vi "UHR-Fleezers Control (host) - Mau_06pol.vi"() -> ()   [LabVIEW 2012]
uses:
  <vilib>/Utility/miscctls.llb/LVPoint32TypeDef.ctl
  <vilib>/Utility/miscctls.llb/LVMinMaxIncTypeDef.ctl
  <vilib>/userdefined/High Color/nirio_resource_hc.ctl
  <vilib>/Platform/TimedLoop/XDataNode/timing_clust.ctl
  <vilib>/Platform/TimedLoop/XDataNode/nitl_modes.ctl
  <vilib>/Platform/TimedLoop/XDataNode/wakeup.ctl
  <vilib>/FPGAPlugInAG/PCIe-7852R/niLvFpga_Open_PCIe-7852R.vi
  <vilib>/FPGAPlugInAG/PCIe-7852R/niLvFpga_Reset_PCIe-7852R.vi
  <vilib>/Utility/error.llb/Error Cluster From Error Code.vi
  <vilib>/rvi/errors/niLvFpgaAdjustHostInterfaceError.vi
  <vilib>/FPGAPlugInAG/PCIe-7852R/niLvFpga_Run_PCIe-7852R.vi
  <vilib>/Analysis/baseanly.llb/Mean (DBL).vi
  <vilib>/express/express analysis/Spectral/Block/exnSpectralBlock spectral measurements PSD poly.vi
  <vilib>/express/express analysis/Spectral/Block/exnSpectralBlock spectral measurements PSD WFM.vi
  <vilib>/Waveform/WDTOps.llb/WDT Append Waveforms DBL.vi
  <vilib>/FPGAPlugInAG/PCIe-7852R/niLvFpga_Abort_PCIe-7852R.vi
  <vilib>/FPGAPlugInAG/PCIe-7852R/niLvFpga_Close_PCIe-7852R.vi
  openfpgaref.8.6.ctl
  <vilib>/Platform/TimedLoop/XDataNode/XDataNode.xnode
  <vilib>/rvi/interface/nirviOpenFPGA/nirviOpenFPGA.xnode
  FPGA Bitfiles/UHR-FleezersInst_FPGATarget_UHR-FleezersCont_0F5B06C4.lvbitx
  UHR-Fleezers Control (fpga) - 10.3.vi
  <vilib>/rvi/interface/nirviMethod/nirviMethod.xnode
  <vilib>/rvi/interface/nirviReadWriteControl/nirviReadWriteControl.xnode
  <vilib>/express/express analysis/Spectral/XNode/ExpressSpectralMeasurementsBlockNode.xnode
  <vilib>/rvi/interface/nirviCloseFPGA/nirviCloseFPGA.xnode
  <vilib>/Analysis/NI_AALBase.lvlib
  <vilib>/Platform/TimedLoop/XDataNode/XDNodeRunTimeDep.lvlib
  <vilib>/vision/NI_Vision_Development_Module.lvlib
  NiFpgaLv.dll
  <vilib>/FPGAPlugInAG/PCIe-7852R/niLvFpga_ConfigureFifo_PCIe-7852R.vi
  <vilib>/rvi/errors/niLvFpgaMergeErrorWithErrorCode.vi
  <vilib>/FPGAPlugInAG/PCIe-7852R/niLvFpga_ReadFifo_PCIe-7852R.vi
panel:
  in  "BD 1 Frequency 1 (MHz) 2":dbl=65.0 caption="T1 X (MHz)" min=50.0 max=100.0 step=1.0 format="%#_6p"
  in  "ESP Port 8":refnum<visa-resource-name>="COM22"
  in  "ESP Port 7":refnum<visa-resource-name>="COM22"
  in  "ESP Port 6":refnum<visa-resource-name>="COM22"
  in  "ESP Port 5":refnum<visa-resource-name>="COM22"
  in  "ESP Port 4":refnum<visa-resource-name>="COM22"
  in  "ESP Port 3":refnum<visa-resource-name>="COM22"
  in  "ESP Port 2":refnum<visa-resource-name>="COM22"
  out "Location path":path=path "D:/UnifiedHighRes_VIs/Locations.txt"
  out "Location Matrix":string[][](array[string])=[["N.D.\r\n", "N.D.\r\n", "N.D.\r\n"], ["0.19233\r\n", "0.00156\r\n", "0.20615\r\n"], ["N.D.\r\n", "N.D.\r\n", "N.D.\r\n"], ["N.D.\r\n", "N.D.\r\n", "N.D.\r\n"]]
  in  "radius":i32=10 min=1 max=20
  in  "clear markers":bool
  in  "trap\nmarkers?":bool
  in  "Sample Channel Flow":bool
  in  "Pump 3 contents":string="Bottom: ADig beads" caption="contents"
  in  "Pump 1 contents":string="Top: DNA beads" caption="contents"
  in  "Scripts":T1(tab)
  in  "Take Stepping Data":bool
  in  "Got DNA bead":bool
  in  "Got ADig bead":bool
  in  "Cap 1 Flow ON":bool=TRUE
  in  "Move Cap. 1 (DNA Top)":bool
  in  "Cal/Data Acq. Spot":bool
  in  "Dump Beads":bool
  in  "Cap 1 T ON":bool=TRUE
  in  "Cap 1 Samp Flow ON":bool=TRUE
  in  "Offset 2 Set":dbl=2.0
  in  "Offset 1 Set":dbl=1.0
  in  "Cal @ (MHz)":dbl=20.0
  in  "W/ Offset 1":bool=TRUE
  in  "Offset 1 Start (MHz)":dbl=13.0
  in  "W/ Offset 2":bool
  in  "Offset 2 Start (MHz)":dbl=16.0
  in  "Pause at Closest Delta (s)":dbl
  in  "Move to Delta 2 (MHz)":dbl=41.0
  in  "Attempt Limit":dbl=30.0 caption="Limit"
  out "Attempts":dbl=1.0
  in  "Wait Before Save (s)":u32=1
  in  "Fish for Tether":bool
  in  "Closest Delta (MHz)":dbl=13.0 step=0.25
  in  "Stop F (pN)":dbl=10.0
  in  "Then...":string(combo)="2"
  in  "Move to Delta 1 (MHz)":dbl=15.0
  in  "Tether Alarm?":bool=TRUE
  out "Tether":bool
  in  "TA Cancel Save?":bool=TRUE
  in  "TA Green Off?":bool=TRUE
  in  "Raster Set Upon Tether":u32=1
  in  "Save at end (5, 6)":bool
  in  "N Steps":dbl=20.0
  in  "Step Size (nm)":dbl=0.34
  in  "Save ave factor":dbl=1.0
  in  "Dip Trap Delta 1 (MHz)":dbl=15.0
  in  "Move Trap Before?":bool
  in  "Save Data After?":bool
  in  "Green ON After?":bool
  in  "Dip Trap Delta 2 (MHz)":dbl=15.0
  in  "Move Trap After?":bool
  in  "Duration (s)":dbl=1.0
  in  "Dip for Protein":bool
  in  "APD to Watch":bool
  out "Duration (s)":dbl
  in  "Action":string(combo)="Yank"
  in  "Fl. Triggered...":bool
  in  "Fl. Delta Thresh. (kHz)":dbl=0.6
  out "Waiting":bool
  out "Fl. High":bool
  in  "N pts to average":u16=6
  in  "Yank Delay (s)":dbl=3.5
  in  "Yank to Delta Array (MHz)":dbl[](array[numeric])=[16.3, 15.85, 14.85]
  in  "N Array El":u8=3 min=1 step=1
  in  "Random Choice":bool=TRUE
  in  "Force Yank":bool
  in  "Force Reset":bool
  in  "Y change (mm)":dbl
  in  "Profile":bool
  out "Sigma/Mean 2":dbl=nan caption="Sigma/Mean" format="%#_2g"
  out "Rate sigma (Hz) 2":dbl caption="Sigma (Hz)" format="%0.2f"
  out "APD 2 Rate (Hz)":dbl format="%#_3p"
  out "Primary Video Display":T2(plugin-control)
  out "Waveform Graph":dbl[](graph) caption="APD Line Scan"
  in  "Inject Top":bool caption="Inject Pump 3"
  in  "Inject Bottom":bool caption="Inject Pump 1"
  out "Messages":string="7:59 AM\tUHR-Fleezers ready.\r"
  in  "APD Ave N":dbl=10.0
  out "Int. Time (s)":dbl=3.0
  in  "Stop All":bool=TRUE
  out "Sigma/Mean":dbl=nan format="%#_2g"
  out "Rate sigma (Hz)":dbl caption="Sigma (Hz)" format="%0.2f"
  in  "Tab Control 6":T3(tab)=enum."Imaging"
  in  "APD 2 Offset":dbl
  in  "APD 1 Offset":dbl
  out "RMS (Ang)":dbl=nan format="%_2g"
  in  "Bead Sep. Int. Time (s)":dbl=5.0 caption="Int. Time (s)"
  in  "Below (kHz)":dbl=0.5
  in  "Above (kHz)":dbl=2.0
  in  "Adjust Scale\nto Mean":bool
  in  "Rescale on Mean":bool
  in  "Offset (nm)":dbl
  out "Mean":dbl=nan caption="Mean (V)" format="%#_3g"
  out "Force":waveform(dbl)[](graph)=[{"t0"=timestamp(12.90000000000001 s since 1904-01-01), "dt"=0.15, "Y"=[nan, nan], "attributes"=variant("NI_ChannelName"=variant(string "T1 X"))}, {"t0"=timestamp(12.90000000000001 s since 1904-01-01), "dt"=0.15, "Y"=[nan, nan], "attributes"=variant("NI_ChannelName"=variant(string "T2 X"))}]
  out "APD Chart":waveform(dbl)[](graph)=[{"t0"=timestamp(12.90000000000001 s since 1904-01-01), "dt"=0.02, "Y"=[0.0, 0.0, 0.0, 0.0, 0.0, 0.0, 0.0, 0.0, 0.0, 0.0, 0.0, 0.0, 0.0, 0.0, 0.0], "attributes"=variant("NI_ChannelName"=variant(string "APD 1"))}, {"t0"=timestamp(12.90000000000001 s since 1904-01-01), "dt"=0.02, "Y"=[0.0, 0.0, 0.0, 0.0, 0.0, 0.0, 0.0, 0.0, 0.0, 0.0, 0.0, 0.0, 0.0, 0.0, 0.0], "attributes"=variant("NI_ChannelName"=variant(string "APD 2"))}]
  in  "Calibration":u16(ring) items=["None", "Position", "Force"]
  out "T1 X":dbl=nan caption="T1 X (V)" format="%0.2f"
  out "T2 X":dbl=nan caption="T2 X (V)" format="%0.2f"
  out "Bead Separation":waveform(dbl)(graph)={"t0"=timestamp(12.90000000000001 s since 1904-01-01), "dt"=0.15, "Y"=[nan, nan], "attributes"=variant("NI_ChannelName"=variant(string "T1 X"))}
  in  "Amplitude (nm)":dbl=3.0
  out "Bead Mean (nm)":dbl=nan caption="Mean (nm)" format="%0.2f"
  out "Difference":dbl=nan caption="Difference (V)" format="%.2g"
  in  "Take Detection Laser\nImage":bool
  out "APD 2":T2(plugin-control) caption="APD 2 (Cy5)"
  in  "Flip Green Filter":bool
  in  "Set X Only":bool
  in  "Set Y Only":bool
  out "APD 1":T2(plugin-control) caption="APD 1 (Cy3)"
  out "Detection Laser Y":T2(plugin-control)
  out "Pointer Y (V)":dbl format="%_3g"
  out "Pointer X (V)":dbl format="%_3g"
  in  "Set Confocal Spot (X-Y)":bool
  out "Detection Laser X":T2(plugin-control)
  out "Saved APD":dbl[][](graph) caption="Most Recent Time Trace"
  out "Trap Delta Graph":dbl[](graph) caption="Most Recent Time Trace"
  out "Save APD Deriv":dbl[][](graph) caption="Most Recent Time Trace"
  out "Delta Fl. 1":dbl
  out "Delta Fl. 2":dbl
  out "All Signals":waveform(dbl)[](graph)=[{"t0"=timestamp(12.90000000000001 s since 1904-01-01), "dt"=0.02, "Y"=[0.0, 0.0, 0.0, 0.0, 0.0, 0.0, 0.0, 0.0, 0.0, 0.0, 0.0, 0.0, 0.0, 0.0, 0.0], "attributes"=variant("NI_ChannelName"=variant(string "APD 1"))}, {"t0"=timestamp(12.90000000000001 s since 1904-01-01), "dt"=0.02, "Y"=[0.0, 0.0, 0.0, 0.0, 0.0, 0.0, 0.0, 0.0, 0.0, 0.0, 0.0, 0.0, 0.0, 0.0, 0.0], "attributes"=variant("NI_ChannelName"=variant(string "APD 2"))}, {"t0"=timestamp(12.90000000000001 s since 1904-01-01), "dt"=0.15, "Y"=[nan, nan], "attributes"=variant("NI_ChannelName"=variant(string "T1 Y"))}, {"t0"=timestamp(12.90000000000001 s since 1904-01-01), "dt"=0.15, "Y"=[nan, nan], "attributes"=variant("NI_ChannelName"=variant(string "T1 X"))}, {"t0"=timestamp(12.90000000000001 s since 1904-01-01), "dt"=0.15, "Y"=[-0.0004235663930173644, -0.0004722739341410556], "attributes"=variant("NI_ChannelName"=variant(string "T1 Sum"))}, {"t0"=timestamp(12.90000000000001 s since 1904-01-01), "dt"=0.15, "Y"=[nan, nan], "attributes"=variant("NI_ChannelName"=variant(string "T2 Y"))}, {"t0"=timestamp(12.90000000000001 s since 1904-01-01), "dt"=0.15, "Y"=[nan, nan], "attributes"=variant("NI_ChannelName"=variant(string "T2 X"))}, {"t0"=timestamp(12.90000000000001 s since 1904-01-01), "dt"=0.15, "Y"=[-0.0005883053071687949, -0.0006281319620349712], "attributes"=variant("NI_ChannelName"=variant(string "T2 Sum"))}, {"t0"=timestamp(12.90000000000001 s since 1904-01-01), "dt"=0.15, "Y"=[nan, nan], "attributes"=variant("NI_ChannelName"=variant(string "T1 FB X"))}, {"t0"=timestamp(12.90000000000001 s since 1904-01-01), "dt"=0.15, "Y"=[-0.0004680013428144157, -0.0005167699209570592], "attributes"=variant("NI_ChannelName"=variant(string "T2 FB Sum"))}, {"t0"=timestamp(12.90000000000001 s since 1904-01-01), "dt"=0.15, "Y"=[nan, nan], "attributes"=variant("NI_ChannelName"=variant(string "T2 FB X"))}, {"t0"=timestamp(12.90000000000001 s since 1904-01-01), "dt"=0.15, "Y"=[-0.0006226691488387671, -0.0006504715109714008], "attributes"=variant("NI_ChannelName"=variant(string "T2 FB Sum"))}, {"t0"=timestamp(12.90000000000001 s since 1904-01-01), "dt"=0.15, "Y"=[-0.0007901852473525123, -0.0008601641895809732], "attributes"=variant("NI_ChannelName"=variant(string "PSD Y"))}, {"t0"=timestamp(12.90000000000001 s since 1904-01-01), "dt"=0.15, "Y"=[0.00031556138798181086, 0.0002525101474044007], "attributes"=variant("NI_ChannelName"=variant(string "PSD X"))}, {"t0"=timestamp(12.90000000000001 s since 1904-01-01), "dt"=0.15, "Y"=[-0.00019678334910122974, -0.0002453993346964931], "attributes"=variant("NI_ChannelName"=variant(string "PSD Sum"))}]
  in  "Signals to Plot":i32(listbox)
  out "Trap Disp. Freq. (Hz)":dbl=6.666666666666667 caption="Freq. (Hz)" format="%#_6p"
  out "Display Period (s)":dbl=0.15 caption="Period (s)" format="%#_6p"
  in  "Trap Disp. Downsample":dbl=10000.0 caption="Downsample" max=20000.0
  in  "APD Disp. Scale":dbl=0.1 caption="Scale (Divide,\nfor above plot only)"
  in  "APD Disp. Downsample":dbl=2.0 caption="Integrate" min=1.0 max=30.0 step=1.0
  out "APD Display Freq. (Hz)":dbl=50.0 caption="Freq. (Hz)"
  out "APD Display Period (s)":dbl=0.02 caption="Period (s)"
  out "FFT 1":cluster{"f0":dbl, "df":dbl, "magnitude":dbl[]}[](graph)=[{"f0"=0.0, "df"=16.666666666666668, "magnitude"=[-331.1367572010275, -79.05506245821404, -86.61411242440559, -88.4728176091699, -90.3181253945935, -94.12566333707997, -92.52740723119955, -94.92192587982518, -99.60936585245742, -96.87568627870715, -94.02570383337763, -83.8058550151726, -97.57441397235512, -101.59968530846606, -101.523049255742, -103.35038532190343, -101.58594091014982, -102.96098031851216, -91.39759462745924, -103.75019963279499, -104.45030075054324, -103.04245334279298, -104.0720279134107, -106.06482372394834, -103.69131867828104, -104.40395035115309, -105.96420043276396, -107.6735556337804, -106.673030006608, -107.34889066208132, -108.05626565233933, -106.25659018850432, -105.29934513380842, -105.43096056709592, -108.3728498841465, -106.0555440144992, -105.78001282181421, -107.48741857324953, -108.67624970548897, -105.39976667156175, -105.91413119232612, -109.4222808198164, -107.0898971593174, -107.91164191890915, -108.26032038855709, -107.58332347164534, -108.23559688234297, -108.01271040303237, -107.66511723652701, -106.51901583170391, -109.27249501469946, -108.55647681594805, -107.93499259231463, -107.05068166453935, -109.13641475410455, -109.29679733781423, -108.19360835527803, -109.57747591546632, -109.58364591011674, -110.47061433372711, -109.8144340420426, -108.79067462293897, -107.54887553357234, -107.99559866705923, -108.85023923652685, -109.68733225238618, -108.51101278437793, -108.51620475114115, -108.22212402200637, -104.63726950302143, -110.2989919678048, -107.61796444414897, -108.68882962798736, -104.79193983043893, -103.59504263746938, -93.64633660288543, -101.9191640501395, -105.73717393151816, -108.92572458793902, -107.43962662800902, -107.79595323081325, -107.0923101993207, -108.17603277205289, -107.87074270713183, -109.20899066381877, -108.61832060412445, -109.10072003106593, -105.76480632823524, -108.60877649218978, -109.67541158970121, -110.2286232768028, -109.84952155309578, -109.33772024076384, -109.95251642394683, -110.14777282585466, -109.13825677905699, -110.05989365698167, -109.39359990189426, -110.56255614635295, -109.66477183197163, -108.9397158528824, -110.26529907650465, -109.20049464984628, -108.20183857013548, -109.09752250184418, -108.00440442238454, -108.35465963524055, -111.16774134451799, -110.34812550238405, -108.94506763426756, -108.72845542102493, -109.41512344014713, -112.44661664432377, -110.35437330889101, -111.32939440655925, -109.42989530434981, -110.98084669076195, -111.92160561143541, -108.57755551751093, -111.40042616180912, -110.15284955891853, -112.21455132279115, -111.40787773511747, -108.82949641635288, -110.13442122547907, -111.42229298204664, -112.06314940885191, -110.6015308813694, -109.51144097251623, -111.15989713761475, -110.25535755335385, -109.65868178057926, -110.51649885452997, -109.77194745285269, -108.4234206864394, -109.50892632093968, -109.46471287444389, -107.92241289271415, -109.72283805386196, -108.63426821579918, -110.37316681536255, -111.09713996884652, -110.32903619589223, -105.32012665515045, -107.36858557554393, -108.00382215905725, -110.06430686942338, -108.81666625979916, -110.01277074453823, -110.94194741225512, -109.65934609082873, -107.80979136006962, -112.81333866824724, -111.61474300955487, -109.83998277184975, -109.45953946904639, -109.79640584952526, -108.19172301667324, -109.28894656674316, -107.61471301278785, -108.83814006090513, -109.08866847726084, -108.20250571862371, -107.96222236861584, -107.03811197900873, -108.93533000393974, -107.74482548035408, -110.79811544577694, -111.1387476496877, -107.42970105883512, -109.18442281176472, -108.73546184641192, -108.71800246690864, -108.51945944378063, -108.06825856571285, -107.27210712368412, -108.12304695877637, -107.84933283677306, -109.73682373154998, -109.32284761503395, -109.31328817453769, -106.68762108642842, -109.79203616876461, -109.9020278896408, -110.27080024357275, -108.54152101558762, -111.00464391726017, -112.42244020766577, -110.82707315747889, -111.00344011890857, -109.90461839395674, -109.42877207451863, -109.73549298167016, -111.67494793393293, -108.85799077901427, -108.5348443278263, -109.803781083881, -108.30644755543659, -108.5079527456017, -111.2055351312823, -108.53089994340155, -108.01739789012176, -108.70360662855235, -107.95873456794631, -109.58297170693093, -108.9372401694271, -110.15921663527153, -109.22399119911955, -110.89883651739237, -108.92840112258382, -110.0545300523626, -109.05961065387005, -109.45831398589371, -108.61239387653227, -110.13001256174265, -108.80060224137931, -109.46327400696283, -108.0177965824709, -109.29727944627197, -110.3237255895986, -109.03258262543821, -110.97880178489321, -109.70034895077919, -111.16405638194153, -109.17324451464711, -109.65698250854277, -108.96750235822178, -112.00534231585624, -108.69274607723942, -108.98110446396657, -108.40723795464795, -111.44459094807324, -111.74799245277113, -111.1601960491512, -108.92048232753773, -110.30506377784799, -111.33145973979093, -110.91850998672503, -110.33684985776448, -108.90206518366908, -109.28458878227542, -108.98773986023751, -110.85813863075646, -109.00041591105906, -110.84543686681204, -109.84382395806176, -109.69722434763266, -108.50915601095721, -107.80829925826895, -110.59736107582401, -109.75377770317087, -109.3992084496136, -110.51151565846742, -112.49753959826434, -109.7299632589479, -109.54070743868353, -109.90314341132164, -111.05974202976806, -109.03766862152392, -109.46667095459878, -109.52800799036197, -111.3163121356807, -110.07817134522178, -108.69251657453547, -109.40472158898045, -109.71400709815576, -110.60534468715097, -109.46937396724682, -107.70342491418788, -109.86331122597839, -108.64971387994616, -110.90117371097081, -108.34928840565928, -110.04172889660904, -111.52979926554961, -110.34759300823305, -109.62712781837159, -109.24131154553284, -110.23196152450447, -108.68509612326807, -108.0246905483419, -106.61876139289784, -101.5519630114271, -80.57695480953835, -102.03744443354402, -107.1449217193017, -110.0695213407169, -106.61597783999268, -110.79221011808191, -109.58974545931426, -109.1149802216988, -109.20993813088597, -109.63768480465863, -110.10428394219181, -109.08445084271477, -108.83472375362581, -109.69508502050168, -108.05588796178941, -110.62586360101581, -109.95315261676905, -107.52208264977473, -108.80708007514875, -110.43484881098874, -110.45942171588936, -107.83804717866751, -109.98973910294193, -109.3496496054193, -108.425252911127, -110.94579264380809, -108.54181722177951, -108.67696070083541, -108.4150202151644, -109.24973583101504, -112.0454922608961, -111.29046597340738, -110.75018248960077, -109.38326363603683, -109.2033340336957, -109.45076170874889, -109.52878049853727, -109.32340869724774, -110.98123395128233, -110.75736340635505, -109.7218385823809, -107.97422606064993, -109.77313701758703, -110.95948744392717, -110.08996774172691, -108.51011830110778, -109.78063140243836, -110.65996628628228, -109.83684298615616, -110.33329049188029, -110.13755118968292, -110.3717925645783, -108.55302219178951, -106.86811628734195, -108.6302156589162, -108.75341391045045, -108.32589578384841, -108.70061474734084, -112.30742263527534, -109.16842570592085, -109.29767035534508, -108.87829025017463, -108.2255616391397, -108.4316108616088, -108.82995906929271, -110.40135575415563, -109.51623498946435, -109.79409808792403, -107.03832759632121, -108.36534528684132, -109.72010868372905, -107.90933028179892, -106.95643597294047, -111.29929166165778, -110.23001135794706, -108.98838015381585, -109.79115357104436, -108.18627479511115, -108.14988122174307, -109.12074063466532, -109.41904850488358, -111.40409873721113, -108.83156790193294, -108.77032248953847, -108.88363158686694, -108.47515048290681, -105.94172147874599, -109.38146940214403, -109.21277078848794, -108.11309390545507, -110.70840012427504, -109.5504457849329, -109.52330684534209, -110.06776026911132, -108.21949434182314, -111.21266686269992, -108.78581501170974, -108.43115799297222, -109.63260325780062, -109.84070220619535, -109.72041980780126, -110.29615941882527, -110.60316734262464, -108.79165446414692, -110.95840439895592, -109.64926233107009, -109.16526769544322, -108.65292362430982, -109.56113898129935, -109.85693046339026, -108.92316027325207, -109.79492493553914, -109.38157962945887, -110.24545136266825, -109.30031463492487, -109.0795429936869, -111.4091719525013, -108.63499083917162, -108.43863465339358, -109.23207864880891, -111.21947487191643, -109.24525201480154, -109.56842406077318, -109.46711940800672, -111.91389548262572, -108.15655736690546, -108.71882059966947, -111.26328503478568, -110.95027143873176, -108.4853106242357, -110.36902802777546, -109.9314203579182, -108.77686164101732, -108.71871020068312, -111.04829661168574, -109.95072655339462, -109.88221342875462, -109.53241732756136, -108.2625005404823, -108.00677030040697, -110.19659317581693, -108.93858924796267, -109.46817875483995, -110.78063992017232, -111.11066570318451, -110.78774336696706, -109.19199744617812, -108.54914256407436, -109.28414960420909, -110.64143585101183, -110.5855350821307, -109.47578632252726, -108.89705360836223, -109.89214013612292, -107.93271261027171, -109.32631601340563, -108.60274611341092, -109.40110159872573, -110.889237682208, -110.01391165813328, -109.99747108785071, -108.65542819213674, -110.37211847668736, -110.44656500845738, -110.8128133834973, -108.8909299260433, -110.19551227077532, -111.37647266643523, -110.83802189730321, -109.98519377913681, -110.52378970770522, -108.16970420057817, -110.70974729773344, -110.76836765494402, -110.26884275594577, -109.22041044268806, -109.87809744746195, -107.76823252107832, -109.12119474042969, -110.28066108731146, -108.55000033509207, -110.18152097767907, -110.73030521152278, -111.49470908029893, -110.2320929919509, -110.03370979233021, -109.79181668155233, -108.6673501209991, -109.86695766650877, -107.88926518046961, -110.95525003776572, -109.18130359755742, -110.42618009658618, -107.90341931158893, -111.44736855661769, -110.72634267386593, -109.29945988519303, -107.67889101961411, -108.81148059987765, -109.13375212757057, -109.8122873383549, -109.80176697684155, -109.96342275204768, -109.90406635707086, -108.75674342748256, -110.12362902701081, -109.82151095527837, -108.62543344241836, -110.09171852771195, -110.21434637862887, -109.97254504855631, -109.27043209093468, -111.35149588204125, -110.12399876776051, -111.65983675538546, -109.28788875768564, -110.86554069990251, -111.26990906470603, -108.60956517491746, -111.49613890850938, -111.79685722966795, -109.26269485364045, -110.38555615546439, -109.40641023162068, -110.966136593156, -108.78892524584494, -110.29340727375603, -111.44032043281035, -109.95212021173755, -109.79233511584334, -112.41184021118175, -109.73687851881148, -108.65493879781806, -110.76132988919045, -108.43230346094671, -110.32968175895853, -110.29890782023821, -108.77609076424456, -110.3298662333555, -109.47734504217333, -108.2677295732245, -109.21234363352882, -107.83278941978479, -108.85136784424789, -108.43241251530755, -109.76609391460555, -108.53204373005357, -110.9660641972934, -110.3152512161094, -110.72570499399905, -109.23877906286317, -111.72407743101837, -109.20311421918561, -108.06021800233717, -109.29288625761943, -108.78395253409145, -111.85250172876302, -108.78827588901797, -109.79775055719482, -109.12089297455859, -109.49896359356035, -110.34432647103819, -107.94700097960238, -109.30489238477631, -108.89170290869342, -108.82574563272509, -110.11024077194833, -107.37946433552314, -109.60167933458756, -107.80625057819019, -110.11489057210264, -107.35436859378505, -105.69819484613895, -109.11280625683739, -109.27770293057978, -107.7053735252589, -109.75022444894368, -109.3310543596577, -107.87683693707739, -108.19931495338068, -109.26462246191564, -106.71885779297867, -100.00018022217961, -92.54434511397295, -107.20472143807373, -107.39203415155283, -110.04461177268398, -108.48860496315312, -109.0057168110333, -108.37627790492552, -108.4108380728248, -109.65509454313073, -109.64243000632982, -97.04219069306761, -109.0928856629964, -107.9760697315632, -107.52611064047497, -108.87702814778996, -109.08437599027614, -110.70097118837974, -109.00969860961283, -110.38275386163214, -110.0699155421545, -106.91498895181175, -106.22178738309017, -109.36827866896039, -107.59953130968307, -109.19516217272808, -108.31502495393616, -109.384158926223, -107.11670654202719, -108.09436312738853, -110.14559230873704, -109.84997663447679, -107.83465335309926, -108.60947100624459, -108.9932479423645, -109.17174810371898, -108.79457339828916, -109.40909327982367, -109.6328723628302, -109.51081854476179, -107.63054408568418, -109.63728404010122, -108.51163794839918, -107.55002282725216, -108.97796212764939, -107.24648164623483, -112.21470452291085, -108.74294024554423, -109.62070777514892, -108.05768666239368, -109.8224946685739, -109.34575507446003, -108.53536952609525, -109.60789300457671, -107.56681538208278, -109.22777325016398, -108.79047910308894, -110.10332477250668, -108.00206387955672, -108.45604004720035, -109.00645795765472, -109.81039564269616, -108.92785144634745, -108.3978471520567, -107.94411095685999, -110.53486519304262, -108.8773780319227, -109.03345093296107, -107.30746693745031, -108.54277704832029, -108.77629108166091, -108.91111762599647, -107.74965195880401, -109.97375370738439, -109.76326492689246, -107.91717581777407, -109.0730556927617, -107.66804873204664, -110.40438871064791, -108.05794247751498, -108.80206615156494, -107.51329354700796, -108.83687012994949, -107.57713176895379, -107.94774159581414, -109.41894615439651, -107.10869425078764, -110.51480854078629, -108.92221367099775, -109.91358786461535, -110.1744263092835, -109.30795472883494, -107.91359710691006, -109.77888185049835, -109.52060975706438, -108.66686651982212, -108.71041801553639, -110.13619546359467, -108.87957097273856, -109.72150387215271, -109.00776068810654, -109.70251113927438, -110.75769213896399, -108.53234896741436, -109.69439526582246, -110.15412541604617, -108.25183374628219, -107.97402569656481, -110.34920156998648, -108.45106995186384, -108.82031145748209, -111.38690005057539, -107.01968459818563, -110.3044500039584, -110.8755481852125, -111.08915057663255, -107.94824988655199, -110.21669144934839, -109.90539774633154, -109.58985438756767, -110.12258796623348, -109.41689951612143, -109.31128210476795, -109.00258476567323, -109.11093063041056, -108.83347064311234, -108.32685287566952, -109.44770946560935, -108.40145063144861, -109.68448193892085, -108.76525439243828, -107.62837139034596, -107.39300298848994, -109.36993934990318, -109.2465218489418, -106.66307369796812, -110.15891092764934, -109.57151745419041, -108.92425698310808, -109.8036704717834, -108.79751146756549, -109.25926431818017, -108.46260574057584, -109.1967554647261, -110.63319560262356, -109.02343067385144, -111.22073171487528, -109.4731095097105, -109.69335000085164, -109.48782989577005, -107.95204227683271, -108.19468255763758, -111.36195112053247, -109.55696116543685, -110.3130767640534, -108.9621824253354, -109.99735074896789, -109.20198058456344, -108.12100614259485, -111.27227490807289, -110.09248554008288, -109.14395535060149, -110.80882692379708, -109.22632926901655, -108.64497210802793, -111.00030482190711, -111.1317849358033, -107.43140429257826, -107.9783302193555, -109.2639893652291, -108.97008485446163, -108.66556668859064, -108.12995785876932, -109.73001061107855, -108.09691302413727, -110.68391499215569, -112.78583642012705, -108.7093037763389, -110.67868795924797, -109.0190959349128, -108.36247198231372, -109.82829353258869, -108.24916379311045, -109.84154533905823, -108.55470160833775, -109.75438989348815, -108.82865632118325, -107.63622268162582, -111.00943492886312, -110.81824358463759, -109.46028423652966, -107.52479398900992, -108.99087806823736, -109.94494831750349, -110.26788355564504, -109.8954055022304, -106.9478122391182, -108.91705388158901, -107.76095584490312, -109.28456723055147, -109.7982307261767, -108.98552661346622, -109.98937979783426, -110.57907422426224, -108.68113463944836, -108.06257240208589, -110.0707224529617, -109.19515280354733, -109.35868842818849, -110.37311467065695, -109.0404734478992, -108.16686395270187, -108.61859220485148, -109.19986437876149, -108.19707189725302, -110.06564239663074, -108.87850403465154, -110.63824157544798, -107.36918104067212, -108.7008736325543, -110.9359398265406, -111.08529123080929, -108.44209934821818, -109.79529621208783, -108.38917887958179, -108.169117639508, -109.24332926356216, -110.50584058811704, -109.63592524002665, -109.32261039377495, -109.16720880524552, -109.3084314664462, -109.5812223978583, -107.70213196487856, -108.0557884982431, -110.67058020007828, -111.68459781023608, -109.66270627185824, -110.52536245663693, -109.70208409132103, -108.78645420809342, -109.23122088059863, -109.24601474121832, -111.25604763816514, -109.50225851581177, -107.32434217163818, -109.28548556764925, -107.59972621660836, -110.46928774723048, -109.25950101547609, -110.32016453935465, -107.78482761561703, -107.89462895091089, -107.51366154391481, -108.08036891159172, -109.53371809947035, -101.2452927166745, -109.32763325689056, -107.52166868423687, -109.89648659445174, -109.11350200980485, -109.81336712738089, -110.02799517445062, -108.02767143538516, -107.97850220501483, -109.50772934896838, -109.31069875721964, -108.49991657749598, -105.60880911233095, -109.79128597340213, -106.91084537903113, -107.84880087118997, -109.63628170511824, -109.03203967193224, -110.64186113413658, -110.98027990365594, -112.33841002907062, -111.01793075565425, -108.58025797022215, -110.4259296883756, -110.38643255981424, -108.93051671115133, -110.97544177116494, -108.63883100482677, -108.37581711765226, -108.90240163126536, -107.94688047875466, -109.9482937437732, -110.09097112364414, -110.09805032265376, -111.44307114024532, -109.15483789122554, -110.9713708217832, -107.8548737634672, -111.41418477109195, -109.45699779859628, -97.03595099331734, -109.16746744169623, -109.66209204485918, -112.57048704774604, -109.73989735035725, -108.16252575067017, -110.7546980664636, -108.91536673403449, -109.20509151422344, -111.0260632167785, -109.62924582406518, -110.45466277291722, -110.2973970018937, -109.67550222925419, -108.84481022020094, -107.23686414357573, -111.79004633370906, -109.85453094194085, -109.45617270081004, -110.73920606732504, -108.90879956851099, -109.67774425528265, -109.4745715721361, -110.18080454693559, -109.26079184315502, -109.41692499885505, -109.02240975088358, -107.80833423058168, -109.32657361431549, -107.87138278655101, -110.910364670719, -109.70067156846706, -108.55301754282077, -109.4243252157005, -109.77567725161107, -107.83737232063925, -110.36509412773016, -109.6371048811367, -109.49430894422814, -108.55509251499753, -108.03996302911446, -110.4385715838736, -110.08864436068788, -109.48922484379962, -109.90865554258562, -109.7491963238264, -110.04796094537969, -107.413043439116, -108.54229076126079, -108.2522516728666, -109.75464941327974, -110.26795832300996, -109.28073673851144, -108.62990200974927, -109.89408067552287, -109.09160284731726, -109.90740624925795, -109.92534708896517, -109.79578862362752, -109.97278346890566, -107.80679350393824, -112.81728446281548, -108.09689504419987, -109.89549991422173, -108.43930976031248, -109.95153099843282, -108.18277483720716, -111.89607792605433, -109.52567003805, -109.17125106979698, -109.64300739407085, -108.21045178846524, -109.64036472149706, -109.02324448538845, -109.039163008889, -110.41006510134076, -109.50289952116489, -110.4732620447796, -110.08777181504614, -110.15589511434341, -109.55705089158471, -109.2547682932589, -110.86823885471617, -109.96330502176939, -109.85995369810554, -110.63211290903473, -112.08007783432191, -110.24725218052279, -107.62861148917592, -110.08691795849435, -108.89793794632287, -111.07702220466341, -109.46946126482341, -109.19747345337464, -110.70018609416007, -109.66366205691908, -110.78032312133551, -108.05724200456513, -108.195661625627, -110.90724508408255, -110.08307674771669, -110.76863516643007, -110.46620425061583, -109.16986788877276, -109.61921294239114, -108.51159432329543, -109.96308336765689, -107.38178944242856, -111.95930944846394, -109.3329826827624, -109.59119636368249, -108.83148571828912, -110.46194288788257, -105.87694286145472, -107.985886302892, -109.2975019660806, -111.05138725716857, -109.60005889204612, -110.92871351729086, -110.73480546964537, -108.41587420326718, -109.84275465824477, -108.8249071047676, -107.65358887817105, -108.3254150042995, -111.47362100321767, -112.7287536850025, -108.8217125660507, -109.50232320231771, -110.29587061625348, -109.30644535112089, -107.69178032077258, -110.84522325672016, -109.3735891463141, -109.12506388923123, -109.65582307934665, -111.11427272192576, -112.19827973435466, -109.11306367925813, -108.19203577968261, -107.89831568266465, -108.85805249169313, -109.51100049661844, -111.71546684086955, -109.53880495724334, -107.07739286222231, -110.66836728754211, -111.5415170557177, -110.16051267940297, -110.6107546662698, -111.36389129556191, -107.77888179117923, -110.34160392509817, -109.61287125994414, -110.23791773883013, -111.00669159903549, -110.97165069538953, -109.43965413392434, -110.6813161690388, -110.31441293654314, -111.96129906273796, -108.15998218707462, -110.08095912053633, -109.41084567452768, -109.28774416263552, -110.80159950384204, -110.41956747809755, -108.85005186267244, -107.9069227847757, -108.84249369063123, -109.92569208845894, -109.34109797584448, -109.41334788055491, -108.76462023086997, -108.22069272136177, -107.0786679601274, -108.30206755098202, -108.57613406368954, -110.83330887636482, -111.93966942736989, -109.76373713473264, -108.25782074884941, -108.16490627215555, -109.93351470267982, -110.75525684428368, -108.22814762283093, -109.73442331991602, -107.53145627482685, -108.27195221226805, -110.33032779278457, -109.48951857415828, -108.12599093700939, -107.97627415508097, -108.81426859968796, -111.21764717894752, -109.80856212352333, -110.92658779118501, -109.71551885834796, -110.38682741010847, -108.87671328341361, -109.68368600774755, -108.35359806351899, -111.7519400010676, -109.89407081573103, -108.24301180922755, -110.00646944788126, -108.6685299083706, -107.52856885980722, -111.7622363038509, -111.0025144494897, -108.64719599357296, -110.62968467177518, -108.821509935539, -107.94915453463719, -111.53070432277694, -109.87282048586256, -110.71167589371663, -109.79225006081626, -109.96203471712074, -110.29921092232489, -110.10644439440416, -111.28815007382043, -111.19165661703703, -108.46024117100558, -110.22528296512183, -110.32184972386672, -110.05120383416072, -109.78792549362107, -109.00355659956696, -108.85989369286315, -113.00899556732638, -110.91756826567867, -111.25016866167897, -111.84225040552181, -110.54451635944174, -110.72722829912917, -109.60759702177283, -110.49362602516815, -108.74419542915284, -110.3379671069179, -109.66259088220754, -110.45956400953156, -109.13956157147233, -109.27130155486806, -110.83015602667983, -109.17970724944131, -109.09662765889193, -108.0447366108107, -108.9536269357457, -110.35663108940085, -108.73418835472056, -113.42965806805827, -111.81270536656905, -110.06155590173537, -108.76582224646269, -106.7488061675813, -108.5700320158723, -111.11038264410035, -110.41435767488723, -109.12763443489911, -109.30517580756394, -111.61251165371237, -109.8116632664339, -109.36845864976851, -109.00390009629231, -110.54359197165573, -109.52629258465976, -110.75932197632896, -109.50903215359567, -107.42652056246085, -107.81146496533543, -103.22224383145215, -108.53803076819163, -109.78623360072066, -109.66306634612869, -110.80245829141279, -111.87835085452016, -102.27372781471168, -111.27763038431458, -108.45838423437681, -108.79077917058028, -109.31951755762685, -110.05415097017186, -109.5535934823387, -111.62732254641111, -110.73478247119641, -109.9468722686683, -110.39698367573979, -109.30612942398305, -109.7578384694043, -109.34817295524313, -105.56944757301993, -110.1940418750125, -109.27076023513962, -111.03491935225027, -112.2980497521063, -110.65725497955563, -109.0567530102422, -110.31700596563523, -109.64508026365678, -109.6190471404421, -110.52566833759428, -109.68595899227789, -109.7431160985074, -110.4798230300751, -109.45506977604765, -110.69504157940786, -110.63067849573177, -108.06456949500138, -107.99354148885966, -108.11349194720599, -109.15944121207349, -110.61766925164031, -110.14145801314527, -110.67420842201165, -111.91532881806512, -112.15901550030345, -109.94774413630104, -109.2819568305201, -110.94623189179737, -110.17685430287735, -110.39082916961016, -109.53953238698966, -110.76940623620611, -109.89327922318515, -109.10275695043765, -110.21445972656734, -110.58968777252528, -110.57016757660259, -109.59208496373341, -109.07946946465374, -109.10762003745964, -110.36892993974607, -109.81864495218393, -112.12972189864566, -109.26185849434863, -111.56305819991357, -111.36019621828058, -110.3397604159226, -109.58675612753163, -110.58041217474447, -106.34739062044932, -108.6722699609389, -110.03906060709869, -109.16794717548382, -109.65012481802809, -109.35377624077988, -110.51889143862303, -110.03397458059777, -110.7981307056636, -110.56653507062292, -107.61367005067231, -109.99279736988825, -111.79875182878175, -108.60382315996031, -109.71381533228038, -108.60388131505613, -107.0933685540362, -107.86037690830757, -108.40980028847238, -108.83869602763895, -110.76921375395764, -109.96766364716046, -110.8256171465781, -110.13805084291067, -108.5349140035878, -110.57158437465219, -110.8920694413417, -108.71646695477324, -108.33274238445665, -108.96152108305608, -111.03750932994224, -109.48915027983756, -110.29725207211165, -110.79527247268442, -109.47969936716117, -109.79306701834035, -110.16840035577498, -110.29840230783668, -109.15306387075587, -110.72651274964761, -109.08881658764956, -110.8349724030761, -110.64653625576447, -111.40392562616867, -109.94581588927414, -108.85136340231294, -109.77228546607624, -111.48297395390018, -109.7334001251941, -109.30537415590783, -109.63937411233408, -109.69785848648013, -109.3523781030017, -112.04667421182404, -111.56311816195343, -108.18548447362308, -110.63388993686104, -111.39768634137992, -109.87157345395542, -108.6734208287271, -109.46213300216168, -111.75774769437145, -110.10245994173216, -109.52385139033495, -110.96513097775451, -111.8709319163154, -111.54948269614047, -110.29760900080463, -108.52168175904663, -111.09033925738258, -111.14752744054172, -108.83074523709202, -109.05704141259113, -111.74377805749482, -109.57200906899736, -108.84121318623825, -110.86657990204343, -109.54363603755047, -110.89448416316372, -109.58965570570145, -110.21012263847972, -110.4063470702923, -109.5021950342969, -110.33648801598177, -110.90551031296536, -109.69205870504638, -109.8648503154861, -110.28183391384131, -109.65970942950766, -108.43615680946908, -111.11790511866548, -110.89043476451553, -113.64898442872548, -113.08004494963895, -110.81525412051718, -113.91009875719509, -110.95802128672312, -110.40944585634135, -110.33464695414992, -109.98984645778987, -110.18795067005652, -110.62364351231234, -110.44029833291248, -109.01598585569788, -110.95430216511514, -109.77987141110621, -108.54452361812068, -111.41780266439777, -110.47172771858405, -109.06084635984516, -109.30794593246578, -108.8764083815745, -108.18222749506985, -110.31330487887435, -109.04176821738014, -108.8558386035048, -109.47888284507395, -110.01459604573937, -110.48596659065309, -112.6781342298378, -109.85522803775775, -109.0569534499285, -109.08991286548698, -110.89485727880403, -109.18715778948663, -111.50381433568144, -111.3545424730884, -110.07710926239977, -111.99977850157067, -109.47444853853723, -109.81605328527645, -110.74995213151195, -112.56834665925544, -108.52052472391404, -110.89121213995557, -112.02004142355113, -108.66413739656008, -111.10053848695652, -110.41241079991636, -111.80152991764473, -110.21746151515111, -110.63265128607344, -109.483042128511, -112.78639954059729, -109.47114195846122, -109.23309637902875, -108.97133643967169, -110.08909147812822, -111.01105271457081, -111.18602432128249, -110.04633990216801, -109.53453538673071, -108.81939452082017, -111.13486114285661, -111.65877073200598, -111.63763706753498, -112.14107810664572, -113.6231865196724, -109.31743865878806, -109.18551713085722, -108.74951309653638, -109.28206426212142, -112.36687029711229, -110.10933061193728, -111.29501093502684, -108.19021080564794, -109.34497312126749, -110.37228033937312, -108.63277512903049, -110.61033993911002, -111.2975761598062, -111.49780004751436, -109.91019436685814, -109.32789992989028, -111.4482538110117, -110.1538439123475, -110.66347034043578, -110.05055133068794, -108.53002033538341, -111.7522199783972, -113.49108651193104, -108.03793940563418, -110.07108694011555, -110.83958739865201, -109.62805629409038, -112.69637731014087, -109.57996950503268, -110.104850643722, -108.83376203949506, -108.69400304840181, -110.59434352922563, -110.69121011800921, -110.18694553784364, -111.90598571547098, -110.30230802494223, -109.66810649416752, -112.6017099000434, -111.00296745333219, -110.64462650261785, -111.4775358707403, -111.98753241268494, -112.26574909791167, -112.04796822399412, -110.65853064447325, -109.6623218025264, -109.40559579075378, -110.42174451813142, -109.18991987957241, -111.02050178263048, -112.77950487440032, -110.42443751566815, -111.35440372400903, -108.5263524245987, -105.07498063939795, -107.15444425741984, -110.4508720018025, -110.25163264819463, -111.1383261104107, -109.91171620173931, -110.52200560606038, -110.5299174299573, -109.34628087255733, -110.26101817411786, -109.65071853372183, -109.66953335961068, -110.83590602054682, -110.980546313788, -109.4110066989163, -111.47223607390256, -110.00281523859483, -109.4088722967626, -109.00401922839337, -109.59655302543185, -109.7359970854586, -111.46016206343049, -110.23478747568004, -109.29441275295858, -109.82941912510167, -110.43088525283673, -108.21649744751299, -108.70220592702613, -105.2334473604296, -110.60620657984927, -107.97533820921146, -110.7664079806058, -110.56406610911355, -111.76465470250328, -108.84172809688911, -111.03661078143631, -109.85351980370237, -110.70091167176791, -109.52380717508088, -108.4356492672842, -112.25498760397127, -110.69648730540193, -110.36748838594507, -109.99090797924349, -111.2678642544111, -110.42541694325627, -111.4575545259775, -109.3211175669008, -112.7465573314208, -109.56208667784249, -111.59733497772172, -109.42295730962105, -108.55804089331346, -108.71397903286748, -110.09188290952392, -108.90810063278326, -110.31333217069538, -109.69794714542728, -109.06210020835357, -112.42465112160288, -111.74630553904855, -109.99304310093493, -108.93867687355595, -113.1669287525049, -109.09193568851137, -109.27500368450697, -108.99643325722404, -110.53962759110647, -111.2052088429852, -110.05855563908841, -110.30763723153481, -110.03411001268613, -109.6161415052669, -110.6304714466923, -110.17116005754627, -109.0753171640551, -110.92564270851628, -109.60831770517053, -110.25913363817017, -107.76644895378317, -109.2619309023068, -107.64198246311884, -107.37056168314048, -107.31978563121643, -107.68171928702894, -104.57515288104209, -104.75187637758803, -105.27246893266054, -106.96524396060869, -105.93920355631757, -103.66449995825586, -104.08476660009461, -104.53081578265315, -103.0148493379086, -106.74751670818362, -104.92309629919443, -103.98320340724693, -104.81633219413234, -105.77996356028235, -107.12559309216644, -107.28196039053535, -108.84583578337953, -109.4494696919565, -109.15525441177898, -109.7634811359225, -110.79433338587495, -108.44440079452527, -108.79597700117748, -109.98590735173822, -110.72144284267539, -109.30550753718086, -109.70072152916897, -109.65801130162137, -109.65949265997646, -109.82238573025273, -110.30669821947491, -109.83394128869384, -108.90433312205332, -110.664046708231, -110.39926453734134, -110.37725911098757, -112.12508639032839, -110.26795666332589, -108.98741993218054, -107.76168841100478, -109.82334992872889, -110.83516363498563, -112.60649745671253, -111.1960726449926, -111.03919163866381, -112.05129034965563, -108.83187987662883, -109.57240688505179, -109.32857861150738, -109.54934849013647, -108.29359879300195, -111.5179112931669, -109.52702486426027, -109.95429980789645, -110.7011078611564, -109.43204524997455, -105.56031249677113, -107.70609254346495, -108.78303653454363, -108.11457060956113, -110.44215460317537, -110.78267897406572, -110.33119812901934, -109.34449539666907, -108.82636558484161, -107.1834151347969, -108.83808254322192, -108.2542825327446, -108.80298057862501, -107.59922121598055, -108.9131916496929, -109.51519107961856, -107.7704986323755, -108.79678029009878, -111.13791068210752, -110.402746275919, -111.31702623823912, -108.49812727557243, -110.63723264798182, -109.32890666586829, -110.29721723278237, -111.66560929315017, -111.04227698307153, -111.36927505376269, -112.5203298417673, -109.93967930487354, -110.14533835678606, -110.3868348991775, -110.85413569165249, -108.44519725537315, -107.93391978795047, -109.82778679299085, -109.79311153223738, -109.25261055399044, -111.47738679135526, -111.11775495397512, -108.65898844492045, -110.26505495390529, -111.02017977446526, -110.34817965403467, -107.55161094495372, -110.21667403085983, -112.43970497917284, -110.70535338255132, -110.79438078890512, -109.81809822502822, -108.99167960596515, -106.5556893069368, -97.51736665041192, -105.29926513345109, -108.72453297392224, -108.23203912463346, -109.50324111400698, -110.9939986929772, -108.05367524487318, -108.37339392211176, -109.8553291283933, -110.46179639493138, -112.48795697163695, -111.88145079973545, -110.8678969738583, -110.62677605624849, -111.83824818603244, -109.76798658735359, -109.6654742351465, -112.58543522753767, -110.3406716250781, -109.55013159400883, -108.00481229232405, -109.90793236599207, -111.28597960985334, -110.54144527494444, -110.14704702870655, -111.2652554338908, -110.97520848958668, -108.63647576273343, -110.52472680617548, -113.16137826273847, -109.62457037485827, -109.53869420402964, -110.71399284283449, -108.55435337782664, -108.09492728294455, -112.2373886856363, -110.3693019226993, -111.65116752865308, -111.3223986412311, -109.67734725401074, -111.36420709226297, -109.14293108556625, -110.5982939020188, -110.29596476096043, -112.69847120697035, -108.39052787054206, -109.06205229490357, -110.00045399262885, -110.71775009467346, -110.69530760167493, -112.54144940754935, -109.55755373438097, -107.88943697845929, -109.98578587243783, -110.14202980613851, -110.80051915904802, -109.11327182471621, -109.50637030500913, -109.77023677605327, -109.98552825925917, -110.40235854896, -109.37603004890141, -111.36989177909379, -110.8399811877331, -109.30394670937987, -112.2769814990538, -109.10893172594731, -109.17733972841754, -108.35968166480572, -112.64492569586005, -110.13779257328873, -110.64439690778532, -108.45446935516622, -108.97325006911116, -110.54637968933774, -110.66412364132371, -111.38627695224784, -109.8942998516069, -110.36392017322382, -109.92355133054227, -109.61886697310419, -109.71969465343778, -109.85627196259388, -112.1407808286419, -111.1013489416651, -110.70428953307596, -109.3454280179969, -110.22984684615578, -109.53826801613613, -107.83673208330934, -108.72742563398342, -109.5745872123195, -108.83031823548816, -110.89059911076627, -109.87842545384129, -109.21980161063786, -109.07140273870678, -109.04628915564135, -108.79255665097845, -105.20875397856382, -110.0838008881032, -109.68293832806683, -111.24644641302518, -110.01257579497496, -110.99281477454484, -108.99296184719546, -110.96495665514604, -110.70404386182749, -108.25078498739035, -100.77667501455139, -107.61479263900088, -110.06600976399395, -110.02035637581871, -111.45524052052504, -109.975541184397, -111.07333860975358, -108.4808974233161, -109.59513524582242, -110.74711589861774, -109.50005300854993, -105.23071652566294, -111.81094849223531, -109.0168079712372, -111.89029991620679, -109.90672274216391, -109.30959446424889, -108.23718655264584, -110.10868108588909, -109.21139771899594, -110.33333323577992, -110.25792318324204, -110.67825932924109, -112.33148517950511, -108.9724848367048, -110.78371843797613, -111.40913868573313, -110.2930522718577, -111.9538408094371, -108.63639312641844, -112.4462941079034, -110.40266356498321, -108.66617580940074, -109.44306834729083, -111.08962916641603, -110.52132608161017, -110.53757698855654, -111.5587344449704, -109.77722315102946, -110.40060629757771, -109.45395807961631, -108.77558572395142, -109.0151938598724, -109.80739619986889, -108.9332873172888, -112.49933978358132, -111.28667321897437, -110.40629082858706, -109.9829216820938, -108.85102919990373, -110.84179127037925, -110.27309817549309, -109.88857884367955, -112.24517967927224, -110.23377125710859, -111.26951227953063, -110.09782138347559, -109.77508406986834, -110.55359722398646, -110.09534729906368, -109.96333904888587, -110.29372855476366, -111.36651812163072, -109.97141184588116, -110.16701683369045, -112.8562627359291, -110.66651146857079, -108.78873821095968, -108.59208174618087, -110.31784275318834, -109.43177042415276, -112.80272887161644, -111.79874205007107, -111.08216899537892, -110.73699224045636, -111.04738767291953, -110.43395896705012, -111.62106163510778, -111.32599933330843, -110.29360981749807, -109.66562228449096, -109.21316193790335, -110.06363162177448, -110.54480468587292, -109.31791670875509, -112.65386492377107, -109.91857609999171, -110.57233605624137, -110.7597333064856, -111.49767138733276, -109.36548654843229, -112.34145274183716, -110.52831153822652, -111.55802243871352, -111.81399803046556, -110.17680125962372, -111.23811621944807, -110.48042049674514, -112.43786993562033, -109.56507357271987, -110.67030752598993, -110.86377249100713, -109.06001892813467, -111.37023727930494, -109.52881096984436, -112.95107295160436, -110.49467818026214, -109.29804210589607, -109.89270706931751, -109.46354468058833, -112.10350702955014, -111.06083529077077, -110.49996587015904, -111.1617248913634, -108.84725633199014, -111.42852695852422, -110.01433866707184, -109.11616968390972, -110.76961079765468, -111.80403513904453, -109.84442686379181, -109.65447921666167, -111.3378640555306, -110.8882647652338, -112.58014202075226, -109.67128881545659, -111.73429980763389, -110.82258070774773, -110.71895931098041, -112.5117489008152, -109.16182299471309, -109.71651258790612, -109.7770618808562, -111.94294809571427, -111.1629115541574, -109.57489224865171, -109.8402445779754, -111.17931450307283, -110.09045865447595, -109.23658206733491, -112.54929616847242, -110.5150381158864, -111.32296447909377, -111.64472156295191, -111.65832771066007, -111.03359562742956, -110.85303206770837, -110.80655337650862, -109.3712696310075, -110.57313454785879, -111.18525355670417, -111.67423695430561, -112.00829831274282, -111.08915434609605, -110.3298290221436, -108.68552957386795, -112.11377370993225, -110.80288297661977, -110.33640536217185, -109.5907971201988, -107.9195263775506, -108.50223113159429, -111.91191347156142, -110.29585599512956, -109.50902788911351, -110.76819145749467, -108.86899533416589, -112.09963049260891, -110.13374376572433, -110.15881393584463, -110.87392107947531, -109.18658540731009, -109.72734703956934, -110.18732487568724, -108.76554115185057, -109.94122289815374, -110.39583285609643, -111.09540935727229, -110.6618176357367, -111.6281345666718, -109.69686483639367, -110.31633402076315, -110.61246951748903, -111.73300235294965, -111.34221378834899, -109.46708370903485, -110.70412671997354, -110.7007891485379, -110.31685483435038, -111.03016917417074, -110.94517365625376, -109.46580797053619, -111.20935248224806, -109.20661126636224, -109.50147037097533, -110.14241781654353, -109.8510950344643, -111.3794198224028, -111.28966889207122, -110.43347441663424, -109.86759980279523, -111.92101892013198, -109.31594011390644, -112.92253433794441, -110.74000829597605, -110.3690783911604, -111.9386136764295, -111.04196305034188, -110.41800427558245, -110.94287511448232, -111.66035388807579, -107.53723747644062, -110.68014818358719, -111.86628806511304, -110.12097497430523, -109.69880468221378, -111.4312783987915, -109.18240866486639, -111.45649839248873, -110.1242345454651, -113.75911576151633, -112.71747598882953, -110.9614554157337, -110.92294419716129, -110.87229098694876, -111.09943759113875, -109.48107247947176, -108.62783006742795, -110.8108025857779, -111.63342408317932, -112.0221522906341, -109.96411229549527, -111.29821085030613, -110.04566676239914, -108.41674583097112, -107.50256474992416, -108.68086611003493, -110.3738906060137, -108.86763212826641, -109.81681043446049, -111.04539822346567, -111.73290882980949, -109.75238769150758, -110.55268275367449, -110.48423701377924, -112.1116140908134, -109.53952175199518, -108.538611608547, -111.3788321484912, -110.36378736224961, -110.37712171023523, -109.82150687920334, -109.17046632238393, -105.1169578108227, -110.84067642540583, -112.91626789016587, -111.32030958133453, -108.93375913686056, -112.44450956563915, -111.1596840012794, -110.17380444915341, -109.634859036508, -110.68819277718731, -110.0648098825346, -108.87385575091399, -111.99676414571755, -111.32585405719519, -110.59892045991457, -110.32589048340424, -111.1172696292077, -109.79946399891651, -110.10030723919304, -110.71841081343656, -112.23013150012054, -108.94400401141407, -109.71044551701596, -111.77560214164039, -109.68779520039777, -110.96119601299907, -113.66477058855787, -110.17794649102234, -110.30159876509862, -110.11953836266514]}, ...(2 in all)]
  out "FFT 2":cluster{"f0":dbl, "df":dbl, "magnitude":dbl[]}[](graph)=[{"f0"=0.0, "df"=16.666666666666668, "magnitude"=[-324.19011195451765, -78.1272953812706, -85.85545438627958, -89.30587144190069, -92.90590394398903, -93.63083388385274, -91.8644929119412, -95.26924857401164, -97.0710469181336, -98.01148078956652, -99.33043660296804, -95.58776817681839, -99.9570097527269, -101.45494093095093, -101.51838334751548, -101.00386616525799, -103.01963069818913, -103.20223925731209, -103.53783076500916, -103.48065647812659, -103.97797518531912, -104.58942778240602, -104.46991277190502, -104.59813972158683, -104.56685024229951, -104.69893799348945, -105.05669000016238, -106.17061117835001, -106.43303821862656, -107.39468286383597, -106.2899368267905, -105.7863846168199, -105.17170638885071, -104.53818172761852, -106.70340956723133, -106.55444321137247, -106.67654843051936, -107.79888413750199, -107.86424326005849, -106.09722609215336, -107.71648639013972, -107.79500725395155, -106.17330953637067, -105.43663624517525, -108.04970689199158, -109.92106271611999, -106.2505251183406, -110.60221373795562, -107.11377887451098, -108.4126937286195, -108.37794745021417, -113.22457316369011, -106.38281814065472, -107.55385617652075, -108.93026538982782, -106.19334142366085, -108.90462602264525, -107.63084712174981, -109.12192537022624, -107.90627042480016, -109.44472079190832, -108.91731458372392, -105.74102972706788, -105.74407510394178, -107.5989477192235, -106.2838630137392, -107.46190542725505, -107.38881299750702, -109.08024783239452, -104.97871836903269, -106.65424712290651, -107.04966019632134, -106.16202578092883, -102.98374199247179, -99.1568704142098, -87.07383781389657, -96.41471411313154, -102.65176579899618, -107.65674867775193, -102.85397890306213, -107.58658613411464, -104.79044898833125, -106.65282019869865, -108.65027966345534, -109.46169054950127, -108.69969979291741, -110.4048706652988, -108.81020193837274, -109.42808902484134, -108.85398463561398, -108.3849716744813, -109.1844457168716, -109.32787859535676, -111.01992124870878, -106.64843449415699, -108.9926343573667, -111.59837822080355, -110.57121677672183, -111.17280164669164, -110.68901970586144, -111.69013245592781, -109.90200577018311, -109.3554172126163, -110.7515368822992, -109.2863324212524, -109.66209701262974, -108.50795548698007, -110.58126481096504, -112.36093896766921, -109.78612141282203, -108.85120530917233, -109.91424431080952, -109.84698632196245, -110.93960894966105, -109.77214706089354, -110.30762971422381, -108.77791302937449, -110.79522659679036, -108.47242514643455, -111.20629758187835, -109.05996769621125, -111.13574821570619, -107.79388178889101, -111.5768481279296, -110.52058839597171, -111.58729762739313, -108.99000864386126, -111.6585121505227, -110.50715371958135, -108.87151956974363, -110.30486244367107, -108.32392040018144, -108.1769507919999, -110.43198471512189, -109.81454097966842, -110.26717009815644, -110.82924135076777, -110.34103661156989, -110.0692667126265, -109.34555682020833, -109.1694484721415, -109.9940980324044, -110.81940616215803, -108.21162003366862, -107.97087538330561, -107.55312461506225, -110.60339321606872, -110.09004629292225, -109.05860430198882, -113.1412749514818, -109.81628200948371, -108.62343219429849, -109.48172424209761, -110.85978755785311, -109.47778611557064, -108.81728552967951, -107.47864241666747, -107.61735128422292, -109.62511618983821, -110.32417726356636, -108.24287897478176, -108.60460879530194, -110.2181558494026, -107.95550802888957, -110.80234484950323, -111.09955733353904, -109.43923052503506, -108.98949130235951, -110.05778199870154, -110.36224432927585, -108.13523430027999, -110.681114579241, -110.49106131529867, -108.73493328004297, -110.07663907252234, -109.9968931372618, -112.10715231091008, -108.80994125105168, -111.63774865669372, -111.54355694032755, -111.64024217585788, -109.34986300492378, -108.88053713185408, -111.14370830146245, -111.17327416167232, -110.36311492990576, -109.99414559884396, -112.96912007380595, -111.43191437097785, -111.71327312809349, -108.77202323682606, -110.25970374932486, -112.59574277180732, -109.77247894866957, -110.09219852365874, -111.7197662726775, -109.85454092697009, -110.06789440397942, -110.38055758638309, -111.04251386932805, -111.54279434240568, -109.74385329575985, -110.98924544863415, -111.17898077762852, -110.98364252730245, -110.75024385843372, -109.24766708578407, -109.67753987004863, -110.6537235844391, -111.84436313010086, -109.12654337292446, -109.65519521121124, -111.1845162935778, -110.5009101465602, -110.22980642268818, -110.88540043278346, -110.29249073109453, -108.80459864528464, -107.49372141121728, -108.50353962704821, -110.00730069533373, -112.012876492648, -109.01283702976382, -109.07442203290057, -108.2961442983685, -111.60962842680907, -108.84312815413224, -108.6276642979969, -108.75132871638827, -109.30004903844721, -107.20359872252604, -109.12175943862074, -110.43914247337625, -109.55954680842791, -110.37116786618797, -108.55907813251434, -110.19249995041955, -106.95269845697632, -111.07027929458712, -110.1073996792702, -110.61729280468039, -109.6419175310234, -109.47995019876329, -109.66602827275211, -110.01953864498805, -108.45989120418268, -109.79778555296474, -109.94663827736616, -109.52410616839379, -110.58014441463794, -110.09182359045897, -111.0487262011397, -110.49609187214915, -110.6114701312941, -111.17752423063314, -109.74965389041003, -108.58973724447526, -108.84292130035902, -108.90689510645983, -110.69840140049361, -111.30494362640982, -111.00224390075273, -110.50848328538423, -111.59232911931113, -109.30826761863756, -108.44510893127558, -109.63744704504391, -108.95037574307332, -111.36486409910674, -112.74508631930381, -111.03952454593811, -110.57133212903979, -110.59969855145111, -108.25570461975128, -110.44617635200193, -110.32190307214704, -110.95204704643322, -112.0595421753479, -110.45342552693265, -112.50183987758867, -110.08217804938009, -108.90353583389084, -107.02032313792242, -88.3334978919524, -107.92027625495886, -109.83148570028482, -110.30427997450572, -110.92855407802753, -109.67404674397338, -111.03606345823586, -110.58277018943096, -109.77692362669393, -109.39170901729935, -110.20711662408928, -109.41601946806779, -110.34213214925832, -111.2283900972803, -111.51682597931386, -110.47069117801351, -110.93808974285523, -111.11277478000933, -112.50698886748012, -112.12918507523611, -110.46316790252011, -109.9387334819968, -109.78723249688426, -107.13037722044297, -108.16132376075751, -109.07255491017162, -108.85068428558272, -110.28038153100799, -107.77611023481016, -110.69754506886444, -110.09495581837979, -109.21214884561816, -112.62718526248648, -109.22048725312992, -109.17793923163308, -110.87372121410577, -109.71902632604333, -112.61041177225496, -109.6374750969677, -110.74738952366951, -108.93404661877067, -109.84938675700889, -112.25316361679832, -110.30788094875312, -109.26929069321925, -111.20853536783942, -110.05212566057608, -111.72448131932816, -111.55474439772887, -111.81988954424324, -108.44452452934028, -109.21897824914645, -109.55634869894358, -111.36318572800242, -110.05777399011298, -109.64458567712875, -108.73315084760529, -108.93332091319675, -108.4816455312154, -108.80120578498936, -108.1804470361839, -109.7177707524778, -109.31977709844544, -109.33603116022124, -111.46120546572519, -111.7480378245176, -109.17907150677627, -110.47970652472505, -109.73718750984082, -109.7935026884937, -110.40458408612054, -110.91781389491092, -108.39352075861481, -108.27512197925346, -109.59155075404814, -110.40183121737397, -109.25423373270381, -108.37769008625712, -107.91335995938509, -109.5576520703013, -107.27392145737491, -110.98592762117059, -108.41809950647861, -111.48163889400448, -109.70961684769624, -109.22952568656495, -109.76504719131209, -108.86928627177666, -107.97855299877004, -109.8412204399902, -109.6690048999326, -112.28329030175193, -111.54977099314607, -109.55689540119126, -107.93716711232997, -109.84247640855929, -111.5098351445789, -109.14317615215809, -110.28319116384824, -110.57901069942578, -107.2890252845352, -109.66754569546274, -110.15708115946433, -108.83782190109405, -111.60783857760667, -111.46884385151185, -109.21985333366634, -109.63605494317056, -110.87999187262697, -112.26992029775087, -111.05491095860552, -109.22795442529183, -108.99135781712076, -110.46475190704264, -109.35746113713218, -109.29125989270668, -107.40922407684049, -109.24391685563656, -110.41554602144217, -110.68952735085914, -110.62457364102458, -110.39856310555466, -108.84256124354566, -110.01614601335088, -109.8071306678428, -110.2804500736802, -108.76205061238203, -110.3962440297242, -108.98253716257014, -109.32990745926702, -111.17276766165281, -110.41113652364085, -110.36616199963426, -112.09767002991742, -108.43599666470733, -110.91876588140981, -109.05329272502944, -107.07198690769708, -108.72934463903034, -108.6666471996132, -108.97529973794413, -109.68895260146817, -109.2658844652487, -109.75690097249196, -109.38585024123027, -110.17593039468063, -107.87223111061134, -108.15261097418302, -110.09277437980633, -110.8665497655964, -108.43061614348413, -110.3052458526819, -109.22446919161898, -110.51909692711594, -110.06620699121913, -109.53439413051383, -110.31952463872884, -111.4732125902982, -110.41443606663168, -109.9579358088152, -109.930778061577, -108.5473214465574, -109.34719220288939, -109.16964653934396, -110.04824158176345, -109.42616539603762, -108.3556027482992, -110.62331917617789, -111.3652147859356, -110.12362012120938, -110.13175448595814, -111.20110099151856, -111.50643914621541, -108.11659117128028, -111.06037600347967, -109.03822892917451, -108.25678204604324, -110.82608024151122, -109.15887945314851, -109.88255674562845, -111.18322672526185, -110.95836040044516, -107.91535345885436, -110.66285812468733, -109.61906549925033, -109.58059721670746, -109.65198009505977, -109.65950565672951, -108.95264505276342, -109.23343669003113, -110.74308548011575, -106.39170014998685, -109.61471203101753, -108.24258770956924, -109.84609566640096, -107.83834185503922, -108.93052854090027, -107.55568820082641, -109.758551082242, -110.65892780872205, -111.99907420485852, -110.71043004141137, -110.62257237494617, -109.15610413532767, -106.87403836327807, -108.19175324576331, -110.27819583792918, -110.23918003777561, -108.29703377268754, -110.07182881114713, -109.60256111108491, -111.00394752430006, -110.30750337485472, -108.78309624082331, -109.24103013025798, -108.76979253891403, -109.91618737478264, -108.83915940855513, -110.92536150834754, -109.72250903746432, -108.96533939688658, -111.08949280651164, -109.20335070860871, -109.37826578362439, -109.77953166722301, -110.1867310744785, -110.07114559821346, -110.7003631567182, -107.86455899696074, -108.94113264174617, -109.35999427135138, -109.33627364788704, -108.96588828808375, -109.08716536982254, -108.73575375369026, -109.47770132070654, -109.83726171472907, -110.73516506891792, -110.56827134787686, -107.65667508354096, -109.30200115708924, -109.28406803847896, -110.55374624323233, -111.2017766725333, -108.50851279608973, -109.79494403619485, -109.08320018013063, -110.21850624918747, -108.4652936555984, -108.74837610538873, -108.81326140648238, -108.83830180036702, -108.785270477003, -110.01845876259073, -108.76030368637825, -108.57879884880157, -110.6610608456059, -108.74669367794318, -111.55956030460833, -110.22906685783455, -110.48411613865359, -109.48060880085136, -112.77556331479562, -108.2676071206087, -108.8571136162698, -108.56944905160177, -109.16406757131058, -111.42259299295839, -108.25216316582294, -110.48487127684025, -109.69532331373831, -108.13992755196784, -109.2987762526628, -109.82536192480795, -111.28650061088359, -109.12820736404241, -109.37960655471406, -108.96014976926716, -107.97535047619023, -112.31953123574708, -109.06198330523004, -107.52722515967098, -107.31555373665437, -99.89671790804692, -107.44442600896275, -110.6549218761941, -108.02265794322076, -109.63582761762919, -110.00574746987859, -109.51565124961209, -109.3550083591902, -110.4541529175301, -107.85799722437162, -105.1197113090786, -110.25038075579738, -110.39710812865657, -109.3618876098789, -107.6131301952152, -109.21529527621463, -108.7995754403799, -108.48347353145697, -106.45678488065816, -109.60427918561142, -110.81194387812535, -109.52215044127382, -109.88751598659705, -109.30205143590227, -110.74984456751768, -109.03952092986351, -110.69170786328897, -110.39236248162467, -108.65456161733339, -107.60439764386904, -109.97367926606955, -110.2754359970249, -108.81546418006434, -106.99691398176165, -108.42047325825182, -107.24499915944605, -109.28116135603187, -108.70650358781573, -108.05516916105047, -107.20893100196241, -112.07029265690055, -109.38099990478445, -111.53461820465232, -108.11312509555277, -108.76714028655223, -109.89565008459624, -107.71879172001115, -108.08434857420214, -108.79142773619792, -107.25153085963885, -110.05595039449301, -109.31604222314259, -109.94405791565286, -109.04715370361387, -108.89278831045846, -108.84682466376424, -110.0067927716526, -107.63768959294084, -108.98109382020348, -111.4720219575084, -110.76023788797733, -108.78599647633777, -106.59726674064618, -108.66715709719243, -107.99134359630926, -110.11396713841884, -107.21091759882775, -108.08576824949941, -108.80217666857972, -111.72949572713338, -107.33126296136014, -107.33731660097102, -108.04470462977443, -109.42963925921418, -111.03517778720736, -109.55293581015796, -107.99948151285162, -106.59480934999681, -107.63777243313498, -108.96490626068824, -108.8948210299064, -108.30870516747477, -109.13612869658097, -109.59971429402015, -110.2571461001396, -108.7655464686992, -109.81144209568883, -109.80796806645141, -109.20948481699544, -108.68653880881129, -109.26329796696166, -109.22428132233863, -110.12571678351438, -109.14615461144786, -107.08261621308327, -109.11338327144382, -107.75421565039201, -107.45291780756361, -109.00477000647248, -107.41031480478154, -109.98948062864928, -107.45953654921264, -106.37522884807879, -107.7786128523167, -108.03610987358499, -108.05926797128022, -108.59400205554164, -109.89620453365603, -109.03811240487515, -109.96909236705363, -109.28212981785472, -109.6772152101994, -108.26493868190678, -110.55558039199732, -106.6252818398841, -110.19075011176416, -109.56520012524705, -109.8023423576176, -111.2697570480663, -108.26752571816566, -112.00337375484828, -109.85709226796116, -109.36922081321148, -108.8424844298318, -111.2512302139209, -110.61775974680471, -110.22501328999012, -107.76874906708105, -110.71023653476604, -109.4025656165291, -107.66667684986125, -107.59759854092948, -107.94763263251238, -107.3888591871119, -108.62692803125044, -109.18012867988286, -107.78662871481455, -108.5072814073944, -109.50348958982907, -109.95177634938378, -107.78756251182895, -108.03865042797304, -110.1814993556385, -109.34937567548833, -109.52162025123161, -109.50819015441117, -108.20953105254624, -110.52154040214435, -109.3324404469266, -109.2696617050831, -109.54675609195674, -108.5940367000989, -109.40184828664549, -108.2518305610941, -108.55972691669434, -109.03647225394408, -108.48166656251695, -107.42023429066523, -109.42453054302521, -110.09532345960083, -108.78315822119662, -109.97508586102265, -108.22687406536997, -109.17110028890058, -110.15390449992647, -107.88577458651508, -108.28851074361447, -108.52030295163331, -110.03496861709483, -109.40014319167584, -107.73048113044877, -108.17571683963915, -110.34839852994926, -108.55894048192191, -108.74107339998285, -111.17734138993401, -110.22946440841412, -109.45511941802884, -108.0657300641843, -109.33797363184166, -106.95974095511333, -107.93068343723691, -109.78867669512647, -107.2087297624043, -109.542665021243, -110.05035859052961, -110.30235238883523, -109.20586170783808, -109.2796396673401, -109.14260673746566, -108.22019460542734, -109.99011886871159, -109.89103038547285, -110.36964772493243, -108.62340319923602, -109.06779821699769, -109.21830861066148, -107.7402395759509, -107.7178850938205, -113.45665085929117, -109.24039191621704, -109.30387033426037, -107.61849760982835, -109.41430582703529, -109.11482836392241, -111.89328423764577, -111.84653367963301, -109.00674896486915, -109.84488648739638, -109.41914760797953, -108.53442910169935, -109.66883322968232, -107.68762956301386, -109.82583101109167, -107.83405397804887, -108.78052031141966, -107.37842078941692, -105.40843158543845, -108.81430898189338, -109.57374640194516, -109.41111270322058, -108.82621700188898, -110.2552502368822, -110.23903890097205, -110.52171662278697, -108.21249857906324, -109.97268479379733, -108.20088823960992, -108.85682002802234, -110.11642849164285, -109.94087886999255, -111.63180946270296, -108.20899499456195, -106.73341567332112, -109.90003508676807, -110.14688274481229, -109.62259307329889, -107.57811196819495, -106.88584597822792, -109.16132624528932, -109.78677836397806, -108.59319344451784, -108.55877448618652, -109.46883711353044, -108.47309455543844, -108.09487065732198, -109.82219079158135, -109.63780237877428, -109.28348848877269, -107.62893405379826, -109.46986737961593, -108.03089712610223, -110.3931917410696, -106.06970126043262, -109.41866550703786, -105.31710372440419, -109.20218082282653, -108.28467118008108, -108.80026326744611, -107.40729224715713, -111.07322915141532, -107.1057186510818, -107.98286374205958, -108.51298722989311, -108.69632670891366, -107.96509231988331, -108.15882223414738, -106.85862416470376, -109.70705792539056, -108.64519930633055, -106.78708421443504, -109.43552377900174, -109.4474526498122, -109.10135248755788, -111.43316642580763, -109.33457343739448, -110.23547887071898, -108.95690647379442, -109.21159903769149, -108.12969562680841, -110.82751409340537, -108.55724349027832, -109.8796329603075, -108.50369978374582, -107.43145467247209, -108.60003323209516, -108.77155705999647, -109.33806063660796, -108.37500858898439, -109.65641721611547, -109.81905873737344, -108.03483220769625, -110.48028107566635, -108.60527372219985, -109.28768201151478, -99.8804125587218, -108.8913334544964, -108.23534920737794, -111.07646463287153, -108.59029790589766, -110.3405916586831, -107.66387718565608, -108.73793152614131, -110.61440166477816, -108.76211382544581, -110.23236978486065, -109.10669297094852, -109.15247609779597, -109.00539004923506, -110.14424353412238, -110.55445060661157, -109.48721312920799, -108.17040942305823, -108.77592227268228, -108.77130256578067, -107.82494496098512, -109.57266989523707, -108.75767497229612, -108.13688624150026, -107.8280716764963, -105.676279602552, -107.6370316684844, -109.73508547021689, -109.25365178573009, -108.86767843317584, -109.70969944273735, -108.91917504090888, -109.97734866522867, -112.17308993943783, -110.28356299479682, -110.7927103729386, -110.30837645846702, -107.56364161860179, -109.50188349731121, -109.36065627483853, -109.75389877587511, -109.81713476007774, -108.14524057525358, -109.43832376796216, -110.89342891210596, -108.15657882822792, -106.84106061627887, -107.83091759905821, -108.61794662682962, -109.57142366843581, -109.85402645528154, -110.12877022469837, -109.19414429724044, -110.56168468006764, -108.74720588273881, -107.90448559921305, -108.54421401507743, -105.06700039841249, -109.17937358052484, -108.94317576365822, -107.79410219455083, -109.24955437598658, -108.23334395173994, -108.98759227946937, -107.05986359444529, -107.20956512998849, -109.00295831471958, -109.43119556916457, -108.93348410522628, -108.99932477701081, -106.6448790859128, -109.06877251308666, -107.67053918439544, -109.15052780608639, -110.16878033319385, -106.55101141640301, -108.02811045752685, -111.52173447126572, -110.16854119242062, -110.93164036911654, -111.25979320890855, -108.82629030379024, -108.52004501839738, -107.09697056562636, -108.94233383169858, -107.37962568194772, -109.1239201710643, -108.93949898577122, -110.62573772949195, -110.09592372075662, -107.56136391005947, -110.45600430869621, -108.79481000016084, -109.41462449554598, -109.30248158488335, -108.70735295493108, -109.9174743694956, -109.94232543385962, -110.71725446170196, -110.0346196158573, -110.34814317845934, -110.6651078322521, -107.55409880424479, -108.71734776861287, -109.50902203986271, -110.40207542979611, -108.7847687630861, -111.10599488129682, -109.30824728923263, -108.20134064331717, -110.55959112431609, -107.77099734327174, -110.23862843385446, -108.48520797666865, -108.54205896654946, -107.79288769037599, -109.84022250170581, -108.02758364115576, -109.35132492327935, -108.87009749667932, -109.86905123364855, -109.19826752168308, -106.835240323691, -109.37910022114056, -110.80633973102931, -109.12703823829597, -111.07432699570984, -111.8064506085314, -110.09349947650527, -108.66467295777367, -108.75119108236053, -112.63983351316729, -110.90940743670113, -110.27973159222081, -109.57141664526549, -108.61645363771719, -109.31742355616147, -109.5839599160637, -110.01188998365383, -110.01923429741011, -108.94779759137936, -108.26169431000017, -109.24553201026085, -109.95709526422822, -110.68677343596859, -108.7678734483002, -110.47090469179284, -110.31604700116512, -110.10256600741997, -109.76634647265719, -110.8830805828562, -109.94609564072982, -109.20662382740542, -108.12492970530919, -110.5274435478767, -108.02351960398035, -110.6264936805739, -107.14559226383577, -109.13821777857531, -111.05324489472586, -110.15190797512811, -107.96366234783144, -110.03950681967147, -109.17476300510336, -110.41251816187909, -111.39219865477246, -111.32530426869943, -109.97369363558423, -108.98666403063845, -109.62049358645565, -109.58130494498671, -111.72738873188874, -110.39825891106616, -108.57430325757545, -111.28625510212446, -108.77421250595326, -109.75025415031793, -109.51948456745635, -108.82129398637998, -109.81362137198361, -107.86292494316123, -107.49318292857053, -109.66948564589373, -109.54288390056654, -107.99912445612077, -110.3497559614379, -108.00549349666127, -110.01361420523357, -108.4977916421456, -109.67078387286976, -109.85678367732866, -112.01237658746248, -108.4855625950998, -110.84880875737286, -110.9178674382154, -110.44187536727453, -108.75076921971127, -110.04946286646651, -109.99780941000827, -110.14242932305507, -109.56343773672316, -109.6278993388131, -108.77419573790174, -109.10543670530926, -109.7801848627463, -110.30733124104881, -113.13440550301436, -109.32709134514755, -109.74136656933283, -110.01525283266193, -109.43924662938396, -110.25325289253, -107.75460576671303, -110.60057027395933, -110.71458404922404, -110.15788509050662, -110.69167485018224, -110.96006652476157, -111.01156633983031, -111.6058448010008, -109.51364005052672, -109.76058205940885, -108.43421621088261, -109.47973949170208, -109.25533250208288, -109.47422603921065, -111.36411644613841, -107.27566171102698, -110.45098686173688, -109.93589296291184, -109.03803734663714, -110.53118128434016, -110.2408872254969, -110.0532234862915, -109.94185495614619, -110.2662004220774, -109.51094016962288, -108.5210104215432, -108.13691752270934, -110.18460088390265, -108.32609309150783, -109.89652230508281, -109.80923900768477, -109.01917388968883, -110.01248300968739, -109.43415605440147, -108.09823485138017, -107.40637725320931, -109.40632232658412, -111.97981999127656, -111.16609811629485, -111.64500793960192, -110.99793748693381, -109.55531276386903, -110.2535662621666, -108.17429802469516, -109.09425673355422, -110.23187110421917, -110.55358397926925, -109.93461124753053, -109.55604345832225, -109.44569510408274, -109.72185151080762, -109.52963702944834, -109.2303630328152, -109.74819502244243, -109.3932530349457, -109.17096788339686, -110.46153727064616, -113.1073731246639, -109.43753070459397, -108.13332547768168, -109.42294574929969, -108.45798401969856, -110.29453435046327, -112.66249403705643, -108.78314667434937, -105.9634478773668, -109.14327524669528, -108.50645190860273, -100.81571594994128, -104.4482859840643, -110.68926237051092, -109.12362553230196, -109.45234390564677, -107.91461416156068, -110.67788819353727, -110.05744935668449, -111.78333392154664, -106.83628914455993, -110.11115457346548, -109.13434608275826, -110.80006861194663, -110.35323502651462, -112.29149906501372, -109.01656376530778, -109.30871662948859, -109.79736315392456, -109.17848983603582, -108.09752397056482, -111.6039030763455, -109.27008844877828, -110.84475733314184, -109.72393917557073, -111.31060762894991, -110.78858793807466, -107.12841545099752, -109.54510865218204, -105.2805426080281, -106.28514149354733, -109.50656759582803, -110.14700878401054, -110.49737016725709, -109.19811547071924, -109.92527399676051, -110.7961615015146, -109.7447227818197, -109.49432012009893, -108.714081576733, -110.09766801550917, -109.08448507943001, -110.36154838733857, -109.86328656267403, -109.21144237434696, -112.4145136888034, -108.57567151011159, -109.66748589540896, -109.72985837578446, -109.29989238126763, -109.85868902806475, -111.01778182304162, -111.23625326328558, -110.01270868104203, -109.27067928081415, -109.71171312410247, -109.28697459293629, -110.67868067201007, -110.91353786857455, -111.21479955051575, -109.11315965407708, -109.40418681804496, -107.80511819596003, -107.37201025889816, -111.81969609169838, -109.89875624306032, -110.29328043898657, -109.74853280072202, -111.39527865400605, -109.47746221101964, -111.75141177452517, -109.31325306583483, -109.30117448911659, -109.3997781364162, -109.45356931295724, -109.60585285774386, -111.33951689512735, -107.74187210470228, -109.62706021606415, -108.72139655505221, -109.79552836110567, -110.64354037499807, -110.96138240913136, -110.02215059889615, -110.92978442698893, -110.0620778287114, -110.85019647293322, -111.77397403227091, -109.81257196800128, -109.15643451383403, -110.72777566469594, -108.7463769025616, -109.80959395914073, -111.24500986151126, -110.48863498350322, -110.30863780110901, -109.79331354195703, -110.34087081762074, -109.45183222569266, -109.6440990067103, -111.15034876658994, -112.14912485578341, -111.8886180186196, -110.57054820211916, -111.07556239924551, -110.5872832735073, -110.28912501038172, -108.91501133754849, -111.44575118962761, -109.90799859177967, -109.74421995550023, -108.70941446115883, -110.28822893097275, -109.70039554000401, -110.33701797570251, -110.79445894683306, -109.57694314608153, -108.816904416038, -109.66517126767175, -109.39501469321644, -110.85775022889956, -109.3689402795614, -112.09107318723095, -110.67985626248422, -110.32971146814747, -112.08166943494875, -109.93955548712543, -109.31722953035252, -110.2062913031861, -108.22565380081006, -110.680898028151, -111.95386604441454, -110.83354130587097, -108.5873626748948, -111.97536144124408, -109.23944159551515, -111.57859477689586, -110.80135186615524, -110.4800953731021, -110.14040729648133, -109.25873050390551, -108.87000960474569, -110.97091597211167, -110.15787270199012, -111.62434537618091, -108.5421625277294, -110.42258666403919, -110.96896115868603, -108.98253068925274, -109.54245055160168, -110.28051096122468, -109.48060498658319, -109.77618362117276, -111.64513838754992, -111.13945484239875, -110.18094280356001, -110.43757222770748, -110.81588360154201, -110.11656805555333, -108.47936291282355, -109.16476249859961, -109.3549985917136, -110.77753190334253, -111.46065694661178, -110.40387985996301, -109.95673803226478, -111.58660981285446, -108.59894875229345, -109.37333363882607, -110.26849699991793, -109.30500469266264, -109.23789020998296, -110.82000706486865, -109.25927538839868, -111.03285659417519, -111.08899832832414, -110.69361682858042, -109.45187168573815, -109.9614018482838, -109.70209527974106, -112.11903952100165, -109.59713611623246, -110.70292028698111, -110.12743849746808, -110.63315585514292, -108.60450276298175, -109.32832664986026, -109.99753023477764, -109.46644696130294, -109.1781290160558, -111.58830180575129, -111.67229040267557, -111.3750024136205, -108.33616679452298, -109.99797067800029, -110.50892429124391, -108.66074740829372, -111.17094662568759, -109.87538933985836, -109.152526628291, -110.44623159817101, -110.21603106403009, -110.64376935639365, -109.36897426842583, -108.67303022227141, -109.89327693080823, -111.50442955563923, -111.37532237834381, -109.38132821290205, -109.73509680539144, -110.53918379735906, -111.22869870340647, -109.39977573957616, -110.3674665334106, -110.5366125953241, -109.99025356764304, -109.97300035646616, -109.87631077033762, -109.64608829594286, -113.02486102973394, -108.26250283140733, -109.62234918138763, -111.18766216512655, -110.33666026406992, -110.5808115327039, -108.2971671321189, -110.10964334161903, -110.61254021379767, -109.89852549557533, -110.16562049054073, -109.41433790018287, -111.2453823439446, -110.45554802599901, -113.11454453784393, -110.7333866145056, -110.00858191882439, -108.54745315874294, -110.08430415376903, -111.9006972727596, -110.3031506154679, -110.26331790366497, -109.36797925566673, -109.04860552478912, -111.83514212681175, -111.38960737633833, -109.01429665187288, -110.96404839103826, -108.95488871107163, -109.09652004914592, -111.884304581971, -110.57566691021339, -111.95113404442795, -110.13677174050159, -108.10078686353354, -107.69442565416006, -112.42676605669463, -109.12681161784135, -109.23120766087519, -110.57649395555585, -110.22143082743162, -108.40065951773644, -109.46923168308618, -111.39095086729745, -110.46375658526013, -111.45145283328486, -112.22610823637353, -110.61090190564383, -112.22250292674809, -111.7379343196361, -110.18530386733481, -108.93867365671692, -111.89304844956082, -109.06146134986984, -110.98405731832798, -109.76366821333497, -108.08326795663608, -109.95041147835065, -112.94140614324155, -111.79814935135965, -108.07337559063119, -109.13733403265212, -111.74906646037496, -111.12228668433455, -110.02899450462209, -110.22237716929811, -109.0224776891049, -110.18135850497721, -113.32516073881047, -111.3576490243877, -110.60510094465171, -109.6935518470342, -110.36313473154901, -111.95933240129618, -109.49625308071019, -109.18827910216122, -110.54311407822692, -108.4811035913567, -112.81280225723607, -108.86530665787413, -110.85796435061886, -110.40059714639627, -108.19250716343407, -108.96956521802292, -108.61281798886506, -109.78061525370413, -111.58885511891798, -109.06279169160345, -111.43043988466789, -111.63169336321079, -109.54702536206447, -109.62860636296405, -109.47865811135546, -108.02265793654806, -109.97461304995515, -110.72549884050886, -111.57309413919933, -110.03317891949746, -110.39570411598524, -110.27606115470397, -110.63294457306095, -110.71821689302902, -110.38076268941819, -111.51223508887897, -110.40703572670697, -112.24933273737743, -109.74954300082398, -108.46020292937696, -111.05315219575881, -110.38635148390118, -109.58268303790976, -112.34211536832117, -108.45894118755307, -108.96463982695337, -110.56040438523046, -110.67803313671729, -111.07349872375121, -110.42184162876096, -111.82081126435692, -108.85923651136297, -112.57723799596502, -113.65690874668172, -112.62314325834605, -110.70357529341362, -110.959925221544, -111.26336183001875, -108.1350700630152, -107.94545932312926, -111.17610778209841, -110.20386728310686, -108.55646511121591, -109.8400922569145, -111.73466587035968, -110.47272877573613, -108.33011124048193, -107.93042857580332, -108.60928277989103, -109.25240966798974, -108.96403833602028, -106.94222615757475, -109.37086694261907, -106.72743097285155, -109.03160193412796, -107.3549903889451, -106.8543848510082, -107.83503929060929, -106.30745467433752, -108.36915807168845, -107.13065938379303, -107.84769200880969, -106.08004345082777, -108.15244601930225, -108.37254117816573, -106.57863034819223, -108.1283698227614, -108.19776505569902, -107.58283412238643, -108.17365133196301, -108.6794309781181, -107.91552140588759, -111.60122989270022, -107.04360635941174, -111.55535949001795, -109.39870426166594, -109.55937904851662, -111.81389508925734, -109.88957041098786, -110.84764586896561, -110.59130246272693, -111.15944135223884, -110.19496154041607, -111.51861903129362, -110.74798816525838, -111.37312965175558, -110.10842817220238, -110.73198099204856, -111.36708667993291, -110.30840247819665, -110.11744489669044, -110.55237850846444, -108.2073528237766, -112.70750856801911, -110.99917956040802, -109.84949484779976, -111.3403161887679, -110.08924435263565, -110.17749213365616, -112.10849123224503, -110.94270741299202, -109.29350963424746, -110.33477486966507, -112.19620157705627, -111.45484078395934, -111.86858843505124, -110.22491147345858, -108.96177661263177, -108.67862820579893, -107.55155410582937, -108.27984439169573, -108.72682528077233, -110.64231212183269, -109.32873093119183, -112.98564364754564, -110.78933114228725, -108.50921025910479, -107.91087245586935, -112.57350030929283, -111.75871577457525, -108.42095298945462, -112.31266064114303, -110.1295657579673, -109.67444664474456, -110.33749884929306, -109.16098218724147, -109.63554874360221, -109.15892392675141, -111.90580809179818, -108.81196712336858, -111.42223552606656, -109.90571484965518, -109.99739812086352, -111.64103850263211, -111.31463957090885, -110.61247447444549, -110.20960333715526, -110.1707327818923, -109.70412636554525, -110.97278093107532, -110.24386747740314, -109.81378546061525, -110.83784085086458, -109.77357954318757, -111.22663832948885, -111.14563050139252, -110.87152231402447, -110.34246044319893, -109.97174570657546, -110.23599592972218, -111.08206161770731, -110.0073315341242, -111.11748366902188, -112.04005964728601, -109.81290191679287, -109.68543639040858, -112.01143296194752, -110.13641850530031, -108.19348942447623, -109.7534468948808, -109.36697824644176, -97.56454580435337, -104.97829040517887, -108.1539132982256, -110.048991273122, -107.46172505860011, -110.49269280640675, -109.94209901400029, -109.38576869679022, -111.43699124347364, -110.89973083498887, -111.2994445418276, -109.25144782032437, -113.25676258473536, -110.82078737428088, -109.97779571182073, -113.36294799183014, -111.38584551238931, -112.17267897274873, -108.56430946159155, -112.06841286528645, -110.36822473102735, -109.54758527532016, -110.48190506674653, -110.03535695860182, -109.3951469796576, -112.41910682256774, -111.38124138857238, -109.37850389100952, -111.65544568836181, -111.55876881606889, -109.3029209617236, -109.20030046194076, -108.82610577621037, -110.53329453526098, -109.96090595542142, -109.67834229432077, -110.62303603007352, -109.8388817181171, -109.22430039793213, -108.92749786663613, -110.05794249283548, -109.58534943218437, -110.50493887507297, -109.96373022997366, -111.0645036323456, -111.28501675364454, -109.77386932343008, -108.8952247140968, -110.09242801628717, -112.90943444063141, -110.72299296247249, -109.39094335967056, -110.95165384057718, -109.59809519359453, -110.4978602309597, -109.67109981692639, -111.2489619905986, -110.0937750887109, -109.76771021128954, -108.32976315018955, -111.3058145792439, -111.09464974601362, -110.99797900696136, -109.174315000222, -109.630351559617, -110.26289147175856, -110.22688407202517, -109.96748050100612, -112.13247633583758, -110.59994952890855, -110.93023020153811, -109.22457750926695, -110.26162558926984, -110.09713110375579, -111.73858994918328, -109.78183160058515, -109.7603471824367, -110.96016892586911, -111.23309626937036, -109.83093663960678, -114.05354944347246, -111.58202863059464, -110.42281828744524, -110.9521484732059, -112.5120328206343, -111.614891937737, -109.84428787405484, -111.61119567831453, -110.43095563229411, -111.71833448430398, -110.01132196809407, -109.37558169247951, -109.14091380022785, -110.42663661754088, -110.3598013572826, -109.78207135281417, -109.94058843992468, -109.88210328447205, -108.6217811850147, -107.17834387173707, -110.6447226986756, -111.10704778101115, -111.24396771977769, -110.47849395539598, -110.75150631628034, -109.67662689396347, -109.23145032835053, -108.83780193265358, -109.43468321661163, -102.22521103859944, -106.90009867479111, -108.91580608784525, -109.58671397003187, -110.56692028436989, -108.75103142680105, -111.00795573084157, -110.75039085328763, -109.48222099288613, -111.8621134816908, -110.26507966786443, -108.885924716389, -109.30841399453053, -112.3188631425597, -111.05677697153163, -108.8268571902449, -109.63028152237679, -114.82339015806369, -107.03435216376964, -111.34847692589166, -109.61354114874855, -112.32687758049907, -109.59816404231358, -111.64248480241805, -111.84075757907273, -110.44017657636552, -110.15181635726277, -111.93813663582833, -109.11826378836209, -109.99779889778326, -109.927119030584, -109.4389650887841, -111.52448814187727, -111.38736268499642, -110.51920914917922, -108.64230614681055, -108.90307263595304, -110.57246891832371, -109.65575340646116, -109.80359672370373, -108.83368585528197, -111.09385004343437, -108.83430005497769, -112.37784208819113, -109.50005381621696, -109.67421750136593, -111.39664088797532, -109.70867599669316, -109.52498993629875, -111.12341349673187, -110.0484037026941, -109.55138667646308, -111.06614422098669, -109.4785941493091, -110.25724082617013, -110.93950616855716, -110.53487953881397, -111.45722057988401, -110.32393446412904, -110.34361936710438, -108.6610336097813, -109.53631603696368, -108.06930707969195, -107.68056561368934, -108.73860971027449, -108.87111384617579, -108.40433837098611, -110.55999576884835, -106.83832061167207, -108.28786975902513, -109.18482905697472, -107.81071696594883, -107.91047268802457, -108.79613111673706, -111.05361322310213, -109.97897453479862, -109.12920563729425, -111.20538391490288, -109.26286135293664, -111.31400407177502, -109.92167984752287, -110.70854322826071, -108.59406515713611, -109.69371333227458, -109.36664873267313, -110.35521729513704, -110.40667924006368, -112.0181844636846, -111.01529188207431, -110.59246505728431, -109.95068312717868, -110.75807466894047, -109.58596443762707, -111.12127793384956, -109.59041634463125, -111.56255571372793, -110.43405578864342, -108.39660324329928, -111.1420710307505, -113.64788483868595, -111.67645688353934, -111.36878760365944, -109.68523694561108, -110.11608766310304, -109.25670490330123, -110.73546181099229, -111.77855039399805, -107.9662794718261, -109.67483334602832, -109.891258579519, -110.24757768183042, -109.50202895993814, -110.07763831916637, -109.96891925839451, -110.97268925927641, -109.31698133827767, -112.27933593506792, -110.36206721075725, -109.47379463718867, -110.27836850941338, -110.63738280998388, -111.3611682777485, -110.72689155959884, -111.55480904927032, -111.16689658479412, -110.35555645743601, -111.56609319131051, -110.88279459952174, -114.73607246523177, -109.95813757295693, -107.64639932425493, -111.26486783320321, -112.03946356928121, -111.8915972448334, -110.35245920812773, -110.83155104803564, -110.67437747473863, -110.9959682920065, -110.7815352345103, -111.13722283763049, -112.54797265493127, -110.06894780898469, -111.65186554925783, -111.83545188116254, -110.65894756123697, -108.48458025065264, -112.43760714427981, -114.1368408201927, -110.40065777895025, -110.1066998945526, -108.60654239598591, -110.5716060205154, -110.74257357180736, -111.1136089342442, -111.53539811075092, -113.2559601458872, -109.2003227548348, -110.42285840441025, -111.4086884998834, -111.61503050693868, -110.8194303494779, -108.9701587059964, -112.58521089509063, -110.10873915265242, -112.43440038319561, -110.03468788439882, -111.57896603236308, -110.21939233582523, -109.03614470500777, -110.11738923539659, -109.55359574898291, -110.416473622654, -109.4626868574157, -111.17164025076731, -110.3579689035081, -109.04338716157822, -112.36157114517567, -109.32125615922843, -112.71105693789394, -110.11019129547768, -108.96439402555632, -111.107663418839, -111.48306369859839, -110.9317530461794, -107.98628540532181, -111.1636972328743, -110.47837837583148, -109.04649309175733, -110.27110334963734, -111.35803630614352, -110.77259078859605, -111.46352820533895, -111.16789261049541, -109.2376344776325, -111.6795794983659, -111.74292205167644, -109.40835022991612, -111.02163652600731, -108.79482078001607, -110.6718658416566, -111.08747067599332, -112.15383726791498, -109.47049126158717, -109.061574046483, -111.23993049318979, -111.02521156588335, -109.46012868444186, -110.13918914826291, -112.08180381836377, -110.61929875223015, -111.4424805369965, -111.43420275069585, -109.71347556238717, -110.24726273025648, -109.7860268673935, -109.94126895018422, -111.41948668868926, -108.90555991781676, -110.81242861886172, -109.65007052722677, -112.12672329335953, -110.01123170946096, -111.13980448279096, -113.92013682657084, -108.6000853867411, -110.66793592761913, -110.61237681642844, -110.00839105230496, -109.38083187034974, -109.46119372195675, -110.3708067287448, -108.55518656223285, -113.33935987443276, -111.92184778392033, -111.80820718236087, -107.36852757311246, -109.51077803361602, -110.066791721019, -108.756710558672, -107.91391289865918, -110.72851430959301, -111.39074956442978, -112.928843679455, -109.87348280521556, -112.21371750380071, -110.82495902297394, -109.94006136010094, -110.58757785050143, -110.2790091349881, -111.43884888223081, -108.09540986530712, -109.63783244641691, -110.19577975613292, -110.01690033746098, -112.75938920157155, -109.27158857362184, -111.19519821680541, -110.14381902425255, -110.45955291199236, -111.55660330002316, -110.75604254261134, -111.02122553784838, -111.6490091060193, -110.93362819419399, -110.49033159684308, -110.70789549836027, -110.41991882034145, -110.0264093421208, -109.18432746063652, -110.15292268755287, -112.40733942236504, -111.32869665965416, -110.95418667871114, -111.14291568823575, -111.75555369152653, -112.98146297069803, -109.73870744292117, -111.33806139459435, -110.18838799491355, -112.60408243005732, -110.26112648646833, -110.58257045107274, -109.75155437454112]}, ...(2 in all)]
  in  "FFT 1 Choice 1":u16(ring) items=["T1 Y", "T1 X", "T1 Sum", "T2 Y", "T2 X", "T2 Sum", "T1 FB X", "T1 FB Sum", "T2 FB X", "T2 FB Sum", "PSD Y", "PSD X", "PSD Y Sum", "none"]
  in  "FFT 2 Choice 1":u16(ring)=3 items=["T1 Y", "T1 X", "T1 Sum", "T2 Y", "T2 X", "T2 Sum", "T1 FB X", "T1 FB Sum", "T2 FB X", "T2 FB Sum", "PSD Y", "PSD X", "PSD Y Sum", "none"]
  in  "FFT 1 Choice 2":u16(ring)=1 items=["T1 Y", "T1 X", "T1 Sum", "T2 Y", "T2 X", "T2 Sum", "T1 FB X", "T1 FB Sum", "T2 FB X", "T2 FB Sum", "PSD Y", "PSD X", "PSD Y Sum", "none"]
  in  "FFT 2 Choice 2":u16(ring)=4 items=["T1 Y", "T1 X", "T1 Sum", "T2 Y", "T2 X", "T2 Sum", "T1 FB X", "T1 FB Sum", "T2 FB X", "T2 FB Sum", "PSD Y", "PSD X", "PSD Y Sum", "none"]
  in  "Compute FFT":bool
  in  "Reset FFT":bool
  in  "# Spectra to Ave.":dbl=25.0
  out "Ave. Time (s)":dbl=1.5
  out "1 Channel":waveform(dbl)(graph)={"t0"=timestamp(0 s since 1904-01-01), "dt"=1.4999999999999999e-05, "Y"=array[20000 elements], "attributes"=variant("NI_ChannelName"=variant(string "T1 Y"))}
  out "Slow mean":dbl=nan format="%0.2f"
  in  "Slow mean N ave.":dbl=1.0 min=1.0 step=1.0
  out "Mean Intensity":dbl=nan
  out "Sigma":dbl=nan
  out "Sigma/Mean":dbl=nan
  in  "Subtract mean":bool
  in  "High Res. Display":u16(ring) items=["T1 Y", "T1 X", "T1 Sum", "T2 Y", "T2 X", "T2 Sum", "T1 FB X", "T1 FB Sum", "T2 FB X", "T2 FB Sum", "PSD Y", "PSD X", "PSD Y Sum"]
  out "APD 1 Rate (Hz)":dbl format="%#_3p"
  in  "Tab Control":T4(tab)
  out "Stage Moving":bool
  in  "Read Cal":bool
  in  "Confocal Linescan":bool
  in  "Speed (nm/s)":dbl=100.0
  in  "Furthest Withdraw (MHz)":dbl=15.0
  in  "Confocal Image":bool
  in  "Round T1 X":bool caption="Round"
  in  "T1 offset_x (mV)":dbl=nan format="%#_2g"
  in  "T1 kappa_x (pN/nm)":dbl=nan min=0.0 step=0.001 format="%#_2g"
  out "Time (s)":dbl=6.12
  out "Total Time (s)":dbl=60.0
  in  "Start Saving":bool
  in  "Cal sets to save":u32=50 min=1 step=1
  in  "Comment (data description)":string="testing confocal setup"
  out "Calibrating Trap...":bool
  in  "Trap 2 (ON/OFF)":bool=TRUE
  in  "Trap 1 (ON/OFF)":bool=TRUE
  in  "Save Calibration":bool
  in  "N sets to save":u32=200 caption="N Sets"
  in  "Save N Sets":bool
  out "Save file name":path=path "C:/Data/110526/110526_022.dat"
  in  "Save ave N":dbl=500.0 caption="Averaging Factor"
  out "Saving...":bool
  in  "Stop Saving":bool
  out "Progress":u16(slide) scale=0.0..100.0
  out "Manipulating Trap":bool
  out "Buffer Status":dbl(slide) scale=0.0..1.0
  out "Overflow (data lost)":bool
  in  "Reset":bool
  out "Data Rate (Hz)":dbl=66666.66666666667 caption="Trap Data Rate (Hz)" format="%#_3p"
  out "Data Period (s)":dbl=1.4999999999999999e-05 caption="Trap Data Period (s)" format="%#_6p"
  out "Save Data Rate (Hz)":dbl=133.33333333333334 caption="Rate (Hz)" format="%#_6p"
  out "Save Data Period (s)":dbl=0.0075 caption="Period (s)" format="%#_6p"
  in  "T1 alpha_x (nm/V)":dbl=nan step=10.0 format="%#_3g"
  in  "T2 alpha_x (nm/V)":dbl=nan step=10.0 format="%#_3g"
  in  "T2 kappa_x (pN/nm)":dbl=nan min=0.0 step=0.001 format="%#_2g"
  in  "T2 offset_x (mV)":dbl=nan format="%#_2g"
  in  "BD 1 Frequency 2 (MHz)":dbl=80.0 caption="T2 X (MHz)" min=50.0 max=100.0 step=1.0 format="%#_6p"
  in  "Green Laser ON/Interlacing":bool=TRUE
  in  "Round T2 X":bool caption="Round"
  in  "AO1":dbl(slide) caption="Confocal Y (V)" min=0.0 max=10.0 step=0.01 scale=0.0..10.0 scale format="%_1f"
  in  "AO2":dbl(slide) caption="Confocal X (V)" min=0.0 max=10.0 step=0.01 scale=0.0..10.0 scale format="%_1f"
  in  "Trap Raster Scan":bool
  out "Raster Scanning...":bool
  in  "Trap Delta (MHz)":dbl=20.0 step=1.0
  in  "Trap Intensity\nSetpoints (V)":cluster{"Set 1":dbl, "Set 2":dbl}={"Set 1"=5.2, "Set 2"=6.6}
  in  "Index":dbl=1.0 caption="Save File Index" min=1.0 step=1.0
  in  "BD 1 Frequency 1 (MHz)":dbl=65.0 caption="T1 X (MHz)" min=50.0 max=100.0 step=1.0 format="%#_6p"
  out "Current Position":dbl[](array[numeric])=[4.2944, 4.91027471, 2.9278058] format="%7_7g"
  in  "Position Label 5":string="upper flow spot" caption="5"
  in  "Position 1 Label":string="Top capillary (SA beads)" caption="1"
  in  "Position 2 Label":string="Bottom capillary (AD) beads)" caption="2"
  in  "Position 3 Label":string="lower flow spot (ATP)" caption="3"
  in  "Position 4 Label":string="Dump beads" caption="4"
  out "Pump 3 cont disp":string="Left: ADig beads"
  out "Pump 1 cont disp":string="Right: DNA beads "
  in  "Ch 1 Inject Rate (ul/h)":dbl=50.0
  in  "Pump write delay (ms)":dbl=300.0
  in  "All Pump Parameters":T5={"Pump 1"={"Diameter (mm)"=4.61, "Units"=4.0, "Volume"=100.0, "Rate"=50.0}, "Pump 2"={"Diameter (mm)"=4.61, "Units"=3.0, "Volume"=0.0, "Rate"=0.0}, "Pump 3"={"Diameter (mm)"=4.61, "Units"=4.0, "Volume"=100.0, "Rate"=250.0}}
  in  "Ch 2 Inject Volume (uL)":dbl=100.0
  in  "Pump pause delay (ms)":u32
  in  "Ch 3 Inject Volume (uL)":dbl=100.0
  in  "Ch 3 Inject Rate (ul/h)":dbl=250.0
  in  "Flush Center Ch Volume (uL)":dbl=15.0
  in  "Flush Center Ch Rate (ul/m)":dbl=100.0
  in  "Inject Valve B":bool caption="Inject Pump 2\n(Flush Center)"
  in  "Total Volume\nFlushed (uL)":dbl
  in  "Tab Control 2":T6(tab)=enum."Feedback on Trap Intensity"
  in  "Restart RF":bool
  out "Total Counts (ticks)":u32=600
  in  "Trap ON/OFF X or Y Amp?":bool=TRUE
  in  "Oscillate Set 2":bool
  in  "Trap 1 ON":bool=TRUE
  in  "Number Interlace Sets":u8=3 min=1 max=3
  in  "DIO count 3 (ticks)":u32=200
  in  "DIO count 2 (ticks)":u32=200
  in  "DIO count 1 (ticks)":u32=200
  in  "BD 2 Amplitude 3 (%)":dbl min=0.0 max=75.0 step=1.0
  in  "BD 2 Amplitude 2 (%)":dbl min=0.0 max=75.0 step=1.0
  in  "BD 2 Amplitude 1 (%)":dbl min=0.0 max=75.0 step=1.0
  in  "BD 1 Amplitude 3 (%)":dbl min=0.0 max=75.0 step=1.0
  in  "BD 1 Amplitude 2 (%)":dbl=30.0 min=0.0 max=75.0 step=1.0
  in  "BD 1 Amplitude 1 (%)":dbl=30.0 min=0.0 max=75.0 step=1.0
  in  "BD 2 Frequency 3 (MHz)":dbl=26.0 min=50.0 max=100.0 step=1.0 format="%#_6p"
  in  "BD 1 Frequency 3 (MHz)":dbl=70.0 min=50.0 max=100.0 step=1.0 format="%#_6p"
  in  "BD 2 Frequency 2 (MHz)":dbl=26.0 min=50.0 max=100.0 step=1.0 format="%#_6p"
  in  "BD 2 Frequency 1 (MHz)":dbl=26.0 min=50.0 max=100.0 step=1.0 format="%#_6p"
  in  "Not-Interlacing Set":enum32{"Set 1", "Set 2", "Set 3"}(radio)
  in  "Interlace":bool=TRUE
  in  "Trap 2 ON":bool=TRUE
  in  "Trap 3 ON":bool
  in  "Scan axis 2":bool=TRUE
  in  "Osc. freq. (Hz)":dbl=0.25
  in  "Osc. amp. (MHz)":dbl=2.0 format="%1_3g"
  out "Coords":T7
  in  "Manipulation Scaling":cluster{"Horizontal":dbl, "Vertical":dbl}={"Horizontal"=0.075, "Vertical"=0.01}
  in  "Freq or Amp switch first":bool=TRUE
  in  "Swap F1 and F2":bool
  in  "Freq switch delay":u16
  in  "Amp switch delay":u16=5
  in  "Period":i64=2
  in  "MCL Step Increment (V_int)":dbl=3.0
  out "Time to Finish All (min)":dbl=0.122877 format="%#_2p"
  in  "Scan Speed (nm/s)":dbl=100.0
  in  "Scan Range (nm)":dbl=369.00000000000034
  in  "Step Size (nm)":dbl=1.0
  in  "MCL/AOM Scale Tweak":dbl=1.0
  in  "MCL Step Position Ratio":dbl=0.5
  in  "Move MCL Also?":bool=TRUE
  out "Final sep (nm)":dbl=4587.0
  out "Initial sep (nm)":dbl=4218.0
  out "Save index":dbl=22.0
  out "Final delta (MHz)":dbl=44.0
  out "Initial delta (MHz)":dbl=41.0
  out "Final freq. (MHz)":dbl=50.0
  out "Initial freq. (MHz)":dbl=53.0
  in  "Saved AOD Raster Scan Parameter Sets":T8(array[cluster])=[{"Scan Range AOD (nm) 2"=500.0, "Step Size AOD (nm) 2"=1.0, "Scan Speed AOD (nm/s) 2"=100.0, "Number of scans (AOD) 2"=1, "Label"="offset curve"}, {"Scan Range AOD (nm) 2"=420.0, "Step Size AOD (nm) 2"=1.0, "Scan Speed AOD (nm/s) 2"=100.0, "Number of scans (AOD) 2"=1, "Label"="hp raster check"}, {"Scan Range AOD (nm) 2"=6.8, "Step Size AOD (nm) 2"=0.34, "Scan Speed AOD (nm/s) 2"=0.34, "Number of scans (AOD) 2"=1, "Label"="3.4 kbp - 1 bp steps"}]
  in  "Load parameters":bool
  out "Scan Range (MHz)":dbl=-3.0000000000000027
  in  "Restart DMA? (AOD)":bool=TRUE caption="Restart DMA?"
  out "Incr. int (AOD)":i64=-7759651845
  out "Time/Scan (s) (AOD)":dbl=3.68631 format="%#_2p"
  out "Data points/scans":dbl=491508.0
  out "Data points/scan (f/b)":dbl=491508.0
  in  "Save scans":bool=TRUE
  out "AOD Scan I":u64 caption="Scan I"
  in  "Continuous AOD Scanning":bool caption="Continuous Scanning"
  in  "Abort AOD Scan":bool caption="Abort Scan"
  in  "Scan BD":bool=TRUE
  out "Cycles/step (AOD)":u64=666 format="%.3p"
  in  "Number of F/B Scans (AOD)":u16=1 min=1
  out "Scan steps (AOD)":u64=369
  out "Scan Increment (MHz)":dbl=-0.008152173913043485
  out "AOD Scanning":bool caption="Scanning"
  in  "Start AOD Scan":bool caption="Start Scan"
  out "N sets should be saved":dbl=24.5754
  out "Progress 2":u16(slide) caption="Progress" scale=0.0..100.0
  in  "Abort save 2":bool caption="Abort save"
  in  "Trap 1 Bead Size (nm)":dbl=2100.0
  in  "Trap 2 Bead Size (nm)":dbl=2100.0
  out "MCL Count":dbl=230502201.82069838
  in  "All FB On/Off":bool
  in  "AI2 to Setpoint":cluster{"Set 1":bool, "Set 2":bool}
  out "AI2 (V)":cluster{"Set 1":dbl, "Set 2":dbl}={"Set 1"=-0.0012207403790398877, "Set 2"=0.004577776421399579}
  in  "Reset Feedback":cluster{"Set 1":bool, "Set 2":bool}
  in  "PID Gains":T9={"Set 1"={"proportional gain (Kc)"=0, "integral gain (Kc*Ts/Ti)"=5, "derivative gain (Kc*Td/Ts)"=0}, "Set 2"={"proportional gain (Kc)"=0, "integral gain (Kc*Ts/Ti)"=5, "derivative gain (Kc*Td/Ts)"=0}}
  in  "Feedback On/Off":cluster{"Set 1":bool, "Set 2":bool}={"Set 1"=TRUE, "Set 2"=TRUE}
  in  "Set SP to Reading":bool
  out "Trap X (AI1)":T10={"Trap 1"=-1.0, "Trap 2"=0.899993896484375}
  in  "Trap Pos FB SP":fxp<+/-,16,1>=-0.092803955078125 caption="Setpoint"
  in  "Trap Pos. FB ON":bool
  in  "Reset Trap Pos. FB":bool
  out "Trap Positions":waveform(dbl)[](graph)=[{"t0"=timestamp(12.90000000000001 s since 1904-01-01), "dt"=0.15, "Y"=[-1.7479351299698465e-12, -1.7479351299698465e-12], "attributes"=variant("NI_ChannelName"=variant(string "Trap 1 Pos."))}, {"t0"=timestamp(12.90000000000001 s since 1904-01-01), "dt"=0.15, "Y"=[6.991740519879386e-12, 6.991740519879386e-12], "attributes"=variant("NI_ChannelName"=variant(string "Trap 2 Pos."))}]
  in  "Tab Control 8":enum32{"Main Setting", "Details"}(tab)
  in  "Trap Pos FB Int Count":u16=100
  in  "Trap Pos. FB Gains":T11={"proportional gain (Kc)"=10.0, "integral gain (Kc*Ts/Ti)"=10.0, "derivative gain (Kc*Td/Ts)"=0.0} {"proportional gain (Kc)" format="%.11g"; "integral gain (Kc*Ts/Ti)" format="%.11g"; "derivative gain (Kc*Td/Ts)" format="%.11g"}
  in  "Trap Pos. FB Offset Factor":i64
  in  "Trap Pos FB Negate Action":bool
  in  "Trap Pos. FB Mult Factor":i64=33554432
  in  "Trap Pos. AI1 X Pre-scale":u16
  in  "Trap Pos. FB Range":T12={"output high"=0.999969482421875, "output low"=-1.0}
  out "Trap Pos FB Int Signal":fxp<+/-,24,9> format="%.18g"
  out "Trap Pos FB Int-Norm Signal":fxp<+/-,16,1> format="%.16g"
  in  "Set SP Using...":bool
  in  "Trap Pos FB Monitor\nT1 or T2":bool
  out "Trap X AI1 (DMA)":T13={"Set 1"=0.999969482421875, "Set 2"=0.999969482421875}
  in  "N El. to Ave.":dbl=10000.0
  out "Trap Pos FB Action":i64
  out "Action (%)":dbl(knob) scale=-100.0..100.0
  in  "Trap Pos. FB Out Scale 2^n":u8=23 caption="Action Scale"
  out "Mean T1 Position (nm)":dbl=-1.7479351299698465e-12 caption="Mean T1 (nm)" format="%0.2f"
  out "Trap 1 Position RMS (A)":dbl caption="RMS (Ang)"
  in  "Tab Control 3":enum32{"Timing", "MCL Scan", "Analog Out"}(tab)
  out "APD 2 Gate Late Counter":u32
  out "APD 2 Gate Relative Phase":i16
  in  "Phase Adj. (APD 2 Gate)":i16=20
  in  "Initial Phase Adjustment (APD 2 Gate)":i16=55
  out "APD 1 Gate Late Counter":u32
  in  "- phase (APD 1 Gate)":bool
  in  "+ phase (APD 1 Gate)":bool
  out "APD 1 Gate Relative Phase":i16
  in  "Phase Adj. (APD 1 Gate)":i16=20
  in  "Initial Phase Adjustment (APD 1 Gate)":i16=60
  in  "Save APD Data\nwith Trap Data":bool=TRUE
  out "APD FIFO Elements Remaining":u32
  in  "- phase (APD Acq)":bool
  in  "+ phase (APD Acq)":bool
  out "APD Acq Late Counter":u32
  out "APD Acq Relative Phase":i16
  in  "Phase Adj. (APD Acq)":i16=20
  in  "Initial Phase Adjustment (APD Acq)":i16
  in  "Invert APD Gate":bool caption="Invert Gate"
  in  "APD Gate OFF Count":u32=450 caption="Gate OFF Count"
  in  "APD Gate ON Count":u32=150 caption="Gate ON Count"
  in  "APD Gate":enum32{"ON", "OFF", "Interlace"}(radio)=enum."Interlace"
  in  "APD Integration Time (s)":dbl=0.01 caption="Integration Time (s)"
  out "APD Acq Rate (Hz)":dbl=100.0 caption="Rate (Hz)"
  out "APD Samples/FIFO Acq.":dbl=30.0
  out "APD Elements/DMA read":u32=60
  out "APD Int. Count":u32=400000 format="%.0p"
  in  "+ phase (APD 2 Gate)":bool
  in  "- phase (APD 2 Gate)":bool
  in  "Tab Control 5":enum32{"PSD X", "PSD Y", "Other Data Channel"}(tab)
  out "Data map":dbl[][](graph)
  in  "Channel":i32=4
  in  "Abort MCL Scan":bool
  out "MCL Scan I":u64
  out "MCL Scanning":bool
  in  "Start MCL Scan":bool
  out "wait to reset values":bool
  in  "Tab Control 4":enum32{"Scan Settings", "MCL FPGA Loop Timing"}(tab)
  out "Total Time (s)":dbl=48.0
  in  "Scan lines (y)":u64=20
  in  "Fast Scan Dir":bool=TRUE
  in  "2D or 1D Scan":bool=TRUE
  out "Initial X":dbl
  out "Initial Y":dbl
  out "Time/f+b scan (s) (MCL)":dbl=2.4 caption="Time/scan (s)"
  in  "Number of scans (MCL)":u64=1 caption="Scans"
  in  "Scan steps (MCL)":u64=40 caption="Scan steps (x)"
  in  "N APD Samp/step":dbl=3.0
  in  "Scan Range (V)\n(of steps)":dbl=3.5
  in  "Restart DMA? (MCL)":bool=TRUE caption="Restart DMA?"
  in  "Continuous MCL Scanning":bool caption="Cont. Scanning"
  in  "Center Scan":bool=TRUE
  in  "Save Data (MCL)":bool=TRUE caption="Save Data"
  out "Actual Incr. int (MCL)":i16=294 caption="Incr. int"
  out "Desired incr (int)":dbl=294.0628205128205
  out "Desired Scan Incr (V)":dbl=0.08974358974358974
  out "N sets should be saved (MCL)":dbl=160.0 caption="N sets should be saved"
  out "Data points/scans (MCL)":dbl=4800.0 caption="Data points/scans"
  out "Data points/scan (f+b)":dbl=240.0 caption="points/scan (f+b)"
  out "Cycles/step (MCL)":u64=2000 caption="Cycles/step" format="%.0p"
  out "Actual MCL Inc (V)":dbl=0.08972441785943175
  in  "Phase adjust (MCL)":i16 caption="Phase adjust"
  out "Relative Phase (MCL)":i16 caption="Relative Phase"
  in  "Initial Phase Adj. (MCL)":i16 caption="Initial Phase Adj."
  in  "Update Count (MCL)":u32=600
  in  "+ phase (MCL)":bool
  in  "- phase (MCL)":bool
  out "MCL Late Counter":u32
  in  "APD 1 AO Mult.":i16=1 min=1
  in  "APD 2 AO Mult.":i16=1 min=1
  in  "Tab Control 7":enum32{"Green FB Signals", "Slow MCL Scan"}(tab)
  out "Green FB Plot":dbl(graph)=10.0
  out "MCL Scan 2":cluster{"Begin (V)":dbl, dbl, dbl[]}(graph)
  out "MCL Scan":cluster{"Begin (V)":dbl, dbl, dbl[]}(graph)
  in  "Green laser mode":enum32{"Laser ON", "Laser OFF", "Interlace"}(radio)
  in  "GI Frequency, ON count":u32=150 min=1 step=1
  in  "Invert GI":bool
  out "GI Late Counter":u32
  in  "Phase adj. (GI)":i16=5
  out "GI relative phase":i16
  in  "+ phase (GI)":bool
  in  "Initial Phase Adjustment (GI)":i16=19
  in  "GI Frequency, OFF count":u32=450 min=1 step=1
  in  "- phase (GI)":bool
  out "Green FB Signals (V)":cluster{"Y":dbl, "X":dbl, "Sum":dbl}={"Y"=1.0, "X"=1.0, "Sum"=10.0}
  out "Relative phase (Green FB)":i16
  in  "+ phase (Green FB)":bool
  in  "- phase (Green FB)":bool
  in  "Green FB Count":u32=600
  in  "Phase adj. (Green FB)":i16=10
  in  "Initial Phase Adjustment (Green FB)":i16=50
  in  "Green FB On/Off":bool
  in  "Current When FB OFF (%)":dbl=10.0 min=0.0 max=100.0 step=1.0
  in  "Green int current ON count adj":u32=150
  in  "Green FB Gains":T14={"proportional gain (Kc)"=10, "integral gain (Kc*Ts/Ti)"=5, "derivative gain (Kc*Td/Ts)"=0}
  in  "Green FB Setpoint (mV)":dbl=100.0
  in  "- phase (GI) 2":bool
  in  "Initial Phase Adjustment (GI) 2":i16=-100
  in  "+ phase (GI) 2":bool
  out "GI relative phase 2":i16
  in  "Phase adj. (GI) 2":i16=20
  out "GI Late Counter 2":u32
  in  "Trap Position FIFO Depth":u32=300000 format="%.0p"
  in  "# Samples/trap":u32=20000 format="%.0p"
  out "Trap AI Elements/DMA read":u32=320000 format="%.0p"
  out "Ave. Rate (Hz)":dbl=200000.0 format="%#_6p"
  out "Trap AI FIFO El. Rem.":u32 format="%.0p"
  in  "Phase adj. (AI1)":i16
  out "Relative phase (AI1)":i16
  in  "+ phase (AI1)":bool
  in  "- phase (AI1)":bool
  out "Late Counter (AI1)":u32
  in  "Initial Phase Adjustment (AI1)":i16=180
  out "AI rate (Hz)":dbl=200000.0 format="%#_6p"
  in  "AI Count (ticks)":u32=200
  out "# Samples/channel":u32=40000 format="%.0p"
  in  "Trap AI FIFO Depth":u32=340000 format="%.0p"
  in  "Detector Type":string(combo)="UCB Fleezers 052511"
  in  "N Acq Sets (Traps + Fl.)":i16=3
  in  "Sets to FIFO (Traps)":T15={"Set 1"=TRUE, "Set 2"=TRUE, "Set 3"=FALSE}
  in  "FPGA Ave.":dbl=1.0 min=1.0 step=1.0
  out "Ave. Period (s)":dbl=5e-06 format="%#_6p"
  out "DMA Update Period (s)":dbl=0.3
  out "FPGA Averaging":bool
  out "Trap Sets":u32=2
  out "Counts/DMA":dbl=12000000.0 format="%#_6p"
  out "Trap Pos FIFO El Remaining":u32=141
  out "Trap Pos Elements/DMA read":u32=120000 format="%.0p"
  out "Trap AI FIFO Timeout":u16
  out "Trap Pos FIFO Timeout":u16
  out "Waveform Chart":i32(graph)=320000
  out "error out 2":errorcluster
  in  "Lost Tether Alarm Threshold (pN)":dbl=0.5
  in  "AOM X Cal (nm/MHz)":dbl=168.33
  in  "MCL X Cal (nm/V)":dbl=1070.0
  out "X RF Amplitude Limits (%)":T16={"Minimum"=0.0, "Maximum"=50.0, "Increment"=1.0}
  out "X RF Frequency Limits (MHz)":T16={"Minimum"=50.0, "Maximum"=100.0, "Increment"=1.0}
  out "Y RF Frequency Limits (MHz)":T16={"Minimum"=50.0, "Maximum"=100.0, "Increment"=1.0}
  out "Y RF Amplitude Limits (%)":T16={"Minimum"=0.0, "Maximum"=50.0, "Increment"=1.0}
  in  "Manip. X?":bool=TRUE
  in  "Manip. Y?":bool
  in  "Force Manip Abort":bool
  out "Read cal error":errorcluster
  in  "DAQ Delay (ms)":u32=1000
  in  "Start Scan":bool
  in  "Scan axis":bool
  in  "Osc. amp. (V)":dbl=5.0
  in  "Osc. center (V)":dbl=5.0
  in  "Osc. freq. (Hz) 2":dbl=1.0
  in  "MCL Mode":u16(ring) items=["Manual Positioning", "Sinusoidal Wave", "Linear Scan"]
  in  "Begin (V)":dbl
  in  "End (V)":dbl=10.0
  in  "N Points":dbl=20.0
  in  "Delay to Interlace (s)":dbl
  in  "Delayed Interlace Start":bool
  in  "Read Lateness and Rel Phase":bool
  out "Vec Mean of T1 T2":dbl[](array[numeric])=[nan, nan]
  in  "Cal read wait (s)":u32=5
  out "Time tether formed":timestamp=timestamp(3371146929.513132 s since 1904-01-01)
  in  "Chemyx Syringe Pump Serial Port":refnum<visa-resource-name>="ASRL3::INSTR"
  in  "Limit Min (MHz)":dbl=10.0 caption="Min (MHz)"
  in  "Limit Max (MHz)":dbl=16.0 caption="Max (MHz)"
  in  "Limits Enable":bool=TRUE caption="Enable"
  out "AI labels":string[](array[string])=["T1 Y", "T1 X", "T1 Sum", "T2 Y", "T2 X", "T2 Sum", "T1 FB X", "T2 FB Sum", "T2 FB X", "T2 FB Sum", "PSD Y", "PSD X", "PSD Sum"]
  in  "Save Trap Pos. Data":bool=TRUE
  in  "ESP Port":refnum<visa-resource-name>="COM22"
  in  "Locations":i32(listbox)=1
  out "Selected Location":cluster{"x":string, "y":string, "z":string}={"x"="0.19233\r\n", "y"="0.00156\r\n", "z"="0.20615\r\n"}
  in  "Capture":bool
  in  "Save":bool
  in  "Goto Top (F6)":bool
  in  "Goto Exp (F8)":bool
  in  "Goto Bottom (F7)":bool
  in  "Axis 3":string="0.00500\r\n"
  in  "Axis 2":string="0.00500\r\n"
  in  "Axis 1":string="0.00500\r\n"
  in  "Axis 3":string="0.20000\r\n"
  in  "Axis 2":string="0.20000\r\n"
  in  "Axis 1":string="0.20000\r\n"
  in  "Activate Joystick":bool
  in  "ESP ZL-Limit":string="-0.09900"
  in  "ESP ZR-Limit":string="0.09900"
  out "Z Pos Pos":string="0.21899\r\n"
  out "Y Pos":string="0.00713\r\n"
  out "X Pos":string="0.20503\r\n"
  in  "error in":errorcluster
  out "error out":errorcluster
  out "Z motion":string
  out "Y Motion":string
  out "X Motion":string
  # "After"
  # "During"
  # "Trap On?"
  # "BD Flow ON?"
  # "Samp Flow ON?"
  # "1"
  # "2"
  # "Trap Display:"
  # "APD Display:"
  # "originally 10k"
  # "Trap Manipulation"
  # "DAQ"
  # "Data Saving"
  # "Central frequency 80 MHz"
  # "F9"
  # "Bead Calibration"
  # "F10"
  # "F4"
  # "Press F12 to move stage\nwith the mouse. F12 to cancel."
  # "F5"
  # "F6"
  # "F7"
  # "F8"
  # "Harvard Pump\n(sample channel for flow exp)"
  # "Chemyx Pump 2"
  # "Units: \n1 = ml/m\n2 = ml/h\n3 = ul/m\n4 = ul/h"
  # "Rate param is ul/h\nVolume param is ul"
  # "X"
  # "Y"
  # "Oscillate Set 2 freq. (debugging)"
  # "BD 1"
  # "BD 2"
  # "AOD Raster Scan"
  # "Approx. trap separations"
  # "X"
  # "Y"
  # "DON'T TURN ON\nUNTIL YOU CLOSE\nTHE LOOP"
  # "FPGA\nreading"
  # "DMA\ntransfer"
  # "APD Gates"
  # "APD 2"
  # "APD 1"
  # "X"
  # "2D"
  # "Y"
  # "1D"
  # "Green Laser Interlacing"
  # "Green FB Measurement"
  # "Digital Gate"
  # "Current Analog Control"
  # "was 87"
  # "originally 600k"
  # "Total AI Rates (NOT rates/trap)"
  # "originally 20k"
  # "(Samples/trap x Trap Sets)"
  # "(Samples/channel x\n8 if averaging (8 channels)\n4 if no averaging)"
  # "Trap 1"
  # "Trap 2"
  # "Flour./Trap 3"
  # "External Video Window"
  # "MCL Position Debugging"
  # "Temporary Control Storage\n(these used to be somewhere else, still want to keep them)"
  # "Y"
  # "X"
  # "Trap Position Difference Limits"
  # "Joystick Control"
  # "Setting Limit for the z-axis"
  # "Current Location"
  # "Save Positions of Cambers"
  # "Errors detected in determing Current Location"
  # "High Jog Velocity"
  # "Low Jog Velocity"
  # "Select the chamber to go to"
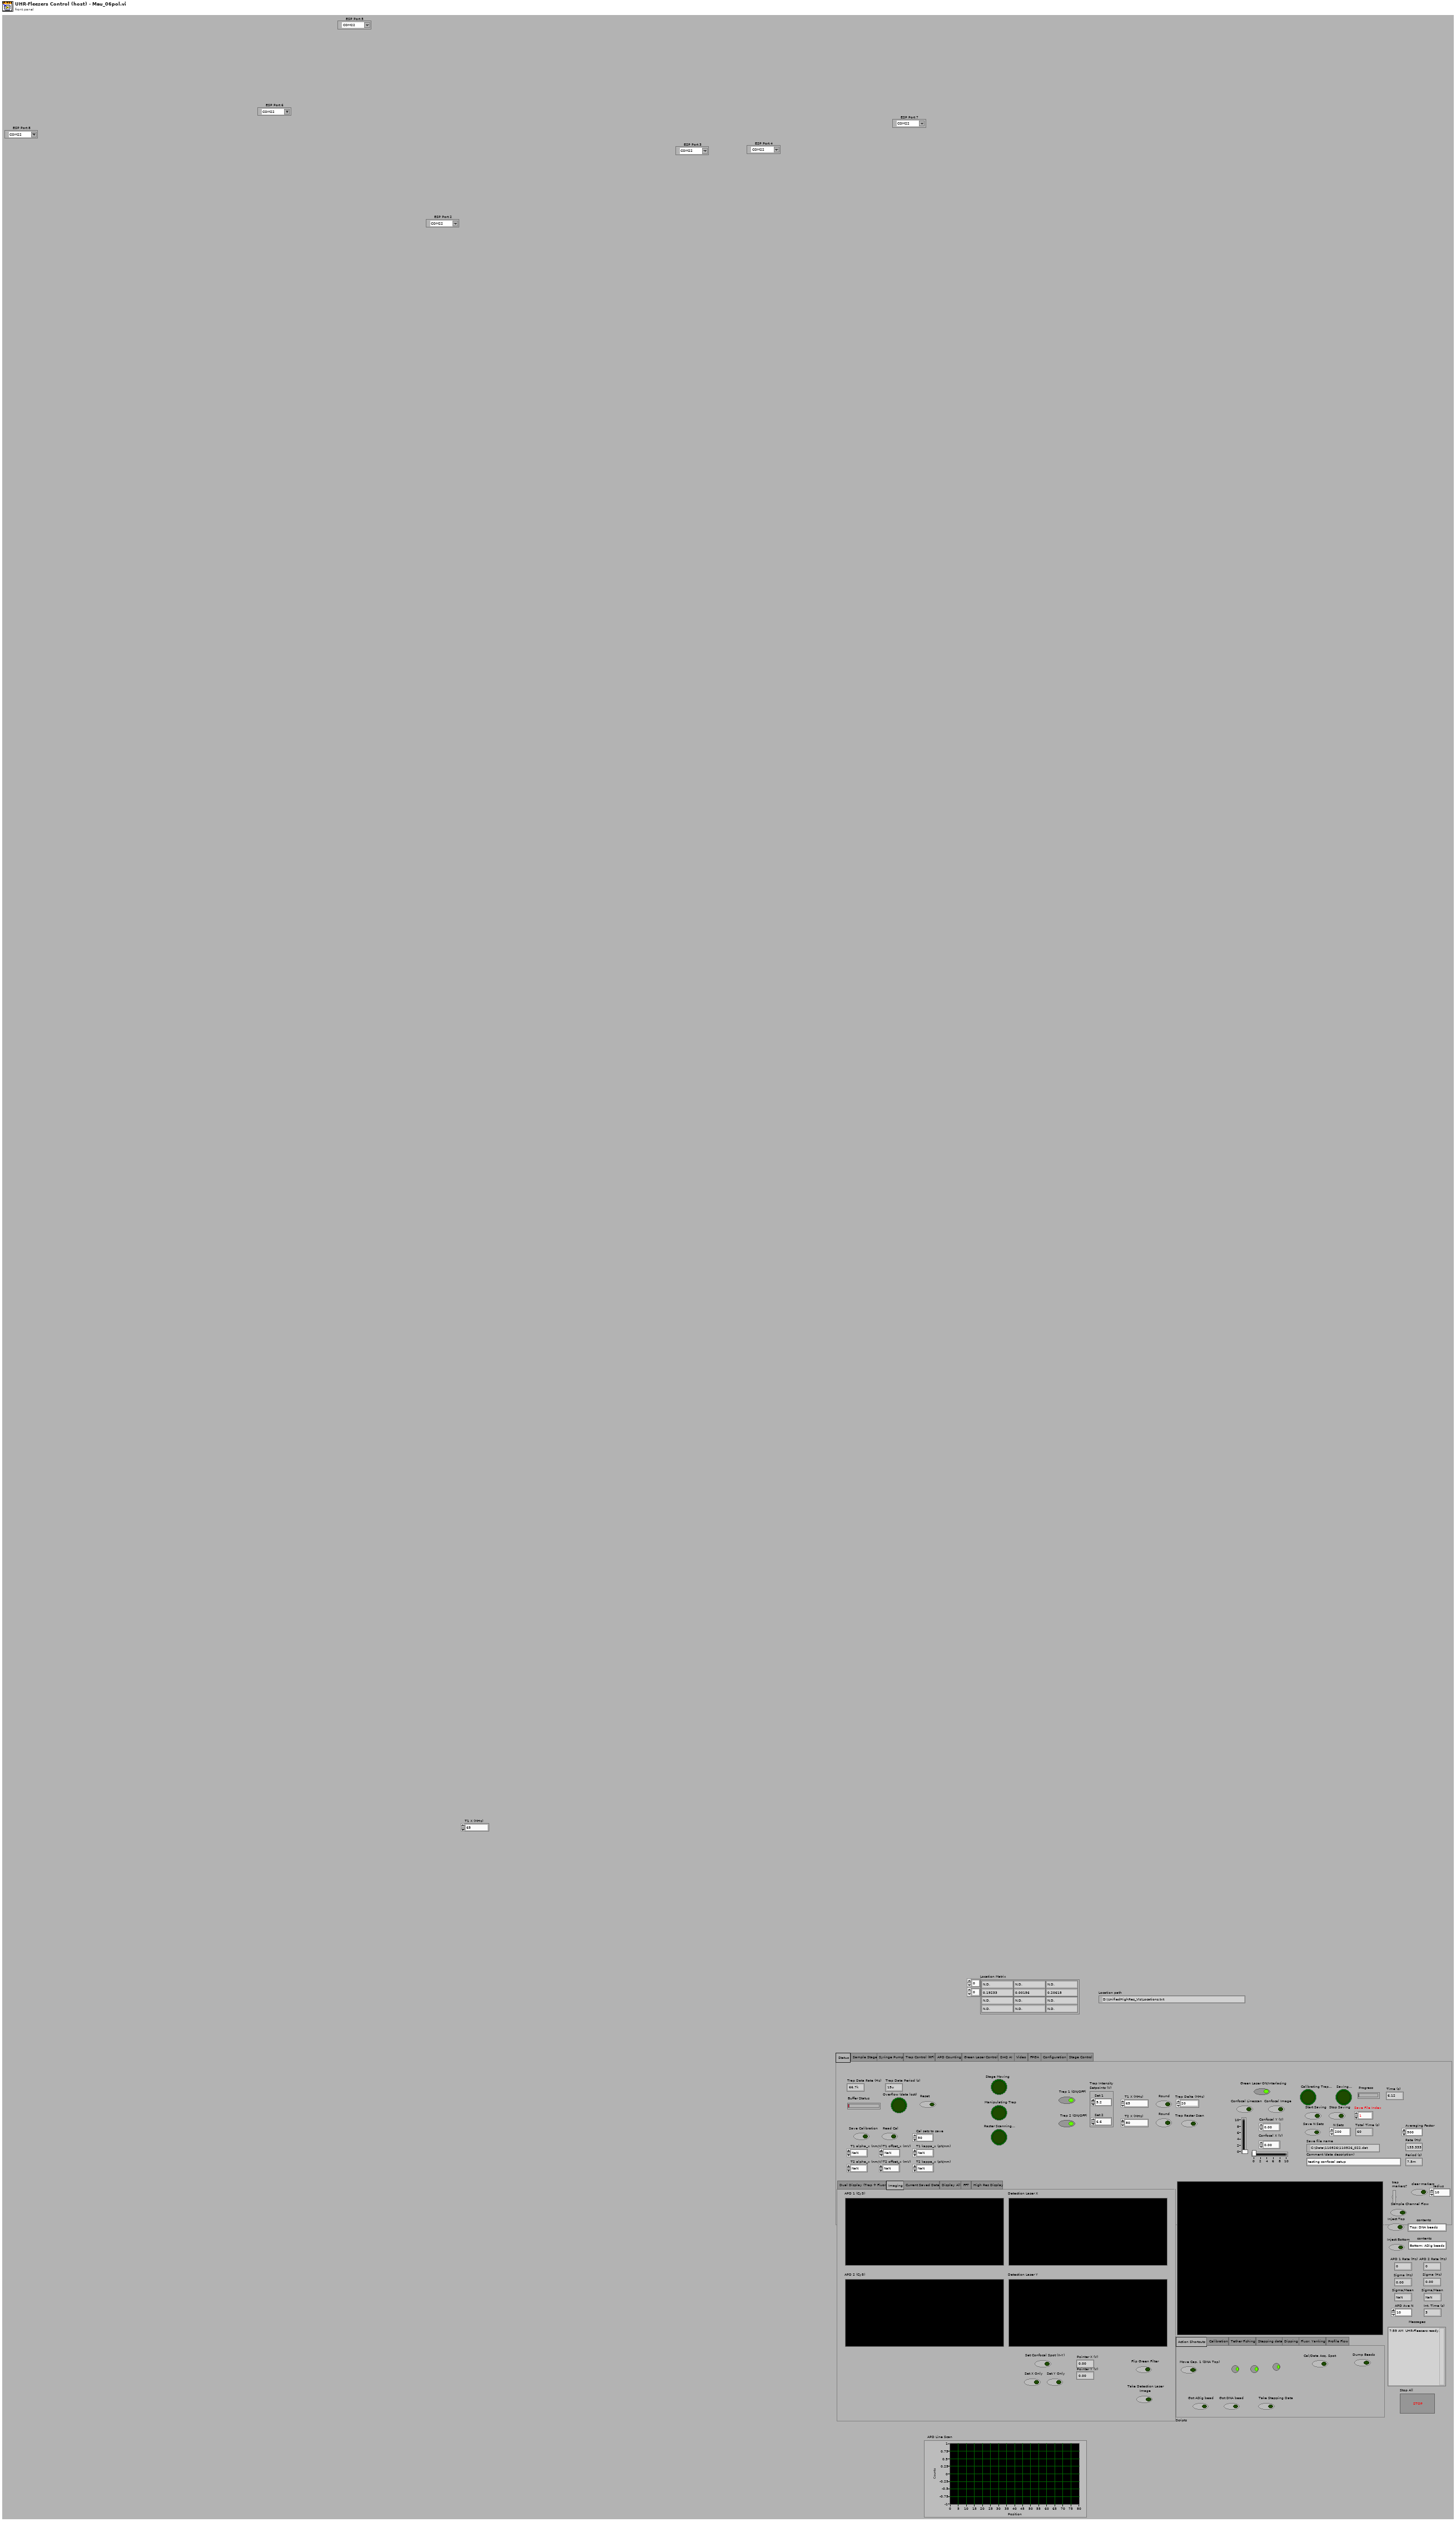
[diagram p1: front panel]
types:
  T1 = enum32{"Action Shortcuts", "Calibration", "Tether Fishing", "Stepping data", "Dipping", "Fluor. Yanking", "Profile Flow"}
  T2 = typedef "IMAQ Image.ctl" = refnum<image>
  T3 = enum32{"Dual Display (Trap + Fluor.)", "Imaging", "Current Saved Data", "Display All", "FFT", "High Res Display"}
  T4 = enum32{"Status", "Sample Stage", "Syringe Pump", "Trap Control (RF)", "APD Counting", "Green Laser Control", "DAQ AI", "Video", "FPGA", "Configuration", "Stage Control"}
  T5 = cluster{"Pump 1":cluster{"Diameter (mm)":dbl, "Units":dbl, "Volume":dbl, "Rate":dbl}, "Pump 2":cluster{"Diameter (mm)":dbl, "Units":dbl, "Volume":dbl, "Rate":dbl}, "Pump 3":cluster{"Diameter (mm)":dbl, "Units":dbl, "Volume":dbl, "Rate":dbl}}
  T6 = enum32{"IR Laser Interlacing (Direct RF Board Control Method)", "AOD Raster Scan", "Feedback on Trap Intensity", "Feedback on Trap Position"}
  T7 = typedef "LVPoint32TypeDef.ctl" = cluster{"Horizontal":i32, "Vertical":i32}
  T8 = cluster{"Scan Range AOD (nm) 2":dbl, "Step Size AOD (nm) 2":dbl, "Scan Speed AOD (nm/s) 2":dbl, "Number of scans (AOD) 2":u16, "Label":string}[]
  T9 = cluster{"Set 1":cluster{"proportional gain (Kc)":i16, "integral gain (Kc*Ts/Ti)":i16, "derivative gain (Kc*Td/Ts)":i16}, "Set 2":cluster{"proportional gain (Kc)":i16, "integral gain (Kc*Ts/Ti)":i16, "derivative gain (Kc*Td/Ts)":i16}}
  T10 = cluster{"Trap 1":fxp<+/-,16,1>, "Trap 2":fxp<+/-,16,1>}
  T11 = cluster{"proportional gain (Kc)":fxp<+/-,16,8>, "integral gain (Kc*Ts/Ti)":fxp<+/-,16,8>, "derivative gain (Kc*Td/Ts)":fxp<+/-,16,8>}
  T12 = cluster{"output high":fxp<+/-,16,1>, "output low":fxp<+/-,16,1>}
  T13 = cluster{"Set 1":fxp<+/-,16,1>, "Set 2":fxp<+/-,16,1>}
  T14 = cluster{"proportional gain (Kc)":i16, "integral gain (Kc*Ts/Ti)":i16, "derivative gain (Kc*Td/Ts)":i16}
  T15 = cluster{"Set 1":bool, "Set 2":bool, "Set 3":bool}
  T16 = typedef "LVMinMaxIncTypeDef.ctl" = cluster{"Minimum":dbl, "Maximum":dbl, "Increment":dbl}
  T17 = typedef "Image Type" = u32
  T18 = typedef "nirio_resource_hc.ctl" = tag
  T19 = typedef "openfpgaref.8.6.ctl" = refnum<k20>
  T20 = enum16{"CONNECT", "INITIALIZE VALVES", "DISCONNECT", "MOVE VALVE"}
  T21 = cluster{"New Image":T2, "New Image":T2, "New Image":T2, "New Image":T2}
  T22 = cluster{"Location Matrix[0]":string, "Location Matrix[1]":string, "Location Matrix[2]":string}
  T23 = enum16{"open", "replace", "create", "open or create", "replace or create", "replace or create with confirmation"}
  T24 = typedef "XDNodeRunTimeDep.lvlib/timing_clust.ctl" = cluster{"Expected End [f-1]":u64, "Actual End [f-1]":u64, "Finished Late? [f-1]":bool, "Expected End [i-1]":u64, "Actual End [i-1]":u64, "Finished Late? [i-1]":bool, "Expected Start [i]":u64, "Actual Start [i]":u64, "Expected Start [f]":u64, "Actual Start [f]":u64, "Source Name":string, "Structure Name":string, "Period":i64, "Deadline":i64, "Offset":i64, "Start":i64, "Priority":i32, "Timeout":i32, "Mode":T25, "Wakeup Reason":T26, "Error":errorcluster, "Source Type":string, "Secondary Source Type":string, "Global End Time":u64, "Global Start Time":u64, "Frame Duration":u64, "Iteration Duration":u64, "Assigned CPU":i32, "I/O Scan Engine Mode":u32}
  T25 = typedef "XDNodeRunTimeDep.lvlib/nitl_modes.ctl" = enum32{"No Change", "Process missed periods, maintain original phase", "Discard missed periods, maintain original phase", "Process missed periods, ignore original phase", "Discard missed periods, ignore original phase"}
  T26 = typedef "XDNodeRunTimeDep.lvlib/wakeup.ctl" = enum32{"Normal", "Aborted", "Asynchronous wakeup", "Timing source error", "Timed loop error", "Timeout"}
  T27 = cluster{"[0]":i32, "[1]":i32, "[2]":i32, "[3]":i32}
  T28 = cluster{"[0]":i32, "[1]":i32, "[2]":i32, "[3]":i32}[]
  T29 = enum16{"big-endian, network order", "native, host order", "little-endian"}
  T30 = cluster{"Scan Range AOD (nm) 2":dbl, "Step Size AOD (nm) 2":dbl, "Scan Speed AOD (nm/s) 2":dbl, "Number of scans (AOD) 2":u16, "Label":string}
  T31 = cluster{"[0]":dbl, "[1]":dbl, "[2]":dbl, "[3]":dbl, "[4]":dbl, "[5]":dbl}
  T32 = cluster{"Diameter (mm)":dbl, "Units":dbl, "Volume":dbl, "Rate":dbl}
  T33 = cluster{"Left":i32, "Top":i32, "Width":u32, "Height":u32}
  T34 = cluster{cluster{"Left":i32, "Top":i32, "Width":u32, "Height":u32}}[]
  T35 = enum32{"Normal Display", "Dual Display (APD)", "FFT", "High Res Display"}
  T36 = cluster{"Origin Pixel":cluster{"X":sgl, "Y":sgl}, "Angle Relative to Horizontal (deg)":sgl, "Axis Reference":u32}
  T37 = typedef "Simple Grid Descriptor" = cluster{"X Step":sgl, "Y Step":sgl, "Unit":T38}
  T38 = typedef "Image Unit" = enum32{"Undefined", "Angström", "Micrometer", "Millimeter", "Centimeter", "Meter", "Kilometer", "Microinch", "Inch", "Feet", "Nautical miles", "Standard miles", "Steps"}
  T39 = cluster{"averaging mode":u16, "weighting mode":u16, "number of averages":u32}
  T40 = cluster{"dB On (F)":bool, "unwrap phase (F)":bool, "convert to degree (F)":bool}
  T41 = cluster{string, string, string, string, string, string, string, string}
  T42 = cluster{string, string, string, string, string, string, string, string, string, string, string, string}
  T43 = cluster{string, string, string, string, string, string, string, string, string, string, string, string, string}
  T44 = cluster{string, string, string, string, string, string, string, string, string, string, string, string, string, string}
  T45 = cluster{"BD 1 Frequency 1 (MHz)":dbl, "BD 1 Frequency 2 (MHz)":dbl}
  T46 = cluster{"f0":dbl, "df":dbl, "magnitude":dbl[]}[][]
  T47 = cluster{"Green FB Ch 0":i16, "Green FB Ch 1":i16, "Green FB Ch 2":i16}
  T48 = cluster{"Green FB Ch 0":dbl, "Green FB Ch 1":dbl, "Green FB Ch 2":dbl}
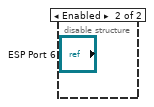
[diagram p3: hidden frame]
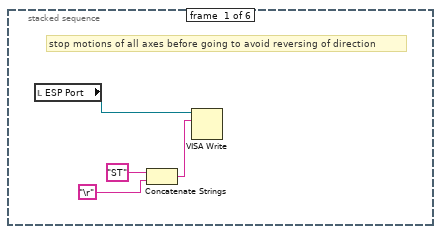
[diagram p5: hidden frame]
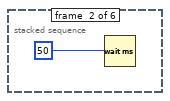
[diagram p6: hidden frame]
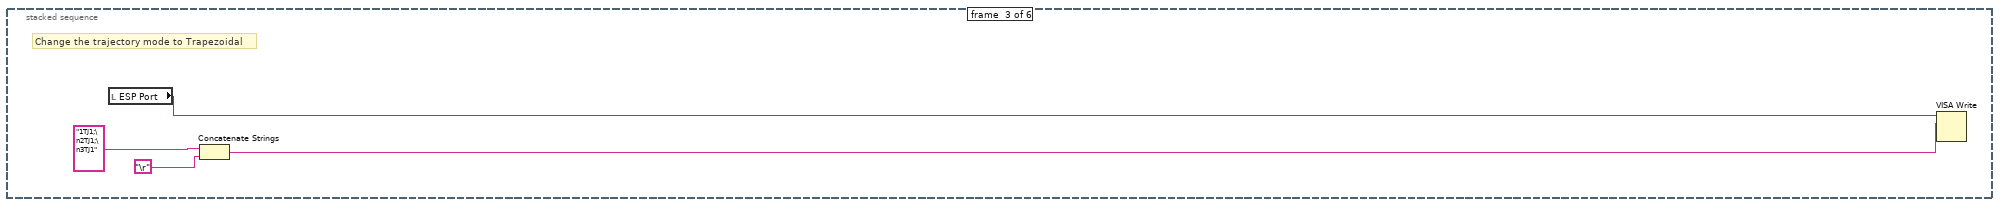
[diagram p7: hidden frame]
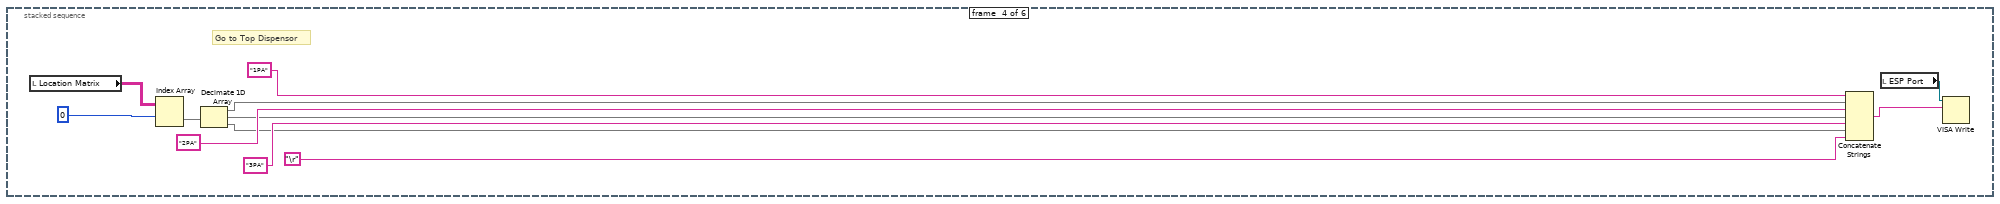
[diagram p8: hidden frame]
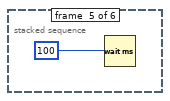
[diagram p9: hidden frame]
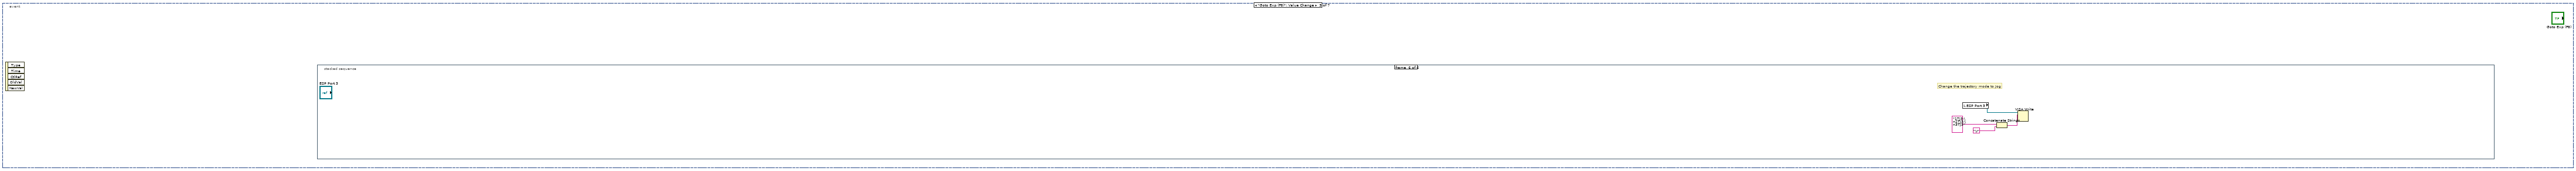
[diagram p10: hidden frame]
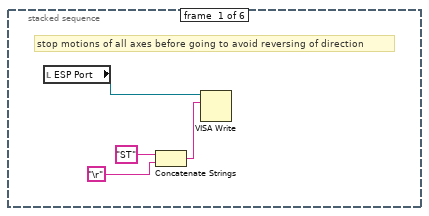
[diagram p11: hidden frame]
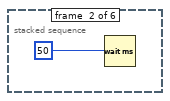
[diagram p12: hidden frame]
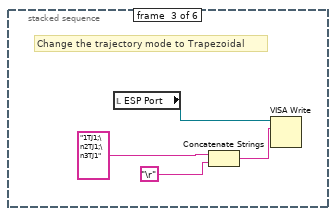
[diagram p13: hidden frame]
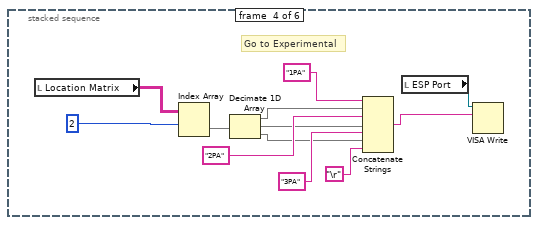
[diagram p14: hidden frame]
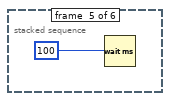
[diagram p15: hidden frame]
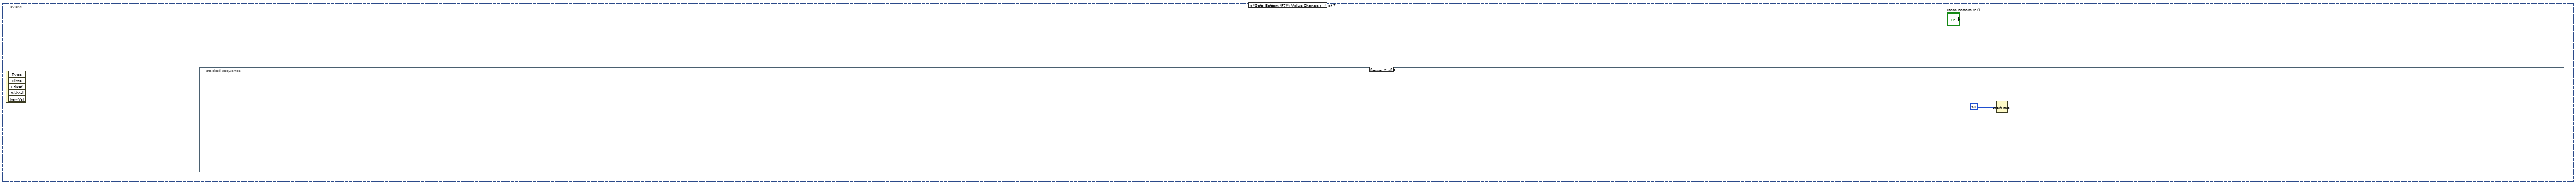
[diagram p16: hidden frame]
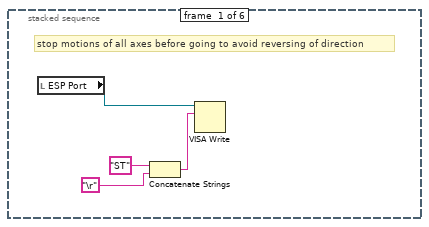
[diagram p17: hidden frame]
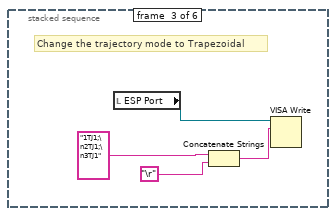
[diagram p18: hidden frame]
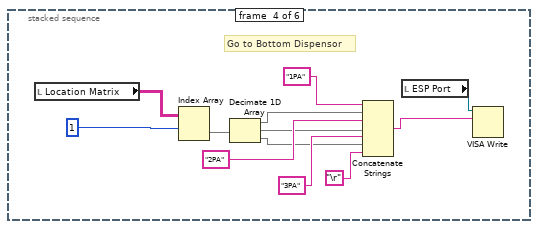
[diagram p19: hidden frame]
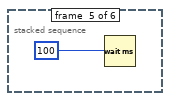
[diagram p20: hidden frame]
diagram:
  w64 = T17 2 items=["Grayscale (U8)", "Grayscale (I16)", "Grayscale (SGL)", "Complex (CSG)", "RGB (U32)", "HSL (U32)", "RGB (U64)", "Grayscale (U16)"] ("Image Type")
  w121 = cluster{"output high":i16, "output low":i16} {"output high"=3000, "output low"=0} ("FB output range 1")
  w196 = 10.0 ("y")
  w195 = 32767.0 ("y")
  w211 = 6.0  # clock mult.
  w212 = 49152000.0  # TCXO frequ.
  # "Initialize location matrix"
  n1 = Build Array("DIO count 1 (ticks)", "DIO count 2 (ticks)", "DIO count 3 (ticks)") -> (w110:u32[])
  n2 = Multiply(x="APD Integration Time (s)", y=40000000.0) -> (x*y=w128:dbl)
  n3 = Reciprocal(x="APD Integration Time (s)") -> (1/x=w125:dbl)
  n4 = local write "APD Acq Rate (Hz)"(w125) -> ()
  n5 = local read "AO1"() -> (w190:dbl)
  n6 = local read "AO2"() -> (w189:dbl)
  n7 = To Unsigned Long Integer(number=w128) -> (unsigned 32bit integer=w127:u32)
  "APD Int. Count" <- w127
  n8 = local read "Scan Increment (MHz)"() -> (w207:dbl)
  n9 = local read "Continuous MCL Scanning"() -> (w177:bool)
  n10 = local read "Fast Scan Dir"() -> (w176:bool)
  n11 = local read "Trap Intensity\nSetpoints (V)"() -> (w226:cluster{"Set 1":dbl, "Set 2":dbl})
  n12 = local read "Number of scans (MCL)"() -> (w178:u64)
  n13 = Multiply(x=w190, y=w195) -> (x*y=w192:dbl)
  n14 = Multiply(x=w189, y=w195) -> (x*y=w194:dbl)
  n15 = Divide(x=w192, y=w196) -> (x/y=w191:dbl)
  n16 = Divide(x=w194, y=w196) -> (x/y=w193:dbl)
  n17 = To Word Integer(number=w191) -> (16bit integer=w188:i16)
  n18 = To Word Integer(number=w193) -> (16bit integer=w187:i16)
  n19 = Not(x=w176) -> (.not. x?=w171:bool)
  n20 = local read "Cycles/step (MCL)"() -> (w179:u64)
  n21 = Multiply(x=w207, y=1000.0) -> (x*y=w214:dbl)
  n22 = local read "Scan steps (MCL)"() -> (w180:u64)
  n23 = local write "Trap Pos FIFO Timeout"(u16 0 ("Trap Pos FIFO Timeout")) -> ()
  n24 = local read "Desired Scan Incr (V)"() -> (w182:dbl)
  n25 = Scale By Power Of 2(n=48, x=w214) -> (x*2^n=w215:dbl)
  n26 = Multiply(x=w212, y=w211) -> (x*y=w210:dbl)
  n27 = Divide(x=w215, y=w210) -> (x/y=w209:dbl)
  n28 = local read "Number Interlace Sets"() -> (w103:u8)
  n29 = Split 1D Array(array=w110, index=w103) -> (first subarray=w112:u32[])  [unwired: 1 out]
  n30 = Add Array Elements(numeric array=w112) -> (sum=w111:u32)
  n31 = property on="AI Count (ticks)" class="DigNum (strict)"("Val(Sgnl)"="AI Count (ticks)") -> ()  [unwired: 2 in, 2 out]
  n32 = local read "# Samples/channel"() -> (w199:u32)
  n33 = local read "Number of F/B Scans (AOD)"() -> (w200:u16)
  n34 = To Quad Integer(1:w209) -> (0:w206:i64)
  n35 = local read "Not-Interlacing Set"() -> (w102:enum32{"Set 1", "Set 2", "Set 3"})
  n36 = To Unsigned Byte Integer(number=w102) -> (unsigned 8bit integer=w108:u8)
  n37 = Index Array(array=w110, index=w108) -> (element=w109:u32)
  n38 = local read "Feedback On/Off"() -> (w229:cluster{"Set 1":bool, "Set 2":bool})
  n39 = local read "PID Gains"() -> (w221:T9)
  n40 = Divide(x=40000000.0, y="AI Count (ticks)") -> (x/y=w168:dbl)
  n41 = Multiply(x=w182, y=32767.0) -> (x*y=w184:dbl)
  n42 = local read "Scan steps (AOD)"() -> (w205:u64)
  n43 = local read "All FB On/Off"() -> (w230:bool)
  n44 = local read "Cycles/step (AOD)"() -> (w204:u64)
  n45 = local write "AI rate (Hz)"(w168) -> ()
  n46 = Divide(x=w184, y=10.0) -> (x/y=w183:dbl)
  n47 = Multiply(x=w205, y=w204) -> (x*y=w203:u64)
  n48 = Multiply(x=3276.7, y=w226) -> (x*y=w225:cluster{"Set 1":dbl, "Set 2":dbl})
  n49 = To Word Integer(number=w183) -> (16bit integer=w181:i16)
  n50 = Multiply(x=w203, y=u64 2) -> (x*y=w201:u64)
  n51 = local read "Sets to FIFO (Traps)"() -> (w233:T15)
  n52 = Divide(x=w168, y="FPGA Ave.") -> (x/y=w169:dbl)
  n53 = To Word Integer(number=w225) -> (16bit integer=w224:cluster{"Set 1":i16, "Set 2":i16})
  n54 = xnode "Open FPGA VI Reference"("resource name"=T18 "750kHzDAQ") -> ("FPGA VI Reference Out"=w218:T19)  [unwired: 1 in, 1 out]
  n55 = Unbundle By Name(w221) -> ("Set 1"=w220:T14, "Set 2"=w219:T14)
  n56 = Multiply(x=w201, y=w200) -> (x*y=w198:u64)
  n57 = local write "Ave. Rate (Hz)"(w169) -> ()
  n58 = Divide(x=w198, y=w199) -> (x/y=w197:dbl)
  n59 = Unbundle By Name(w224) -> ("Set 1"=w223:i16, "Set 2"=w222:i16)
  n60 = local read "2D or 1D Scan"() -> (w122:bool)
  n61 = local write "Data points/scans"(w198) -> ()
  n62 = local read "Scan BD"() -> (w216:bool)
  n63 = And(x=w229, y=w230) -> (x .and. y?=w228:cluster{"Set 1":bool, "Set 2":bool})
  n64 = local write "Data points/scan (f/b)"(w201) -> ()
  n65 = Reciprocal(x=w169) -> (1/x=w170:dbl)
  n66 = local read "N Acq Sets (Traps + Fl.)"() -> (w161:i16)
  n67 = local write "N sets should be saved"(w197) -> ()
  n68 = Unbundle By Name(w228) -> ("Set 1"=w232:bool, "Set 2"=w231:bool)
  n69 = local read "Interlace"() -> (w104:bool)
  n70 = Select(t=w111, s=w104, f=w109) -> (s? t:f=w101:u32)
  n71 = local write "Update Count (MCL)"(w101) -> ()
  n72 = local write "Total Counts (ticks)"(w101) -> ()
  n73 = xnode "Invoke Method"("FPGA VI Reference In"=w218) -> ("FPGA VI Reference Out"=w120:T19, "error out"=w139:errorcluster)  [unwired: 1 in]
  n74 = local write "Ave. Period (s)"(w170) -> ()
  n75 = property on="2D or 1D Scan" class="Bool (strict)"("Val(Sgnl)"=w122) -> ()  [unwired: 2 in, 2 out]
  n76 = xnode "Read/Write Control"("FPGA VI Reference In"=w119, "error in"=w139, "ai count"="AI Count (ticks)", "Interlace ON/OFF"=w104, "Number Interlace Cycles"=w103, "AI1 Sets to FIFO"=w233, "FB On/Off Set 1"=w232, "FB On/Off Set 2"=w231, "Interlace Off Parameters"=w102, "FB Setpoint Set 1"=w223, "FB Setpoint Set 2"=w222, "FB Gains Set 1"=w220, "FB Gains Set 2"=w219, "FB output range 1"=w121, "FB output range 2"=w121, "Cycles per step"=w204, "Scan BD"=w216, "Number of scans"=w200, "Scan steps"=w205, "Scan freq.  increment"=w206, "AO1"=w188, "AO2"=w187, "Scan freq.  increment (MCL)"=w181, "Scan steps (MCL)"=w180, "Cycles per step (MCL)"=w179, "Number of scans (MCL)"=w178, "MCL count"=w101, "Cont. Scan (MCL)"=w177, "MCL Scan Axis"=w171, "1D or 2D Scan?"=w122, "N of AI1 Int Acq Sets"=w161, "Freq or Amp switch first"="Freq or Amp switch first", "Freq switch delay"="Freq switch delay", "Amp switch delay"="Amp switch delay", "Swap F1 and F2"="Swap F1 and F2", "APD Acq Rate Count"=w127, "APD to FIFO"=FALSE, "APD Gate Operating Mode"="APD Gate", "APD Gate ON Count"="APD Gate ON Count", "APD Gate OFF Count"="APD Gate OFF Count", "Invert APD Gate"="Invert APD Gate", "DIO count 1 (ticks)"="DIO count 1 (ticks)", "DIO count 2 (ticks)"="DIO count 2 (ticks)", "DIO count 3 (ticks)"="DIO count 3 (ticks)", "APD 1 AO scale factor"="APD 1 AO Mult.", "APD 2 AO scale factor"="APD 2 AO Mult.") -> ("FPGA VI Reference Out"=w96:T19, "error out"=w98:errorcluster)  [unwired: 1 in]
  n77 = local read "Green Laser ON/Interlacing"() -> (w99:bool)
  n78 = local read "Green laser mode"() -> (w100:enum32{"Laser ON", "Laser OFF", "Interlace"})
  n79 = local read "GI Frequency, OFF count"() -> (w92:u32)
  n80 = local read "GI Frequency, ON count"() -> (w91:u32)
  n81 = Multiply(x="Current When FB OFF (%)", y=655.35) -> (x*y=w82:dbl)
  n82 = local read "Green FB Count"() -> (w90:u32)
  n83 = Multiply(x="Green FB Setpoint (mV)", y=3.2767) -> (x*y=w79:dbl)
  n84 = To Unsigned Word Integer(number=w82) -> (unsigned 16bit integer=w80:u16)
  n85 = local read "Invert GI"() -> (w94:bool)
  n86 = To Word Integer(number=w79) -> (16bit integer=w77:i16)
  n87 = case shown="True" w99 {
    tunnel: w100 -> [_ w253]
    tunnel: [enum32{"Laser ON", "Laser OFF", "Interlace"}."Laser OFF" ("Green laser mode") w253] -> w93
    frame False {
    }
    frame True {
    }
  }
  n88 = local read "Trap Pos. AI1 X Pre-scale"() -> (w48:u16)
  n89 = local read "Trap Pos FB Monitor\nT1 or T2"() -> (w55:bool)
  n90 = local read "Trap Pos FB Int Count"() -> (w43:u16)
  n91 = local read "Trap Pos FB Negate Action"() -> (w54:bool)
  n92 = local read "Trap Pos. FB Offset Factor"() -> (w53:i64)
  n93 = local read "Trap Pos. FB Mult Factor"() -> (w52:i64)
  n94 = local read "Trap Pos. FB Gains"() -> (w50:T11)
  n95 = local read "Trap Pos. FB Range"() -> (w51:T12)
  n96 = xnode "Read/Write Control"("FPGA VI Reference In"=w96, "error in"=w98, "Green interlace ON count 2"=w91, "Green interlace OFF count 2"=w92, "Invert GI 2"=w94, "Operating Mode 2"=w93, "Green FB Gains"="Green FB Gains", "Green FB Setpoint"=w77, "Green FB On/Off"="Green FB On/Off", "Current Out"=w80, "Green int current ON count adj"="Green int current ON count adj", "Green FB Count"=w90, "Operating Mode"=w93, "Green interlace OFF count"=w92, "Green interlace ON count"=w91, "Invert GI"=w94, "Trap Pos FB Monitor T1 or T2"=w55, "Trap Pos FB Negate Action"=w54, "Trap Pos. FB Offset Factor"=w53, "Trap Pos. FB Mult Factor"=w52, "Trap Pos. FB Range"=w51, "Trap Pos. FB Gains"=w50, "Force feedback"=FALSE, "AI1 X Scale"=w48, "Trap Pos to FIFO"=TRUE, "Trap Pos FB Int Count"=w43) -> ("FPGA VI Reference Out"=w95:T19, "error out"=w97:errorcluster)
  n97 = xnode "Invoke Method"("FPGA VI Reference In"=w95, "error in"=w97, "Requested Depth"="Trap AI FIFO Depth") -> ("FPGA VI Reference Out"=w58:T19, "error out"=w57:errorcluster)  [unwired: 1 out]
  n98 = xnode "Invoke Method"("FPGA VI Reference In"=w58, "error in"=w57, "Requested Depth"="Trap Position FIFO Depth") -> ("FPGA VI Reference Out"=w45:T19, "error out"=w44:errorcluster)  [unwired: 1 out]
  n99 = flat-sequence {
    tunnel: w120 -> [w258]
    tunnel: [w258] -> w119
    tunnel: [w257] -> w118
    tunnel: [w256] -> w117
    tunnel: [w254] -> w115
    tunnel: [w255] -> w116
    frame #0 {
      w255 = T16 {"Minimum"=50.0, "Maximum"=100.0, "Increment"=1.0} ("Min Max Inc")
      w254 = T16 {"Minimum"=0.0, "Maximum"=75.0, "Increment"=1.0} ("Data Entry Limits")
      w257 = T16 {"Minimum"=50.0, "Maximum"=100.0, "Increment"=1.0} ("Min Max Inc")
      w256 = T16 {"Minimum"=0.0, "Maximum"=75.0, "Increment"=1.0} ("Data Entry Limits")
      n100 = property on="BD 2 Frequency 1 (MHz)" class="DigNum (strict)"("Data Range"=w255) -> ()  [unwired: 2 in, 2 out]
      n101 = property on="BD 2 Frequency 3 (MHz)" class="DigNum (strict)"("Data Range"=w255) -> ()  [unwired: 2 in, 2 out]
      n102 = property on="BD 2 Frequency 2 (MHz)" class="DigNum (strict)"("Data Range"=w255) -> ()  [unwired: 2 in, 2 out]
      n103 = property on="BD 1 Frequency 1 (MHz)" class="DigNum (strict)"("Data Range"=w257) -> ()  [unwired: 2 in, 2 out]
      n104 = property on="BD 1 Frequency 2 (MHz)" class="DigNum (strict)"("Data Range"=w257) -> ()  [unwired: 2 in, 2 out]
      n105 = property on="BD 1 Frequency 3 (MHz)" class="DigNum (strict)"("Data Range"=w257) -> ()  [unwired: 2 in, 2 out]
      n106 = property on="BD 2 Amplitude 1 (%)" class="DigNum (strict)"("Data Range"=w254) -> ()  [unwired: 2 in, 2 out]
      n107 = property on="BD 2 Amplitude 2 (%)" class="DigNum (strict)"("Data Range"=w254) -> ()  [unwired: 2 in, 2 out]
      n108 = property on="BD 2 Amplitude 3 (%)" class="DigNum (strict)"("Data Range"=w254) -> ()  [unwired: 2 in, 2 out]
      n109 = property on="BD 1 Amplitude 3 (%)" class="DigNum (strict)"("Data Range"=w256) -> ()  [unwired: 2 in, 2 out]
      n110 = property on="BD 1 Amplitude 2 (%)" class="DigNum (strict)"("Data Range"=w256) -> ()  [unwired: 2 in, 2 out]
      n111 = property on="BD 1 Amplitude 1 (%)" class="DigNum (strict)"("Data Range"=w256) -> ()  [unwired: 2 in, 2 out]
      "X RF Frequency Limits (MHz)" <- w257
      "X RF Amplitude Limits (%)" <- w256
      "Y RF Amplitude Limits (%)" <- w254
      "Y RF Frequency Limits (MHz)" <- w255
    }
  }
  n112 = xnode "Invoke Method"("FPGA VI Reference In"=w45, "error in"=w44) -> ("FPGA VI Reference Out"=w22:T19, "error out"=w21:errorcluster)  [unwired: 1 in]
  n113 = flat-sequence "Initial FPGA Loop Relative Phase Adjustment" {
    tunnel: "Initial Phase Adjustment (APD 2 Gate)" -> [w260]
    tunnel: "Initial Phase Adjustment (GI) 2" -> [w261]
    tunnel: "Initial Phase Adj. (MCL)" -> [w262]
    tunnel: w21 -> [w263]
    tunnel: w22 -> [w264]
    tunnel: "Initial Phase Adjustment (GI)" -> [w265]
    tunnel: "Initial Phase Adjustment (AI1)" -> [w266]
    tunnel: [w266] -> w31
    tunnel: [w265] -> w30
    tunnel: [w264] -> w29
    tunnel: [w263] -> w28
    tunnel: [w262] -> w27
    tunnel: [w261] -> w26
    tunnel: [w260] -> w25
    tunnel: [w278] -> w145
    tunnel: [w272] -> w143
    tunnel: "Initial Phase Adjustment (APD Acq)" -> [w271]
    tunnel: "Initial Phase Adjustment (APD 1 Gate)" -> [w270]
    tunnel: "Initial Phase Adjustment (Green FB)" -> [w269]
    tunnel: w31 -> [w277]
    tunnel: w30 -> [w276]
    tunnel: w29 -> [w275]
    tunnel: w28 -> [w274]
    tunnel: w27 -> [w273]
    tunnel: w26 -> [w268]
    tunnel: w25 -> [w267]
    tunnel: w145 -> [w280]
    tunnel: [w281] -> w144
    tunnel: w143 -> [w281]
    tunnel: [w280] -> w142
    tunnel: w144 -> [w284]
    tunnel: w142 -> [w283]
    tunnel: [w286] -> w141
    tunnel: [w285] -> w140
    tunnel: [w288] -> w20
    tunnel: [w289] -> w23
    tunnel: w141 -> [w289]
    tunnel: w140 -> [w288]
    frame #0 {
      n114 = Wait (ms)(milliseconds to wait=u32 1000) -> ()  [unwired: 1 out]
    }
    frame #1 {
      n115 = xnode "Read/Write Control"("FPGA VI Reference In"=w275, "error in"=w274, "Phase count adjustment"=w277, "Phase count adjustment (GI)"=w276, "Phase count adjustment (MCL)"=w273, "Phase Count Adjustment (APD Acq)"=w271, "Phase count adjustment (APD 1 Gate)"=w270, "Phase count adjustment (APD 2 Gate)"=w267, "Phase count adjustment (Green FB)"=w269, "Phase count adjustment (GI) 2"=w268) -> ("FPGA VI Reference Out"=w272:T19, "error out"=w278:errorcluster)
    }
    frame #2 {
      n116 = Wait (ms)(milliseconds to wait=u32 1000) -> ()  [unwired: 1 out]
    }
    frame #3 {
      w282 = TRUE
      n117 = xnode "Read/Write Control"("FPGA VI Reference In"=w284, "error in"=w283, "+ phase"=w282, "+ phase (GI)"=w282, "+ phase (MCL)"=w282, "+ phase (APD Acq)"=w282, "+ phase (APD 1 Gate)"=w282, "+ phase (APD 2 Gate)"=w282, "+ phase (Green FB)"=w282, "+ phase (GI) 2"=w282) -> ("FPGA VI Reference Out"=w285:T19, "error out"=w286:errorcluster)
    }
    frame #4 {
      n118 = Wait (ms)(milliseconds to wait=u32 1000) -> ()  [unwired: 1 out]
    }
  }
  n119 = local read "Phase adj. (Green FB)"() -> (w113:i16)
  n120 = local read "Phase adj. (GI) 2"() -> (w83:i16)
  n121 = local read "Phase adjust (MCL)"() -> (w172:i16)
  n122 = local read "Phase adj. (AI1)"() -> (w174:i16)
  n123 = local read "Phase adj. (GI)"() -> (w173:i16)
  n124 = xnode "Read/Write Control"("FPGA VI Reference In"=w20, "error in"=w23, "Phase count adjustment"=w174, "Phase count adjustment (GI)"=w173, "Phase count adjustment (MCL)"=w172, "Phase Count Adjustment (APD Acq)"="Phase Adj. (APD Acq)", "Phase count adjustment (APD 1 Gate)"="Phase Adj. (APD 1 Gate)", "Phase count adjustment (APD 2 Gate)"="Phase Adj. (APD 2 Gate)", "Phase count adjustment (Green FB)"=w113, "Phase count adjustment (GI) 2"=w83) -> ("FPGA VI Reference Out"=w19:T19, "error out"=w18:errorcluster)
  n125 = call "Initialize RF boards - interlace 3.vi"("error in"=w18, "FPGA VI Reference In"=w19) -> ("FPGA VI Reference Out"=w150:T19)  [unwired: 1 out]
  n126 = call "set RF board frequency - interlace.vi"("Board 2 Frequency Limits"=w116, "Board 1 Frequency Limits"=w118, "FPGA VI Reference In"=w150, "Board 2 Frequency 3 (MHz)"="BD 2 Frequency 3 (MHz)", "Board 1 Frequency 3 (MHz)"="BD 1 Frequency 3 (MHz)", "Board 2 Frequency 2 (MHz)"="BD 2 Frequency 2 (MHz)", "Board 2 Frequency 1 (MHz)"="BD 2 Frequency 1 (MHz)", "Board 1 Frequency 2 (MHz)"="BD 1 Frequency 2 (MHz)", "Board 1 Frequency 1  (MHz)"="BD 1 Frequency 1 (MHz)") -> ("error out"=w244:errorcluster, "FPGA VI Reference Out"=w245:T19)  [unwired: 1 in]
  n127 = call "set RF board amplitude - interlace.vi"("Board 2 Amplitude Limits"=w115, "Board 1 Amplitude Limits"=w117, "error in"=w244, "FPGA VI Reference In"=w245, "Board 2 Amplitude 3 (%)"="BD 2 Amplitude 3 (%)", "Board 1 Amplitude 3 (%)"="BD 1 Amplitude 3 (%)", "Board 2 Amplitude 2 (%)"="BD 2 Amplitude 2 (%)", "Board 2 Amplitude 1 (%)"="BD 2 Amplitude 1 (%)", "Board 1 Amplitude 2 (%)"="BD 1 Amplitude 2 (%)", "Board 1 Amplitude 1 (%)"="BD 1 Amplitude 1 (%)") -> ("error out"=w16:errorcluster, "FPGA VI Reference Out"=w17:T19)
  n128 = flat-sequence {
    tunnel: w17 -> [w298]
    tunnel: w16 -> [w297]
    tunnel: [w296] -> w237
    tunnel: [w295] -> w236
    tunnel: [w302] -> w235
    tunnel: w237 -> [w302]
    tunnel: [w301] -> w234
    tunnel: w236 -> [w301]
    tunnel: w235 -> [w311]
    tunnel: w234 -> [w310]
    tunnel: [w309] -> w12
    tunnel: [w304] -> w11
    tunnel: [w314] -> w40
    tunnel: [w318] -> w24
    tunnel: w12 -> [w318]
    tunnel: w11 -> [w313]
    frame #0 {
      n129 = local read "Trap 1 (ON/OFF)"() -> (w290:bool)
      n130 = xnode "Read/Write Control"("FPGA VI Reference In"=w298, "error in"=w297, "Direct RF Box  Communication"=FALSE) -> ("FPGA VI Reference Out"=w296:T19, "error out"=w295:errorcluster)
      n131 = local write "Saving..."(FALSE ("Saving Data")) -> ()
      n132 = local write "Stop All"(FALSE ("Stop All")) -> ()
      n133 = local write "Index"(1.0 ("Index")) -> ()
      n134 = property on="Trap 1 ON" class="Bool (strict)"("Value"=w290) -> ()  [unwired: 2 in, 2 out]
      "Manipulating Trap" <- FALSE ("Manipulating Trap")
    }
    frame #1 {
      n135 = local read "Trap 2 (ON/OFF)"() -> (w300:bool)
      n136 = Wait (ms)(milliseconds to wait=u32 50) -> ()  [unwired: 1 out]
      n137 = property on="Trap 2 ON" class="Bool (strict)"("Val(Sgnl)"=w300) -> ()  [unwired: 2 in, 2 out]
    }
    frame #2 {
      n138 = local read "Scan Range (nm)"() -> (w305:dbl)
      n139 = xnode "Read/Write Control"("FPGA VI Reference In"=w311, "error in"=w310, "FPGA Controls  RF Box"=TRUE ("Direct RF Box  Communication")) -> ("FPGA VI Reference Out"=w309:T19, "error out"=w304:errorcluster)
      n140 = call "Update messages.vi"("Message to add"="UHR-Fleezers ready.", "Old message string"="") -> ("New message string"=w308:string)
      n141 = local write "Messages"(w308) -> ()
      n142 = property on="Scan Range (nm)" class="DigNum (strict)"("Val(Sgnl)"=w305) -> ()  [unwired: 2 in, 2 out]
    }
    frame #3 {
      n143 = call "hamilton_controller.vi"("error in"=w313, "action"=T20."CONNECT") -> ("error out"=w315:errorcluster)  [unwired: 9 in]
      n144 = call "hamilton_controller.vi"("error in"=w315, "action"=T20."INITIALIZE VALVES") -> ("error out"=w314:errorcluster)  [unwired: 9 in]
    }
  }
  n145 = Subtract(x="BD 1 Frequency 1 (MHz)", y="BD 1 Frequency 2 (MHz)") -> (x-y=w160:dbl)
  n146 = Subtract(x="BD 2 Frequency 1 (MHz)", y="BD 2 Frequency 2 (MHz)") -> (x-y=w159:dbl)
  n147 = Square(x=w159) -> (x^2=w157:dbl)
  n148 = Square(x=w160) -> (x^2=w158:dbl)
  n149 = Add(x=w158, y=w157) -> (x+y=w156:dbl)
  n150 = Square Root(x=w156) -> (sqrt(x)=w155:dbl)
  n151 = local write "Trap Delta (MHz)"(w155) -> ()
  n152 = Current VI's Path() -> (path=w1:path)
  n153 = Strip Path(path=w1) -> (stripped path=w2:path)  [unwired: 1 out]
  n154 = Build Path(base path=w2, name or relative path="Locations.txt") -> (appended path=→"Location path":path)
  n155 = Concatenate Strings("N.D.", "\r\n") -> (w5:string)
  n156 = Initialize Array(w5, 4, 3) -> (w8:string[][])
  n157 = local write "Location Matrix"(w8) -> ()
  n158 = call "IMAQ Create"("Image Name"="APD 1 Image", "Image Type"=w64) -> ("New Image"=w63:T2)  [unwired: 3 in, 1 out]
  n159 = call "IMAQ Create"("Image Name"="APD 2 Image", "Image Type"=w64) -> ("New Image"=w62:T2)  [unwired: 3 in, 1 out]
  n160 = call "IMAQ Create"("Image Name"="Det. X Image", "Image Type"=w64) -> ("New Image"=w61:T2)  [unwired: 3 in, 1 out]
  n161 = call "IMAQ Create"("Image Name"="Det. Y Image", "Image Type"=w64) -> ("New Image"=w60:T2)  [unwired: 3 in, 1 out]
  n162 = Bundle("New Image"=w63, "New Image"=w62, "New Image"=w61, "New Image"=w60) -> (w59:T21)  [unwired: 1 in]
  n163 = while {
    stop <- w319 stop-if-true
    n164 = event shown="[1] \"Goto Top (F6)\": Value Change" {
      selector: _ -> [_ _ _ _ _ _ _]
      dyn-events: _ -> [_ _ _ _ _ _ _]
      timeout: 10 -> [_ _ _ _ _ _ _]
      tunnel: [FALSE _ _ _ _ _ _] -> w319
      event Timeout {
        # "Change the trajectory mode to Jog"
        # "Query and display stage positions"
        # "Setting ESP300 left and right limits for Z-axis, input in mm"
        # "Display Selected Location"
        n165 = event-data() -> ()  [unwired: 1 in, 2 out]
        n166 = local read "ESP Port"() -> (w340:refnum<visa-resource-name>)
        n167 = Concatenate Strings("3SL" ("Substring"), "ESP ZL-Limit", ";3SR", "ESP ZR-Limit", "\r") -> (w339:string)
        n168 = VISA Write(VISA resource name=w340, write buffer=w339) -> ()  [unwired: 1 in, 3 out]
        n169 = disable-structure shown="Disabled" {
          frame Disabled {
            # "Change Low Jog Velocity"
            # "Change High Jog Velocity"
            n170 = Concatenate Strings("1JH" ("Substring"), "Axis 1", "2JH" ("Substring"), "Axis 2", "3JH" ("Substring"), "Axis 3", "\r") -> (w363:string)
            n171 = local read "ESP Port"() -> (w362:refnum<visa-resource-name>)
            n172 = VISA Write(VISA resource name=w362, write buffer=w363) -> ()  [unwired: 1 in, 3 out]
            n173 = Concatenate Strings("1JW" ("Substring"), "Axis 1", "2JW" ("Substring"), "Axis 2", "3JW" ("Substring"), "Axis 3", "\r") -> (w354:string)
            n174 = local read "ESP Port"() -> (w353:refnum<visa-resource-name>)
            n175 = VISA Write(VISA resource name=w353, write buffer=w354) -> ()  [unwired: 1 in, 3 out]
          }
          frame Enabled {
          }
        }
        n176 = local read "Location Matrix"() -> (w345:string[][])
        n177 = local read "Locations"() -> (w344:i32)
        n178 = Index Array(array=w345, index (row)=w344) -> (element=w343:string[])  [unwired: 1 in]
        n179 = Array To Cluster(array=w343) -> (cluster=w342:T22)
        n180 = local write "Selected Location"(w342) -> ()
        n181 = local read "ESP Port 8"() -> (w321:refnum<visa-resource-name>)
        n182 = Concatenate Strings("1TJ3;\n2TJ3;\n3TJ3" ("Substring"), "\r") -> (w324:string)
        n183 = VISA Write(VISA resource name=w321, write buffer=w324) -> ()  [unwired: 1 in, 3 out]
        n184 = Concatenate Strings("1TP;\n2TP;\n3TP;\n1MD?;\n2MD?;\n3MD?" ("Substring"), "\r") -> (w328:string)
        n185 = local read "ESP Port"() -> (w331:refnum<visa-resource-name>)
        n186 = VISA Write(VISA resource name=w331, write buffer=w328, error in (no error)="error in") -> (VISA resource name out=w329:refnum<visa-resource-name>, error out=w327:errorcluster)  [unwired: 1 out]
        n187 = case shown="True" TRUE ("Case Constant\n(See Context Help)") {
          tunnel: w329 -> [_ w383]
          tunnel: w327 -> [w364 w382]
          tunnel: [w364 w366] -> w333
          frame False {
          }
          frame True {
            w376 = u16 10 items=["1.0"=10, "1.5"=15, "2.0"=20] ("Serial Settings:Stop Bits")
            w377 = u16 0 items=["None", "Odd", "Even", "Mark", "Space"] ("Serial Settings:Parity")
            n188 = property class="Instr"(reference=w383, error in=w382, "Baud"=u32 921600 ("Serial Settings:Baud Rate"), "Data Bits"=u16 8 ("Serial Settings:Data Bits"), "Parity"=w377, "Stop Bits"=w376) -> (reference out=w381:refnum<visa-resource-name>, error out=w380:errorcluster, "Bytes at Port"=w365:u32)
            n189 = Wait (ms)(milliseconds to wait=u32 10) -> ()  [unwired: 1 out]
            n190 = VISA Read(VISA resource name=w381, byte count=w365, error in (no error)=w380) -> (VISA resource name out=w389:refnum<visa-resource-name>, read buffer=→"X Pos":string, error out=w390:errorcluster)  [unwired: 1 out]
            n191 = VISA Read(VISA resource name=w389, byte count=w365, error in (no error)=w390) -> (VISA resource name out=w387:refnum<visa-resource-name>, read buffer=→"Y Pos":string, error out=w388:errorcluster)  [unwired: 1 out]
            n192 = VISA Read(VISA resource name=w387, byte count=w365, error in (no error)=w388) -> (VISA resource name out=w375:refnum<visa-resource-name>, read buffer=→"Z Pos Pos":string, error out=w374:errorcluster)  [unwired: 1 out]
            n193 = VISA Read(VISA resource name=w375, byte count=w365, error in (no error)=w374) -> (VISA resource name out=w371:refnum<visa-resource-name>, read buffer=→"X Motion":string, error out=w372:errorcluster)  [unwired: 1 out]
            n194 = VISA Read(VISA resource name=w371, byte count=w365, error in (no error)=w372) -> (VISA resource name out=w370:refnum<visa-resource-name>, read buffer=→"Y Motion":string, error out=w368:errorcluster)  [unwired: 1 out]
            n195 = VISA Read(VISA resource name=w370, byte count=w365, error in (no error)=w368) -> (read buffer=→"Z motion":string, error out=w366:errorcluster)  [unwired: 2 out]
          }
        }
        "error out" <- w333
      }
      event "Goto Top (F6)": Value Change {
        n196 = event-data() -> ()  [unwired: 1 in, 5 out]
        n197 = stacked-sequence {
          frame #0 {
            # "stop motions of all axes before going to avoid reversing of direction"
            n198 = local read "ESP Port"() -> (w395:refnum<visa-resource-name>)
            n199 = Concatenate Strings("ST" ("Substring"), "\r") -> (w392:string)
            n200 = VISA Write(VISA resource name=w395, write buffer=w392) -> ()  [unwired: 1 in, 3 out]
          }
          frame #1 {
            n201 = Wait (ms)(milliseconds to wait=u32 50) -> ()  [unwired: 1 out]
          }
          frame #2 {
            # "Change the trajectory mode to Trapezoidal"
            n202 = local read "ESP Port"() -> (w400:refnum<visa-resource-name>)
            n203 = Concatenate Strings("1TJ1;\n2TJ1;\n3TJ1" ("Substring"), "\r") -> (w397:string)
            n204 = VISA Write(VISA resource name=w400, write buffer=w397) -> ()  [unwired: 1 in, 3 out]
          }
          frame #3 {
            # "Go to Top Dispensor"
            n205 = local read "Location Matrix"() -> (w412:string[][])
            n206 = Index Array(array=w412, index (row)=0) -> (element=w408:string[])  [unwired: 1 in]
            n207 = Decimate 1D Array(w408) -> (w406:string[], w404:string[], w402:string[])
            n208 = Concatenate Strings("1PA" ("Substring"), w406, "2PA" ("Substring"), w404, "3PA" ("Substring"), w402, "\r") -> (w410:string)
            n209 = local read "ESP Port"() -> (w409:refnum<visa-resource-name>)
            n210 = VISA Write(VISA resource name=w409, write buffer=w410) -> ()  [unwired: 1 in, 3 out]
          }
          frame #4 {
            n211 = Wait (ms)(milliseconds to wait=u32 100) -> ()  [unwired: 1 out]
          }
          frame #5 {
            # "Change the trajectory mode to Jog"
            n212 = local read "ESP Port 2"() -> (w417:refnum<visa-resource-name>)
            n213 = Concatenate Strings("1TJ3;\n2TJ3;\n3TJ3" ("Substring"), "\r") -> (w414:string)
            n214 = VISA Write(VISA resource name=w417, write buffer=w414) -> ()  [unwired: 1 in, 3 out]
          }
        }
      }
      event "Goto Exp (F8)": Value Change {
        n215 = event-data() -> ()  [unwired: 1 in, 5 out]
        n216 = stacked-sequence {
          frame #0 {
            # "stop motions of all axes before going to avoid reversing of direction"
            n217 = local read "ESP Port"() -> (w421:refnum<visa-resource-name>)
            n218 = Concatenate Strings("ST" ("Substring"), "\r") -> (w418:string)
            n219 = VISA Write(VISA resource name=w421, write buffer=w418) -> ()  [unwired: 1 in, 3 out]
          }
          frame #1 {
            n220 = Wait (ms)(milliseconds to wait=u32 50) -> ()  [unwired: 1 out]
          }
          frame #2 {
            # "Change the trajectory mode to Trapezoidal"
            n221 = local read "ESP Port"() -> (w426:refnum<visa-resource-name>)
            n222 = Concatenate Strings("1TJ1;\n2TJ1;\n3TJ1" ("Substring"), "\r") -> (w423:string)
            n223 = VISA Write(VISA resource name=w426, write buffer=w423) -> ()  [unwired: 1 in, 3 out]
          }
          frame #3 {
            # "Go to Experimental"
            n224 = local read "Location Matrix"() -> (w438:string[][])
            n225 = Index Array(array=w438, index (row)=2) -> (element=w434:string[])  [unwired: 1 in]
            n226 = Decimate 1D Array(w434) -> (w432:string[], w430:string[], w428:string[])
            n227 = Concatenate Strings("1PA" ("Substring"), w432, "2PA" ("Substring"), w430, "3PA" ("Substring"), w428, "\r") -> (w436:string)
            n228 = local read "ESP Port"() -> (w435:refnum<visa-resource-name>)
            n229 = VISA Write(VISA resource name=w435, write buffer=w436) -> ()  [unwired: 1 in, 3 out]
          }
          frame #4 {
            n230 = Wait (ms)(milliseconds to wait=u32 100) -> ()  [unwired: 1 out]
          }
          frame #5 {
            # "Change the trajectory mode to Jog"
            n231 = local read "ESP Port 3"() -> (w440:refnum<visa-resource-name>)
            n232 = Concatenate Strings("1TJ3;\n2TJ3;\n3TJ3" ("Substring"), "\r") -> (w443:string)
            n233 = VISA Write(VISA resource name=w440, write buffer=w443) -> ()  [unwired: 1 in, 3 out]
          }
        }
      }
      event "Goto Bottom (F7)": Value Change {
        n234 = event-data() -> ()  [unwired: 1 in, 5 out]
        n235 = stacked-sequence {
          frame #0 {
            # "stop motions of all axes before going to avoid reversing of direction"
            n236 = local read "ESP Port"() -> (w447:refnum<visa-resource-name>)
            n237 = Concatenate Strings("ST" ("Substring"), "\r") -> (w444:string)
            n238 = VISA Write(VISA resource name=w447, write buffer=w444) -> ()  [unwired: 1 in, 3 out]
          }
          frame #1 {
            n239 = Wait (ms)(milliseconds to wait=u32 50) -> ()  [unwired: 1 out]
          }
          frame #2 {
            # "Change the trajectory mode to Trapezoidal"
            n240 = local read "ESP Port"() -> (w452:refnum<visa-resource-name>)
            n241 = Concatenate Strings("1TJ1;\n2TJ1;\n3TJ1" ("Substring"), "\r") -> (w449:string)
            n242 = VISA Write(VISA resource name=w452, write buffer=w449) -> ()  [unwired: 1 in, 3 out]
          }
          frame #3 {
            # "Go to Bottom Dispensor"
            n243 = local read "Location Matrix"() -> (w464:string[][])
            n244 = Index Array(array=w464, index (row)=1) -> (element=w460:string[])  [unwired: 1 in]
            n245 = Decimate 1D Array(w460) -> (w458:string[], w456:string[], w454:string[])
            n246 = Concatenate Strings("1PA" ("Substring"), w458, "2PA" ("Substring"), w456, "3PA" ("Substring"), w454, "\r") -> (w462:string)
            n247 = local read "ESP Port"() -> (w461:refnum<visa-resource-name>)
            n248 = VISA Write(VISA resource name=w461, write buffer=w462) -> ()  [unwired: 1 in, 3 out]
          }
          frame #4 {
            n249 = Wait (ms)(milliseconds to wait=u32 100) -> ()  [unwired: 1 out]
          }
          frame #5 {
            # "Change the trajectory mode to Jog"
            n250 = local read "ESP Port 4"() -> (w466:refnum<visa-resource-name>)
            n251 = Concatenate Strings("1TJ3;\n2TJ3;\n3TJ3" ("Substring"), "\r") -> (w469:string)
            n252 = VISA Write(VISA resource name=w466, write buffer=w469) -> ()  [unwired: 1 in, 3 out]
          }
        }
      }
      event "Capture": Value Change {
        n253 = event-data() -> ()  [unwired: 1 in, 5 out]
        n254 = local read "Locations"() -> (w470:i32)
        n255 = local read "Z Pos Pos"() -> (w471:string)
        n256 = local read "X Pos"() -> (w473:string)
        n257 = local read "Y Pos"() -> (w472:string)
        n258 = case shown="1" w470 {
          selector: w470 -> [w477 w484 w491 w498]
          tunnel: w473 -> [w480 w487 w494 w501]
          tunnel: w472 -> [w479 w486 w493 w500]
          tunnel: w471 -> [w478 w485 w492 w499]
          frame 0, Default {
            # "Capture Top Dispensor Location"
            n259 = local read "Location Matrix"() -> (w476:string[][])
            n260 = Build Array(w480, w479, w478) -> (w475:string[])
            n261 = Replace Array Subset(array=w476, new element=w475, index (row)=w477) -> (w474:string[][])  [unwired: 1 in]
            n262 = local write "Location Matrix"(w474) -> ()
          }
          frame 1 {
            # "Capture Bottom Dispensor Location"
            n263 = local read "Location Matrix"() -> (w483:string[][])
            n264 = Build Array(w487, w486, w485) -> (w482:string[])
            n265 = Replace Array Subset(array=w483, new element=w482, index (row)=w484) -> (w481:string[][])  [unwired: 1 in]
            n266 = local write "Location Matrix"(w481) -> ()
          }
          frame 2 {
            # "Capture Experimental Region Location"
            n267 = local read "Location Matrix"() -> (w490:string[][])
            n268 = Build Array(w494, w493, w492) -> (w489:string[])
            n269 = Replace Array Subset(array=w490, new element=w489, index (row)=w491) -> (w488:string[][])  [unwired: 1 in]
            n270 = local write "Location Matrix"(w488) -> ()
          }
          frame 3 {
            # "Capture Other Location"
            n271 = local read "Location Matrix"() -> (w497:string[][])
            n272 = Build Array(w501, w500, w499) -> (w496:string[])
            n273 = Replace Array Subset(array=w497, new element=w496, index (row)=w498) -> (w495:string[][])  [unwired: 1 in]
            n274 = local write "Location Matrix"(w495) -> ()
          }
        }
      }
      event "Save": Value Change {
        # "reshape Location Matrix to 1-D array to write"
        n275 = event-data() -> ()  [unwired: 1 in, 5 out]
        n276 = local read "Location Matrix"() -> (w505:string[][])
        n277 = local read "Location path"() -> (w502:path)
        n278 = Reshape Array(w505, 12) -> (w503:string[])
        n279 = Write to Text File(file (use dialog)=w502, text=w503) -> ()  [unwired: 2 in, 3 out]
      }
      event "Activate Joystick": Value Change {
        # "Change the trajectory mode to Jog"
        n280 = event-data() -> ()  [unwired: 1 in, 5 out]
        n281 = disable-structure shown="Disabled" {
          frame Disabled {
            n282 = case shown="True" "Activate Joystick" {
              frame False {
              }
              frame True {
                # "Change the trajectory mode to Jog"
                n283 = local read "ESP Port"() -> (w514:refnum<visa-resource-name>)
                n284 = Concatenate Strings("1TJ3;\n2TJ3;\n3TJ3" ("Substring"), "\r") -> (w511:string)
                n285 = VISA Write(VISA resource name=w514, write buffer=w511) -> ()  [unwired: 1 in, 3 out]
              }
            }
          }
          frame Enabled {
          }
        }
        n286 = local read "ESP Port 5"() -> (w509:refnum<visa-resource-name>)
        n287 = Concatenate Strings("1TJ3;\n2TJ3;\n3TJ3" ("Substring"), "\r") -> (w506:string)
        n288 = VISA Write(VISA resource name=w509, write buffer=w506) -> ()  [unwired: 1 in, 3 out]
      }
    }
  }
  n289 = disable-structure shown="Disabled" {
    disable-tunnel: w24 -> [w543 _]
    frame Disabled {
      w538 = T17 0 items=["Grayscale (U8)", "Grayscale (I16)", "Grayscale (SGL)", "Complex (CSG)", "RGB (U32)", "HSL (U32)", "RGB (U64)", "Grayscale (U16)"] ("Image Type")
      n290 = call <vilib>:"IMAQ Init.vi"("Interface Name"="img0") -> ("error out"=w540:errorcluster, "IMAQ Session Out"=w542:refnum<k11>)  [unwired: 9 in]
      n291 = call <vilib>:"IMAQ Grab Setup.vi"("error in (no error)"=w540, "IMAQ Session In"=w542) -> ("error out"=w536:errorcluster, "IMAQ Session Out"=w537:refnum<k11>)  [unwired: 8 in]
      n292 = call "IMAQ Create"("Image Name"="untitled", "Image Type"=w538) -> ("New Image"=w535:T2)  [unwired: 3 in, 1 out]
      n293 = call <vilib>:"Application Directory.vi"() -> ("Application Directory"=w522:path)
      n294 = Build Path(base path=w522, name or relative path="_trap_screen_positions") -> (appended path=w530:path)
      n295 = Open/Create/Replace File(file path (use dialog)=w530, operation (0:open)=T23."open or create", access (0:read/write)=enum16{"read/write", "read-only", "write-only"}."read/write") -> (refnum out=w532:refnum<file>)  [unwired: 3 in, 2 out]
      n296 = local read "Trap Sets"() -> (w524:u32)
      n297 = for "Load trap positions on video screen from file." {
        N: w524 -> [_]
        tunnel: [w550] -> w525
        tunnel: w532 -> [w549]
        tunnel: [w546] -> w521 mode=indexing
        w548 = 4
        n298 = for {
          N: w548 -> [_]
          tunnel: [w554] -> w550
          tunnel: w549 -> [w553]
          tunnel: w548 -> [w552]
          tunnel: [w551] -> w547 mode=indexing
          n299 = Read from Binary File(5:w552, 11:w553) -> (2:w551:i32, 3:w554:refnum<file>)  [unwired: 4 in, 2 out]
        }
        n300 = Array To Cluster(array=w547) -> (cluster=w546:T27)
      }
      n301 = node-c288() -> (w545:T24)  [unwired: 4 in]
      n302 = timed-loop "acquire video and stage position" {
        timing: w545 -> [_]
        timing-out: [_] -> w544
        tunnel: w537 -> [w573]
        tunnel: w536 -> [w572]
        tunnel: w535 -> [w571]
        tunnel: [w570] -> w517
        tunnel: [w567] -> w518
        tunnel: [w568] -> w516
        tunnel: w543 -> [_]
        shift-right: [w564] -> w534
        shift-left: w521 -> [w565]
        tunnel: w524 -> [w562]
        stop <- w569 stop-if-true
        n303 = node-c288() -> ()  [unwired: 1 in, 1 out]
        n304 = event shown="[2] \"Primary Video Display\": Mouse Down" {
          selector: _ -> [_ _ _ _]
          dyn-events: _ -> [_ _ _ _]
          timeout: 10 -> [_ _ _ _]
          tunnel: w573 -> [w584 w599 w608 w627]
          tunnel: w572 -> [w583 w601 w606 w629]
          tunnel: w571 -> [w582 w600 w607 w628]
          tunnel: [w581 w599 w608 w627] -> w570
          tunnel: [w574 w603 FALSE FALSE] -> w569
          tunnel: [w578 w601 w606 w629] -> w568
          tunnel: [w577 w600 w607 w628] -> w567
          tunnel: "radius" -> [_ _ w613 _]
          tunnel: w565 -> [w575 w602 w611 _]
          tunnel: [w575 w602 w612 cluster{i32, i32, i32, i32}[] []] -> w564
          tunnel: w562 -> [_ _ w604 _]
          event Timeout {
            n305 = event-data() -> ()  [unwired: 1 in, 2 out]
            n306 = call <vilib>:"IMAQ Grab Acquire.vi"("error in (no error)"=w583, "Image In"=w582, "IMAQ Session In"=w584) -> ("error out"=w579:errorcluster, "Image Out"=w580:T2, "IMAQ Session Out"=w581:refnum<k11>)  [unwired: 5 in, 1 out]
            n307 = case shown="True" "trap\nmarkers?" {
              tunnel: w575 -> [_ w592]
              tunnel: w580 -> [w586 w591]
              tunnel: w579 -> [w585 w590]
              tunnel: [w585 w589] -> w578
              tunnel: [w586 w587] -> w577
              frame False {
              }
              frame True {
                n308 = for {
                  tunnel: w592 -> [w598] mode=indexing
                  shift-right: [w596] -> w587
                  shift-left: w591 -> [w597]
                  tunnel: w590 -> [w595]
                  tunnel: [w594] -> w589
                  tunnel: u32 16711680 ("Color") -> [w593]
                  n309 = call "IMAQ Overlay Oval"("Color"=w593, "error in (no error)"=w595, "Bounding Rectangle"=w598, "Image"=w597) -> ("error out"=w594:errorcluster, "Image Out"=w596:T2)  [unwired: 6 in]
                }
              }
            }
            "Primary Video Display" <- w577
            n310 = Unbundle By Name(w579) -> ("status"=w574:bool)
          }
          event "Stop All": Value Change {
            n311 = event-data() -> ()  [unwired: 1 in, 5 out]
            n312 = local read "Stop All"() -> (w603:bool)
          }
          event "Primary Video Display": Mouse Down {
            n313 = event-data() -> ()  [unwired: 1 in, 7 out]
            n314 = Array Size(array=w611) -> (size(s)=w610:i32)
            n315 = Less?(x=w610, y=w604) -> (x < y?=w609:bool)
            n316 = case shown="True" w609 {
              tunnel: w613 -> [_ w623]
              tunnel: w611 -> [w614 w617]
              tunnel: [w614 w616] -> w612
              frame False {
              }
              frame True {
                n317 = property on="Primary Video Display" class="ImageControl"() -> ("Last Mouse Position"=w615:cluster{"X":i32, "Y":i32})  [unwired: 2 in, 2 out]
                n318 = Unbundle By Name(w615) -> ("X"=w625:i32, "Y"=w624:i32)
                n319 = Add(x=w624, y=w623) -> (x+y=w621:i32)
                n320 = Subtract(x=w624, y=w623) -> (x-y=w619:i32)
                n321 = Add(x=w625, y=w623) -> (x+y=w620:i32)
                n322 = Subtract(x=w625, y=w623) -> (x-y=w622:i32)
                n323 = Bundle(w622, w621, w620, w619) -> (w618:cluster{i32, i32, i32, i32})  [unwired: 1 in]
                n324 = Build Array (concatenate)(w617, w618) -> (w616:T28)
              }
            }
          }
          event "clear markers": Value Change {
            n325 = event-data() -> ()  [unwired: 1 in, 5 out]
          }
        }
        n326 = node-c288() -> ()  [unwired: 1 in, 1 out]
      }
      n327 = node-c288(w544) -> ()  [unwired: 1 out]
      n328 = Set File Position(offset (in bytes) (0)=i64 0, refnum=w525, from (0:start)=enum16{"start", "end", "current"}."start") -> (refnum out=w526:refnum<file>)  [unwired: 1 in, 1 out]
      n329 = for "Write trap positions to file so they can be remembered\nwhen program is removed from memory" {
        tunnel: w534 -> [w558] mode=indexing
        tunnel: [w556] -> w533
        tunnel: w526 -> [w555]
        n330 = Cluster To Array(cluster=w558) -> (array=w557:i32[])
        n331 = for {
          tunnel: w557 -> [w561] mode=indexing
          tunnel: [w560] -> w556
          tunnel: w555 -> [w559]
          n332 = Write to Binary File(file (use dialog)=w559, data=w561) -> (refnum out=w560:refnum<file>)  [unwired: 4 in, 2 out]
        }
      }
      n333 = Close File(refnum=w533) -> ()  [unwired: 1 in, 2 out]
      n334 = call "IMAQ Dispose"("Image"=w518, "error in (no error)"=w516) -> ("error out"=w515:errorcluster)  [unwired: 4 in]
      n335 = call <vilib>:"IMAQ Stop.vi"("error in (no error)"=w515, "IMAQ Session In"=w517) -> ("error out"=w519:errorcluster, "IMAQ Session Out"=w520:refnum<k11>)  [unwired: 8 in]
      n336 = call <vilib>:"IMAQ Close.vi"("error in (no error)"=w519, "IMAQ Session In"=w520) -> ()  [unwired: 9 in, 1 out]
    }
    frame Enabled {
    }
  }
  n337 = disable-structure shown="Enabled" {
    disable-tunnel: [w636 _] -> w35
    disable-tunnel: w24 -> [w635 _]
    frame Enabled {
      n338 = node-c288() -> (w638:T24)  [unwired: 4 out]
      n339 = timed-loop "Rough control of MCL mirror stage (debugging)" {
        tunnel: w635 -> [w641]
        tunnel: [w640] -> w636
        timing: w638 -> [_]
        timing-out: [_] -> w637
        stop <- w640 stop-if-true
        n340 = node-c288() -> ()  [unwired: 2 out]
        n341 = case shown="0, Default" "MCL Mode" {
          tunnel: w641 -> [_ w644 w691]
          frame 0, Default {
            # "manual positioning"
          }
          frame 1 {
            # "sinusoidal wave"
            n342 = node-c288() -> (w646:T24)  [unwired: 4 out]
            n343 = timed-loop "Oscillate MCL mirror" {
              timing: w646 -> [_]
              timing-out: [_] -> w645
              tunnel: w644 -> [w685]
              i -> [w684]
              stop <- w647 stop-if-true
              n344 = node-c288() -> (w683:i64)  [unwired: 1 out]
              n345 = Multiply(x="AO1", y=32767.0) -> (x*y=w679:dbl)
              n346 = Multiply(x="AO2", y=32767.0) -> (x*y=w674:dbl)
              n347 = Divide(x=w679, y=10.0) -> (x/y=w680:dbl)
              n348 = Divide(x=w674, y=10.0) -> (x/y=w675:dbl)
              n349 = To Word Integer(number=w680) -> (16bit integer=w672:i16)
              n350 = To Word Integer(number=w675) -> (16bit integer=w671:i16)
              n351 = Divide(x=w683, y=i64 1000) -> (x/y=w654:dbl)
              n352 = Multiply(x=w654, y=w684) -> (x*y=w665:dbl)
              n353 = Multiply(x="Osc. freq. (Hz) 2", y=6.283185307179586) -> (x*y=w666:dbl)
              n354 = Multiply(x=w666, y=w665) -> (x*y=w664:dbl)
              n355 = Sine(x=w664) -> (sin(x)=w663:dbl)
              n356 = Multiply(x=w663, y="Osc. amp. (V)") -> (x*y=w661:dbl)
              n357 = Add(x=w661, y="Osc. center (V)") -> (x+y=w659:dbl)
              n358 = Divide(x=w659, y=10.0) -> (x/y=w657:dbl)
              n359 = Multiply(x=w657, y=32767.0) -> (x*y=w652:dbl)
              n360 = Select(t=w652, s="Scan axis", f=w672) -> (s? t:f=w670:dbl)
              n361 = Select(t=w671, s="Scan axis", f=w652) -> (s? t:f=w669:dbl)
              n362 = local read "MCL Mode"() -> (w651:u16)
              n363 = Not Equal?(x=w651, y=u16 1) -> (x != y?=w648:bool)
              n364 = local read "Stop All"() -> (w649:bool)
              n365 = xnode "Read/Write Control"("FPGA VI Reference In"=w685, "AO1"=w670, "AO2"=w669) -> ()  [unwired: 1 in, 2 out]
              n366 = Compound Arithmetic op=OR(w649, w648) -> (w647:bool)
              n367 = node-c288() -> ()  [unwired: 2 out]
            }
            n368 = node-c288(w645) -> ()  [unwired: 1 out]
          }
          frame 2 {
            # "linear scan"
            n369 = case shown="True" "Start Scan" {
              tunnel: w691 -> [_ w703]
              frame False {
              }
              frame True {
                n370 = Subtract(x="End (V)", y="Begin (V)") -> (x-y=w699:dbl)
                n371 = Decrement(x="N Points") -> (x-1=w698:dbl)
                n372 = Divide(x=w699, y=w698) -> (x/y=w696:dbl)
                n373 = for {
                  N: "N Points" -> [_]
                  tunnel: "Begin (V)" -> [w716]
                  tunnel: w703 -> [w708]
                  tunnel: [w707] -> w702 mode=indexing
                  tunnel: w696 -> [w706]
                  tunnel: [w704] -> w695 mode=indexing
                  i -> [w715]
                  n374 = Multiply(x=w706, y=w715) -> (x*y=w714:dbl)
                  n375 = Add(x=w716, y=w714) -> (x+y=w711:dbl)
                  n376 = local read "Scan axis"() -> (w705:bool)
                  n377 = local read "AO1"() -> (w713:dbl)
                  n378 = local read "AO2"() -> (w712:dbl)
                  n379 = Select(t=w711, s=w705, f=w713) -> (s? t:f=w710:dbl)
                  n380 = Select(t=w712, s=w705, f=w711) -> (s? t:f=w709:dbl)
                  n381 = flat-sequence {
                    tunnel: w710 -> [w720]
                    tunnel: w709 -> [w719]
                    tunnel: w708 -> [w717]
                    tunnel: [w730] -> w707
                    tunnel: [w729] -> w704
                    frame #0 {
                      w723 = 10.0 ("y")
                      w718 = 32767.0 ("y")
                      n382 = Multiply(x=w720, y=w718) -> (x*y=w726:dbl)
                      n383 = Multiply(x=w719, y=w718) -> (x*y=w724:dbl)
                      n384 = Divide(x=w726, y=w723) -> (x/y=w727:dbl)
                      n385 = Divide(x=w724, y=w723) -> (x/y=w725:dbl)
                      n386 = To Word Integer(number=w727) -> (16bit integer=w721:i16)
                      n387 = To Word Integer(number=w725) -> (16bit integer=w722:i16)
                      n388 = xnode "Read/Write Control"("FPGA VI Reference In"=w717, "AO1"=w721, "AO2"=w722) -> ()  [unwired: 1 in, 2 out]
                    }
                    frame #1 {
                      n389 = Wait (ms)(milliseconds to wait="DAQ Delay (ms)") -> ()  [unwired: 1 out]
                    }
                    frame #2 {
                      n390 = local read "Slow mean"() -> (w730:dbl)
                      n391 = local read "Sigma"() -> (w729:dbl)
                    }
                  }
                }
                n392 = Bundle("Begin (V)"="Begin (V)", w696, w702) -> (→"MCL Scan":cluster{"Begin (V)":dbl, dbl, dbl[]})  [unwired: 1 out]
                n393 = Bundle("Begin (V)"="Begin (V)", w696, w695) -> (→"MCL Scan 2":cluster{"Begin (V)":dbl, dbl, dbl[]})  [unwired: 1 out]
              }
            }
          }
        }
        n394 = local read "Stop All"() -> (w640:bool)
        n395 = node-c288() -> ()  [unwired: 2 out]
      }
      n396 = node-c288(w637) -> ()  [unwired: 1 out]
    }
    frame Disabled {
    }
  }
  n397 = node-c288(2 ("Processor")) -> (w15:T24)  [unwired: 3 in]
  n398 = timed-loop "Control parameters (event loop)" {
    tunnel: w24 -> [w736]
    shift-right: [w735] -> _
    shift-left: errorcluster {"status"=FALSE, "code"=0, "source"=""} ("error out") -> [w734]
    tunnel: [w733] -> w37
    timing: w15 -> [_]
    timing-out: [_] -> w14
    stop <- w733 stop-if-true
    n399 = node-c288() -> ()  [unwired: 1 in, 1 out]
    n400 = event shown="[6] \"BD 1 Frequency 1 (MHz)\", \"BD 1 Frequency 2 (MHz)\", \"BD 1 Frequency 3 (MHz)\", \"BD 2 Frequency 1 (MHz)\", \"BD 2 Frequency 2 (MHz)\", \"BD 2 Frequency 3 (MHz)\", \"Trap Delta (MHz)\": Value Change" {
      selector: _ -> [_ _ _ _ _ _ _ _ _ _ _ _ _ _ _ _ _ _ _ _ _ _ _ _ _ _ _ _ _ _ _ _ _ _ _ _ _ _ _ _ _ _ _ _ _ _ _ _ _ _ _ _ _ _ _]
      dyn-events: _ -> [_ _ _ _ _ _ _ _ _ _ _ _ _ _ _ _ _ _ _ _ _ _ _ _ _ _ _ _ _ _ _ _ _ _ _ _ _ _ _ _ _ _ _ _ _ _ _ _ _ _ _ _ _ _ _]
      timeout: _ -> [_ _ _ _ _ _ _ _ _ _ _ _ _ _ _ _ _ _ _ _ _ _ _ _ _ _ _ _ _ _ _ _ _ _ _ _ _ _ _ _ _ _ _ _ _ _ _ _ _ _ _ _ _ _ _]
      tunnel: w736 -> [w774 _ _ _ w811 _ w833 _ w897 _ _ _ w940 _ _ w983 w989 w994 w1000 w1036 w1054 w1061 w1079 w1090 w1101 w1112 w1123 w1134 w1152 w1158 w1252 _ w1261 w1299 _ w1334 w1338 w1349 w1353 w1357 _ w1365 _ _ _ _ w1498 _ w1515 w1518 w1527 w1530 w1534 _ w1551]
      tunnel: [w773 _ _ _ w801 _ w832 _ w860 _ w905 _ w919 _ _ w982 w985 w991 w997 w1035 w1052 w1060 w1073 w1084 w1095 w1106 w1117 w1128 w1150 w1157 w1250 _ w1259 w1297 _ w1332 w1336 w1339 w1351 w1355 _ w1363 _ _ _ _ w1496 _ _ _ _ _ _ _ _] -> w735
      tunnel: w734 -> [w772 _ _ _ w810 _ w831 _ w892 _ w905 _ w939 _ _ w981 w984 w990 w996 w1034 w1053 w1059 w1078 w1089 w1100 w1111 w1122 w1133 w1151 w1156 w1251 _ w1260 w1298 _ w1333 w1337 w1348 w1352 w1356 _ w1364 _ _ _ _ w1497 _ w1514 w1517 w1526 w1529 w1533 _ w1550]
      tunnel: [_ _ _ _ _ _ _ _ _ _ w904 _ _ _ _ _ _ _ _ _ _ _ _ _ _ _ _ _ _ _ _ _ _ _ _ _ _ _ _ _ _ _ _ _ _ _ _ _ _ _ _ _ _ _ _] -> w733
      tunnel: [_ _ _ _ _ _ _ "Round T1 X" _ _ _ _ _ _ _ _ _ _ _ _ _ _ _ _ _ _ _ _ _ _ _ _ _ _ _ _ _ _ _ _ _ _ _ _ _ _ _ _ _ _ _ _ _ _ _] -> _
      tunnel: [_ _ _ "Adjust Scale\nto Mean" _ _ _ _ _ _ _ _ _ _ _ _ _ _ _ _ _ _ _ _ _ _ _ _ _ _ _ _ _ _ _ _ _ _ _ _ _ _ _ _ _ _ _ _ _ _ _ _ "Set SP to Reading" _ _] -> _
      tunnel: [_ _ _ _ _ _ _ _ _ "Round T2 X" _ "Delayed Interlace Start" _ _ _ _ _ _ _ _ _ _ _ _ _ _ _ _ _ _ _ _ _ _ _ _ _ _ _ _ _ _ _ _ _ _ _ _ _ _ _ _ _ _ _] -> _
      event "AI Count (ticks)", "Sets to FIFO (Traps)", "Save ave N", "FPGA Ave.", "# Samples/channel", "N sets to save": Value Change {
        # "So that if 'Save ave N' is updated, the AOD scanning code updates too."
        n401 = event-data() -> ()  [unwired: 6 out]
        n402 = local read "AI Count (ticks)"() -> (w754:u32)
        n403 = Boolean To (0,1)(Boolean="Sets to FIFO (Traps)") -> (0, 1=w764:cluster{"Set 1":i16, "Set 2":i16, "Set 3":i16})
        n404 = xnode "Read/Write Control"("FPGA VI Reference In"=w774, "error in"=w772, "ai count"=w754, "AI1 Sets to FIFO"="Sets to FIFO (Traps)", "N of AI1 Int Acq Sets"="N Acq Sets (Traps + Fl.)") -> ("error out"=w773:errorcluster)  [unwired: 1 out]
        n405 = Cluster To Array(cluster=w764) -> (array=w763:i16[])
        n406 = To Unsigned Long Integer(number=w763) -> (unsigned 32bit integer=w743:u32[])
        n407 = local read "Scan steps (AOD)"() -> (w765:u64)
        n408 = Multiply(x=w754, y="N Acq Sets (Traps + Fl.)") -> (x*y=w752:u32)
        n409 = Divide(x=40000000.0, y=w754) -> (x/y=w746:dbl)
        "AI rate (Hz)" <- w746
        "Ave. Rate (Hz)" <- w746
        n410 = Add Array Elements(numeric array=w743) -> (sum=w755:u32)
        "Trap Sets" <- w755
        n411 = Reciprocal(x=w746) -> (1/x=→"Ave. Period (s)":dbl)
        n412 = property on="Scan steps (AOD)" class="DigNum (strict)"("Val(Sgnl)"=w765) -> ()  [unwired: 2 in, 2 out]
        n413 = Divide(x=w746, y="N Acq Sets (Traps + Fl.)") -> (x/y=w769:dbl)
        "Data Rate (Hz)" <- w769
        n414 = Reciprocal(x=w769) -> (1/x=→"Data Period (s)":dbl)
        n415 = local read "Save ave N"() -> (w768:dbl)
        n416 = Divide(x=w769, y=w768) -> (x/y=w767:dbl)
        "Save Data Rate (Hz)" <- w767
        n417 = Reciprocal(x=w767) -> (1/x=→"Save Data Period (s)":dbl)
        n418 = Multiply(x=w752, y="# Samples/trap") -> (x*y=w750:u32)
        "Counts/DMA" <- w750
        n419 = property on="Trap Disp. Downsample" class="DigNum (strict)"("Maximum"="# Samples/trap") -> ()  [unwired: 2 in, 2 out]
        n420 = Multiply(x=w755, y="# Samples/trap") -> (x*y=w744:u32)
        "# Samples/channel" <- w744
        n421 = Multiply(x=w744, y=u32 8) -> (x*y=→"Trap AI Elements/DMA read":u32)
        n422 = local read "APD Int. Count"() -> (w751:u32)
        n423 = Multiply(x=w744, y=u32 3) -> (x*y=→"Trap Pos Elements/DMA read":u32)
        n424 = Divide(x=w750, y=w751) -> (x/y=w741:dbl)
        "APD Samples/FIFO Acq." <- w741
        n425 = Divide(x=w750, y=40000000.0) -> (x/y=w748:dbl)
        "DMA Update Period (s)" <- w748
        n426 = Multiply(x=2.0, y=w741) -> (x*y=→"APD Elements/DMA read":dbl)
        n427 = property on="APD Disp. Downsample" class="DigNum (strict)"("Maximum"=w741) -> ()  [unwired: 2 in, 2 out]
        n428 = local read "N sets to save"() -> (w761:u32)
        n429 = Multiply(x=w748, y=w761) -> (x*y=→"Total Time (s)":dbl)
        "FPGA Averaging" <- FALSE ("FPGA Averaging")
      }
      event "Rescale on Mean": Value Change {
        n430 = event-data() -> ()  [unwired: 7 out]
        n431 = And(x=FALSE, y="Rescale on Mean") -> (x .and. y?=w776:bool)
        n432 = local write "Rescale on Mean"(w776) -> ()
        n433 = local read "Bead Mean (nm)"() -> (w781:dbl)
        n434 = Add(x="Amplitude (nm)", y=w781) -> (x+y=w779:dbl)
        n435 = Subtract(x=w781, y="Amplitude (nm)") -> (x-y=w778:dbl)
        n436 = property on="Bead Separation" class="WFChart (strict)"("YScale.Minimum"=w778) -> ()  [unwired: 2 in, 2 out]
        n437 = property on="Bead Separation" class="WFChart (strict)"("YScale.Maximum"=w779) -> ()  [unwired: 2 in, 2 out]
      }
      event "Detector Type": Value Change {
        n438 = event-data() -> ()  [unwired: 7 out]
        n439 = local read "AI labels"() -> (w782:string[])
        n440 = property on="High Res. Display" class="Ring (strict)"("Strings []"=w782) -> ()  [unwired: 2 in, 2 out]
        n441 = Build Array (concatenate)(w782, "none") -> (w783:string[])
        n442 = property on="FFT 1 Choice 1" class="Ring (strict)"("Strings []"=w783) -> ()  [unwired: 2 in, 2 out]
        n443 = property on="FFT 1 Choice 2" class="Ring (strict)"("Strings []"=w783) -> ()  [unwired: 2 in, 2 out]
        n444 = property on="FFT 2 Choice 1" class="Ring (strict)"("Strings []"=w783) -> ()  [unwired: 2 in, 2 out]
        n445 = property on="FFT 2 Choice 2" class="Ring (strict)"("Strings []"=w783) -> ()  [unwired: 2 in, 2 out]
        n446 = Bundle("APD 1", "APD 2") -> (w786:cluster{string, string})  [unwired: 1 out]
        n447 = Cluster To Array(cluster=w786) -> (array=w784:string[])
        n448 = Build Array (concatenate)(w784, w783) -> (w788:string[])
        n449 = Array Size(array=w788) -> (size(s)=w789:i32)
        n450 = property on="Signals to Plot" class="LstBox (strict)"("Item Names"=w788) -> ()  [unwired: 2 in, 2 out]
        n451 = property on="Signals to Plot" class="LstBox (strict)"("Number of Rows"=w789) -> ()  [unwired: 2 in, 2 out]
        n452 = property on="All Signals" class="WFChart (strict)"("LegNumRows"=w789) -> ()  [unwired: 2 in, 2 out]
      }
      event "Adjust Scale\nto Mean": Value Change {
        n453 = event-data() -> ()  [unwired: 7 out]
        n454 = local read "APD 1 Rate (Hz)"() -> (w798:dbl)
        n455 = Multiply(x=1000.0, y="Above (kHz)") -> (x*y=w796:dbl)
        n456 = Multiply(x=1000.0, y="Below (kHz)") -> (x*y=w794:dbl)
        n457 = Add(x=w796, y=w798) -> (x+y=w791:dbl)
        n458 = Subtract(x=w798, y=w794) -> (x-y=w792:dbl)
        n459 = property on="APD Chart" class="WFChart (strict)"("YScale.Minimum"=w792) -> ()  [unwired: 2 in, 2 out]
        n460 = property on="APD Chart" class="WFChart (strict)"("YScale.Maximum"=w791) -> ()  [unwired: 2 in, 2 out]
      }
      event "Phase adj. (AI1)", "+ phase (AI1)", "- phase (AI1)": Value Change {
        n461 = event-data() -> ()  [unwired: 7 out]
        n462 = Negate(x="Phase adj. (AI1)") -> (-x=w808:i16)
        n463 = Select(t=w808, s="- phase (AI1)", f="Phase adj. (AI1)") -> (s? t:f=w807:i16)
        n464 = xnode "Read/Write Control"("FPGA VI Reference In"=w811, "error in"=w810, "Phase count adjustment"=w807) -> ("FPGA VI Reference Out"=w806:T19, "error out"=w805:errorcluster)
        n465 = Or(x="- phase (AI1)", y="+ phase (AI1)") -> (x .or. y?=w802:bool)
        n466 = xnode "Read/Write Control"("FPGA VI Reference In"=w806, "error in"=w805, "+ phase"=w802) -> ("error out"=w801:errorcluster)  [unwired: 1 out]
      }
      event "Signals to Plot": Double Click {
        w814 = u32 9868950 ("Color Box")
        n467 = event-data() -> ("Row"=w816:i32)  [unwired: 9 out]
        n468 = property on="All Signals" class="WFChart (strict)"("Active Plot"=w816) -> (error out=w827:errorcluster)  [unwired: 2 in, 1 out]
        n469 = property on="All Signals" class="WFChart (strict)" props=["Plot", "Visible?", "Plot", "Plot Color"](error in=w827) -> (error out=w826:errorcluster, "Plot.Visible?"=w825:bool)  [unwired: 1 in, 2 out]
        n470 = Select(t=FALSE ("Plot.Visible"), s=w825, f=TRUE ("Plot.Visible")) -> (s? t:f=w820:bool)
        n471 = property on="All Signals" class="WFChart (strict)"(error in=w826, "Plot.Visible?"=w820) -> (error out=w822:errorcluster)  [unwired: 1 in, 1 out]
        n472 = property on="All Signals" class="WFChart (strict)"(error in=w822) -> (error out=w817:errorcluster, "Plot.Plot Color"=w821:u32)  [unwired: 1 in, 1 out]
        n473 = property on="Signals to Plot" class="LstBox (strict)"(error in=w817, "Active Row"=w816) -> (error out=w815:errorcluster)  [unwired: 1 in, 1 out]
        n474 = Select(t=w821, s=w820, f=u32 0) -> (s? t:f=w818:u32)
        n475 = property on="Signals to Plot" class="LstBox (strict)"(error in=w815, "CellFontColor"=w818, "SelColor"=w814, "CellBG"=w814, "CellFontSize"=u32 20 ("Active Row:Cell Font:Size"), "CellFontBold"=TRUE ("Active Row:Cell Font:Bold")) -> ()  [unwired: 1 in, 2 out]
      }
      event "BD 1 Frequency 1 (MHz)", "BD 1 Frequency 2 (MHz)", "BD 1 Frequency 3 (MHz)", "BD 2 Frequency 1 (MHz)", "BD 2 Frequency 2 (MHz)", "BD 2 Frequency 3 (MHz)", "Trap Delta (MHz)": Value Change {
        # "anytime one of the frequencies is changed, write it to the RF board UNLESS Set 2 is being oscillated. The oscillation\nscript writes the frequencies to the RF board."
        n476 = event-data() -> ("CtlRef"=w830:refnum<vi>)  [unwired: 6 out]
        n477 = control-ref of="Trap Delta (MHz)"() -> (w829:refnum<vi>)
        n478 = Equal?(x=w829, y=w830) -> (x = y?=w828:bool)
        n479 = case shown="False" "Oscillate Set 2" {
          tunnel: w833 -> [w853 _]
          tunnel: [w852 w856] -> w832
          tunnel: w831 -> [w851 w856]
          tunnel: w828 -> [w838 _]
          frame False {
            n480 = local read "BD 1 Frequency 1 (MHz)"() -> (w835:dbl)
            n481 = local read "BD 1 Frequency 2 (MHz)"() -> (w840:dbl)
            n482 = Add(x=w835, y="Trap Delta (MHz)") -> (x+y=w839:dbl)
            n483 = Select(t=w839, s=w838, f=w840) -> (s? t:f=w837:dbl)
            n484 = local read "Y RF Frequency Limits (MHz)"() -> (w841:T16)
            n485 = local read "X RF Frequency Limits (MHz)"() -> (w842:T16)
            n486 = local read "BD 1 Frequency 3 (MHz)"() -> (w854:dbl)
            n487 = local write "BD 1 Frequency 2 (MHz)"(w837) -> ()
            n488 = local read "BD 2 Frequency 1 (MHz)"() -> (w845:dbl)
            n489 = local read "BD 2 Frequency 2 (MHz)"() -> (w844:dbl)
            n490 = local read "BD 2 Frequency 3 (MHz)"() -> (w855:dbl)
            n491 = call "set RF board frequency - interlace.vi"("Board 2 Frequency Limits"=w841, "Board 1 Frequency Limits"=w842, "error in"=w851, "FPGA VI Reference In"=w853, "Board 2 Frequency 3 (MHz)"=w855, "Board 1 Frequency 3 (MHz)"=w854, "Board 2 Frequency 2 (MHz)"=w844, "Board 2 Frequency 1 (MHz)"=w845, "Board 1 Frequency 2 (MHz)"=w837, "Board 1 Frequency 1  (MHz)"=w835) -> ("error out"=w852:errorcluster)  [unwired: 1 out]
            n492 = Subtract(x=w845, y=w844) -> (x-y=w849:dbl)
            n493 = Subtract(x=w837, y=w835) -> (x-y=w850:dbl)
            n494 = Square(x=w849) -> (x^2=w847:dbl)
            n495 = Square(x=w850) -> (x^2=w848:dbl)
            n496 = Add(x=w848, y=w847) -> (x+y=w846:dbl)
            n497 = Square Root(x=w846) -> (sqrt(x)=w843:dbl)
            n498 = local write "Trap Delta (MHz)"(w843) -> ()
            n499 = property on="Initial delta (MHz)" class="DigNum (strict)"("Val(Sgnl)"=w843) -> ()  [unwired: 2 in, 2 out]
          }
          frame True {
          }
        }
      }
      event "Round T1 X": Value Change {
        n500 = event-data() -> ()  [unwired: 7 out]
        n501 = local read "BD 1 Frequency 1 (MHz)"() -> (w859:dbl)
        n502 = Round To Nearest(number=w859) -> (nearest integer value=w858:dbl)
        n503 = property on="BD 1 Frequency 1 (MHz)" class="DigNum (strict)"("Val(Sgnl)"=w858) -> ()  [unwired: 2 in, 2 out]
      }
      event "Restart RF": Value Change {
        n504 = event-data() -> ()  [unwired: 7 out]
        n505 = xnode "Read/Write Control"("FPGA VI Reference In"=w897, "error in"=w892, "FPGA Controls  RF Box"=FALSE) -> ("FPGA VI Reference Out"=w896:T19, "error out"=w891:errorcluster)
        n506 = local read "Y RF Amplitude Limits (%)"() -> (w872:T16)
        n507 = local read "X RF Amplitude Limits (%)"() -> (w873:T16)
        n508 = local read "X RF Frequency Limits (MHz)"() -> (w875:T16)
        n509 = local read "Y RF Frequency Limits (MHz)"() -> (w874:T16)
        n510 = xnode "Read/Write Control"("FPGA VI Reference In"=w896, "error in"=w891, "Direct RF Box  Communication"=TRUE) -> ("FPGA VI Reference Out"=w895:T19, "error out"=w890:errorcluster)
        n511 = local read "BD 2 Frequency 3 (MHz)"() -> (w882:dbl)
        n512 = local read "BD 2 Frequency 2 (MHz)"() -> (w883:dbl)
        n513 = local read "BD 1 Frequency 3 (MHz)"() -> (w886:dbl)
        n514 = local read "BD 1 Frequency 1 (MHz)"() -> (w887:dbl)
        n515 = local read "BD 2 Frequency 1 (MHz)"() -> (w884:dbl)
        n516 = local read "BD 1 Frequency 2 (MHz)"() -> (w885:dbl)
        n517 = call "Initialize RF boards - interlace 3.vi"("error in"=w890, "FPGA VI Reference In"=w895) -> ("error out"=w889:errorcluster, "FPGA VI Reference Out"=w894:T19)
        n518 = local read "BD 2 Amplitude 2 (%)"() -> (w877:dbl)
        n519 = local read "BD 2 Amplitude 1 (%)"() -> (w878:dbl)
        n520 = local read "BD 2 Amplitude 3 (%)"() -> (w876:dbl)
        n521 = local read "BD 1 Amplitude 3 (%)"() -> (w881:dbl)
        n522 = local read "BD 1 Amplitude 1 (%)"() -> (w880:dbl)
        n523 = local read "BD 1 Amplitude 2 (%)"() -> (w879:dbl)
        n524 = call "set RF board frequency - interlace.vi"("Board 2 Frequency Limits"=w874, "Board 1 Frequency Limits"=w875, "error in"=w889, "FPGA VI Reference In"=w894, "Board 2 Frequency 3 (MHz)"=w882, "Board 1 Frequency 3 (MHz)"=w886, "Board 2 Frequency 2 (MHz)"=w883, "Board 2 Frequency 1 (MHz)"=w884, "Board 1 Frequency 2 (MHz)"=w885, "Board 1 Frequency 1  (MHz)"=w887) -> ("error out"=w888:errorcluster, "FPGA VI Reference Out"=w893:T19)
        n525 = call "set RF board amplitude - interlace.vi"("Board 2 Amplitude Limits"=w872, "Board 1 Amplitude Limits"=w873, "error in"=w888, "FPGA VI Reference In"=w893, "Board 2 Amplitude 3 (%)"=w876, "Board 1 Amplitude 3 (%)"=w881, "Board 2 Amplitude 2 (%)"=w877, "Board 2 Amplitude 1 (%)"=w878, "Board 1 Amplitude 2 (%)"=w879, "Board 1 Amplitude 1 (%)"=w880) -> ("error out"=w865:errorcluster, "FPGA VI Reference Out"=w869:T19)
        n526 = xnode "Read/Write Control"("FPGA VI Reference In"=w869, "error in"=w865, "Direct RF Box  Communication"=FALSE) -> ("FPGA VI Reference Out"=w868:T19, "error out"=w867:errorcluster)
        n527 = flat-sequence {
          tunnel: w867 -> [w898]
          tunnel: [w898] -> w866
          frame #0 {
            n528 = Wait (ms)(milliseconds to wait=u32 50) -> ()  [unwired: 1 out]
          }
        }
        n529 = xnode "Read/Write Control"("FPGA VI Reference In"=w868, "error in"=w866, "FPGA Controls  RF Box"=TRUE) -> ("error out"=w861:errorcluster)  [unwired: 1 out]
        n530 = property on="Restart RF" class="Bool (strict)"(error in=w861, "Value"=FALSE ("Restart RF")) -> (error out=w860:errorcluster)  [unwired: 1 in, 1 out]
      }
      event "Round T2 X": Value Change {
        n531 = event-data() -> ()  [unwired: 7 out]
        n532 = local read "BD 1 Frequency 2 (MHz)"() -> (w901:dbl)
        n533 = Round To Nearest(number=w901) -> (nearest integer value=w900:dbl)
        n534 = property on="BD 1 Frequency 2 (MHz)" class="DigNum (strict)"("Val(Sgnl)"=w900) -> ()  [unwired: 2 in, 2 out]
      }
      event "Stop All": Value Change {
        n535 = event-data() -> ()  [unwired: 7 out]
        n536 = call "hamilton_controller.vi"("action"=T20."DISCONNECT") -> ()  [unwired: 10 in, 1 out]
        n537 = local read "Stop All"() -> (w904:bool)
      }
      event "Delayed Interlace Start": Value Change {
        n538 = event-data() -> ()  [unwired: 7 out]
        n539 = flat-sequence {
          frame #0 {
            n540 = Multiply(x="Delay to Interlace (s)", y=1000.0) -> (x*y=w907:dbl)
            n541 = Wait (ms)(milliseconds to wait=w907) -> ()  [unwired: 1 out]
          }
          frame #1 {
            n542 = property on="Green laser mode" class="RadioBtnsControl (strict)"("Val(Sgnl)"=enum32{"Laser ON", "Laser OFF", "Interlace"}."Interlace" ("Value (Signaling)")) -> ()  [unwired: 2 in, 2 out]
          }
        }
      }
      event "BD 1 Amplitude 1 (%)", "BD 1 Amplitude 2 (%)", "BD 1 Amplitude 3 (%)", "BD 2 Amplitude 1 (%)", "BD 2 Amplitude 2 (%)", "BD 2 Amplitude 3 (%)", "Trap 1 ON", "Trap 2 ON", "Trap 3 ON", "Feedback On/Off", "All FB On/Off": Value Change {
        w931 = i16 1 ("f")
        n543 = event-data() -> ()  [unwired: 7 out]
        n544 = local write "Trap 1 (ON/OFF)"("Trap 1 ON") -> ()
        n545 = local write "Trap 2 (ON/OFF)"("Trap 2 ON") -> ()
        n546 = Boolean To (0,1)(Boolean="Trap 3 ON") -> (0, 1=w932:i16)
        n547 = Boolean To (0,1)(Boolean="Trap 1 ON") -> (0, 1=w933:i16)
        n548 = Boolean To (0,1)(Boolean="Trap 2 ON") -> (0, 1=w934:i16)
        n549 = Select(t=w934, s="Trap ON/OFF X or Y Amp?", f=w931) -> (s? t:f=w929:i16)
        n550 = Select(t=w933, s="Trap ON/OFF X or Y Amp?", f=w931) -> (s? t:f=w930:i16)
        n551 = Select(t=w932, s="Trap ON/OFF X or Y Amp?", f=w931) -> (s? t:f=w928:i16)
        n552 = Select(t=w931, s="Trap ON/OFF X or Y Amp?", f=w934) -> (s? t:f=w926:i16)
        n553 = Select(t=w931, s="Trap ON/OFF X or Y Amp?", f=w933) -> (s? t:f=w927:i16)
        n554 = Select(t=w931, s="Trap ON/OFF X or Y Amp?", f=w932) -> (s? t:f=w925:i16)
        n555 = And(x="All FB On/Off", y="Feedback On/Off") -> (x .and. y?=w923:cluster{"Set 1":bool, "Set 2":bool})
        n556 = local read "BD 1 Amplitude 1 (%)"() -> (w943:dbl)
        n557 = local read "BD 1 Amplitude 2 (%)"() -> (w942:dbl)
        n558 = local read "BD 1 Amplitude 3 (%)"() -> (w941:dbl)
        n559 = Unbundle By Name(w923) -> ("Set 1"=w918:bool, "Set 2"=w915:bool)
        n560 = local read "Y RF Amplitude Limits (%)"() -> (w911:T16)
        n561 = local read "X RF Amplitude Limits (%)"() -> (w912:T16)
        n562 = local read "BD 2 Amplitude 1 (%)"() -> (w944:dbl)
        n563 = local read "BD 2 Amplitude 2 (%)"() -> (w945:dbl)
        n564 = local read "BD 2 Amplitude 3 (%)"() -> (w946:dbl)
        n565 = And(x="Trap 2 ON", y=w915) -> (x .and. y?=w913:bool)
        n566 = And(x="Trap 1 ON", y=w918) -> (x .and. y?=w916:bool)
        n567 = Multiply(x=w930, y=w943) -> (x*y=w938:dbl)
        n568 = Multiply(x=w942, y=w929) -> (x*y=w936:dbl)
        n569 = Multiply(x=w941, y=w928) -> (x*y=w937:dbl)
        n570 = Multiply(x=w944, y=w927) -> (x*y=w947:dbl)
        n571 = Multiply(x=w945, y=w926) -> (x*y=w948:dbl)
        n572 = Multiply(x=w946, y=w925) -> (x*y=w949:dbl)
        n573 = call "set RF board amplitude - interlace.vi"("Board 2 Amplitude Limits"=w911, "Board 1 Amplitude Limits"=w912, "error in"=w939, "FPGA VI Reference In"=w940, "Board 2 Amplitude 3 (%)"=w949, "Board 1 Amplitude 3 (%)"=w937, "Board 2 Amplitude 2 (%)"=w948, "Board 2 Amplitude 1 (%)"=w947, "Board 1 Amplitude 2 (%)"=w936, "Board 1 Amplitude 1 (%)"=w938) -> ("error out"=w920:errorcluster, "FPGA VI Reference Out"=w921:T19)
        n574 = xnode "Read/Write Control"("FPGA VI Reference In"=w921, "error in"=w920, "FB On/Off Set 1"=w916, "FB On/Off Set 2"=w913) -> ("error out"=w919:errorcluster)  [unwired: 1 out]
      }
      event "Load parameters": Value Change {
        n575 = event-data() -> ()  [unwired: 7 out]
        n576 = property on="Saved AOD Raster Scan Parameter Sets" class="Arr (strict)"() -> ("Index Values"=w960:u32[])  [unwired: 2 in, 2 out]
        n577 = Index Array(array=w960, index=0) -> (element=w957:u32)
        n578 = local write "Load parameters"(FALSE ("Load parameters")) -> ()
        n579 = Index Array(array="Saved AOD Raster Scan Parameter Sets", index=w957) -> (element=w956:T30)
        n580 = Unbundle By Name(w956) -> ("Scan Range AOD (nm) 2"=w955:dbl, "Step Size AOD (nm) 2"=w954:dbl, "Scan Speed AOD (nm/s) 2"=w953:dbl, "Number of scans (AOD) 2"=w952:u16)
        n581 = flat-sequence {
          tunnel: w955 -> [w963]
          tunnel: w954 -> [w962]
          tunnel: w953 -> [w961]
          tunnel: w952 -> [w964]
          frame #0 {
            n582 = local write "Scan Speed (nm/s)"(w961) -> ()
            n583 = local write "Scan Range (nm)"(w963) -> ()
            n584 = local write "Step Size (nm)"(w962) -> ()
          }
          frame #1 {
            n585 = property on="Number of F/B Scans (AOD)" class="DigNum (strict)"("Val(Sgnl)"=w964) -> ()  [unwired: 2 in, 2 out]
          }
        }
      }
      event "Trap 1 (ON/OFF)", "Trap 2 (ON/OFF)": Value Change {
        n586 = event-data() -> ()  [unwired: 7 out]
        n587 = property on="Trap 2 ON" class="Bool (strict)"("Val(Sgnl)"="Trap 2 (ON/OFF)") -> ()  [unwired: 2 in, 2 out]
        n588 = property on="Trap 1 ON" class="Bool (strict)"("Val(Sgnl)"="Trap 1 (ON/OFF)") -> ()  [unwired: 2 in, 2 out]
      }
      event "DIO count 1 (ticks)", "DIO count 2 (ticks)", "DIO count 3 (ticks)", "Interlace", "Number Interlace Sets", "Not-Interlacing Set": Value Change {
        n589 = event-data() -> ()  [unwired: 7 out]
        n590 = local read "DIO count 3 (ticks)"() -> (w977:u32)
        n591 = local read "DIO count 1 (ticks)"() -> (w979:u32)
        n592 = local read "DIO count 2 (ticks)"() -> (w978:u32)
        n593 = To Unsigned Byte Integer(number="Not-Interlacing Set") -> (unsigned 8bit integer=w968:u8)
        n594 = Add(x=w968, y=u8 1) -> (x+y=w972:u8)
        n595 = xnode "Read/Write Control"("FPGA VI Reference In"=w983, "error in"=w981, "DIO count 1 (ticks)"=w979, "DIO count 2 (ticks)"=w978, "DIO count 3 (ticks)"=w977, "Interlace ON/OFF"="Interlace", "Number Interlace Cycles"="Number Interlace Sets", "Interlace Off Parameters"=w972) -> ("error out"=w982:errorcluster)  [unwired: 1 out]
        n596 = Build Array(w979, w978, w977) -> (w970:u32[])
        n597 = Split 1D Array(array=w970, index="Number Interlace Sets") -> (first subarray=w980:u32[])  [unwired: 1 out]
        n598 = Index Array(array=w970, index=w968) -> (element=w969:u32)
        n599 = Add Array Elements(numeric array=w980) -> (sum=w974:u32)
        n600 = Select(t=w974, s="Interlace", f=w969) -> (s? t:f=→"Total Counts (ticks)":u32)
      }
      event "Reset Feedback": Value Change {
        n601 = event-data() -> ()  [unwired: 7 out]
        n602 = Unbundle By Name("Reset Feedback") -> ("Set 1"=w987:bool, "Set 2"=w986:bool)
        n603 = xnode "Read/Write Control"("FPGA VI Reference In"=w989, "error in"=w984, "FB Reset Set 1"=w987, "FB Reset Set 2"=w986) -> ("error out"=w985:errorcluster)  [unwired: 1 out]
      }
      event "PID Gains": Value Change {
        n604 = event-data() -> ()  [unwired: 7 out]
        n605 = Unbundle By Name("PID Gains") -> ("Set 1"=w993:T14, "Set 2"=w992:T14)
        n606 = xnode "Read/Write Control"("FPGA VI Reference In"=w994, "error in"=w990, "FB Gains Set 1"=w993, "FB Gains Set 2"=w992) -> ("error out"=w991:errorcluster)  [unwired: 1 out]
      }
      event "AI2 to Setpoint", "Trap Intensity\nSetpoints (V)": Value Change {
        n607 = event-data() -> ()  [unwired: 7 out]
        n608 = xnode "Read/Write Control"("FPGA VI Reference In"=w1000, "error in"=w996) -> ("FPGA VI Reference Out"=w999:T19, "error out"=w998:errorcluster, "AI2 Y Sum Set 1"=w1007:i16, "AI2 Y Sum Set 2"=w1006:i16)
        n609 = Cluster To Array(cluster="AI2 to Setpoint") -> (array=w1010:bool[])
        n610 = local read "AI2 (V)"() -> (w1008:cluster{"Set 1":dbl, "Set 2":dbl})
        n611 = Or Array Elements(Boolean array=w1010) -> (logical OR=w1011:bool)
        n612 = Bundle By Name(cluster=w1008, "Set 1"=w1007, "Set 2"=w1006) -> (w1005:cluster{"Set 1":dbl, "Set 2":dbl})
        n613 = Divide(x=w1005, y=3276.7) -> (x/y=w1004:cluster{"Set 1":dbl, "Set 2":dbl})
        "AI2 (V)" <- w1004
        n614 = case shown="True" w1011 {
          tunnel: [w1014 w1031] -> w1003
          tunnel: "AI2 to Setpoint" -> [_ w1027]
          tunnel: "Trap Intensity\nSetpoints (V)" -> [w1015 w1030]
          tunnel: w1004 -> [_ w1024]
          frame False {
            n615 = Multiply(x=3276.7, y=w1015) -> (x*y=w1016:cluster{"Set 1":dbl, "Set 2":dbl})
            n616 = To Word Integer(number=w1016) -> (16bit integer=w1014:cluster{"Set 1":i16, "Set 2":i16})
          }
          frame True {
            n617 = Unbundle By Name(w1024) -> ("Set 1"=w1023:dbl, "Set 2"=w1022:dbl)
            n618 = Unbundle By Name(w1030) -> ("Set 1"=w1029:dbl, "Set 2"=w1028:dbl)
            n619 = Unbundle By Name(w1027) -> ("Set 1"=w1026:bool, "Set 2"=w1025:bool)
            n620 = Select(t=w1023, s=w1026, f=w1029) -> (s? t:f=w1021:dbl)
            n621 = Select(t=w1022, s=w1025, f=w1028) -> (s? t:f=w1020:dbl)
            n622 = Bundle By Name(cluster=w1030, "Set 1"=w1021, "Set 2"=w1020) -> (w1018:cluster{"Set 1":dbl, "Set 2":dbl})
            n623 = local write "Trap Intensity\nSetpoints (V)"(w1018) -> ()
            n624 = Multiply(x=3276.7, y=w1018) -> (x*y=w1019:cluster{"Set 1":dbl, "Set 2":dbl})
            n625 = To Word Integer(number=w1019) -> (16bit integer=w1031:cluster{"Set 1":i16, "Set 2":i16})
          }
        }
        n626 = Unbundle By Name(w1003) -> ("Set 1"=w1002:i16, "Set 2"=w1001:i16)
        n627 = xnode "Read/Write Control"("FPGA VI Reference In"=w999, "error in"=w998, "FB Setpoint Set 1"=w1002, "FB Setpoint Set 2"=w1001) -> ("error out"=w997:errorcluster)  [unwired: 1 out]
      }
      event "Invert GI": Value Change {
        n628 = event-data() -> ()  [unwired: 7 out]
        n629 = xnode "Read/Write Control"("FPGA VI Reference In"=w1036, "error in"=w1034, "Invert GI"="Invert GI", "Invert GI 2"="Invert GI") -> ("error out"=w1035:errorcluster)  [unwired: 1 out]
      }
      event "Green FB Setpoint (mV)", "Green FB Gains", "Green FB On/Off", "Current When FB OFF (%)", "Green int current ON count adj": Value Change {
        n630 = event-data() -> ()  [unwired: 7 out]
        n631 = local read "Green FB Setpoint (mV)"() -> (w1043:dbl)
        n632 = local read "Current When FB OFF (%)"() -> (w1046:dbl)
        n633 = Multiply(x=w1043, y=3.2767) -> (x*y=w1042:dbl)
        n634 = Multiply(x=w1046, y=655.35) -> (x*y=w1047:dbl)
        n635 = To Unsigned Word Integer(number=w1047) -> (unsigned 16bit integer=w1045:u16)
        n636 = local read "Green int current ON count adj"() -> (w1050:u32)
        n637 = local read "Green FB Gains"() -> (w1049:T14)
        n638 = local read "Green Laser ON/Interlacing"() -> (w1040:bool)
        n639 = local read "Green laser mode"() -> (w1039:enum32{"Laser ON", "Laser OFF", "Interlace"})
        n640 = local read "Green FB On/Off"() -> (w1051:bool)
        n641 = Equal?(x=w1039, y=enum32{"Laser ON", "Laser OFF", "Interlace"}."Interlace") -> (x = y?=w1037:bool)
        n642 = Compound Arithmetic op=AND(w1037, w1051, w1040) -> (w1041:bool)
        n643 = xnode "Read/Write Control"("FPGA VI Reference In"=w1054, "error in"=w1053, "Green FB Setpoint"=w1042, "Green FB On/Off"=w1041, "Current Out"=w1045, "Green int current ON count adj"=w1050, "Green FB Gains"=w1049) -> ("error out"=w1052:errorcluster)  [unwired: 1 out]
      }
      event "Green laser mode", "Green Laser ON/Interlacing": Value Change {
        n644 = event-data() -> ()  [unwired: 7 out]
        n645 = case shown="True" "Green Laser ON/Interlacing" {
          tunnel: "Green laser mode" -> [_ w1068]
          tunnel: [enum32{"Laser ON", "Laser OFF", "Interlace"}."Laser OFF" ("Green laser mode") w1068] -> w1056
          tunnel: [FALSE w1064] -> w1055
          frame False {
          }
          frame True {
            n646 = local read "Green FB On/Off"() -> (w1065:bool)
            n647 = Equal?(x=w1068, y=enum32{"Laser ON", "Laser OFF", "Interlace"}."Interlace") -> (x = y?=w1066:bool)
            n648 = And(x=w1066, y=w1065) -> (x .and. y?=w1064:bool)
          }
        }
        n649 = xnode "Read/Write Control"("FPGA VI Reference In"=w1061, "error in"=w1059, "Operating Mode"=w1056, "Operating Mode 2"=w1056, "Green FB On/Off"=w1055) -> ("error out"=w1060:errorcluster)  [unwired: 1 out]
      }
      event "- phase (APD 1 Gate)", "+ phase (APD 1 Gate)": Value Change {
        n650 = event-data() -> ()  [unwired: 7 out]
        n651 = local read "Phase Adj. (APD 1 Gate)"() -> (w1069:i16)
        n652 = Negate(x=w1069) -> (-x=w1077:i16)
        n653 = Select(t=w1077, s="- phase (APD 1 Gate)", f=w1069) -> (s? t:f=w1076:i16)
        n654 = Or(x="- phase (APD 1 Gate)", y="+ phase (APD 1 Gate)") -> (x .or. y?=w1072:bool)
        n655 = xnode "Read/Write Control"("FPGA VI Reference In"=w1079, "error in"=w1078, "Phase count adjustment (APD 1 Gate)"=w1076) -> ("FPGA VI Reference Out"=w1074:T19, "error out"=w1075:errorcluster)
        n656 = xnode "Read/Write Control"("FPGA VI Reference In"=w1074, "error in"=w1075, "+ phase (APD 1 Gate)"=w1072) -> ("error out"=w1073:errorcluster)  [unwired: 1 out]
      }
      event "+ phase (APD 2 Gate)", "- phase (APD 2 Gate)": Value Change {
        n657 = event-data() -> ()  [unwired: 7 out]
        n658 = local read "Phase Adj. (APD 2 Gate)"() -> (w1080:i16)
        n659 = Negate(x=w1080) -> (-x=w1088:i16)
        n660 = Select(t=w1088, s="- phase (APD 2 Gate)", f=w1080) -> (s? t:f=w1087:i16)
        n661 = Or(x="- phase (APD 2 Gate)", y="+ phase (APD 2 Gate)") -> (x .or. y?=w1083:bool)
        n662 = xnode "Read/Write Control"("FPGA VI Reference In"=w1090, "error in"=w1089, "Phase count adjustment (APD 2 Gate)"=w1087) -> ("FPGA VI Reference Out"=w1085:T19, "error out"=w1086:errorcluster)
        n663 = xnode "Read/Write Control"("FPGA VI Reference In"=w1085, "error in"=w1086, "+ phase (APD 2 Gate)"=w1083) -> ("error out"=w1084:errorcluster)  [unwired: 1 out]
      }
      event "Phase Adj. (APD Acq)", "+ phase (APD Acq)", "- phase (APD Acq)": Value Change {
        n664 = event-data() -> ()  [unwired: 7 out]
        n665 = local read "Phase Adj. (APD Acq)"() -> (w1093:i16)
        n666 = Negate(x=w1093) -> (-x=w1099:i16)
        n667 = Select(t=w1099, s="+ phase (APD Acq)", f=w1093) -> (s? t:f=w1098:i16)
        n668 = Or(x="+ phase (APD Acq)", y="- phase (APD Acq)") -> (x .or. y?=w1094:bool)
        n669 = xnode "Read/Write Control"("FPGA VI Reference In"=w1101, "error in"=w1100, "Phase Count Adjustment (APD Acq)"=w1098) -> ("FPGA VI Reference Out"=w1096:T19, "error out"=w1097:errorcluster)
        n670 = xnode "Read/Write Control"("FPGA VI Reference In"=w1096, "error in"=w1097, "+ phase (APD Acq)"=w1094) -> ("error out"=w1095:errorcluster)  [unwired: 1 out]
      }
      event "Phase adj. (GI)", "+ phase (GI)", "- phase (GI)": Value Change {
        n671 = event-data() -> ()  [unwired: 7 out]
        n672 = Negate(x="Phase adj. (GI)") -> (-x=w1110:i16)
        n673 = Select(t=w1110, s="+ phase (GI)", f="Phase adj. (GI)") -> (s? t:f=w1109:i16)
        n674 = Or(x="+ phase (GI)", y="- phase (GI)") -> (x .or. y?=w1105:bool)
        n675 = xnode "Read/Write Control"("FPGA VI Reference In"=w1112, "error in"=w1111, "Phase count adjustment (GI)"=w1109) -> ("FPGA VI Reference Out"=w1107:T19, "error out"=w1108:errorcluster)
        n676 = xnode "Read/Write Control"("FPGA VI Reference In"=w1107, "error in"=w1108, "+ phase (GI)"=w1105) -> ("error out"=w1106:errorcluster)  [unwired: 1 out]
      }
      event "Phase adj. (GI) 2", "+ phase (GI) 2", "- phase (GI) 2": Value Change {
        n677 = event-data() -> ()  [unwired: 7 out]
        n678 = Negate(x="Phase adj. (GI) 2") -> (-x=w1121:i16)
        n679 = Select(t=w1121, s="+ phase (GI) 2", f="Phase adj. (GI) 2") -> (s? t:f=w1120:i16)
        n680 = Or(x="+ phase (GI) 2", y="- phase (GI) 2") -> (x .or. y?=w1116:bool)
        n681 = xnode "Read/Write Control"("FPGA VI Reference In"=w1123, "error in"=w1122, "Phase count adjustment (GI) 2"=w1120) -> ("FPGA VI Reference Out"=w1118:T19, "error out"=w1119:errorcluster)
        n682 = xnode "Read/Write Control"("FPGA VI Reference In"=w1118, "error in"=w1119, "+ phase (GI) 2"=w1116) -> ("error out"=w1117:errorcluster)  [unwired: 1 out]
      }
      event "Phase adj. (Green FB)", "- phase (Green FB)", "+ phase (Green FB)": Value Change {
        n683 = event-data() -> ()  [unwired: 7 out]
        n684 = Negate(x="Phase adj. (Green FB)") -> (-x=w1132:i16)
        n685 = Select(t=w1132, s="+ phase (Green FB)", f="Phase adj. (Green FB)") -> (s? t:f=w1131:i16)
        n686 = Or(x="+ phase (Green FB)", y="- phase (Green FB)") -> (x .or. y?=w1127:bool)
        n687 = xnode "Read/Write Control"("FPGA VI Reference In"=w1134, "error in"=w1133, "Phase count adjustment (Green FB)"=w1131) -> ("FPGA VI Reference Out"=w1129:T19, "error out"=w1130:errorcluster)
        n688 = xnode "Read/Write Control"("FPGA VI Reference In"=w1129, "error in"=w1130, "+ phase (Green FB)"=w1127) -> ("error out"=w1128:errorcluster)  [unwired: 1 out]
      }
      event "Invert APD Gate", "APD Gate ON Count", "APD Gate OFF Count", "APD Gate", "APD Integration Time (s)", "APD 1 AO Mult.", "APD 2 AO Mult.": Value Change {
        n689 = event-data() -> ()  [unwired: 7 out]
        n690 = local read "APD Integration Time (s)"() -> (w1135:dbl)
        n691 = local read "APD Gate ON Count"() -> (w1148:u32)
        n692 = local read "APD Gate OFF Count"() -> (w1147:u32)
        n693 = local read "Invert APD Gate"() -> (w1149:bool)
        n694 = local read "APD Gate"() -> (w1146:enum32{"ON", "OFF", "Interlace"})
        n695 = Multiply(x=w1135, y=40000000.0) -> (x*y=w1144:dbl)
        n696 = Reciprocal(x=w1135) -> (1/x=→"APD Acq Rate (Hz)":dbl)
        n697 = To Unsigned Long Integer(number=w1144) -> (unsigned 32bit integer=w1143:u32)
        n698 = local read "DMA Update Period (s)"() -> (w1136:dbl)
        n699 = Divide(x=w1136, y=w1135) -> (x/y=w1139:dbl)
        n700 = local read "APD 1 AO Mult."() -> (w1141:i16)
        n701 = local read "APD 2 AO Mult."() -> (w1140:i16)
        n702 = Multiply(x=2.0, y=w1139) -> (x*y=w1138:dbl)
        n703 = local write "APD Samples/FIFO Acq."(w1139) -> ()
        n704 = local write "APD Elements/DMA read"(w1138) -> ()
        n705 = xnode "Read/Write Control"("FPGA VI Reference In"=w1152, "error in"=w1151, "Invert APD Gate"=w1149, "APD Gate ON Count"=w1148, "APD Gate OFF Count"=w1147, "APD Acq Rate Count"=w1143, "APD Gate Operating Mode"=w1146, "APD 1 AO scale factor"=w1141, "APD 2 AO scale factor"=w1140) -> ("error out"=w1150:errorcluster)  [unwired: 1 out]
      }
      event "GI Frequency, ON count", "Green FB Count", "GI Frequency, OFF count": Value Change {
        n706 = event-data() -> ()  [unwired: 7 out]
        n707 = xnode "Read/Write Control"("FPGA VI Reference In"=w1158, "error in"=w1156, "Green interlace ON count"="GI Frequency, ON count", "Green interlace OFF count"="GI Frequency, OFF count", "Green interlace ON count 2"="GI Frequency, ON count", "Green interlace OFF count 2"="GI Frequency, OFF count", "Green FB Count"="Green FB Count") -> ("error out"=w1157:errorcluster)  [unwired: 1 out]
      }
      event "Number of F/B Scans (AOD)", "Scan Speed (nm/s)", "Scan BD", "Initial delta (MHz)", "Step Size (nm)", "Scan Range (nm)": Value Change {
        w1220 = 123.0  # AOM cal (nm/MHz)
        n708 = event-data() -> ()  [unwired: 7 out]
        n709 = local read "BD 1 Frequency 1 (MHz)"() -> (w1203:dbl)
        n710 = local read "AOM X Cal (nm/MHz)"() -> (w1195:dbl)
        n711 = local read "X RF Frequency Limits (MHz)"() -> (w1207:T16)
        n712 = local read "Y RF Frequency Limits (MHz)"() -> (w1204:T16)
        n713 = local read "BD 2 Frequency 1 (MHz)"() -> (w1209:dbl)
        n714 = Negate(x="Scan Range (nm)") -> (-x=w1173:dbl)
        n715 = Divide(x=w1173, y=w1195) -> (x/y=w1177:dbl)
        n716 = Select(t=w1207, s="Scan BD", f=w1204) -> (s? t:f=w1206:T16)
        n717 = Select(t=w1203, s="Scan BD", f=w1209) -> (s? t:f=w1208:dbl)
        n718 = Unbundle By Name(w1206) -> ("Maximum"=w1215:dbl, "Minimum"=w1214:dbl)
        n719 = Add(x=w1177, y=w1208) -> (x+y=w1212:dbl)
        n720 = Divide(x=w1173, y="Step Size (nm)") -> (x/y=w1192:dbl)
        n721 = Divide(x="Step Size (nm)", y=w1195) -> (x/y=w1201:dbl)
        n722 = Absolute Value(x=w1192) -> (abs(x)=w1176:dbl)
        n723 = Sign(1:w1173) -> (0:w1174:dbl)
        n724 = In Range and Coerce(upper limit=w1215, x=w1212, lower limit=w1214) -> (coerced(x)=w1211:dbl, In Range?=w1213:bool)
        n725 = To Unsigned Quad Integer(1:w1176) -> (0:w1191:u64)
        "Scan steps (AOD)" <- w1191
        n726 = call "IR AOM freq to word.vi"("Frequency In (MHz)"=w1201) -> ("Frequency Word Out (double)"=w1198:dbl)
        n727 = Multiply(x=w1174, y=w1198) -> (x*y=w1175:dbl)
        n728 = Subtract(x=w1212, y=w1211) -> (x-y=w1210:dbl)
        n729 = To Quad Integer(1:w1175) -> (0:w1197:i64)
        "Incr. int (AOD)" <- w1197
        n730 = Subtract(x=w1177, y=w1210) -> (x-y=w1196:dbl)
        "Scan Range (MHz)" <- w1196
        n731 = Select(t=w1177, s=w1213, f=w1196) -> (s? t:f=w1216:dbl)
        n732 = Multiply(x=w1196, y=w1195) -> (x*y=w1194:dbl)
        n733 = Decrement(x=w1191) -> (x-1=w1244:u64)
        n734 = Negate(x=w1194) -> (-x=w1190:dbl)
        n735 = local write "Scan Range (nm)"(w1190) -> ()
        n736 = Divide(x=w1216, y=w1244) -> (x/y=w1200:dbl)
        "Scan Increment (MHz)" <- w1200
        n737 = call "IR AOM freq to word.vi"("Frequency In (MHz)"=w1200) -> ("Frequency Word Out (double)"=w1199:dbl)
        n738 = Divide(x="Step Size (nm)", y="Scan Speed (nm/s)") -> (x/y=w1187:dbl)
        n739 = To Quad Integer(1:w1199) -> ()  [unwired: 1 out]
        n740 = local read "Number Interlace Sets"() -> (w1171:u8)
        n741 = local read "AI Count (ticks)"() -> (w1172:u32)
        n742 = local read "Total Counts (ticks)"() -> (w1170:u32)
        n743 = local read "# Samples/trap"() -> (w1202:u32)
        n744 = Multiply(x=w1172, y=w1171) -> (x*y=w1169:u32)
        n745 = Divide(x=w1170, y=w1169) -> (x/y=w1168:dbl)
        n746 = Select(t=w1203, s="Scan BD", f=w1209) -> (s? t:f=w1241:dbl)
        "Initial freq. (MHz)" <- w1241
        n747 = Add(x=w1216, y=w1241) -> (x+y=→"Final freq. (MHz)":dbl)
        n748 = Divide(x=w1170, y=40000000.0) -> (x/y=w1186:dbl)
        n749 = Divide(x=w1187, y=w1186) -> (x/y=w1185:dbl)
        n750 = To Unsigned Quad Integer(1:w1185) -> (0:w1160:u64)
        n751 = Quotient & Remainder(x=w1160, y=u64 2) -> (x-y*floor(x/y)=w1164:u64)  [unwired: 1 out]
        n752 = Equal?(x=w1164, y=u64 0) -> (x = y?=w1162:bool)
        n753 = Decrement(x=w1160) -> (x-1=w1161:u64)
        n754 = Select(t=w1160, s=w1162, f=w1161) -> (s? t:f=w1159:u64)
        "Cycles/step (AOD)" <- w1159
        n755 = xnode "Read/Write Control"("FPGA VI Reference In"=w1252, "error in"=w1251, "Scan steps"=w1191, "Number of scans"="Number of F/B Scans (AOD)", "Cycles per step"=w1159, "Scan freq.  increment"=w1197, "Scan BD"="Scan BD") -> ("error out"=w1250:errorcluster)  [unwired: 1 out]
        n756 = Multiply(x=w1191, y=w1159) -> (x*y=w1245:u64)
        n757 = Multiply(x=w1245, y=u64 2) -> (x*y=w1167:u64)
        n758 = Multiply(x=w1168, y=w1167) -> (x*y=w1166:dbl)
        "Data points/scan (f/b)" <- w1166
        n759 = Multiply(x=w1166, y="Number of F/B Scans (AOD)") -> (x*y=w1248:dbl)
        "Data points/scans" <- w1248
        n760 = Divide(x=w1248, y=w1202) -> (x/y=→"N sets should be saved":dbl)
        n761 = Multiply(x=w1245, y=w1186) -> (x*y=w1184:dbl)
        "Time/Scan (s) (AOD)" <- w1184
        n762 = Select(t=w1216, s="Scan BD", f=0.0) -> (s? t:f=w1242:dbl)
        n763 = Select(t=0.0, s="Scan BD", f=w1216) -> (s? t:f=w1238:dbl)
        n764 = local read "BD 2 Frequency 2 (MHz)"() -> (w1234:dbl)
        n765 = local read "BD 1 Frequency 2 (MHz)"() -> (w1237:dbl)
        n766 = Add(x=w1238, y=w1209) -> (x+y=w1235:dbl)
        n767 = Add(x=w1203, y=w1242) -> (x+y=w1236:dbl)
        n768 = Multiply(x=w1184, y=2.0) -> (x*y=w1183:dbl)
        n769 = Multiply(x=w1183, y="Number of F/B Scans (AOD)") -> (x*y=w1180:dbl)
        n770 = Divide(x=w1180, y=60.0) -> (x/y=→"Time to Finish All (min)":dbl)
        n771 = Add(x="Trap 2 Bead Size (nm)", y="Trap 1 Bead Size (nm)") -> (x+y=w1224:dbl)
        n772 = local read "Initial delta (MHz)"() -> (w1221:dbl)
        n773 = Divide(x=w1224, y=2.0) -> (x/y=w1218:dbl)
        n774 = Subtract(x=w1235, y=w1234) -> (x-y=w1232:dbl)
        n775 = Subtract(x=w1236, y=w1237) -> (x-y=w1233:dbl)
        n776 = Square(x=w1232) -> (x^2=w1231:dbl)
        n777 = Square(x=w1233) -> (x^2=w1230:dbl)
        n778 = Add(x=w1230, y=w1231) -> (x+y=w1229:dbl)
        n779 = Square Root(x=w1229) -> (sqrt(x)=w1228:dbl)
        "Final delta (MHz)" <- w1228
        n780 = Multiply(x=w1220, y=w1228) -> (x*y=w1227:dbl)
        n781 = Multiply(x=w1221, y=w1220) -> (x*y=w1219:dbl)
        n782 = Subtract(x=w1219, y=w1218) -> (x-y=→"Initial sep (nm)":dbl)
        n783 = Subtract(x=w1227, y=w1218) -> (x-y=→"Final sep (nm)":dbl)
      }
      event "Raster Scanning...": Value Change {
        n784 = event-data() -> ("NewVal"=w1253:bool)  [unwired: 6 out]
        n785 = case shown="True" w1253 {
          frame False {
          }
          frame True {
            n786 = property on="BD 1 Frequency 1 (MHz)" class="DigNum (strict)"("Val(Sgnl)"=65.0 ("Value (Signaling)")) -> ()  [unwired: 2 in, 2 out]
          }
        }
      }
      event "Freq or Amp switch first", "Swap F1 and F2", "Freq switch delay", "Amp switch delay": Value Change {
        n787 = event-data() -> ()  [unwired: 7 out]
        n788 = local read "Freq or Amp switch first"() -> (w1255:bool)
        n789 = local read "Amp switch delay"() -> (w1256:u16)
        n790 = local read "Freq switch delay"() -> (w1258:u16)
        n791 = local read "Swap F1 and F2"() -> (w1257:bool)
        n792 = xnode "Read/Write Control"("FPGA VI Reference In"=w1261, "error in"=w1260, "Freq switch delay"=w1258, "Swap F1 and F2"=w1257, "Amp switch delay"=w1256, "Freq or Amp switch first"=w1255) -> ("error out"=w1259:errorcluster)  [unwired: 1 out]
      }
      event "Scan steps (MCL)", "Number of scans (MCL)", "Scan Range (V)\n(of steps)", "2D or 1D Scan", "N APD Samp/step", "Fast Scan Dir", "Continuous MCL Scanning", "Scan lines (y)": Value Change {
        w1263 = 32767.0 ("y")
        n793 = event-data() -> ()  [unwired: 7 out]
        n794 = Select(t="Scan lines (y)", s="2D or 1D Scan", f="Number of scans (MCL)") -> (s? t:f=w1268:u64)
        n795 = Decrement(x="Scan steps (MCL)") -> (x-1=w1284:u64)
        n796 = Divide(x="Scan Range (V)\n(of steps)", y=w1284) -> (x/y=w1283:dbl)
        "Desired Scan Incr (V)" <- w1283
        n797 = local read "APD Integration Time (s)"() -> (w1276:dbl)
        n798 = Multiply(x=w1283, y=w1263) -> (x*y=w1292:dbl)
        n799 = Divide(x=w1292, y=10.0) -> (x/y=w1282:dbl)
        "Desired incr (int)" <- w1282
        n800 = local read "Update Count (MCL)"() -> (w1288:u32)
        n801 = Round Toward -Infinity(1:w1282) -> (0:w1291:dbl)
        n802 = To Word Integer(number=w1291) -> (16bit integer=w1266:i16)
        "Actual Incr. int (MCL)" <- w1266
        n803 = Multiply(x=w1276, y=40000000.0) -> (x*y=w1289:dbl)
        n804 = Divide(x=w1289, y=w1288) -> (x/y=w1287:dbl)
        n805 = Multiply(x=i16 10, y=w1266) -> (x*y=w1264:i16)
        n806 = Multiply(x="N APD Samp/step", y=w1287) -> (x*y=w1286:dbl)
        "Cycles/step (MCL)" <- w1286
        n807 = Divide(x=w1264, y=w1263) -> (x/y=→"Actual MCL Inc (V)":dbl)
        n808 = Multiply(x="N APD Samp/step", y="Scan steps (MCL)") -> (x*y=w1278:dbl)
        n809 = local read "APD Samples/FIFO Acq."() -> (w1275:dbl)
        n810 = Multiply(x=w1278, y=u64 2) -> (x*y=w1277:dbl)
        "Data points/scan (f+b)" <- w1277
        n811 = Multiply(x=w1277, y=w1268) -> (x*y=w1295:dbl)
        "Data points/scans (MCL)" <- w1295
        n812 = Multiply(x=w1276, y=w1277) -> (x*y=w1269:dbl)
        "Time/f+b scan (s) (MCL)" <- w1269
        n813 = Divide(x=w1295, y=w1275) -> (x/y=→"N sets should be saved (MCL)":dbl)
        n814 = Multiply(x=w1269, y=w1268) -> (x*y=→"Total Time (s)":dbl)
        n815 = Not(x="Fast Scan Dir") -> (.not. x?=w1273:bool)
        n816 = xnode "Read/Write Control"("FPGA VI Reference In"=w1299, "error in"=w1298, "Scan steps (MCL)"="Scan steps (MCL)", "Number of scans (MCL)"=w1268, "Cycles per step (MCL)"=w1286, "Scan freq.  increment (MCL)"=w1266, "1D or 2D Scan?"="2D or 1D Scan", "MCL Scan Axis"=w1273, "Cont. Scan (MCL)"="Continuous MCL Scanning") -> ("error out"=w1297:errorcluster)  [unwired: 1 out]
      }
      event "Read Cal": Value Change {
        w1301 = 1000.0 ("y")
        n817 = event-data() -> ()  [unwired: 7 out]
        n818 = local read "Save file name"() -> (w1326:path)
        n819 = local write "Read Cal"(FALSE ("Read Cal")) -> ()
        n820 = Strip Path(path=w1326) -> (stripped path=w1325:path)  [unwired: 1 out]
        n821 = Path To String(path=w1325) -> (string=w1324:string)
        n822 = Concatenate Strings(w1324, "\\current.cal" ("string")) -> (w1322:string)
        n823 = String To Path(string=w1322) -> (path=w1321:path)
        n824 = Open/Create/Replace File(file path (use dialog)=w1321, operation (0:open)=T23."open", access (0:read/write)=enum16{"read/write", "read-only", "write-only"}."read-only") -> (refnum out=w1329:refnum<file>, error out=w1315:errorcluster)  [unwired: 1 in, 3 out]
        n825 = Deny Access(4:w1315, 7:w1329) -> (0:w1314:errorcluster, 3:w1320:refnum<file>)  [unwired: 1 out]
        n826 = Read from Binary File(5:0.0, 8:w1314, 9:T29."big-endian, network order" ("byte order (0:big-endian, network order)"), 10:-1 ("count (1)"), 11:w1320) -> (0:w1313:errorcluster, 2:w1311:dbl[], 3:w1316:refnum<file>)  [unwired: 2 out]
        n827 = Array To Cluster(array=w1311) -> (cluster=w1310:T31)
        n828 = Unbundle(w1310) -> ("[0]"=w1309:dbl, "[1]"=w1308:dbl, "[2]"=w1307:dbl, "[3]"=w1306:dbl, "[4]"=w1305:dbl, "[5]"=w1304:dbl)
        n829 = Close File(refnum=w1316, error in=w1313) -> (error out=→"Read cal error":errorcluster)  [unwired: 1 out]
        n830 = Multiply(x=w1304, y=w1301) -> (x*y=w1302:dbl)
        n831 = local write "T2 kappa_x (pN/nm)"(w1306) -> ()
        n832 = local write "T1 kappa_x (pN/nm)"(w1307) -> ()
        n833 = local write "T1 alpha_x (nm/V)"(w1309) -> ()
        n834 = local write "T2 alpha_x (nm/V)"(w1308) -> ()
        n835 = Multiply(x=w1305, y=w1301) -> (x*y=w1303:dbl)
        n836 = local write "T1 offset_x (mV)"(w1303) -> ()
        n837 = local write "T2 offset_x (mV)"(w1302) -> ()
      }
      event "Abort MCL Scan": Value Change {
        n838 = event-data() -> ()  [unwired: 7 out]
        n839 = local write "MCL Scanning"(FALSE ("MCL Scanning")) -> ()
        n840 = xnode "Read/Write Control"("FPGA VI Reference In"=w1334, "error in"=w1333, "Abort scan (MCL)"="Abort MCL Scan") -> ("error out"=w1332:errorcluster)  [unwired: 1 out]
      }
      event "Update Count (MCL)": Value Change {
        n841 = event-data() -> ()  [unwired: 7 out]
        n842 = xnode "Read/Write Control"("FPGA VI Reference In"=w1338, "error in"=w1337, "MCL count"="Update Count (MCL)") -> ("error out"=w1336:errorcluster)  [unwired: 1 out]
      }
      event "Phase adjust (MCL)", "+ phase (MCL)", "- phase (MCL)": Value Change {
        n843 = event-data() -> ()  [unwired: 7 out]
        n844 = Negate(x="Phase adjust (MCL)") -> (-x=w1347:i16)
        n845 = Select(t=w1347, s="- phase (MCL)", f="Phase adjust (MCL)") -> (s? t:f=w1345:i16)
        n846 = Or(x="- phase (MCL)", y="+ phase (MCL)") -> (x .or. y?=w1340:bool)
        n847 = xnode "Read/Write Control"("FPGA VI Reference In"=w1349, "error in"=w1348, "Phase count adjustment (MCL)"=w1345) -> ("FPGA VI Reference Out"=w1341:T19, "error out"=w1342:errorcluster)
        n848 = xnode "Read/Write Control"("FPGA VI Reference In"=w1341, "error in"=w1342, "+ phase (MCL)"=w1340) -> ("error out"=w1339:errorcluster)  [unwired: 1 out]
      }
      event "Abort AOD Scan": Value Change {
        n849 = event-data() -> ()  [unwired: 7 out]
        n850 = xnode "Read/Write Control"("FPGA VI Reference In"=w1353, "error in"=w1352, "Abort scan"="Abort AOD Scan") -> ("error out"=w1351:errorcluster)  [unwired: 1 out]
      }
      event "Continuous AOD Scanning": Value Change {
        n851 = event-data() -> ()  [unwired: 7 out]
        n852 = xnode "Read/Write Control"("FPGA VI Reference In"=w1357, "error in"=w1356, "Cont. Scan"="Continuous AOD Scanning") -> ("error out"=w1355:errorcluster)  [unwired: 1 out]
      }
      event "Index": Value Change {
        n853 = event-data() -> ()  [unwired: 7 out]
        n854 = call "Create new save file.vi"("Insert"="", "Ext"=".dat" ("string"), "Index In"="Index") -> ("Path Out"=→"Save file name":path, "Index Out"=w1358:dbl)
        "Save index" <- w1358
        n855 = local write "Index"(w1358) -> ()
      }
      event "AO1", "AO2": Value Change {
        w1373 = 10.0 ("y")
        w1372 = 32767.0 ("y")
        n856 = event-data() -> ()  [unwired: 7 out]
        n857 = local read "AO2"() -> (w1371:dbl)
        n858 = local read "AO1"() -> (w1368:dbl)
        n859 = Multiply(x=w1368, y=w1372) -> (x*y=w1367:dbl)
        n860 = Multiply(x=w1371, y=w1372) -> (x*y=w1370:dbl)
        n861 = Divide(x=w1367, y=w1373) -> (x/y=w1366:dbl)
        n862 = Divide(x=w1370, y=w1373) -> (x/y=w1369:dbl)
        n863 = To Word Integer(number=w1366) -> (16bit integer=w1374:i16)
        n864 = To Word Integer(number=w1369) -> (16bit integer=w1375:i16)
        n865 = xnode "Read/Write Control"("FPGA VI Reference In"=w1365, "error in"=w1364, "AO1"=w1374, "AO2"=w1375) -> ("error out"=w1363:errorcluster)  [unwired: 1 out]
      }
      event "Inject Bottom": Value Change {
        n866 = event-data() -> ()  [unwired: 7 out]
        n867 = disable-structure shown="Enabled" {
          disable-tunnel: "Inject Bottom" -> [w1377 w1417]
          frame Disabled {
            n868 = local read "Chemyx Syringe Pump Serial Port"() -> (w1378:refnum<visa-resource-name>)
            n869 = local read "Pump write delay (ms)"() -> (w1379:dbl)
            n870 = case shown="True" w1377 {
              tunnel: w1379 -> [w1385 w1399]
              tunnel: w1378 -> [w1382 w1398]
              frame False {
                n871 = flat-sequence {
                  tunnel: w1382 -> [w1386]
                  tunnel: [w1386] -> w1383
                  tunnel: w1385 -> [_]
                  tunnel: [w1389] -> w1384
                  tunnel: w1383 -> [w1389]
                  tunnel: w1384 -> [w1390]
                  tunnel: [w1390] -> w1380
                  tunnel: [w1392] -> w1381
                  tunnel: w1380 -> [w1392]
                  tunnel: w1381 -> [w1394]
                  frame #0 {
                    n872 = call "Write to pump.vi"("string"="enter pump1", "VISA resource name"=w1386) -> ()  [unwired: 1 out]
                  }
                  frame #1 {
                    n873 = Wait (ms)(milliseconds to wait="Pump pause delay (ms)") -> ()  [unwired: 1 out]
                  }
                  frame #2 {
                    n874 = call "Write to pump.vi"("string"="stop", "VISA resource name"=w1390) -> ()  [unwired: 1 out]
                  }
                  frame #3 {
                    n875 = Wait (ms)(milliseconds to wait=u32 500) -> ()  [unwired: 1 out]
                  }
                  frame #4 {
                    n876 = call "Write to pump.vi"("string"="stop", "VISA resource name"=w1394) -> ()  [unwired: 1 out]
                  }
                }
              }
              frame True {
                n877 = flat-sequence {
                  tunnel: w1398 -> [w1408]
                  tunnel: w1399 -> [w1403]
                  tunnel: w1399 -> [w1410]
                  tunnel: w1398 -> [w1411]
                  tunnel: [w1411] -> w1396
                  tunnel: [w1413] -> w1397
                  tunnel: w1396 -> [w1413]
                  tunnel: w1397 -> [w1415]
                  frame #0 {
                    n878 = local read "All Pump Parameters"() -> (w1402:T5)
                    n879 = Unbundle By Name(w1402) -> ("Pump 1"=w1409:T32)
                    n880 = call "Set pump parameters.vi"("Pump write delay (ms)"=w1403, "Volume (uL)"="Ch 2 Inject Volume (uL)", "Rate (uL/h)"="Ch 1 Inject Rate (ul/h)", "Units"=4.0, "Pump #"=1.0, "Pump Parameters In"=w1409, "VISA resource name"=w1408) -> ("Pump Parameters Out"=w1401:T32)  [unwired: 3 in]
                    n881 = Bundle By Name(cluster=w1402, "Pump 1"=w1401) -> (w1400:T5)
                    n882 = local write "All Pump Parameters"(w1400) -> ()
                  }
                  frame #1 {
                    n883 = Wait (ms)(milliseconds to wait=w1410) -> ()  [unwired: 1 out]
                  }
                  frame #2 {
                    n884 = call "Write to pump.vi"("string"="start", "VISA resource name"=w1411) -> ()  [unwired: 1 out]
                  }
                  frame #3 {
                    n885 = Wait (ms)(milliseconds to wait=u32 500) -> ()  [unwired: 1 out]
                  }
                  frame #4 {
                    n886 = call "Write to pump.vi"("string"="start", "VISA resource name"=w1415) -> ()  [unwired: 1 out]
                  }
                }
              }
            }
          }
          frame Enabled {
            n887 = call "hamilton_controller.vi"("Open?"=w1417, "valve"=enum16{"A", "B", "C", "D", "ALL"}."B", "action"=T20."MOVE VALVE") -> ()  [unwired: 8 in, 1 out]
          }
        }
      }
      event "Inject Top": Value Change {
        n888 = event-data() -> ()  [unwired: 7 out]
        n889 = disable-structure shown="Disabled" {
          disable-tunnel: "Inject Top" -> [_ w1461]
          frame Disabled {
            n890 = local read "Pump write delay (ms)"() -> (w1422:dbl)
            n891 = case shown="False" w1423 {
              tunnel: w1422 -> [w1429 w1443]
              tunnel: "Chemyx Syringe Pump Serial Port" -> [w1426 w1442]
              frame False {
                n892 = flat-sequence {
                  tunnel: w1426 -> [w1430]
                  tunnel: [w1430] -> w1427
                  tunnel: w1429 -> [_]
                  tunnel: [w1433] -> w1428
                  tunnel: w1427 -> [w1433]
                  tunnel: w1428 -> [w1434]
                  tunnel: [w1434] -> w1424
                  tunnel: [w1436] -> w1425
                  tunnel: w1424 -> [w1436]
                  tunnel: w1425 -> [w1438]
                  frame #0 {
                    n893 = call "Write to pump.vi"("string"="enter pump3", "VISA resource name"=w1430) -> ()  [unwired: 1 out]
                  }
                  frame #1 {
                    n894 = local read "Pump pause delay (ms)"() -> (w1432:u32)
                    n895 = Wait (ms)(milliseconds to wait=w1432) -> ()  [unwired: 1 out]
                  }
                  frame #2 {
                    n896 = call "Write to pump.vi"("string"="stop", "VISA resource name"=w1434) -> ()  [unwired: 1 out]
                  }
                  frame #3 {
                    n897 = Wait (ms)(milliseconds to wait=u32 0) -> ()  [unwired: 1 out]
                  }
                  frame #4 {
                    n898 = call "Write to pump.vi"("string"="stop", "VISA resource name"=w1438) -> ()  [unwired: 1 out]
                  }
                }
              }
              frame True {
                n899 = flat-sequence {
                  tunnel: w1442 -> [w1452]
                  tunnel: w1443 -> [w1447]
                  tunnel: w1443 -> [w1454]
                  tunnel: w1442 -> [w1455]
                  tunnel: [w1455] -> w1440
                  tunnel: [w1458] -> w1441
                  tunnel: w1440 -> [w1458]
                  tunnel: w1441 -> [w1459]
                  frame #0 {
                    n900 = local read "All Pump Parameters"() -> (w1446:T5)
                    n901 = Unbundle By Name(w1446) -> ("Pump 3"=w1453:T32)
                    n902 = call "Set pump parameters.vi"("Pump write delay (ms)"=w1447, "Volume (uL)"="Ch 3 Inject Volume (uL)", "Rate (uL/h)"="Ch 3 Inject Rate (ul/h)", "Units"=4.0, "Pump #"=3.0, "Pump Parameters In"=w1453, "VISA resource name"=w1452) -> ("Pump Parameters Out"=w1445:T32)  [unwired: 3 in]
                    n903 = Bundle By Name(cluster=w1446, "Pump 3"=w1445) -> (w1444:T5)
                    n904 = local write "All Pump Parameters"(w1444) -> ()
                  }
                  frame #1 {
                    n905 = Wait (ms)(milliseconds to wait=w1454) -> ()  [unwired: 1 out]
                  }
                  frame #2 {
                    n906 = call "Write to pump.vi"("string"="start", "VISA resource name"=w1455) -> ()  [unwired: 1 out]
                  }
                  frame #3 {
                    n907 = Wait (ms)(milliseconds to wait=u32 500) -> ()  [unwired: 1 out]
                  }
                  frame #4 {
                    n908 = call "Write to pump.vi"("string"="start", "VISA resource name"=w1459) -> ()  [unwired: 1 out]
                  }
                }
              }
            }
          }
          frame Enabled {
            n909 = call "hamilton_controller.vi"("Open?"=w1461, "valve"=enum16{"A", "B", "C", "D", "ALL"}."A", "action"=T20."MOVE VALVE") -> ()  [unwired: 8 in, 1 out]
          }
        }
      }
      event "Inject Valve B": Value Change {
        n910 = event-data() -> ()  [unwired: 7 out]
        n911 = disable-structure shown="Enabled" {
          disable-tunnel: "Inject Valve B" -> [w1465 w1485]
          frame Disabled {
            n912 = local read "Pump write delay (ms)"() -> (w1467:dbl)
            n913 = flat-sequence {
              tunnel: w1466 -> [w1480]
              tunnel: w1467 -> [w1476]
              tunnel: w1465 -> [_]
              tunnel: w1467 -> [w1482]
              tunnel: w1466 -> [w1483]
              frame #0 {
                n914 = local read "All Pump Parameters"() -> (w1475:T5)
                n915 = Multiply(x=60.0, y="Flush Center Ch Rate (ul/m)") -> (x*y=w1472:dbl)
                n916 = Unbundle By Name(w1475) -> ("Pump 2"=w1481:T32)
                n917 = call "Set pump parameters.vi"("Pump write delay (ms)"=w1476, "Volume (uL)"="Flush Center Ch Volume (uL)", "Rate (uL/h)"=w1472, "Units"=3.0, "Pump #"=2.0, "Pump Parameters In"=w1481, "VISA resource name"=w1480) -> ("Pump Parameters Out"=w1474:T32)  [unwired: 3 in]
                n918 = Bundle By Name(cluster=w1475, "Pump 2"=w1474) -> (w1473:T5)
                n919 = local write "All Pump Parameters"(w1473) -> ()
                n920 = Add(x="Flush Center Ch Volume (uL)", y="Total Volume\nFlushed (uL)") -> (x+y=w1469:dbl)
                n921 = local write "Total Volume\nFlushed (uL)"(w1469) -> ()
              }
              frame #1 {
                n922 = Wait (ms)(milliseconds to wait=w1482) -> ()  [unwired: 1 out]
              }
              frame #2 {
                n923 = call "Write to pump.vi"("string"="start", "VISA resource name"=w1483) -> ()  [unwired: 1 out]
              }
            }
            n924 = local read "Chemyx Syringe Pump Serial Port"() -> (w1466:refnum<visa-resource-name>)
          }
          frame Enabled {
            n925 = call "hamilton_controller.vi"("Open?"=w1485, "valve"=enum16{"A", "B", "C", "D", "ALL"}."B", "action"=T20."MOVE VALVE") -> ()  [unwired: 8 in, 1 out]
          }
        }
      }
      event "Sample Channel Flow": Value Change {
        n926 = event-data() -> ()  [unwired: 7 out]
        n927 = call "hamilton_controller.vi"("Open?"="Sample Channel Flow", "valve"=enum16{"A", "B", "C", "D", "ALL"}."C", "action"=T20."MOVE VALVE") -> ()  [unwired: 8 in, 1 out]
      }
      event "Flip Green Filter": Value Change {
        n928 = event-data() -> ()  [unwired: 7 out]
        n929 = local write "Flip Green Filter"("Flip Green Filter") -> ()
        n930 = flat-sequence {
          tunnel: w1498 -> [w1503]
          tunnel: w1497 -> [w1502]
          tunnel: [w1500] -> w1495
          tunnel: [w1499] -> w1494
          tunnel: [w1505] -> w1493
          tunnel: w1495 -> [w1505]
          tunnel: [w1504] -> w1492
          tunnel: w1494 -> [w1504]
          tunnel: w1493 -> [w1509]
          tunnel: w1492 -> [w1508]
          tunnel: [w1507] -> w1496
          frame #0 {
            n931 = xnode "Read/Write Control"("FPGA VI Reference In"=w1503, "error in"=w1502, "Green Filter Flipper"=TRUE) -> ("FPGA VI Reference Out"=w1500:T19, "error out"=w1499:errorcluster)
          }
          frame #1 {
            n932 = Wait (ms)(milliseconds to wait=u32 100) -> ()  [unwired: 1 out]
          }
          frame #2 {
            n933 = xnode "Read/Write Control"("FPGA VI Reference In"=w1509, "error in"=w1508, "Green Filter Flipper"=FALSE) -> ("error out"=w1507:errorcluster)  [unwired: 1 out]
          }
        }
      }
      event "Pump 1 contents", "Pump 3 contents": Value Change {
        n934 = event-data() -> ()  [unwired: 7 out]
        n935 = local read "Pump 1 contents"() -> (→"Pump 1 cont disp":string)
        n936 = local read "Pump 3 contents"() -> (→"Pump 3 cont disp":string)
      }
      event "Reset Trap Pos. FB": Value Change {
        n937 = event-data() -> ()  [unwired: 7 out]
        n938 = xnode "Read/Write Control"("FPGA VI Reference In"=w1515, "error in"=w1514, "Trap Pos. FB Reset"="Reset Trap Pos. FB") -> ()  [unwired: 2 out]
      }
      event "Trap Pos. FB ON": Value Change {
        n939 = event-data() -> ()  [unwired: 7 out]
        n940 = xnode "Read/Write Control"("FPGA VI Reference In"=w1518, "error in"=w1517, "Force feedback"="Trap Pos. FB ON") -> ()  [unwired: 2 out]
      }
      event "Trap Pos. FB Range", "Trap Pos. FB Gains", "Trap Pos. FB Mult Factor", "Trap Pos. FB Offset Factor", "Trap Pos FB Negate Action", "Trap Pos FB Monitor\nT1 or T2": Value Change {
        n941 = event-data() -> ()  [unwired: 7 out]
        n942 = xnode "Read/Write Control"("FPGA VI Reference In"=w1527, "error in"=w1526, "Trap Pos. FB Range"="Trap Pos. FB Range", "Trap Pos. FB Gains"="Trap Pos. FB Gains", "Trap Pos. FB Mult Factor"="Trap Pos. FB Mult Factor", "Trap Pos. FB Offset Factor"="Trap Pos. FB Offset Factor", "Trap Pos FB Negate Action"="Trap Pos FB Negate Action", "Trap Pos FB Monitor T1 or T2"="Trap Pos FB Monitor\nT1 or T2", "AI1 X Scale"="Trap Pos. AI1 X Pre-scale") -> ()  [unwired: 2 out]
      }
      event "Trap Pos FB SP": Value Change {
        n943 = event-data() -> ()  [unwired: 7 out]
        n944 = xnode "Read/Write Control"("FPGA VI Reference In"=w1530, "error in"=w1529, "Trap Pos. FB SP"="Trap Pos FB SP") -> ()  [unwired: 2 out]
      }
      event "Set SP to Reading": Value Change {
        n945 = event-data() -> ()  [unwired: 7 out]
        n946 = local read "Trap Pos FB Monitor\nT1 or T2"() -> (w1538:bool)
        n947 = local read "Trap X AI1 (DMA)"() -> (w1541:T13)
        n948 = local read "Trap X (AI1)"() -> (w1544:T10)
        n949 = Unbundle By Name(w1544) -> ("Trap 1"=w1543:fxp<+/-,16,1>, "Trap 2"=w1542:fxp<+/-,16,1>)
        n950 = Unbundle By Name(w1541) -> ("Set 1"=w1540:fxp<+/-,16,1>, "Set 2"=w1539:fxp<+/-,16,1>)
        n951 = Select(t=w1543, s=w1538, f=w1542) -> (s? t:f=w1537:fxp<+/-,16,1>)
        n952 = Select(t=w1540, s=w1538, f=w1539) -> (s? t:f=w1536:fxp<+/-,16,1>)
        n953 = Not(x="Set SP Using...") -> (.not. x?=w1531:bool)
        n954 = Select(t=w1537, s=w1531, f=w1536) -> (s? t:f=w1532:fxp<+/-,16,1>)
        n955 = xnode "Read/Write Control"("FPGA VI Reference In"=w1534, "error in"=w1533, "Trap Pos. FB SP"=w1532) -> ()  [unwired: 2 out]
        n956 = local write "Trap Pos FB SP"(w1532) -> ()
      }
      event "Trap Pos. FB Out Scale 2^n": Value Change {
        n957 = event-data() -> ()  [unwired: 7 out]
        n958 = Scale By Power Of 2(n="Trap Pos. FB Out Scale 2^n", x=ext 1.0) -> (x*2^n=w1546:ext)
        n959 = property on="Trap Pos. FB Mult Factor" class="DigNum (strict)"("Val(Sgnl)"=w1546) -> ()  [unwired: 2 in, 2 out]
      }
      event "Trap Pos FB Int Count": Value Change {
        n960 = event-data() -> ()  [unwired: 7 out]
        n961 = xnode "Read/Write Control"("FPGA VI Reference In"=w1551, "error in"=w1550, "Trap Pos FB Int Count"="Trap Pos FB Int Count") -> ()  [unwired: 2 out]
      }
    }
    "error out 2" <- w735
    n962 = node-c288() -> ()  [unwired: 1 in, 1 out]
  }
  n963 = node-c288() -> (w69:T24)  [unwired: 4 in]
  n964 = timed-loop "Run Scripts, including: stage motion" {
    timing: w69 -> [_]
    timing-out: [_] -> w68
    tunnel: w24 -> [_]
    stop <- w1553 stop-if-true
    n965 = node-c288() -> ()  [unwired: 1 in, 1 out]
    n966 = event shown="[1] Timeout" {
      selector: _ -> [_ _ _ _ _ _ _ _ _ _ _ _]
      dyn-events: _ -> [_ _ _ _ _ _ _ _ _ _ _ _]
      timeout: 50 -> [_ _ _ _ _ _ _ _ _ _ _ _]
      tunnel: ["Move Cap. 1 (DNA Top)" _ "Cal/Data Acq. Spot" "Dump Beads" "Dip for Protein" _ "Got ADig bead" "Got DNA bead" "Take Stepping Data" _ "Take Detection Laser\nImage" _] -> _
      tunnel: [_ _ _ _ _ _ _ _ _ _ _ w1761] -> w1553
      event "Move Cap. 1 (DNA Top)": Value Change {
        n967 = event-data() -> ()  [unwired: 1 in, 5 out]
        n968 = local write "Move Cap. 1 (DNA Top)"(FALSE ("Move Cap. 1 (DNA Right)")) -> ()
        n969 = flat-sequence {
          tunnel: "Cap 1 Samp Flow ON" -> [w1559]
          frame #0 {
            n970 = local write "Stage Moving"(FALSE ("Stage Moving")) -> ()
            n971 = case "stop flow" shown="True" w1559 {
              frame False {
              }
              frame True {
                n972 = call "hamilton_controller.vi"("Open?"=FALSE, "valve"=enum16{"A", "B", "C", "D", "ALL"}."C", "action"=T20."MOVE VALVE") -> ()  [unwired: 8 in, 1 out]
              }
            }
            n973 = case shown="True" TRUE {
              tunnel: "Cap 1 T ON" -> [w1568 w1569]
              frame False {
                n974 = property on="Trap 1 (ON/OFF)" class="Bool (strict)"("Val(Sgnl)"=w1568) -> ()  [unwired: 2 in, 2 out]
              }
              frame True {
                n975 = property on="Trap 2 (ON/OFF)" class="Bool (strict)"("Val(Sgnl)"=w1569) -> ()  [unwired: 2 in, 2 out]
              }
            }
            n976 = call <vilib>:"Beep.vi"() -> ()  [unwired: 3 in, 9 out]
            n977 = case shown="True" "Cap 1 Flow ON" {
              frame False {
              }
              frame True {
                n978 = property on="Inject Top" class="Bool (strict)"("Val(Sgnl)"=TRUE ("Value (Signaling)")) -> ()  [unwired: 2 in, 2 out]
              }
            }
          }
        }
      }
      event Timeout {
        n979 = event-data() -> ()  [unwired: 1 in, 2 out]
      }
      event "Cal/Data Acq. Spot": Value Change {
        # "wait for calibration file\nto be written"
        # "signal save cal true\nthis tells the data \nacquisition loop to\nstart sending the data\nto a calibration file"
        # "separate traps to\nthe desired trap delta"
        # "move stage to data acquisition spot"
        # "CHANGE FISH FOR TETHER BACK\nTO TRUE VALUE HERE."
        n980 = event-data() -> ()  [unwired: 1 in, 5 out]
        n981 = local write "Cal/Data Acq. Spot"(FALSE ("Cal/Data Acq. Spot")) -> ()
        n982 = flat-sequence {
          tunnel: ["Cal @ (MHz)"] -> w1570
          tunnel: w1570 -> [w1580]
          tunnel: w1570 -> [w1601]
          frame #0 {
            n983 = property on="Trap Delta (MHz)" class="DigNum (strict)"("Val(Sgnl)"="Cal @ (MHz)") -> ()  [unwired: 2 in, 2 out]
            n984 = call <vilib>:"Beep.vi"() -> ()  [unwired: 3 in, 9 out]
          }
          frame #1 {
            n985 = Wait (ms)(milliseconds to wait=u32 100) -> ()  [unwired: 1 out]
          }
          frame #2 {
            n986 = property on="Save Calibration" class="Bool (strict)"("Val(Sgnl)"=TRUE ("Value (Signaling)")) -> ()  [unwired: 2 in, 2 out]
          }
          frame #3 {
            n987 = Wait (ms)(milliseconds to wait=u32 4000) -> ()  [unwired: 1 out]
          }
          frame #4 {
            n988 = while {
              stop <- w1577 stop-if-true
              n989 = local read "Saving..."() -> (w1578:bool)
              n990 = Wait (ms)(milliseconds to wait=u32 100) -> ()  [unwired: 1 out]
              n991 = Not(x=w1578) -> (.not. x?=w1577:bool)
            }
          }
          frame #5 {
            n992 = case shown="True" "W/ Offset 1" {
              tunnel: w1580 -> [_ w1582]
              frame False {
              }
              frame True {
                n993 = stacked-sequence {
                  tunnel: w1582 -> [_ _ _ _ _ _ _ w1599]
                  frame #0 {
                    n994 = Replace Array Subset(array=u32[] [0] ("Index Values"), new element="Offset 1 Set", index=0) -> (w1583:u32[])
                    n995 = property on="Saved AOD Raster Scan Parameter Sets" class="Arr (strict)"("Index Values"=w1583) -> ()  [unwired: 2 in, 2 out]
                    n996 = property on="Trap Delta (MHz)" class="DigNum (strict)"("Val(Sgnl)"="Offset 1 Start (MHz)") -> ()  [unwired: 2 in, 2 out]
                  }
                  frame #1 {
                    n997 = Wait (ms)(milliseconds to wait=u32 200) -> ()  [unwired: 1 out]
                  }
                  frame #2 {
                    n998 = property on="Load parameters" class="Bool (strict)"("Val(Sgnl)"=TRUE ("Value (Signaling)")) -> ()  [unwired: 2 in, 2 out]
                  }
                  frame #3 {
                    n999 = Wait (ms)(milliseconds to wait=u32 200) -> ()  [unwired: 1 out]
                  }
                  frame #4 {
                    n1000 = property on="Trap Raster Scan" class="Bool (strict)"("Val(Sgnl)"=TRUE ("Value (Signaling)")) -> ()  [unwired: 2 in, 2 out]
                  }
                  frame #5 {
                    n1001 = Wait (ms)(milliseconds to wait=u32 2000) -> ()  [unwired: 1 out]
                  }
                  frame #6 {
                    n1002 = while {
                      stop <- w1596 stop-if-true
                      n1003 = local read "Raster Scanning..."() -> (w1598:bool)
                      n1004 = local read "Saving..."() -> (w1594:bool)
                      n1005 = Wait (ms)(milliseconds to wait=u32 100) -> ()  [unwired: 1 out]
                      n1006 = Not(x=w1594) -> (.not. x?=w1593:bool)
                      n1007 = Not(x=w1598) -> (.not. x?=w1595:bool)
                      n1008 = And(x=w1595, y=w1593) -> (x .and. y?=w1596:bool)
                    }
                  }
                  frame #7 {
                    n1009 = property on="Trap Delta (MHz)" class="DigNum (strict)"("Val(Sgnl)"=w1599) -> ()  [unwired: 2 in, 2 out]
                  }
                }
              }
            }
          }
          frame #6 {
            n1010 = local read "Save ave N"() -> (w1600:dbl)
            n1011 = case shown="True" "W/ Offset 2" {
              tunnel: w1601 -> [_ w1607]
              tunnel: w1600 -> [_ w1606]
              frame False {
                n1012 = Multiply(x="Cal read wait (s)", y=u32 1000 ("milliseconds to wait")) -> (x*y=w1604:u32)
                n1013 = Wait (ms)(milliseconds to wait=w1604) -> ()  [unwired: 1 out]
              }
              frame True {
                n1014 = stacked-sequence {
                  tunnel: w1607 -> [_ _ _ _ _ _ _ _ _ w1628 _ _]
                  tunnel: w1606 -> [_ _ _ _ _ _ _ _ _ w1626 _ _]
                  frame #0 {
                    n1015 = property on="Save ave N" class="DigNum (strict)"("Val(Sgnl)"=1.0 ("Value (Signaling)")) -> ()  [unwired: 2 in, 2 out]
                  }
                  frame #1 {
                    n1016 = Wait (ms)(milliseconds to wait=u32 500) -> ()  [unwired: 1 out]
                  }
                  frame #2 {
                    n1017 = property on="Trap Delta (MHz)" class="DigNum (strict)"("Val(Sgnl)"="Offset 2 Start (MHz)") -> ()  [unwired: 2 in, 2 out]
                    n1018 = Replace Array Subset(array=u32[] [0] ("Index Values"), new element="Offset 2 Set", index=0) -> (w1612:u32[])
                    n1019 = property on="Saved AOD Raster Scan Parameter Sets" class="Arr (strict)"("Index Values"=w1612) -> ()  [unwired: 2 in, 2 out]
                  }
                  frame #3 {
                    n1020 = Wait (ms)(milliseconds to wait=u32 500) -> ()  [unwired: 1 out]
                  }
                  frame #4 {
                    n1021 = property on="Load parameters" class="Bool (strict)"("Val(Sgnl)"=TRUE ("Value (Signaling)")) -> ()  [unwired: 2 in, 2 out]
                  }
                  frame #5 {
                    n1022 = Wait (ms)(milliseconds to wait=u32 500) -> ()  [unwired: 1 out]
                  }
                  frame #6 {
                    n1023 = property on="Trap Raster Scan" class="Bool (strict)"("Val(Sgnl)"=TRUE ("Value (Signaling)")) -> ()  [unwired: 2 in, 2 out]
                  }
                  frame #7 {
                    n1024 = Wait (ms)(milliseconds to wait=u32 2000) -> ()  [unwired: 1 out]
                  }
                  frame #8 {
                    n1025 = while {
                      stop <- w1621 stop-if-true
                      n1026 = local read "Raster Scanning..."() -> (w1624:bool)
                      n1027 = local read "Saving..."() -> (w1622:bool)
                      n1028 = Wait (ms)(milliseconds to wait=u32 100) -> ()  [unwired: 1 out]
                      n1029 = Not(x=w1622) -> (.not. x?=w1620:bool)
                      n1030 = Not(x=w1624) -> (.not. x?=w1623:bool)
                      n1031 = And(x=w1623, y=w1620) -> (x .and. y?=w1621:bool)
                    }
                  }
                  frame #9 {
                    n1032 = property on="Trap Delta (MHz)" class="DigNum (strict)"("Val(Sgnl)"=w1628) -> ()  [unwired: 2 in, 2 out]
                    n1033 = property on="Saved AOD Raster Scan Parameter Sets" class="Arr (strict)"("Index Values"=u32[] [0]) -> ()  [unwired: 2 in, 2 out]
                    n1034 = property on="Save ave N" class="DigNum (strict)"("Val(Sgnl)"=w1626) -> ()  [unwired: 2 in, 2 out]
                  }
                  frame #10 {
                    n1035 = Wait (ms)(milliseconds to wait=u32 500) -> ()  [unwired: 1 out]
                  }
                  frame #11 {
                    n1036 = property on="Load parameters" class="Bool (strict)"("Val(Sgnl)"=TRUE ("Value (Signaling)")) -> ()  [unwired: 2 in, 2 out]
                  }
                }
              }
            }
          }
          frame #7 {
            n1037 = property on="Read Cal" class="Bool (strict)"("Val(Sgnl)"=TRUE ("Value (Signaling)")) -> ()  [unwired: 2 in, 2 out]
          }
          frame #8 {
            n1038 = Wait (ms)(milliseconds to wait=u32 500) -> ()  [unwired: 1 out]
          }
          frame #9 {
            n1039 = property on="Fish for Tether" class="Bool (strict)"("Val(Sgnl)"=FALSE ("Value (Signaling)")) -> ()  [unwired: 2 in, 2 out]
          }
        }
      }
      event "Dump Beads": Value Change {
        # "SCRIPT TO REMOVE BOTH BEADS FROM THE TRAPS. TURNS ON LIGHT WHICH INDICATES THAT STAGE IS MOVING. THEN STOPS SAVING DATA. \nSETS Sample Channel Flow TO TRUE. STOPS INTERLACING GREEN FLUORESCENCE. TURNS OFF Tether INDICATOR BECAUSE WE ARE THROWING IT\nAWAY. SHUTS OFF TRAP POSITION FEEDBACK."
        n1040 = event-data() -> ()  [unwired: 1 in, 5 out]
        n1041 = flat-sequence {
          frame #0 {
            w1635 = FALSE ("Fl. Triggered...")
            w1636 = TRUE ("Stage Moving")
            n1042 = local read "Saving..."() -> (w1637:bool)
            n1043 = local write "Fl. Triggered..."(w1635) -> ()
            n1044 = local write "Stage Moving"(w1636) -> ()
            n1045 = local write "Tether"(w1635) -> ()
            n1046 = property on="Green Laser ON/Interlacing" class="Bool (strict)"("Val(Sgnl)"=w1635) -> ()  [unwired: 2 in, 2 out]
            n1047 = property on="Trap Pos. FB ON" class="Bool (strict)"("Val(Sgnl)"=w1635) -> ()  [unwired: 2 in, 2 out]
            n1048 = property on="Sample Channel Flow" class="Bool (strict)"("Val(Sgnl)"=w1636) -> ()  [unwired: 2 in, 2 out]
            n1049 = local write "Stop Saving"(w1637) -> ()
          }
          frame #1 {
            w1638 = FALSE ("Value (Signaling)")
            # "TURNS TRAPS OFF SO THAT\nBEADS REMAIN AT DUMP \nBEADS POSITION"
            n1050 = property on="Trap 1 (ON/OFF)" class="Bool (strict)"("Val(Sgnl)"=w1638) -> ()  [unwired: 2 in, 2 out]
            n1051 = property on="Trap 2 (ON/OFF)" class="Bool (strict)"("Val(Sgnl)"=w1638) -> ()  [unwired: 2 in, 2 out]
            n1052 = call <vilib>:"Beep.vi"() -> ()  [unwired: 3 in, 9 out]
          }
          frame #2 {
            n1053 = property on="Goto Bottom (F7)" class="Bool (strict)"("Val(Sgnl)"=TRUE ("Value (Signaling)")) -> ()  [unwired: 2 in, 2 out]
          }
          frame #3 {
            n1054 = Wait (ms)(milliseconds to wait=u32 8000) -> ()  [unwired: 1 out]
          }
          frame #4 {
            n1055 = property on="Trap Delta (MHz)" class="DigNum (strict)"("Val(Sgnl)"=20.0 ("Value (Signaling)")) -> ()  [unwired: 2 in, 2 out]
          }
          frame #5 {
            n1056 = property on="Trap 2 (ON/OFF)" class="Bool (strict)"("Val(Sgnl)"=TRUE ("Value (Signaling)")) -> ()  [unwired: 2 in, 2 out]
          }
          frame #6 {
            n1057 = property on="Sample Channel Flow" class="Bool (strict)"("Val(Sgnl)"=FALSE ("Value (Signaling)")) -> ()  [unwired: 2 in, 2 out]
          }
        }
      }
      event "Dip for Protein": Value Change {
        n1058 = event-data() -> ()  [unwired: 1 in, 5 out]
        n1059 = flat-sequence {
          frame #0 {
            n1060 = case shown="True" "Move Trap Before?" {
              frame False {
              }
              frame True {
                n1061 = property on="Trap Delta (MHz)" class="DigNum (strict)"("Val(Sgnl)"="Dip Trap Delta 1 (MHz)") -> ()  [unwired: 2 in, 2 out]
              }
            }
          }
          frame #1 {
            n1062 = Multiply(x="Duration (s)", y=1000.0) -> (x*y=w1647:dbl)
            n1063 = Wait (ms)(milliseconds to wait=w1647) -> ()  [unwired: 1 out]
          }
          frame #2 {
            n1064 = case shown="True" "Move Trap After?" {
              frame False {
              }
              frame True {
                n1065 = property on="Trap Delta (MHz)" class="DigNum (strict)"("Val(Sgnl)"="Dip Trap Delta 2 (MHz)") -> ()  [unwired: 2 in, 2 out]
              }
            }
          }
          frame #3 {
            n1066 = case shown="True" "Green ON After?" {
              frame False {
              }
              frame True {
                n1067 = property on="Green Laser ON/Interlacing" class="Bool (strict)"("Val(Sgnl)"=TRUE ("Value (Signaling)")) -> ()  [unwired: 2 in, 2 out]
              }
            }
          }
          frame #4 {
            n1068 = Wait (ms)(milliseconds to wait=u32 500) -> ()  [unwired: 1 out]
          }
          frame #5 {
            n1069 = case shown="True" "Save Data After?" {
              frame False {
              }
              frame True {
                n1070 = property on="Start Saving" class="Bool (strict)"("Val(Sgnl)"=TRUE ("Value (Signaling)")) -> ()  [unwired: 2 in, 2 out]
              }
            }
          }
        }
      }
      event "Profile": Value Change {
        n1071 = event-data() -> ()  [unwired: 1 in, 5 out]
        n1072 = flat-sequence {
          frame #0 {
            w1657 = 0.0 ("element")
            n1073 = Build Array(w1657, "Y change (mm)", w1657) -> ()  [unwired: 1 out]
          }
          frame #1 {
            # "stop saving"
            n1074 = local write "Stop Saving"(TRUE ("Stop Saving")) -> ()
            n1075 = local write "Stage Moving"(FALSE ("Stage Moving")) -> ()
          }
        }
      }
      event "Got ADig bead": Value Change {
        n1076 = event-data() -> ()  [unwired: 1 in, 5 out]
        n1077 = property on="Move Cap. 1 (DNA Top)" class="Bool (strict)"("Val(Sgnl)"=TRUE ("Value (Signaling)")) -> ()  [unwired: 2 in, 2 out]
        n1078 = property on="Inject Bottom" class="Bool (strict)"("Val(Sgnl)"=FALSE ("Value (Signaling)")) -> ()  [unwired: 2 in, 2 out]
      }
      event "Got DNA bead": Value Change {
        n1079 = event-data() -> ()  [unwired: 1 in, 5 out]
        n1080 = property on="Cal/Data Acq. Spot" class="Bool (strict)"("Val(Sgnl)"=TRUE ("Value (Signaling)")) -> ()  [unwired: 2 in, 2 out]
        n1081 = property on="Inject Top" class="Bool (strict)"("Val(Sgnl)"=FALSE ("Value (Signaling)")) -> ()  [unwired: 2 in, 2 out]
      }
      event "Take Stepping Data": Value Change {
        n1082 = event-data() -> ()  [unwired: 1 in, 5 out]
        n1083 = local read "Save ave N"() -> (w1675:dbl)
        n1084 = flat-sequence {
          tunnel: w1675 -> [w1677]
          tunnel: [w1677] -> w1670
          tunnel: [w1679] -> w1671
          tunnel: w1670 -> [w1679]
          tunnel: [w1681] -> w1672
          tunnel: w1671 -> [w1681]
          tunnel: [w1684] -> w1673
          tunnel: w1672 -> [w1684]
          tunnel: [w1686] -> w1674
          tunnel: w1673 -> [w1686]
          tunnel: [w1688] -> w1668
          tunnel: w1674 -> [w1688]
          tunnel: w1668 -> [w1691]
          tunnel: [w1691] -> w1667
          tunnel: w1667 -> [w1692]
          tunnel: [w1692] -> w1669
          tunnel: w1669 -> [w1698]
          frame #0 {
            n1085 = property on="Save ave N" class="DigNum (strict)"("Val(Sgnl)"="Save ave factor") -> ()  [unwired: 2 in, 2 out]
          }
          frame #1 {
            n1086 = Wait (ms)(milliseconds to wait=u32 100) -> ()  [unwired: 1 out]
          }
          frame #2 {
            n1087 = local read "Offset 2 Start (MHz)"() -> (w1683:dbl)
            n1088 = property on="Saved AOD Raster Scan Parameter Sets" class="Arr (strict)"("Index Values"=u32[] [2]) -> ()  [unwired: 2 in, 2 out]
            n1089 = property on="Trap Delta (MHz)" class="DigNum (strict)"("Val(Sgnl)"=w1683) -> ()  [unwired: 2 in, 2 out]
          }
          frame #3 {
            n1090 = property on="Load parameters" class="Bool (strict)"("Val(Sgnl)"=TRUE ("Value (Signaling)")) -> ()  [unwired: 2 in, 2 out]
          }
          frame #4 {
            n1091 = Wait (ms)(milliseconds to wait=u32 100) -> ()  [unwired: 1 out]
          }
          frame #5 {
            n1092 = property on="Trap Raster Scan" class="Bool (strict)"("Val(Sgnl)"=TRUE ("Value (Signaling)")) -> ()  [unwired: 2 in, 2 out]
          }
          frame #6 {
            n1093 = Wait (ms)(milliseconds to wait=u32 1000) -> ()  [unwired: 1 out]
          }
          frame #7 {
            n1094 = while {
              stop <- w1695 stop-if-true
              n1095 = local read "Raster Scanning..."() -> (w1697:bool)
              n1096 = local read "Saving..."() -> (w1696:bool)
              n1097 = Not(x=w1696) -> (.not. x?=w1693:bool)
              n1098 = Not(x=w1697) -> (.not. x?=w1694:bool)
              n1099 = And(x=w1694, y=w1693) -> (x .and. y?=w1695:bool)
            }
          }
          frame #8 {
            n1100 = property on="Save ave N" class="DigNum (strict)"("Val(Sgnl)"=w1698) -> ()  [unwired: 2 in, 2 out]
          }
        }
      }
      event "Step Size (nm)": Value Change {
        n1101 = event-data() -> ()  [unwired: 1 in, 5 out]
        n1102 = flat-sequence {
          frame #0 {
            n1103 = property on="Saved AOD Raster Scan Parameter Sets" class="Arr (strict)"("Index Values"=u32[] [1]) -> ()  [unwired: 2 in, 2 out]
          }
          frame #1 {
            n1104 = Multiply(x="N Steps", y="Step Size (nm)") -> (x*y=w1700:dbl)
            n1105 = property on="Scan Speed AOD (nm/s) 2" class="DigNum (strict)"("Value"="Step Size (nm)") -> ()  [unwired: 2 in, 2 out]
            n1106 = property on="Step Size AOD (nm) 2" class="DigNum (strict)"("Value"="Step Size (nm)") -> ()  [unwired: 2 in, 2 out]
            n1107 = property on="Scan Range AOD (nm) 2" class="DigNum (strict)"("Value"=w1700) -> ()  [unwired: 2 in, 2 out]
          }
        }
      }
      event "Take Detection Laser\nImage": Value Change {
        n1108 = event-data() -> ()  [unwired: 1 in, 5 out]
        n1109 = flat-sequence {
          tunnel: [w1728] -> w1718
          tunnel: [w1727] -> w1711
          tunnel: [w1726] -> w1703
          tunnel: [w1731] -> w1719
          tunnel: w1718 -> [w1731]
          tunnel: [w1730] -> w1712
          tunnel: w1711 -> [w1730]
          tunnel: [w1729] -> w1704
          tunnel: w1703 -> [w1729]
          tunnel: [w1735] -> w1720
          tunnel: w1719 -> [w1735]
          tunnel: [w1734] -> w1713
          tunnel: w1712 -> [w1734]
          tunnel: [w1733] -> w1705
          tunnel: w1704 -> [w1733]
          tunnel: [w1741] -> w1721
          tunnel: w1720 -> [w1741]
          tunnel: [w1740] -> w1714
          tunnel: w1713 -> [w1740]
          tunnel: [w1739] -> w1706
          tunnel: w1705 -> [w1739]
          tunnel: [w1745] -> w1722
          tunnel: w1721 -> [w1745]
          tunnel: [w1744] -> w1715
          tunnel: w1714 -> [w1744]
          tunnel: [w1743] -> w1707
          tunnel: w1706 -> [w1743]
          tunnel: [w1749] -> w1723
          tunnel: w1722 -> [w1749]
          tunnel: [w1748] -> w1716
          tunnel: w1715 -> [w1748]
          tunnel: [w1747] -> w1708
          tunnel: w1707 -> [w1747]
          tunnel: [w1753] -> w1724
          tunnel: w1723 -> [w1753]
          tunnel: [w1752] -> w1717
          tunnel: w1716 -> [w1752]
          tunnel: [w1751] -> w1709
          tunnel: w1708 -> [w1751]
          tunnel: w1724 -> [w1759]
          tunnel: w1717 -> [w1758]
          tunnel: [w1756] -> w1710
          tunnel: w1709 -> [w1756]
          tunnel: w1710 -> [w1760]
          frame #0 {
            n1110 = local read "Green Laser ON/Interlacing"() -> (w1728:bool)
            n1111 = local read "Green laser mode"() -> (w1727:enum32{"Laser ON", "Laser OFF", "Interlace"})
            n1112 = local read "Green FB On/Off"() -> (w1726:bool)
          }
          frame #1 {
            n1113 = property on="Green FB On/Off" class="Bool (strict)"("Val(Sgnl)"=FALSE ("Value (Signaling)")) -> ()  [unwired: 2 in, 2 out]
          }
          frame #2 {
            n1114 = property on="Green Laser ON/Interlacing" class="Bool (strict)"("Val(Sgnl)"=TRUE ("Value (Signaling)")) -> ()  [unwired: 2 in, 2 out]
            n1115 = property on="Flip Green Filter" class="Bool (strict)"("Val(Sgnl)"=TRUE ("Value (Signaling)")) -> ()  [unwired: 2 in, 2 out]
            n1116 = property on="Green laser mode" class="RadioBtnsControl (strict)"("Val(Sgnl)"=enum32{"Laser ON", "Laser OFF", "Interlace"}."Laser ON" ("Value (Signaling)")) -> ()  [unwired: 2 in, 2 out]
          }
          frame #3 {
            n1117 = Wait (ms)(milliseconds to wait=u32 500) -> ()  [unwired: 1 out]
          }
          frame #4 {
            n1118 = property on="Confocal Image" class="Bool (strict)"("Val(Sgnl)"=TRUE ("Value (Signaling)")) -> ()  [unwired: 2 in, 2 out]
          }
          frame #5 {
            n1119 = Wait (ms)(milliseconds to wait=u32 2000) -> ()  [unwired: 1 out]
          }
          frame #6 {
            n1120 = while {
              stop <- w1754 stop-if-true
              n1121 = local read "Saving..."() -> (w1755:bool)
              n1122 = Not(x=w1755) -> (.not. x?=w1754:bool)
            }
          }
          frame #7 {
            n1123 = property on="Flip Green Filter" class="Bool (strict)"("Val(Sgnl)"=TRUE ("Value (Signaling)")) -> ()  [unwired: 2 in, 2 out]
            n1124 = property on="Green Laser ON/Interlacing" class="Bool (strict)"("Val(Sgnl)"=w1759) -> ()  [unwired: 2 in, 2 out]
            n1125 = property on="Green laser mode" class="RadioBtnsControl (strict)"("Val(Sgnl)"=w1758) -> ()  [unwired: 2 in, 2 out]
          }
          frame #8 {
            n1126 = property on="Green FB On/Off" class="Bool (strict)"("Val(Sgnl)"=w1760) -> ()  [unwired: 2 in, 2 out]
          }
        }
      }
      event "Stop All": Value Change {
        n1127 = event-data() -> ()  [unwired: 1 in, 5 out]
        n1128 = local read "Stop All"() -> (w1761:bool)
      }
    }
    n1129 = node-c288() -> ()  [unwired: 1 in, 1 out]
  }
  n1130 = node-c288() -> (w76:T24)  [unwired: 4 out]
  n1131 = timed-loop "Mouse control: trap position (AOM deflection), set confocal spot from image" {
    tunnel: [w1763] -> w34
    tunnel: w24 -> [w1762]
    timing: w76 -> [_]
    timing-out: [_] -> w75
    stop <- w1763 stop-if-true
    n1132 = node-c288() -> ()  [unwired: 2 out]
    n1133 = event shown="[0] \"Pane\": Mouse Down" {
      selector: _ -> [_ _]
      dyn-events: _ -> [_ _]
      timeout: _ -> [_ _]
      tunnel: w1762 -> [w1766 _]
      event Mouse Down {
        n1134 = event-data() -> ("Time"=w1768:u32, "Coords"=w1767:T7, "Button"=w1769:u16)  [unwired: 6 out]
        n1135 = case shown="1" w1769 {
          tunnel: w1768 -> [_ _ w1872]
          tunnel: w1767 -> [_ w1806 w1870]
          tunnel: w1766 -> [_ _ w1868]
          frame 0, Default {
          }
          frame 1 {
            n1136 = property on="APD 2" class="ImageControl"() -> ("Displayed Image Position"=w1776:cluster{"Left":i32, "Top":i32})  [unwired: 2 in, 2 out]
            n1137 = property on="APD 1" class="ImageControl"() -> ("Displayed Image Position"=w1805:cluster{"Left":i32, "Top":i32})  [unwired: 2 in, 2 out]
            n1138 = property on="Detection Laser X" class="ImageControl"() -> ("Displayed Image Position"=w1802:cluster{"Left":i32, "Top":i32})  [unwired: 2 in, 2 out]
            n1139 = property on="Detection Laser Y" class="ImageControl"() -> ("Displayed Image Position"=w1801:cluster{"Left":i32, "Top":i32})  [unwired: 2 in, 2 out]
            n1140 = property on="APD 2" class="ImageControl"() -> ("Displayed Image Size"=w1775:cluster{"Width":u32, "Height":u32})  [unwired: 2 in, 2 out]
            n1141 = property on="APD 1" class="ImageControl"() -> ("Displayed Image Size"=w1803:cluster{"Width":u32, "Height":u32})  [unwired: 2 in, 2 out]
            n1142 = property on="Detection Laser X" class="ImageControl"() -> ("Displayed Image Size"=w1804:cluster{"Width":u32, "Height":u32})  [unwired: 2 in, 2 out]
            n1143 = property on="Detection Laser Y" class="ImageControl"() -> ("Displayed Image Size"=w1800:cluster{"Width":u32, "Height":u32})  [unwired: 2 in, 2 out]
            n1144 = Unbundle By Name(w1775) -> ("Width"=w1772:u32, "Height"=w1771:u32)
            n1145 = Unbundle By Name(w1776) -> ("Left"=w1774:i32, "Top"=w1773:i32)
            n1146 = Unbundle By Name(w1803) -> ("Width"=w1797:u32, "Height"=w1796:u32)
            n1147 = Unbundle By Name(w1804) -> ("Width"=w1793:u32, "Height"=w1792:u32)
            n1148 = Unbundle By Name(w1800) -> ("Width"=w1789:u32, "Height"=w1788:u32)
            n1149 = Unbundle By Name(w1805) -> ("Left"=w1799:i32, "Top"=w1798:i32)
            n1150 = Unbundle By Name(w1802) -> ("Left"=w1795:i32, "Top"=w1794:i32)
            n1151 = Unbundle By Name(w1801) -> ("Left"=w1791:i32, "Top"=w1790:i32)
            n1152 = Bundle("Left"=w1774, "Top"=w1773, "Width"=w1772, "Height"=w1771) -> (w1770:T33)  [unwired: 1 in]
            n1153 = Bundle("Left"=w1799, "Top"=w1798, "Width"=w1797, "Height"=w1796) -> (w1787:T33)  [unwired: 1 in]
            n1154 = Bundle("Left"=w1795, "Top"=w1794, "Width"=w1793, "Height"=w1792) -> (w1786:T33)  [unwired: 1 in]
            n1155 = Bundle("Left"=w1791, "Top"=w1790, "Width"=w1789, "Height"=w1788) -> (w1785:T33)  [unwired: 1 in]
            n1156 = Build Cluster Array(w1770, w1787, w1786, w1785) -> (w1784:T34)
            n1157 = for {
              tunnel: w1806 -> [w1817]
              tunnel: w1784 -> [w1818] mode=indexing
              shift-right: [w1815] -> w1782
              shift-left: TRUE -> [w1816]
              shift-right: [w1814] -> w1780
              shift-left: _ -> [w1810]
              shift-right: [w1813] -> w1779
              shift-left: _ -> [w1809]
              shift-right: [w1812] -> w1778
              shift-left: _ -> [w1808]
              shift-right: [w1811] -> w1777
              shift-left: _ -> [w1807]
              n1158 = case shown="True" w1816 {
                selector: w1816 -> [w1823 _]
                tunnel: w1818 -> [_ w1832]
                tunnel: w1817 -> [_ w1830]
                tunnel: [w1823 w1828] -> w1815
                tunnel: [w1822 w1827] -> w1814
                tunnel: [w1821 w1826] -> w1813
                tunnel: [w1820 w1825] -> w1812
                tunnel: [w1819 w1824] -> w1811
                tunnel: w1810 -> [w1822 _]
                tunnel: w1809 -> [w1821 _]
                tunnel: w1808 -> [w1820 _]
                tunnel: w1807 -> [w1819 _]
                frame False {
                }
                frame True {
                  n1159 = Unbundle(w1832) -> (w1831:T33)
                  n1160 = call "isclickinwindow.vi"("Image Param"=w1831, "Point32"=w1830) -> ("4 Y"=w1824:i32, "3 Height"=w1825:i32, "2 X"=w1826:i32, "1 Width"=w1827:i32, "In image?"=w1829:bool)  [unwired: 1 in]
                  n1161 = Not(x=w1829) -> (.not. x?=w1828:bool)
                }
              }
            }
            n1162 = Not(x=w1782) -> (.not. x?=w1781:bool)
            n1163 = case shown="False" w1781 {
              tunnel: w1779 -> [_ w1845]
              tunnel: w1777 -> [_ w1844]
              tunnel: w1780 -> [_ w1843]
              tunnel: w1778 -> [_ w1842]
              frame False {
              }
              frame True {
                w1838 = FALSE ("Get Point")
                n1164 = local read "Scan lines (y)"() -> (w1847:u64)
                n1165 = local read "Actual MCL Inc (V)"() -> (w1839:dbl)
                n1166 = local read "Scan steps (MCL)"() -> (w1846:u64)
                n1167 = Divide "Y Pix/step"(x=w1842, y=w1847) -> (x/y=w1854:dbl)
                n1168 = Divide "Y V/pix"(x=w1839, y=w1854) -> (x/y=w1853:dbl)
                n1169 = Divide "Y half step offset"(x=w1839, y=2.0) -> (x/y=w1855:dbl)
                n1170 = Divide "X pix/step"(x=w1843, y=w1846) -> (x/y=w1852:dbl)
                n1171 = Negate(x=w1855) -> (-x=w1856:dbl)
                n1172 = local read "Initial Y"() -> (w1862:dbl)
                n1173 = Multiply(x=w1844, y=w1853) -> (x*y=w1863:dbl)
                n1174 = Divide "X half step offset"(x=w1839, y=2.0) -> (x/y=w1849:dbl)
                n1175 = Divide "X V/pix"(x=w1839, y=w1852) -> (x/y=w1851:dbl)
                n1176 = Multiply(x=w1839, y=w1846) -> (x*y=w1858:dbl)
                n1177 = Compound Arithmetic op=ADD(w1856, w1863, w1862) -> (w1840:dbl)
                "Pointer Y (V)" <- w1840
                n1178 = Multiply(x=w1851, y=w1845) -> (x*y=w1860:dbl)
                n1179 = Negate(x=w1849) -> (-x=w1848:dbl)
                n1180 = local read "Initial X"() -> (w1861:dbl)
                n1181 = Negate(x=w1860) -> (-x=w1859:dbl)
                n1182 = Compound Arithmetic op=ADD(w1848, w1858, w1861, w1859) -> (w1841:dbl)
                "Pointer X (V)" <- w1841
                n1183 = Or(x="Set X Only", y="Set Confocal Spot (X-Y)") -> (x .or. y?=w1834:bool)
                n1184 = Or(x="Set Confocal Spot (X-Y)", y="Set Y Only") -> (x .or. y?=w1833:bool)
                n1185 = case shown="True" w1834 {
                  tunnel: w1841 -> [_ w1864]
                  frame False {
                  }
                  frame True {
                    n1186 = property on="AO2" class="Slide (strict)"("Val(Sgnl)"=w1864) -> ()  [unwired: 2 in, 2 out]
                  }
                }
                n1187 = case shown="True" w1833 {
                  tunnel: w1840 -> [_ w1865]
                  frame False {
                  }
                  frame True {
                    n1188 = property on="AO1" class="Slide (strict)"("Val(Sgnl)"=w1865) -> ()  [unwired: 2 in, 2 out]
                  }
                }
                n1189 = local write "Set Confocal Spot (X-Y)"(w1838) -> ()
                n1190 = local write "Set X Only"(w1838) -> ()
                n1191 = local write "Set Y Only"(w1838) -> ()
              }
            }
          }
          frame 3 {
            n1192 = local read "BD 2 Frequency 1 (MHz)"() -> (w1866:dbl)
            n1193 = local read "BD 1 Frequency 1 (MHz)"() -> (w1867:dbl)
            n1194 = local write "Manipulating Trap"(TRUE ("Manipulating Trap")) -> ()
            n1195 = local write "Coords"(T7 {"Horizontal"=0, "Vertical"=0} ("Coords")) -> ()
            n1196 = while {
              tunnel: w1872 -> [w1877]
              tunnel: w1870 -> [w1876]
              tunnel: w1868 -> [w1875]
              tunnel: w1867 -> [w1874]
              tunnel: w1866 -> [w1873]
              stop <- w1878 stop-if-true
              n1197 = event shown="[0] \"Pane\": Mouse Move" {
                selector: _ -> [_ _]
                dyn-events: _ -> [_ _]
                timeout: _ -> [_ _]
                tunnel: ["Force Manip Abort" w1942] -> w1878
                tunnel: w1877 -> [w1885 _]
                tunnel: w1876 -> [w1883 _]
                tunnel: w1875 -> [w1882 _]
                tunnel: w1874 -> [w1881 _]
                tunnel: w1873 -> [w1880 _]
                event Mouse Move {
                  n1198 = event-data() -> ("Time"=w1886:u32, "Coords"=w1887:T7)  [unwired: 3 out]
                  n1199 = Less?(x=w1886, y=w1885) -> (x < y?=w1884:bool)
                  n1200 = case "Makes sure old motion events prior to mouse click aren't used" shown="False" w1884 {
                    tunnel: w1887 -> [w1929 _]
                    tunnel: w1883 -> [w1930 _]
                    tunnel: w1882 -> [w1907 _]
                    tunnel: w1881 -> [w1903 _]
                    tunnel: w1880 -> [w1902 _]
                    frame False {
                      n1201 = Subtract(x=w1929, y=w1930) -> (x-y=w1928:T7)
                      "Coords" <- w1928
                      n1202 = local read "Y RF Frequency Limits (MHz)"() -> (w1888:T16)
                      n1203 = To Double Precision Float(number=w1928) -> (double precision float=w1927:cluster{"Horizontal":dbl, "Vertical":dbl})
                      n1204 = Multiply(x=cluster{"Horizontal":dbl, "Vertical":dbl} {"Horizontal"=-1.0, "Vertical"=1.0}, y="Manipulation Scaling") -> (x*y=w1923:cluster{"Horizontal":dbl, "Vertical":dbl})
                      n1205 = local read "X RF Frequency Limits (MHz)"() -> (w1889:T16)
                      n1206 = Multiply(x=w1927, y=w1923) -> (x*y=w1925:cluster{"Horizontal":dbl, "Vertical":dbl})
                      n1207 = Unbundle By Name(w1925) -> ("Horizontal"=w1920:dbl, "Vertical"=w1924:dbl)
                      n1208 = Unbundle By Name(w1888) -> ("Maximum"=w1891:dbl, "Minimum"=w1890:dbl)
                      n1209 = Boolean To (0,1)(Boolean="Manip. X?") -> (0, 1=w1918:i16)
                      n1210 = Boolean To (0,1)(Boolean="Manip. Y?") -> (0, 1=w1915:i16)
                      n1211 = local read "BD 1 Frequency 2 (MHz)"() -> (w1905:dbl)
                      n1212 = Multiply(x=w1924, y=w1915) -> (x*y=w1917:dbl)
                      n1213 = Multiply(x=w1918, y=w1920) -> (x*y=w1921:dbl)
                      n1214 = local read "BD 2 Frequency 2 (MHz)"() -> (w1904:dbl)
                      n1215 = Unbundle By Name(w1889) -> ("Maximum"=w1893:dbl, "Minimum"=w1892:dbl)
                      n1216 = Add(x=w1902, y=w1917) -> (x+y=w1895:dbl)
                      n1217 = Add(x=w1903, y=w1921) -> (x+y=w1897:dbl)
                      n1218 = In Range and Coerce(upper limit=w1893, x=w1897, lower limit=w1892) -> (coerced(x)=w1896:dbl)  [unwired: 1 out]
                      n1219 = In Range and Coerce(upper limit=w1891, x=w1895, lower limit=w1890) -> (coerced(x)=w1894:dbl)  [unwired: 1 out]
                      n1220 = Subtract(x=w1896, y=w1905) -> (x-y=w1914:dbl)
                      n1221 = Subtract(x=w1894, y=w1904) -> (x-y=w1913:dbl)
                      n1222 = Square(x=w1914) -> (x^2=w1912:dbl)
                      n1223 = Square(x=w1913) -> (x^2=w1911:dbl)
                      n1224 = Add(x=w1912, y=w1911) -> (x+y=w1910:dbl)
                      n1225 = Square Root(x=w1910) -> (sqrt(x)=w1906:dbl)
                      n1226 = In Range and Coerce(upper limit="Limit Max (MHz)", x=w1906, lower limit="Limit Min (MHz)") -> (In Range?=w1899:bool)  [unwired: 1 out]
                      n1227 = Not(x="Limits Enable") -> (.not. x?=w1898:bool)
                      n1228 = Or(x=w1899, y=w1898) -> (x .or. y?=w1900:bool)
                      n1229 = case shown="True" w1900 {
                        tunnel: w1907 -> [_ w1940]
                        tunnel: w1906 -> [_ w1931]
                        tunnel: w1896 -> [_ w1938]
                        tunnel: w1905 -> [_ w1937]
                        tunnel: w1894 -> [_ w1936]
                        tunnel: w1904 -> [_ w1935]
                        tunnel: w1889 -> [_ w1933]
                        tunnel: w1888 -> [_ w1932]
                        frame False {
                        }
                        frame True {
                          n1230 = local read "BD 1 Frequency 3 (MHz)"() -> (w1939:dbl)
                          n1231 = local read "BD 2 Frequency 3 (MHz)"() -> (w1934:dbl)
                          n1232 = local write "Trap Delta (MHz)"(w1931) -> ()
                          n1233 = property on="Initial delta (MHz)" class="DigNum (strict)"("Val(Sgnl)"=w1931) -> ()  [unwired: 2 in, 2 out]
                          n1234 = call "set RF board frequency - interlace.vi"("Board 2 Frequency Limits"=w1932, "Board 1 Frequency Limits"=w1933, "FPGA VI Reference In"=w1940, "Board 2 Frequency 3 (MHz)"=w1934, "Board 1 Frequency 3 (MHz)"=w1939, "Board 2 Frequency 2 (MHz)"=w1935, "Board 2 Frequency 1 (MHz)"=w1936, "Board 1 Frequency 2 (MHz)"=w1937, "Board 1 Frequency 1  (MHz)"=w1938) -> ()  [unwired: 1 in, 2 out]
                          n1235 = local write "BD 2 Frequency 1 (MHz)"(w1936) -> ()
                          n1236 = local write "BD 1 Frequency 1 (MHz)"(w1938) -> ()
                        }
                      }
                    }
                    frame True {
                    }
                  }
                }
                event Mouse Up {
                  n1237 = event-data() -> ("Button"=w1941:u16)  [unwired: 8 out]
                  n1238 = case shown="3" w1941 {
                    tunnel: [FALSE TRUE] -> w1942
                    frame 0, Default {
                    }
                    frame 3 {
                      n1239 = local write "Manipulating Trap"(FALSE ("Manipulating Trap")) -> ()
                    }
                  }
                }
              }
            }
          }
        }
      }
      event Mouse Move {
        n1240 = event-data() -> ()  [unwired: 6 out]
      }
    }
    n1241 = local read "Stop All"() -> (w1763:bool)
    n1242 = node-c288() -> ()  [unwired: 2 out]
  }
  n1243 = node-c288(w68) -> ()  [unwired: 1 out]
  n1244 = node-c288(w75) -> ()  [unwired: 1 out]
  n1245 = node-c288(w14) -> ()  [unwired: 1 out]
  n1246 = node-c288(i64 1 ("Period"), 1 ("Processor")) -> (w164:T24)  [unwired: 2 out]
  n1247 = timed-loop "Acquire Data" {
    tunnel: w24 -> [w2200]
    tunnel: w40 -> [w2199]
    tunnel: [w2230] -> w33
    tunnel: [w2224] -> w32
    timing: w164 -> [_]
    timing-out: [_] -> w163
    tunnel: w59 -> [w2028]
    stop <- "Stop All" stop-if-true
    (unwired) u32 0 ("Number of Elements")
    w2015 = "NI_ChannelName" ("name")
    n1248 = node-c288() -> ()  [unwired: 2 out]
    n1249 = First Call?() -> (First Call?: T/F=w1981:bool)
    n1250 = Or(x="Reset", y=w1981) -> (x .or. y?=w1982:bool)
    n1251 = case "Reset data stream" shown="True" w1982 {
      tunnel: w2200 -> [w2246 w2254]
      tunnel: w2199 -> [w2245 w2253]
      tunnel: [w2246 w2248] -> w2195
      tunnel: [w2245 w2247] -> w2194
      frame False {
      }
      frame True {
        w2251 = TRUE ("AI to FIFO")
        n1252 = local write "Overflow (data lost)"(FALSE ("Overflow (data lost)")) -> ()
        n1253 = call "reset FPGA DMA.vi"("error in"=w2253, "FPGA VI Reference In"=w2254) -> ("error out"=w2249:errorcluster, "FPGA VI Reference Out"=w2250:T19)
        n1254 = xnode "Read/Write Control"("FPGA VI Reference In"=w2250, "error in"=w2249, "AI to FIFO"=w2251, "APD to FIFO"=w2251) -> ("FPGA VI Reference Out"=w2248:T19, "error out"=w2247:errorcluster)
      }
    }
    n1255 = Or(x="Start AOD Scan", y="Trap Raster Scan") -> (x .or. y?=w2145:bool)
    n1256 = case "Start AOM raster scan" shown="True" w2145 {
      tunnel: w2195 -> [w2983 w2993]
      tunnel: w2194 -> [w2982 w2992]
      tunnel: [w2983 w2986] -> w2193
      tunnel: [w2982 w2985] -> w2192
      frame False {
      }
      frame True {
        n1257 = case shown="True" "Restart DMA? (AOD)" {
          tunnel: [w3031 w3033] -> w2987
          tunnel: [w3030 w3032] -> w2988
          tunnel: w2993 -> [w3031 w3035]
          tunnel: w2992 -> [w3030 w3034]
          frame False {
          }
          frame True {
            n1258 = local write "Overflow (data lost)"(FALSE ("Overflow (data lost)")) -> ()
            n1259 = call "reset FPGA DMA.vi"("error in"=w3034, "FPGA VI Reference In"=w3035) -> ("error out"=w3032:errorcluster, "FPGA VI Reference Out"=w3033:T19)
          }
        }
        n1260 = local write "Trap Raster Scan"(FALSE ("Trap Raster Scan")) -> ()
        n1261 = case shown="False" "Move MCL Also?" {
          tunnel: w2988 -> [w2996 w3025]
          tunnel: w2987 -> [w2997 w3026]
          tunnel: [w2995 w3029] -> w2986
          tunnel: [w2994 w3028] -> w2985
          frame False {
            w2998 = TRUE ("AI to FIFO")
            n1262 = xnode "Read/Write Control"("FPGA VI Reference In"=w2997, "error in"=w2996, "AI to FIFO"=w2998, "APD to FIFO"=w2998, "Start scan"=w2998) -> ("FPGA VI Reference Out"=w2995:T19, "error out"=w2994:errorcluster)
          }
          frame True {
            w3022 = FALSE ("1D or 2D Scan?")
            w3027 = TRUE ("AI to FIFO")
            # "Count for MCL loop"
            # "N total cycles"
            # "N steps"
            # "V_int"
            n1263 = local read "Scan Range (nm)"() -> (w3004:dbl)
            n1264 = local read "Number of F/B Scans (AOD)"() -> (w3021:u16)
            n1265 = Sign(1:w3004) -> (0:w3003:dbl)
            n1266 = Compound Arithmetic op=MULTIPLY(w3004, "MCL Step Position Ratio", "MCL/AOM Scale Tweak") -> (w3008:dbl)
            n1267 = Negate(x=w3003) -> (-x=w3000:dbl)
            n1268 = Multiply(x=w3000, y="MCL Step Increment (V_int)") -> (x*y=w3002:dbl)
            n1269 = Divide(x=w3008, y="MCL X Cal (nm/V)") -> (x/y=w3014:dbl)
            n1270 = Multiply(x=32767.0 ("y"), y=w3014) -> (x*y=w3020:dbl)
            n1271 = local read "Total Counts (ticks)"() -> (w3005:u32)
            n1272 = local read "Cycles/step (AOD)"() -> (w3016:u64)
            n1273 = local read "Scan steps (AOD)"() -> (w3017:u64)
            n1274 = Divide(x=w3020, y=10.0) -> (x/y=w3013:dbl)
            n1275 = Divide(x=w3013, y="MCL Step Increment (V_int)") -> (x/y=w3011:dbl)
            n1276 = Absolute Value(x=w3011) -> (abs(x)=w2999:dbl)
            n1277 = Compound Arithmetic op=MULTIPLY(w3017, w3016, w3005) -> (w3012:u64)
            n1278 = local write "wait to reset values"(w3027) -> ()
            n1279 = local write "MCL Scanning"(w3027) -> ()
            n1280 = Divide(x=w3012, y=w2999) -> (x/y=w3009:dbl)
            "MCL Count" <- w3009
            n1281 = xnode "Read/Write Control"("FPGA VI Reference In"=w3026, "error in"=w3025, "Scan steps (MCL)"=w2999, "Number of scans (MCL)"=w3021, "Cycles per step (MCL)"=u64 1, "Scan freq.  increment (MCL)"=w3002, "1D or 2D Scan?"=w3022, "MCL Scan Axis"=w3022, "Cont. Scan (MCL)"=w3022, "MCL count"=w3009) -> ("FPGA VI Reference Out"=w3024:T19, "error out"=w3023:errorcluster)
            n1282 = xnode "Read/Write Control"("FPGA VI Reference In"=w3024, "error in"=w3023, "AI to FIFO"=w3027, "APD to FIFO"=w3027, "Start scan"=w3027, "Start scan (MCL)"=w3027) -> ("FPGA VI Reference Out"=w3029:T19, "error out"=w3028:errorcluster)
          }
        }
        "Raster Scanning..." <- TRUE ("Scanning...")
      }
    }
    n1283 = And(x="Save scans", y=w2145) -> (x .and. y?=w2191:bool)
    n1284 = Compound Arithmetic op=OR("Start MCL Scan", "Confocal Image", "Confocal Linescan") -> (w2143:bool)
    n1285 = And(x="Save Data (MCL)", y=w2143) -> (x .and. y?=w2190:bool)
    n1286 = case "Start MCL raster scan" shown="True" w2143 {
      tunnel: w2193 -> [w2537 w2552]
      tunnel: w2192 -> [w2536 w2551]
      tunnel: [w2537 w2547] -> w1950
      tunnel: [w2536 w2546] -> w1949
      tunnel: [FALSE w2545] -> w2176
      tunnel: "Start MCL Scan" -> [_ w2540]
      tunnel: "Confocal Image" -> [_ w2539]
      tunnel: "Confocal Linescan" -> [_ _]
      frame False {
      }
      frame True {
        w2545 = TRUE
        n1287 = case shown="True" "Restart DMA? (MCL)" {
          tunnel: [w2597 w2599] -> w2550
          tunnel: [w2596 w2598] -> w2549
          tunnel: w2552 -> [w2597 w2602]
          tunnel: w2551 -> [w2596 w2601]
          frame False {
          }
          frame True {
            n1288 = call "reset FPGA DMA.vi"("error in"=w2601, "FPGA VI Reference In"=w2602) -> ("error out"=w2598:errorcluster, "FPGA VI Reference Out"=w2599:T19)
            n1289 = local write "Overflow (data lost)"(FALSE ("Overflow (data lost)")) -> ()
          }
        }
        n1290 = case shown="False" w2540 {
          selector: w2540 -> [_ w2556]
          tunnel: w2539 -> [w2555 _]
          tunnel: [w2555 w2556] -> w2538
          frame False {
            n1291 = property on="2D or 1D Scan" class="Bool (strict)"("Val(Sgnl)"=w2555) -> ()  [unwired: 2 in, 2 out]
            n1292 = property on="Confocal Image" class="Bool (strict)"("Value"=FALSE ("Start Confocal Map")) -> ()  [unwired: 2 in, 2 out]
          }
          frame True {
          }
        }
        n1293 = local write "MCL Scanning"(w2545) -> ()
        n1294 = local read "AO1"() -> (w2542:dbl)
        n1295 = local read "AO2"() -> (w2541:dbl)
        n1296 = case shown="True" "Center Scan" {
          tunnel: w2550 -> [w2563 w2595]
          tunnel: w2549 -> [w2562 w2594]
          tunnel: [w2561 w2593] -> w2547
          tunnel: [w2560 w2592] -> w2546
          tunnel: [w2558 w2579] -> w2544
          tunnel: [w2557 w2578] -> w2543
          tunnel: w2542 -> [w2558 w2584]
          tunnel: w2541 -> [w2557 w2587]
          tunnel: w2538 -> [_ _]
          frame False {
            w2559 = TRUE ("AI to FIFO")
            n1297 = xnode "Read/Write Control"("FPGA VI Reference In"=w2563, "error in"=w2562, "AI to FIFO"=w2559, "APD to FIFO"=w2559, "Start scan (MCL)"=w2559) -> ("FPGA VI Reference Out"=w2561:T19, "error out"=w2560:errorcluster)
          }
          frame True {
            w2591 = TRUE ("AI to FIFO")
            n1298 = local read "Scan steps (MCL)"() -> (w2570:u64)
            n1299 = local read "Scan lines (y)"() -> (w2566:u64)
            n1300 = local read "Fast Scan Dir"() -> (w2577:bool)
            n1301 = local read "Actual MCL Inc (V)"() -> (w2567:dbl)
            n1302 = Decrement(x=w2566) -> (x-1=w2565:u64)
            n1303 = Decrement(x=w2570) -> (x-1=w2569:u64)
            n1304 = Multiply(x=w2567, y=w2565) -> (x*y=w2564:dbl)
            n1305 = Divide(x=w2564, y=2.0) -> (x/y=w2574:dbl)
            n1306 = Multiply(x=w2567, y=w2569) -> (x*y=w2568:dbl)
            n1307 = Divide(x=w2568, y=2.0) -> (x/y=w2573:dbl)
            n1308 = Select(t=w2573, s=w2577, f=w2574) -> (s? t:f=w2572:dbl)
            n1309 = Select(t=w2574, s=w2577, f=w2573) -> (s? t:f=w2576:dbl)
            n1310 = Subtract(x=w2584, y=w2576) -> (x-y=w2575:dbl)
            n1311 = Subtract(x=w2587, y=w2572) -> (x-y=w2571:dbl)
            n1312 = local read "2D or 1D Scan"() -> (w2589:bool)
            n1313 = Not(x=w2577) -> (.not. x?=w2583:bool)
            n1314 = Not(x=w2589) -> (.not. x?=w2585:bool)
            n1315 = And(x=w2577, y=w2585) -> (x .and. y?=w2586:bool)
            n1316 = And(x=w2585, y=w2583) -> (x .and. y?=w2588:bool)
            n1317 = Select(t=w2587, s=w2588, f=w2571) -> (s? t:f=w2578:dbl)
            n1318 = Select(t=w2584, s=w2586, f=w2575) -> (s? t:f=w2579:dbl)
            n1319 = call "Volt to I16.vi"("Voltage In"=w2579) -> ("I16 Voltage Out"=w2582:i16)
            n1320 = call "Volt to I16.vi"("Voltage In"=w2578) -> ("I16 Voltage Out"=w2581:i16)
            n1321 = xnode "Read/Write Control"("FPGA VI Reference In"=w2595, "error in"=w2594, "AI to FIFO"=w2591, "APD to FIFO"=w2591, "Start scan (MCL)"=w2591, "AO1"=w2582, "AO2"=w2581) -> ("FPGA VI Reference Out"=w2593:T19, "error out"=w2592:errorcluster)
          }
        }
        "Initial Y" <- w2544
        "Initial X" <- w2543
        "wait to reset values" <- w2545
      }
    }
    n1322 = local read "Trap Pos Elements/DMA read"() -> (w2024:u32)
    n1323 = local read "Trap AI Elements/DMA read"() -> (w1948:u32)
    n1324 = local read "APD Elements/DMA read"() -> (w2067:u32)
    n1325 = local read "Trap AI FIFO Depth"() -> (w2240:u32)
    n1326 = xnode "Invoke Method"("FPGA VI Reference In"=w1950, "error in"=w1949, "Number of Elements"=w2024, "Timeout (ms)"=-1) -> ("Data"=w1988:u16[], "Elements Remaining"=→"Trap Pos FIFO El Remaining":u32)  [unwired: 2 out]
    n1327 = xnode "Invoke Method"("FPGA VI Reference In"=w1950, "error in"=w1949, "Number of Elements"=w1948, "Timeout (ms)"=-1 ("Timeout")) -> ("FPGA VI Reference Out"=w1952:T19, "error out"=w1951:errorcluster, "Data"=w1947:i16[], "Elements Remaining"=w1953:u32)
    "Trap AI FIFO El. Rem." <- w1953
    n1328 = xnode "Get APD Data"("FPGA VI Reference In"=w1950, "error in"=w1949, "Number of Elements"=w2067, "Timeout (ms)"=-1) -> ("Data"=w2066:u32[], "Elements Remaining"=→"APD FIFO Elements Remaining":u32)  [unwired: 2 out]
    n1329 = Subtract(x=w2240, y=w1948) -> (x-y=w2239:u32)
    n1330 = Decimate 1D Array(w1988) -> (w1985:u16[], w1987:u16[], w1986:u16[])
    n1331 = Divide(x=w1953, y=w2239) -> (x/y=w2238:dbl)
    "Buffer Status" <- w2238
    n1332 = To Unsigned Long Integer(number=w1985) -> (unsigned 32bit integer=w1984:u32[])
    n1333 = Join Numbers(hi=w1987, lo=w1986) -> ((hi.lo)=w1983:u32[])
    n1334 = Equal?(x=w2238, y=1.0) -> (x = y?=w2236:bool)
    n1335 = Join Numbers(hi=w1984, lo=w1983) -> ((hi.lo)=w1977:u64[])
    n1336 = call "IR AOM word to freq - vec.vi"("Frequency Word In (double vec)"=w1977) -> ("Frequency Out"=w2023:dbl[])
    n1337 = case "Alert buffer overflow" shown="False" w2236 {
      frame False {
      }
      frame True {
        n1338 = call <vilib>:"Beep.vi"() -> ()  [unwired: 3 in, 9 out]
        "Overflow (data lost)" <- TRUE ("Overflow (data lost)")
      }
    }
    n1339 = Decimate 1D Array(w2023) -> (w2022:dbl[], w2021:dbl[])
    n1340 = Array Size(array=w1947) -> (size(s)=→"Waveform Chart":i32)
    n1341 = Build Array(w2022, w2021) -> (w2020:dbl[][])
    n1342 = local read "Trap Sets"() -> (w2104:u32)
    n1343 = case "Deinterlace trap data, average down PSD" shown="2" w2104 {
      tunnel: w1947 -> [w2632 w2697]
      tunnel: [w2629 w2694] -> w2097
      tunnel: [w2632 w2696] -> w1980
      tunnel: "Detector Type" -> [w2631 w2692]
      tunnel: [w2630 w2695] -> w2096
      tunnel: [w2628 w2693] -> w2211
      frame 1, Default {
        n1344 = Divide(x=w2632, y=3276.7) -> (x/y=w2633:dbl[])
        n1345 = Decimate 1D Array(w2633) -> (w2642:dbl[], w2641:dbl[], w2640:dbl[], w2639:dbl[], w2638:dbl[], w2637:dbl[], w2636:dbl[], w2635:dbl[])
        n1346 = case shown="\"IR-QPD + PSD + FB-QPD position\"" w2631 {
          tunnel: w2642 -> [w2666 w2691]
          tunnel: w2641 -> [w2665 w2690]
          tunnel: w2640 -> [w2650 w2668]
          tunnel: w2639 -> [w2651 w2678]
          tunnel: w2638 -> [w2664 w2689]
          tunnel: w2637 -> [w2663 w2688]
          tunnel: w2636 -> [w2647 w2669]
          tunnel: w2635 -> [w2646 w2667]
          tunnel: [w2645 w2675] -> w2630
          tunnel: [w2644 w2674] -> w2629
          tunnel: [w2643 w2673] -> w2628
          frame "IR-QPD + PSD + FB-QPD", Default {
            w2643 = 0  # Channel pattern
            n1347 = Divide(x=w2666, y=w2651) -> (x/y=w2653:dbl[])
            n1348 = Divide(x=w2665, y=w2651) -> (x/y=w2652:dbl[])
            n1349 = Divide(x=w2664, y=w2647) -> (x/y=w2649:dbl[])
            n1350 = Divide(x=w2663, y=w2646) -> (x/y=w2648:dbl[])
            n1351 = Build Array(w2653, w2652, w2651, w2650, w2649, w2648, w2647, w2646) -> (w2644:dbl[][])
            n1352 = Bundle("T1 Y", "T1 X", "T1 Sum", "FB Sum", "PSD Y", "PSD X", "PSD Y Sum", "PSD X Sum") -> (w2662:T41)  [unwired: 1 out]
            n1353 = Cluster To Array(cluster=w2662) -> (array=w2645:string[])
          }
          frame "IR-QPD + PSD + FB-QPD position" {
            w2673 = 3  # Channel pattern
            n1354 = Negate(x=w2669) -> (-x=w2670:dbl[])
            n1355 = Divide(x=w2691, y=w2678) -> (x/y=w2680:dbl[])
            n1356 = Divide(x=w2690, y=w2678) -> (x/y=w2679:dbl[])
            n1357 = Divide(x=w2689, y=w2669) -> (x/y=w2677:dbl[])
            n1358 = Divide(x=w2688, y=w2670) -> (x/y=w2676:dbl[])
            n1359 = Build Array(w2680, w2679, w2678, w2667, w2668, w2677, w2676, w2669) -> (w2674:dbl[][])
            n1360 = Bundle("T1 Y", "T1 X", "T1 Sum", "FB X", "FB Sum", "PSD Y", "PSD X", "PSD Y Sum") -> (w2687:T41)  [unwired: 1 out]
            n1361 = Cluster To Array(cluster=w2687) -> (array=w2675:string[])
          }
        }
      }
      frame 2 {
        n1362 = case shown="\"UCB Fleezers 052511\"" w2692 {
          tunnel: w2697 -> [w2759 w2826 w2854 w2961]
          tunnel: [w2698 w2818 w2849 w2892] -> w2696
          tunnel: [w2725 w2809 w2851 w2939] -> w2695
          tunnel: [w2724 w2773 w2828 w2906] -> w2694
          tunnel: [w2718 w2808 w2891 w2937] -> w2693
          frame "IR-QPD + PSD + FB-QPD", Default {
            w2718 = 1  # Channel pattern
            # "time average x2 the 4th signal and the 4 psd signals (detection laser)"
            # "deinterlace 3 signals from qpd"
            n1363 = Decimate 1D Array(w2759) -> (w2758:i16[], w2757:i16[], w2723:i16[], w2756:i16[], w2746:i16[], w2744:i16[], w2743:i16[], w2741:i16[])
            n1364 = call "downsample 1D array - double.vi"("Ave N"=2.0, "Array In"=w2746) -> ("Array Out"=w2745:dbl[])  [unwired: 1 out]
            n1365 = call "downsample 1D array - double.vi"("Ave N"=2.0, "Array In"=w2741) -> ("Array Out"=w2740:dbl[])  [unwired: 1 out]
            n1366 = call "downsample 1D array - double.vi"("Ave N"=2.0, "Array In"=w2743) -> ("Array Out"=w2742:dbl[])  [unwired: 1 out]
            n1367 = call "downsample 1D array - double.vi"("Ave N"=2.0, "Array In"=w2744) -> ("Array Out"=w2726:dbl[])  [unwired: 1 out]
            n1368 = Decimate 1D Array(w2758) -> (w2755:i16[], w2727:i16[])
            n1369 = Decimate 1D Array(w2757) -> (w2754:i16[], w2752:i16[])
            n1370 = Decimate 1D Array(w2756) -> (w2753:i16[], w2751:i16[])
            n1371 = Decimate 1D Array(w2723) -> (w2722:i16[], w2721:i16[])
            n1372 = Interleave 1D Arrays(w2755, w2754, w2753, w2727, w2752, w2751, w2722, w2721, w2745, w2726, w2742, w2740) -> (w2739:dbl[])
            n1373 = To Word Integer(number=w2739) -> (16bit integer=w2698:i16[])
            n1374 = Divide(x=w2739, y=3276.7) -> (x/y=w2738:dbl[])
            n1375 = Decimate 1D Array(w2738) -> (w2737:dbl[], w2736:dbl[], w2735:dbl[], w2734:dbl[], w2733:dbl[], w2732:dbl[], w2720:dbl[], w2719:dbl[], w2731:dbl[], w2730:dbl[], w2729:dbl[], w2728:dbl[])
            n1376 = Divide(x=w2737, y=w2735) -> (x/y=w2705:dbl[])
            n1377 = Divide(x=w2736, y=w2735) -> (x/y=w2704:dbl[])
            n1378 = Divide(x=w2734, y=w2732) -> (x/y=w2703:dbl[])
            n1379 = Divide(x=w2733, y=w2732) -> (x/y=w2702:dbl[])
            n1380 = Divide(x=w2731, y=w2729) -> (x/y=w2701:dbl[])
            n1381 = Divide(x=w2730, y=w2728) -> (x/y=w2700:dbl[])
            n1382 = Bundle("T1 Y", "T1 X", "T1 Sum", "T2 Y", "T2 X", "T2 Sum", "T1 FB Sum", "T2 FB Sum", "PSD Y", "PSD X", "PSD Y Sum", "PSD X Sum") -> (w2706:T42)  [unwired: 1 out]
            n1383 = Build Array(w2705, w2704, w2735, w2703, w2702, w2732, w2720, w2719, w2701, w2700, w2729, w2728) -> (w2724:dbl[][])
            n1384 = Cluster To Array(cluster=w2706) -> (array=w2725:string[])
          }
          frame "IR-QPD + PSD + FB-QPD X position" {
            w2808 = 2  # Channel pattern
            # "convert\nADC numbers\nto volts"
            # "time average x2 the 3 psd signals (detection laser)"
            # "deinterlace 3 signals from qpds"
            n1385 = Decimate 1D Array(w2826) -> (w2825:i16[], w2824:i16[], w2761:i16[], w2762:i16[], w2771:i16[], w2768:i16[], w2765:i16[], w2796:i16[])
            n1386 = Decimate 1D Array(w2825) -> (w2823:i16[], w2810:i16[])
            n1387 = call "downsample 1D array - I16.vi"("Ave N"=2.0, "Array In"=w2771) -> ("Array Out"=w2769:i16[])  [unwired: 1 in]
            n1388 = call "downsample 1D array - I16.vi"("Ave N"=2.0, "Array In"=w2768) -> ("Array Out"=w2766:i16[])  [unwired: 1 in]
            n1389 = Decimate 1D Array(w2824) -> (w2822:i16[], w2820:i16[])
            n1390 = Decimate 1D Array(w2762) -> (w2821:i16[], w2819:i16[])
            n1391 = Decimate 1D Array(w2796) -> (w2795:i16[], w2793:i16[])
            n1392 = Decimate 1D Array(w2761) -> (w2794:i16[], w2792:i16[])
            n1393 = call "downsample 1D array - I16.vi"("Ave N"=2.0, "Array In"=w2765) -> ("Array Out"=w2763:i16[])  [unwired: 1 in]
            n1394 = Interleave 1D Arrays(w2823, w2822, w2821, w2810, w2820, w2819, w2795, w2794, w2793, w2792, w2769, w2766, w2763) -> (w2818:i16[])
            n1395 = Divide(x=w2818, y=3276.7) -> (x/y=w2817:dbl[])
            n1396 = Decimate 1D Array(w2817) -> (w2816:dbl[], w2815:dbl[], w2814:dbl[], w2813:dbl[], w2812:dbl[], w2811:dbl[], w2784:dbl[], w2782:dbl[], w2781:dbl[], w2779:dbl[], w2778:dbl[], w2777:dbl[], w2774:dbl[])
            n1397 = Divide(x=w2816, y=w2814) -> (x/y=w2800:dbl[])
            n1398 = Divide(x=w2815, y=w2814) -> (x/y=w2799:dbl[])
            n1399 = Divide(x=w2813, y=w2811) -> (x/y=w2798:dbl[])
            n1400 = Divide(x=w2812, y=w2811) -> (x/y=w2797:dbl[])
            n1401 = Divide(x=w2784, y=w2782) -> (x/y=w2783:dbl[])
            n1402 = Divide(x=w2781, y=w2779) -> (x/y=w2780:dbl[])
            n1403 = Divide(x=w2778, y=w2774) -> (x/y=w2776:dbl[])
            n1404 = Negate(x=w2774) -> (-x=w2772:dbl[])
            n1405 = Divide(x=w2777, y=w2772) -> (x/y=w2775:dbl[])
            n1406 = Bundle("T1 Y", "T1 X", "T1 Sum", "T2 Y", "T2 X", "T2 Sum", "T1 FB X", "T1 FB Sum", "T2 FB X", "T2 FB Sum", "PSD Y", "PSD X", "PSD Y Sum") -> (w2801:T43)  [unwired: 1 out]
            n1407 = Build Array(w2800, w2799, w2814, w2798, w2797, w2811, w2783, w2782, w2780, w2779, w2776, w2775, w2774) -> (w2773:dbl[][])
            n1408 = Cluster To Array(cluster=w2801) -> (array=w2809:string[])
          }
          frame "UCB Fleezers 052511" {
            w2891 = 2  # Channel pattern
            n1409 = Decimate 1D Array(w2854) -> (w2889:i16[], w2888:i16[], w2853:i16[], w2852:i16[], w2846:i16[], w2843:i16[], w2842:i16[], w2841:i16[])
            n1410 = Decimate 1D Array(w2889) -> (w2887:i16[], w2872:i16[])
            n1411 = Decimate 1D Array(w2888) -> (w2886:i16[], w2884:i16[])
            n1412 = Decimate 1D Array(w2853) -> (w2885:i16[], w2883:i16[])
            n1413 = Decimate 1D Array(w2852) -> (w2848:i16[], w2847:i16[])
            n1414 = Decimate 1D Array(w2846) -> (w2845:i16[], w2844:i16[])
            n1415 = call "downsample 1D array - I16.vi"("Ave N"=2.0, "Array In"=w2843) -> ("Array Out"=w2840:i16[])  [unwired: 1 in]
            n1416 = call "downsample 1D array - I16.vi"("Ave N"=2.0, "Array In"=w2842) -> ("Array Out"=w2839:i16[])  [unwired: 1 in]
            n1417 = call "downsample 1D array - I16.vi"("Ave N"=2.0, "Array In"=w2841) -> ("Array Out"=w2838:i16[])  [unwired: 1 in]
            n1418 = Interleave 1D Arrays(w2887, w2886, w2885, w2872, w2884, w2883, w2848, w2845, w2847, w2844, w2840, w2839, w2838) -> (w2849:i16[])
            n1419 = Divide(x=w2849, y=3276.7) -> (x/y=w2879:dbl[])
            n1420 = Decimate 1D Array(w2879) -> (w2878:dbl[], w2877:dbl[], w2876:dbl[], w2875:dbl[], w2874:dbl[], w2873:dbl[], w2837:dbl[], w2835:dbl[], w2834:dbl[], w2832:dbl[], w2831:dbl[], w2830:dbl[], w2829:dbl[])
            n1421 = Divide(x=w2878, y=w2876) -> (x/y=w2859:dbl[])
            n1422 = Divide(x=w2877, y=w2876) -> (x/y=w2858:dbl[])
            n1423 = Divide(x=w2875, y=w2873) -> (x/y=w2857:dbl[])
            n1424 = Divide(x=w2874, y=w2873) -> (x/y=w2856:dbl[])
            n1425 = Divide(x=w2837, y=w2835) -> (x/y=w2836:dbl[])
            n1426 = Divide(x=w2834, y=w2832) -> (x/y=w2833:dbl[])
            n1427 = Bundle("T1 Y", "T1 X", "T1 Sum", "T2 Y", "T2 X", "T2 Sum", "T1 FB X", "T2 FB Sum", "T2 FB X", "T2 FB Sum", "PSD Y", "PSD X", "PSD Sum") -> (w2860:T43)  [unwired: 1 out]
            n1428 = Build Array(w2859, w2858, w2876, w2857, w2856, w2873, w2836, w2835, w2833, w2832, w2831, w2830, w2829) -> (w2828:dbl[][])
            n1429 = Cluster To Array(cluster=w2860) -> (array=w2851:string[])
          }
          frame "IR-QPD + PSD + FB-QPD XY positions" {
            w2937 = 4  # Channel pattern
            # "time average x2 the 3 psd signals (detection laser)"
            # "deinterlace 3 signals from qpds"
            n1430 = Decimate 1D Array(w2961) -> (w2960:i16[], w2959:i16[], w2938:i16[], w2958:i16[], w2904:i16[], w2950:i16[], w2949:i16[], w2926:i16[])
            n1431 = Decimate 1D Array "QPD Y"(w2960) -> (w2957:i16[], w2940:i16[])
            n1432 = call "downsample 1D array - double.vi"("Ave N"=2.0, "Array In"=w2950) -> ("Array Out"=w2925:dbl[])  [unwired: 1 out]
            n1433 = call "downsample 1D array - double.vi"("Ave N"=2.0, "Array In"=w2949) -> ("Array Out"=w2924:dbl[])  [unwired: 1 out]
            n1434 = Decimate 1D Array "Feedback Sum"(w2938) -> (w2922:i16[], w2920:i16[])
            n1435 = Decimate 1D Array "Feedback Y"(w2904) -> (w2903:i16[], w2902:i16[])
            n1436 = Decimate 1D Array "Feedback X"(w2926) -> (w2923:i16[], w2921:i16[])
            n1437 = Decimate 1D Array "QPD Sum"(w2958) -> (w2955:i16[], w2953:i16[])
            n1438 = Decimate 1D Array "QPD X"(w2959) -> (w2956:i16[], w2954:i16[])
            n1439 = Interleave 1D Arrays(w2957, w2956, w2955, w2940, w2954, w2953, w2903, w2923, w2922, w2902, w2921, w2920, w2925, w2924) -> (w2948:dbl[])
            n1440 = To Word Integer(number=w2948) -> (16bit integer=w2892:i16[])
            n1441 = Divide(x=w2948, y=3276.7) -> (x/y=w2947:dbl[])
            n1442 = Decimate 1D Array(w2947) -> (w2946:dbl[], w2945:dbl[], w2944:dbl[], w2943:dbl[], w2942:dbl[], w2941:dbl[], w2899:dbl[], w2913:dbl[], w2897:dbl[], w2898:dbl[], w2911:dbl[], w2895:dbl[], w2909:dbl[], w2907:dbl[])
            n1443 = Divide(x=w2946, y=w2944) -> (x/y=w2930:dbl[])
            n1444 = Divide(x=w2945, y=w2944) -> (x/y=w2929:dbl[])
            n1445 = Divide(x=w2943, y=w2941) -> (x/y=w2928:dbl[])
            n1446 = Divide(x=w2942, y=w2941) -> (x/y=w2927:dbl[])
            n1447 = Divide(x=w2899, y=w2897) -> (x/y=w2896:dbl[])
            n1448 = Divide(x=w2913, y=w2897) -> (x/y=w2912:dbl[])
            n1449 = Divide(x=w2898, y=w2895) -> (x/y=w2894:dbl[])
            n1450 = Divide(x=w2911, y=w2895) -> (x/y=w2910:dbl[])
            n1451 = Negate(x=w2907) -> (-x=w2905:dbl[])
            n1452 = Divide(x=w2909, y=w2905) -> (x/y=w2908:dbl[])
            n1453 = Bundle("T1 Y", "T1 X", "T1 Sum", "T2 Y", "T2 X", "T2 Sum", "T1 FB Y", "T1 FB X", "T1 FB Sum", "T2 FB Y", "T2 FB X", "T2 FB Sum", "PSD X", "PSD Y Sum") -> (w2893:T44)  [unwired: 1 out]
            n1454 = Build Array(w2930, w2929, w2944, w2928, w2927, w2941, w2896, w2912, w2897, w2894, w2910, w2895, w2908, w2907) -> (w2906:dbl[][])
            n1455 = Cluster To Array(cluster=w2893) -> (array=w2939:string[])
          }
        }
      }
    }
    "AI labels" <- w2096
    n1456 = Decimate 1D Array(w2066) -> (w2094:u32[], w2030:u32[])
    n1457 = local read "DMA Update Period (s)"() -> (w2105:dbl)
    n1458 = local read "BD 1 Frequency 2 (MHz)"() -> (w1972:dbl)
    n1459 = local read "BD 1 Frequency 1 (MHz)"() -> (w1973:dbl)
    n1460 = Build Array(w2094, w2030) -> (w2173:u32[][])
    n1461 = local read "Data Period (s)"() -> (w2079:dbl)
    n1462 = Decimate 1D Array(w1980) -> (w2003:i16[], w2002:i16[], w2000:i16[], w1999:i16[])  [unwired: 9 out]
    n1463 = To Double Precision Float(number=w2173) -> (double precision float=w2174:dbl[][])
    n1464 = local read "APD Integration Time (s)"() -> (w2043:dbl)
    n1465 = Divide(x=w2003, y=w2002) -> (x/y=w2004:dbl[])
    n1466 = Divide(x=w2000, y=w1999) -> (x/y=w2001:dbl[])
    n1467 = feedback #1(0.0) -> (w2017:dbl)
    n1468 = Add(x=w2105, y=w2017) -> (x+y=w2213:dbl)
    n1469 = feedback-in #1(w2213) -> ()
    n1470 = local read "AOM X Cal (nm/MHz)"() -> (w1970:dbl)
    n1471 = To Time Stamp(1:w2017) -> (0:w2016:timestamp)
    n1472 = Split 1D Array(array=w2004, index="N El. to Ave.") -> (second subarray=w2007:dbl[])  [unwired: 1 out]
    n1473 = Split 1D Array(array=w2001, index="N El. to Ave.") -> (second subarray=w2006:dbl[])  [unwired: 1 out]
    n1474 = local read "Trap X AI1 (DMA)"() -> (w2005:T13)
    n1475 = Multiply(x=w2079, y="Trap Disp. Downsample") -> (x*y=w2018:dbl)
    "Display Period (s)" <- w2018
    n1476 = Bundle("BD 1 Frequency 1 (MHz)"=w1973, "BD 1 Frequency 2 (MHz)"=w1972) -> (w1974:T45)  [unwired: 1 out]
    n1477 = for "Trap AI" {
      tunnel: [w2627] -> w2207 mode=indexing
      tunnel: w2016 -> [w2617]
      tunnel: "Trap Disp. Downsample" -> [w2625]
      tunnel: w2097 -> [w2623] mode=indexing
      tunnel: w2079 -> [w2622]
      tunnel: w2096 -> [w2621] mode=indexing
      tunnel: w2015 -> [w2620]
      tunnel: [w2619] -> w2054 mode=indexing
      tunnel: w2018 -> [w2618]
      n1478 = Bundle By Name("Y"=w2623, "dt"=w2622) -> (w2624:waveform(dbl))  [unwired: 1 out]
      n1479 = Set Waveform Attribute(5:w2621, 6:w2620, 7:w2624) -> (3:w2619:waveform(dbl))  [unwired: 1 in, 2 out]
      n1480 = call "downsample 1D array - double.vi"("Ave N"=w2625, "Array In"=w2623) -> ("Array Out"=w2626:dbl[])  [unwired: 1 out]
      n1481 = Bundle By Name(cluster=w2619, "t0"=w2617, "Y"=w2626, "dt"=w2618) -> (w2627:waveform(dbl))
    }
    n1482 = call-poly <vilib>:"Mean.vi"("X"=w2006) -> ("mean"=w1994:dbl)  [unwired: 1 out]
    n1483 = call-poly <vilib>:"Mean.vi"("X"=w2007) -> ("mean"=w1995:dbl)  [unwired: 1 out]
    n1484 = Cluster To Array(cluster=w1974) -> (array=w1971:dbl[])
    n1485 = Reciprocal(x=w2018) -> (1/x=→"Trap Disp. Freq. (Hz)":dbl)
    n1486 = local read "Data points/scans (MCL)"() -> (w2185:dbl)
    n1487 = To Fixed-Point(number=w1994) -> (fixed-point=w1992:fxp<+/-,16,1>)  [unwired: 1 in]
    n1488 = To Fixed-Point(number=w1995) -> (fixed-point=w1993:fxp<+/-,16,1>)  [unwired: 1 in]
    n1489 = Bundle("Trap 1 Pos.", "Trap 2 Pos.") -> (w2014:cluster{string, string})  [unwired: 1 out]
    n1490 = Bundle By Name(cluster=w2005, "Set 1"=w1993, "Set 2"=w1992) -> (→"Trap X AI1 (DMA)":T13)
    n1491 = Cluster To Array(cluster=w2014) -> (array=w2011:string[])
    n1492 = for "Trap Position" {
      tunnel: w2020 -> [w2267] mode=indexing
      tunnel: "Trap Disp. Downsample" -> [w2266]
      tunnel: w2018 -> [w2264]
      tunnel: w2016 -> [w2263]
      tunnel: w2015 -> [w2261]
      tunnel: w2011 -> [w2260] mode=indexing
      tunnel: [w2259] -> w1969 mode=indexing
      tunnel: w1971 -> [w2257] mode=indexing
      tunnel: w1970 -> [w2255]
      n1493 = call "downsample 1D array - double.vi"("Ave N"=w2266, "Array In"=w2267) -> ("Array Out"=w2265:dbl[])  [unwired: 1 out]
      n1494 = Subtract(x=w2265, y=w2257) -> (x-y=w2258:dbl[])
      n1495 = Multiply(x=w2255, y=w2258) -> (x*y=w2256:dbl[])
      n1496 = Bundle By Name("Y"=w2256, "dt"=w2264, "t0"=w2263) -> (w2262:waveform(dbl))  [unwired: 1 out]
      n1497 = Set Waveform Attribute(5:w2260, 6:w2261, 7:w2262) -> (3:w2259:waveform(dbl))  [unwired: 1 in, 2 out]
    }
    "Trap Positions" <- w1969
    n1498 = Bundle("APD 1", "APD 2") -> (w2206:cluster{string, string})  [unwired: 1 out]
    n1499 = Cluster To Array(cluster=w2206) -> (array=w2203:string[])
    n1500 = for "APD" {
      tunnel: w2174 -> [w2606] mode=indexing
      tunnel: w2043 -> [w2614]
      tunnel: [w2610] -> w2050 mode=indexing
      tunnel: "APD Disp. Scale" -> [w2611]
      tunnel: w2015 -> [w2609]
      tunnel: w2203 -> [w2608] mode=indexing
      tunnel: "APD Disp. Downsample" -> [w2604]
      tunnel: [w2607] -> w2202
      tunnel: w2016 -> [w2603]
      n1501 = call "integrate 1D array interval - double.vi"("Ave N"=w2604, "Array In"=w2606) -> ("Array Out"=w2605:dbl[])  [unwired: 1 out]
      n1502 = Multiply(x=w2614, y=w2604) -> (x*y=w2607:dbl)
      n1503 = Divide(x=w2605, y=w2611) -> (x/y=w2612:dbl[])
      n1504 = Bundle By Name("t0"=w2603, "Y"=w2612, "dt"=w2607) -> (w2613:waveform(dbl))  [unwired: 1 out]
      n1505 = Set Waveform Attribute(5:w2608, 6:w2609, 7:w2613) -> (3:w2610:waveform(dbl))  [unwired: 1 in, 2 out]
    }
    "APD Display Period (s)" <- w2202
    n1506 = Reciprocal(x=w2202) -> (1/x=→"APD Display Freq. (Hz)":dbl)
    n1507 = local read "Display Period (s)"() -> (w2078:dbl)
    n1508 = Increment(x=w2185) -> (x+1=w2186:dbl)
    n1509 = Index Array(array=w1969, index=0) -> (element=w1967:waveform(dbl))
    n1510 = To Double Precision Float(number=w2094) -> (double precision float=w2093:dbl[])
    n1511 = feedback #2(w2186) -> (w2189:dbl)
    n1512 = Select(t=0, s=w2176, f=w2189) -> (s? t:f=w2182:dbl)
    n1513 = Array Size(array=w2093) -> (size(s)=w2188:i32)
    n1514 = Add(x=w2188, y=w2182) -> (x+y=w2183:dbl)
    n1515 = Unbundle By Name(w1967) -> ("Y"=w1965:dbl[])
    n1516 = feedback #3(w2094) -> (w2172:u32[])
    n1517 = Build Array (concatenate)(w2172, w2094) -> (w2169:u32[])
    n1518 = feedback #4(w2030) -> (w2049:u32[])
    n1519 = Divide(x="Bead Sep. Int. Time (s)", y=w2078) -> (x/y=w1963:dbl)
    n1520 = Build Array (concatenate)(w2049, w2030) -> (w2048:u32[])
    n1521 = Greater?(x=w2183, y=w2185) -> (0:w2184:bool)
    n1522 = feedback #5(w1965) -> (w1966:dbl[])
    n1523 = Build Array (concatenate)(w1965, w1966) -> (w1964:dbl[])
    n1524 = Select(t=w2182, s=w2184, f=w2183) -> (s? t:f=w2181:dbl)
    n1525 = feedback-in #2(w2181) -> ()
    n1526 = Array Size(array=w2169) -> (size(s)=w2166:i32)
    n1527 = Array Size(array=w2094) -> (size(s)=w2168:i32)
    n1528 = local read "MCL Scanning"() -> (w2179:bool)
    n1529 = local read "APD Integration Time (s)"() -> (w2057:dbl)
    n1530 = Build Array (concatenate)(w2050, w2207) -> (w2052:waveform(dbl)[])
    "All Signals" <- w2052
    n1531 = Split 1D Array(array=w1964, index=w1963) -> (first subarray=w1957:dbl[])  [unwired: 1 out]
    n1532 = feedback-in #5(w1957) -> ()
    n1533 = Multiply(x=w2168, y="APD Ave N") -> (x*y=w2167:dbl)
    n1534 = Greater?(x=w2166, y=w2167) -> (0:w2170:bool)
    n1535 = Not(x=w2184) -> (.not. x?=w2178:bool)
    n1536 = To Double Precision Float(number=w2030) -> (double precision float=w2029:dbl[])
    n1537 = call-poly <vilib>:"Mean.vi"("X"=w1957) -> ("mean"=w1956:dbl)  [unwired: 1 out]
    "Mean T1 Position (nm)" <- w1956
    n1538 = Subtract(x=w1957, y=w1956) -> (x-y=w1962:dbl[])
    n1539 = Square(x=w1962) -> (x^2=w1961:dbl[])
    n1540 = And(x=w2178, y=w2179) -> (x .and. y?=w2180:bool)
    n1541 = call-poly <vilib>:"Mean.vi"("X"=w1961) -> ("mean"=w1960:dbl)  [unwired: 1 out]
    n1542 = case shown="True" w2170 {
      tunnel: w2169 -> [w2387 w2394]
      tunnel: [w2387 w2392] -> w2110
      tunnel: w2167 -> [_ w2389]
      tunnel: w2166 -> [_ w2393]
      tunnel: w2048 -> [w2386 w2391]
      tunnel: [w2386 w2388] -> w2045
      frame False {
      }
      frame True {
        n1543 = Subtract(x=w2393, y=w2389) -> (x-y=w2390:dbl)
        n1544 = Array Subset(array=w2394, index=w2390, length=w2389) -> (w2392:u32[])
        n1545 = Array Subset(array=w2391, index=w2390, length=w2389) -> (w2388:u32[])
      }
    }
    n1546 = feedback-in #3(w2110) -> ()
    n1547 = feedback-in #4(w2045) -> ()
    n1548 = Or(x=w2180, y=w2176) -> (x .or. y?=w2177:bool)
    n1549 = Square Root(x=w1960) -> (sqrt(x)=w1959:dbl)
    n1550 = Equal?(x="Tab Control 6", y=T35."High Res Display") -> (x = y?=w2100:bool)
    n1551 = Multiply(x="APD Disp. Scale", y=w2050) -> (x*y=w2059:waveform(dbl)[])
    n1552 = Multiply(x="APD Disp. Downsample", y=w2057) -> (x*y=w2055:dbl)
    n1553 = Multiply(x=10.0, y=w1959) -> (x*y=→"Trap 1 Position RMS (A)":dbl)
    n1554 = Divide(x=w2059, y=w2055) -> (x/y=w2027:waveform(dbl)[])
    n1555 = Index Array(array=w2027, index=0) -> (element=w2037:waveform(dbl))
    n1556 = case "For computing FFTs for display" shown="True" "Compute FFT" {
      tunnel: w2054 -> [_ w3064]
      frame False {
      }
      frame True {
        n1557 = Build Array("FFT 1 Choice 1", "FFT 1 Choice 2", "FFT 2 Choice 1", "FFT 2 Choice 2") -> (w3057:u16[])
        n1558 = Array Size(array=w3064) -> (size(s)=w3063:i32)
        n1559 = feedback-in #6(w3057) -> ()
        n1560 = feedback #6(u16[] [100, 100, 100, 100]) -> (w3058:u16[])
        n1561 = feedback-in #7("# Spectra to Ave.") -> ()
        n1562 = feedback #7("# Spectra to Ave.") -> (w3055:dbl)
        n1563 = Not Equal?(x="# Spectra to Ave.", y=w3055) -> (x != y?=w3054:bool)
        n1564 = Not Equal?(x=w3057, y=w3058) -> (x != y?=w3056:bool)
        n1565 = feedback #8(1.0) -> (w3041:dbl)
        n1566 = Compound Arithmetic op=OR("Reset FFT", w3056, w3054) -> (w3039:bool)
        n1567 = Select(t=1.0, s=w3039, f=w3041) -> (s? t:f=w3043:dbl)
        n1568 = Greater?(x=w3043, y="# Spectra to Ave.") -> (0:w3062:bool)
        n1569 = Increment(x=w3043) -> (x+1=w3042:dbl)
        n1570 = feedback-in #8(w3042) -> ()
        n1571 = local read "DMA Update Period (s)"() -> (w3037:dbl)
        n1572 = Multiply(x="# Spectra to Ave.", y=w3037) -> (x*y=→"Ave. Time (s)":dbl)
        n1573 = Build Array(cluster{"f0":dbl, "df":dbl, "magnitude":dbl[]} {"f0"=0.0, "df"=0.0, "magnitude"=[]} ("PSD")) -> (w3046:cluster{"f0":dbl, "df":dbl, "magnitude":dbl[]}[])
        n1574 = Build Array(w3046, w3046, w3046, w3046) -> (w3048:T46)
        n1575 = feedback #9(w3048) -> (w3053:T46)
        n1576 = for {
          N: 4 -> [_]
          tunnel: w3057 -> [w3086] mode=indexing
          tunnel: w3064 -> [w3087]
          tunnel: w3063 -> [w3089]
          tunnel: w3039 -> [w3082]
          tunnel: w3062 -> [w3081]
          tunnel: "# Spectra to Ave." -> [w3080]
          tunnel: [w3079] -> w3052 mode=indexing
          tunnel: w3053 -> [w3084] mode=indexing
          tunnel: [w3083] -> w3040 mode=indexing
          tunnel: w3043 -> [w3078]
          n1577 = Less?(x=w3086, y=w3089) -> (x < y?=w3088:bool)
          n1578 = Index Array(array=w3087, index=w3086) -> (element=w3085:waveform(dbl))
          n1579 = case shown="True" w3088 {
            tunnel: w3085 -> [_ w3106]
            tunnel: w3084 -> [w3091 w3104]
            tunnel: [w3091 w3092] -> w3083
            tunnel: w3082 -> [_ w3103]
            tunnel: w3081 -> [_ w3096]
            tunnel: w3080 -> [_ w3095]
            tunnel: [cluster{"f0":dbl, "df":dbl, "magnitude":dbl[]} {"f0"=0.0, "df"=0.0, "magnitude"=[]} ("PSD") w3097] -> w3079
            tunnel: w3078 -> [_ w3094]
            frame False {
            }
            frame True {
              n1580 = call <vilib>:"Std Deviation and Variance.vi"("X"=w3106) -> ("mean"=w3107:dbl)  [unwired: 1 in, 2 out]
              n1581 = Subtract(x=w3106, y=w3107) -> (x-y=w3105:waveform(dbl))
              n1582 = xnode "Spectral Measurements"("Signals"=w3105) -> ("PSD"=w3099:cluster{"f0":dbl, "df":dbl, "magnitude":dbl[]})  [unwired: 1 in, 1 out]
              n1583 = case shown="False" w3103 {
                tunnel: w3104 -> [w3116 _]
                tunnel: [w3112 w3121] -> w3092
                tunnel: w3099 -> [w3115 w3122]
                tunnel: w3096 -> [w3114 _]
                frame False {
                  n1584 = Build Array (concatenate)(w3116, w3115) -> (w3113:cluster{"f0":dbl, "df":dbl, "magnitude":dbl[]}[])
                  n1585 = case shown="True" w3114 {
                    tunnel: w3113 -> [w3117 w3120]
                    tunnel: [w3117 w3118] -> w3112
                    frame False {
                    }
                    frame True {
                      n1586 = Delete From Array(array=w3120, index=0) -> (array with subset deleted=w3118:cluster{"f0":dbl, "df":dbl, "magnitude":dbl[]}[])  [unwired: 1 in, 1 out]
                    }
                  }
                }
                frame True {
                  n1587 = Build Array(w3122) -> (w3121:cluster{"f0":dbl, "df":dbl, "magnitude":dbl[]}[])
                }
              }
              n1588 = for {
                tunnel: w3092 -> [w3111] mode=indexing
                tunnel: [w3110] -> w3102 mode=indexing
                workers-P: _ -> [_]
                n1589 = Unbundle By Name(w3111) -> ("magnitude"=w3110:dbl[])
              }
              n1590 = Transpose 2D Array(2D array=w3102) -> (transposed array=w3101:dbl[][])
              n1591 = for {
                tunnel: w3101 -> [w3109] mode=indexing
                tunnel: [w3108] -> w3100 mode=indexing
                workers-P: _ -> [_]
                n1592 = Add Array Elements(numeric array=w3109) -> (sum=w3108:dbl)
              }
              n1593 = Select(t=w3095, s=w3096, f=w3094) -> (s? t:f=w3093:dbl)
              n1594 = Divide(x=w3100, y=w3093) -> (x/y=w3098:dbl[])
              n1595 = Bundle By Name(cluster=w3099, "magnitude"=w3098) -> (w3097:cluster{"f0":dbl, "df":dbl, "magnitude":dbl[]})
            }
          }
        }
        n1596 = case shown="True" w3039 {
          tunnel: w3040 -> [w3071 w3077]
          tunnel: [w3071 w3072] -> w3038
          frame False {
          }
          frame True {
            n1597 = Array Subset(array=w3077, index (row)=0 ("index"), length (row)=4 ("length"), index (col)=0 ("index"), length (col)=1 ("length")) -> (w3072:T46)
          }
        }
        n1598 = feedback-in #9(w3038) -> ()
        n1599 = Split 1D Array(array=w3052, index=2) -> (first subarray=→"FFT 1":cluster{"f0":dbl, "df":dbl, "magnitude":dbl[]}[], second subarray=→"FFT 2":cluster{"f0":dbl, "df":dbl, "magnitude":dbl[]}[])
      }
    }
    n1600 = Index Array(array=w2027, index=1) -> (element=w2035:waveform(dbl))
    n1601 = case "For displaying the high resolution display (no downsampling)" shown="True" w2100 {
      tunnel: w2054 -> [_ w2287]
      frame False {
      }
      frame True {
        n1602 = Index Array(array=w2287, index="High Res. Display") -> (element=w2288:waveform(dbl))
        n1603 = call <vilib>:"Std Deviation and Variance.vi"("X"=w2288) -> ("mean"=w2295:dbl, "standard deviation"=w2300:dbl)  [unwired: 1 in, 1 out]
        "Mean Intensity" <- w2295
        "Sigma" <- w2300
        n1604 = Subtract(x=w2288, y=w2295) -> (x-y=w2294:waveform(dbl))
        n1605 = Select(t=w2294, s="Subtract mean", f=w2288) -> (s? t:f=→"1 Channel":waveform(dbl))
        n1606 = Divide(x=w2300, y=w2295) -> (x/y=→"Sigma/Mean":dbl)
        n1607 = feedback #10(1) -> (w2289:i32)
        n1608 = Greater Or Equal?(x=w2289, y="Slow mean N ave.") -> (x >= y?=w2302:bool)
        n1609 = Increment(x=w2289) -> (x+1=w2304:i32)
        n1610 = Select(t=1, s=w2302, f=w2304) -> (s? t:f=w2291:i32)
        n1611 = feedback-in #10(w2291) -> ()
        n1612 = feedback #11() -> (w2292:waveform(dbl))  [unwired: 1 out]
        n1613 = case shown="Default" w2289 {
          tunnel: [w2307 w2310] -> w2293
          tunnel: w2292 -> [w2309 _]
          tunnel: w2288 -> [w2308 w2310]
          frame Default {
            n1614 = call-poly <vilib>:"Append Waveforms.vi"("waveform B"=w2308, "waveform A"=w2309) -> ("waveform out"=w2307:waveform(dbl))  [unwired: 1 in, 8 out]
          }
          frame 1 {
          }
        }
        n1615 = feedback-in #11(w2293) -> ()
        n1616 = case shown="True" w2302 {
          tunnel: w2293 -> [_ w2306]
          frame False {
          }
          frame True {
            n1617 = call-poly <vilib>:"Mean.vi"("X"=w2306) -> ("mean"=→"Slow mean":dbl)  [unwired: 1 out]
          }
        }
      }
    }
    n1618 = case "For plotting results of scanning MCL" shown="True" w2177 {
      tunnel: w2176 -> [_ w2427]
      tunnel: w2093 -> [_ w2523]
      tunnel: w2185 -> [_ _]
      tunnel: w2054 -> [_ w2497]
      tunnel: w2029 -> [_ w2428]
      tunnel: w2028 -> [_ w2401]
      frame False {
      }
      frame True {
        w2408 = u32 0 items=["Horizontal", "Vertical", "Central", "1st Diagonal", "2nd Diagonal"] ("Type of Symmetry")
        w2436 = u32 0 items=["Horizontal", "Vertical", "Central", "1st Diagonal", "2nd Diagonal"] ("Type of Symmetry")
        w2439 = u32 0 items=["Horizontal", "Vertical", "Central", "1st Diagonal", "2nd Diagonal"] ("Type of Symmetry")
        w2468 = u32 0 items=["Horizontal", "Vertical", "Central", "1st Diagonal", "2nd Diagonal"] ("Type of Symmetry")
        n1619 = Index Array(array=w2497, index=10) -> (element=w2503:waveform(dbl))
        n1620 = Index Array(array=w2497, index=11) -> (element=w2500:waveform(dbl))
        n1621 = local read "Cycles/step (MCL)"() -> (w2453:u64)
        n1622 = Index Array(array=w2497, index="Channel") -> (element=w2499:waveform(dbl))
        n1623 = Unbundle(w2401) -> ("New Image"=w2400:T2, "New Image"=w2399:T2, "New Image"=w2398:T2, "New Image"=w2397:T2)
        n1624 = Unbundle By Name(w2503) -> ("Y"=w2455:dbl[])
        n1625 = Unbundle By Name(w2500) -> ("Y"=w2457:dbl[])
        n1626 = Unbundle By Name(w2499) -> ("Y"=w2462:dbl[])
        n1627 = call "downsample 1D array - double.vi"("Ave N"=w2453, "Array In"=w2455) -> ("Array Out"=w2454:dbl[])  [unwired: 1 out]
        n1628 = call "downsample 1D array - double.vi"("Ave N"=w2453, "Array In"=w2457) -> ("Array Out"=w2456:dbl[])  [unwired: 1 out]
        n1629 = call "downsample 1D array - double.vi"("Ave N"=w2453, "Array In"=w2462) -> ("Array Out"=w2461:dbl[])  [unwired: 1 out]
        n1630 = feedback #12(w2523) -> (w2524:dbl[])
        n1631 = Build Array (concatenate)(w2524, w2523) -> (w2505:dbl[])
        n1632 = feedback #13(w2428) -> (w2430:dbl[])
        n1633 = Build Array (concatenate)(w2430, w2428) -> (w2429:dbl[])
        n1634 = local read "Scan steps (MCL)"() -> (w2410:u64)
        n1635 = Select(t=w2523, s=w2427, f=w2505) -> (s? t:f=w2509:dbl[])
        n1636 = feedback-in #12(w2509) -> ()
        n1637 = Select(t=w2428, s=w2427, f=w2429) -> (s? t:f=w2411:dbl[])
        n1638 = feedback-in #13(w2411) -> ()
        n1639 = local read "Scan lines (y)"() -> (w2396:u64)
        n1640 = local read "N APD Samp/step"() -> (w2412:dbl)
        n1641 = feedback #14(w2454) -> (w2511:dbl[])
        n1642 = Build Array (concatenate)(w2511, w2454) -> (w2502:dbl[])
        n1643 = feedback #15(w2461) -> (w2521:dbl[])
        n1644 = Build Array (concatenate)(w2521, w2461) -> (w2520:dbl[])
        n1645 = feedback #16(w2456) -> (w2513:dbl[])
        n1646 = Build Array (concatenate)(w2513, w2456) -> (w2514:dbl[])
        n1647 = Select(t=w2454, s=w2427, f=w2502) -> (s? t:f=w2458:dbl[])
        n1648 = feedback-in #14(w2458) -> ()
        n1649 = Select(t=w2461, s=w2427, f=w2520) -> (s? t:f=w2460:dbl[])
        n1650 = feedback-in #15(w2460) -> ()
        n1651 = Select(t=w2456, s=w2427, f=w2514) -> (s? t:f=w2459:dbl[])
        n1652 = feedback-in #16(w2459) -> ()
        n1653 = Multiply(x=w2410, y=u64 2) -> (x*y=w2395:u64)
        n1654 = call "integrate 1D array interval - double.vi"("Ave N"=w2412, "Array In"=w2411) -> ("Array Out"=w2423:dbl[])  [unwired: 1 out]
        n1655 = call "integrate 1D array interval - double.vi"("Ave N"=w2412, "Array In"=w2509) -> ("Array Out"=w2508:dbl[])  [unwired: 1 out]
        n1656 = Array Size(array=w2423) -> (size(s)=w2424:i32)
        n1657 = Array Size(array=w2508) -> (size(s)=w2510:i32)
        n1658 = Multiply(x=w2396, y=w2395) -> (x*y=w2426:u64)
        n1659 = Multiply(x=w2396, y=w2395) -> (x*y=w2518:u64)
        n1660 = call-poly <vilib>:"Mean.vi"("X"=w2458) -> ("mean"=w2442:dbl)  [unwired: 1 out]
        n1661 = Subtract(x=w2426, y=w2424) -> (x-y=w2417:u64)
        n1662 = call-poly <vilib>:"Mean.vi"("X"=w2460) -> ("mean"=w2447:dbl)  [unwired: 1 out]
        n1663 = call-poly <vilib>:"Mean.vi"("X"=w2459) -> ("mean"=w2445:dbl)  [unwired: 1 out]
        n1664 = call-poly <vilib>:"Mean.vi"("X"=w2423) -> ("mean"=w2414:dbl)  [unwired: 1 out]
        n1665 = Subtract(x=w2518, y=w2510) -> (x-y=w2452:u64)
        n1666 = call-poly <vilib>:"Mean.vi"("X"=w2508) -> ("mean"=w2449:dbl)  [unwired: 1 out]
        n1667 = Initialize Array(1.0 ("element"), w2417) -> (w2413:dbl[])
        n1668 = Initialize Array(1.0 ("element"), w2452) -> (w2443:dbl[])
        n1669 = Multiply(x=w2413, y=w2414) -> (x*y=w2415:dbl[])
        n1670 = Multiply(x=w2443, y=w2445) -> (x*y=w2446:dbl[])
        n1671 = Multiply(x=w2443, y=w2447) -> (x*y=w2448:dbl[])
        n1672 = Multiply(x=w2443, y=w2442) -> (x*y=w2444:dbl[])
        n1673 = Multiply(x=w2443, y=w2449) -> (x*y=w2450:dbl[])
        n1674 = Build Array (concatenate)(w2458, w2444) -> (w2512:dbl[])
        n1675 = Build Array (concatenate)(w2460, w2448) -> (w2516:dbl[])
        n1676 = Build Array (concatenate)(w2459, w2446) -> (w2515:dbl[])
        n1677 = Build Array (concatenate)(w2423, w2415) -> (w2425:dbl[])
        n1678 = Build Array (concatenate)(w2508, w2450) -> (w2517:dbl[])
        n1679 = Reshape Array(w2512, w2396, w2395) -> (w2478:dbl[][])
        n1680 = Reshape Array(w2425, w2396, w2395) -> (w2421:dbl[][])
        n1681 = Reshape Array(w2516, w2396, w2395) -> (w2470:dbl[][])
        n1682 = Reshape Array(w2515, w2396, w2395) -> (w2485:dbl[][])
        n1683 = Reshape Array(w2517, w2396, w2395) -> (w2495:dbl[][])
        n1684 = Array Subset(array=w2485, index (col)=0 ("index"), length (col)=w2410) -> (w2490:dbl[][])  [unwired: 2 in]
        n1685 = Array Subset(array=w2485, index (col)=w2410) -> (w2488:dbl[][])  [unwired: 3 in]
        n1686 = Array Subset(array=w2470, index (col)=0 ("index"), length (col)=w2410) -> (w2476:dbl[][])  [unwired: 2 in]
        n1687 = Array Subset(array=w2470, index (col)=w2410) -> (w2474:dbl[][])  [unwired: 3 in]
        n1688 = Array Subset(array=w2421, index (col)=0 ("index"), length (col)=w2410) -> (w2420:dbl[][])  [unwired: 2 in]
        n1689 = Array Subset(array=w2421, index (col)=w2410) -> (w2418:dbl[][])  [unwired: 3 in]
        n1690 = Array Subset(array=w2495, index (col)=0 ("index"), length (col)=w2410) -> (w2494:dbl[][])  [unwired: 2 in]
        n1691 = Array Subset(array=w2495, index (col)=w2410) -> (w2492:dbl[][])  [unwired: 3 in]
        n1692 = Array Subset(array=w2478, index (col)=0 ("index"), length (col)=w2410) -> (w2483:dbl[][])  [unwired: 2 in]
        n1693 = Array Subset(array=w2478, index (col)=w2410) -> (w2481:dbl[][])  [unwired: 3 in]
        n1694 = for {
          tunnel: w2490 -> [w2532] mode=indexing
          tunnel: [w2531] -> w2489 mode=indexing
          workers-P: _ -> [_]
          n1695 = Reverse 1D Array(array=w2532) -> (reversed array=w2531:dbl[])
        }
        n1696 = for {
          tunnel: w2476 -> [w2528] mode=indexing
          tunnel: [w2527] -> w2475 mode=indexing
          workers-P: _ -> [_]
          n1697 = Reverse 1D Array(array=w2528) -> (reversed array=w2527:dbl[])
        }
        n1698 = for {
          tunnel: w2420 -> [w2526] mode=indexing
          tunnel: [w2525] -> w2419 mode=indexing
          workers-P: _ -> [_]
          n1699 = Reverse 1D Array(array=w2526) -> (reversed array=w2525:dbl[])
        }
        n1700 = for {
          tunnel: w2494 -> [w2534] mode=indexing
          tunnel: [w2533] -> w2493 mode=indexing
          workers-P: _ -> [_]
          n1701 = Reverse 1D Array(array=w2534) -> (reversed array=w2533:dbl[])
        }
        n1702 = for {
          tunnel: w2483 -> [w2530] mode=indexing
          tunnel: [w2529] -> w2482 mode=indexing
          workers-P: _ -> [_]
          n1703 = Reverse 1D Array(array=w2530) -> (reversed array=w2529:dbl[])
        }
        n1704 = Index Array(array=w2495, index (row)=0) -> (element=→"Waveform Graph":dbl[])  [unwired: 1 in]
        n1705 = Add(x=w2489, y=w2488) -> (x+y=w2487:dbl[][])
        n1706 = Add(x=w2475, y=w2474) -> (x+y=w2473:dbl[][])
        n1707 = Add(x=w2419, y=w2418) -> (x+y=w2403:dbl[][])
        n1708 = Add(x=w2493, y=w2492) -> (x+y=w2467:dbl[][])
        n1709 = Add(x=w2482, y=w2481) -> (x+y=w2480:dbl[][])
        n1710 = Divide(x=w2473, y=2) -> (x/y=w2471:dbl[][])
        n1711 = Divide(x=w2487, y=2) -> (x/y=w2432:dbl[][])
        n1712 = Divide(x=w2480, y=2) -> (x/y=w2434:dbl[][])
        n1713 = To Single Precision Float(number=w2467) -> (single precision float=w2466:sgl[][])
        n1714 = Transpose 2D Array(2D array=w2471) -> (transposed array=→"Data map":dbl[][])
        n1715 = To Single Precision Float(number=w2403) -> (single precision float=w2407:sgl[][])
        n1716 = To Single Precision Float(number=w2432) -> (single precision float=w2438:sgl[][])
        n1717 = To Single Precision Float(number=w2434) -> (single precision float=w2435:sgl[][])
        n1718 = call "IMAQ ArrayToImage"("Image Pixels (Float)"=w2466, "Image"=w2400) -> ("Image Out"=w2469:T2)  [unwired: 8 in, 1 out]
        n1719 = call "IMAQ ArrayToImage"("Image Pixels (Float)"=w2407, "Image"=w2399) -> ("Image Out"=w2409:T2)  [unwired: 8 in, 1 out]
        n1720 = call "IMAQ ArrayToImage"("Image Pixels (Float)"=w2438, "Image"=w2398) -> ("Image Out"=w2440:T2)  [unwired: 8 in, 1 out]
        n1721 = call "IMAQ ArrayToImage"("Image Pixels (Float)"=w2435, "Image"=w2397) -> ("Image Out"=w2437:T2)  [unwired: 8 in, 1 out]
        n1722 = call "IMAQ Symmetry"("Type of Symmetry"=w2468, "Image Src"=w2469) -> ("Image Dst Out"=w2464:T2)  [unwired: 3 in, 1 out]
        n1723 = call "IMAQ Symmetry"("Type of Symmetry"=w2408, "Image Src"=w2409) -> ("Image Dst Out"=w2405:T2)  [unwired: 3 in, 1 out]
        n1724 = call "IMAQ Symmetry"("Type of Symmetry"=w2439, "Image Src"=w2440) -> ("Image Dst Out"=→"Detection Laser X":T2)  [unwired: 3 in, 1 out]
        n1725 = call "IMAQ Symmetry"("Type of Symmetry"=w2436, "Image Src"=w2437) -> ("Image Dst Out"=→"Detection Laser Y":T2)  [unwired: 3 in, 1 out]
        n1726 = call "IMAQ Set Simple Calibration"("Calibration Axis Info"=T36 {"Origin Pixel"={"X"=0.0, "Y"=0.0}, "Angle Relative to Horizontal (deg)"=0.0, "Axis Reference"=0}, "Grid Descriptor"=T37 {"X Step"=0.3, "Y Step"=0.3, "Unit"=enum."Undefined"}, "Image"=w2464) -> ("Calibrated Image"=→"APD 1":T2)  [unwired: 7 in, 1 out]
        n1727 = call "IMAQ Set Simple Calibration"("Calibration Axis Info"=T36 {"Origin Pixel"={"X"=0.0, "Y"=0.0}, "Angle Relative to Horizontal (deg)"=0.0, "Axis Reference"=0}, "Grid Descriptor"=T37 {"X Step"=0.3, "Y Step"=0.3, "Unit"=enum."Undefined"}, "Image"=w2405) -> ("Calibrated Image"=→"APD 2":T2)  [unwired: 7 in, 1 out]
      }
    }
    n1728 = Subtract(x=w2035, y="APD 2 Offset") -> (x-y=w2032:waveform(dbl))
    n1729 = Subtract(x=w2037, y="APD 1 Offset") -> (x-y=w2033:waveform(dbl))
    n1730 = Index Array(array=w2052, index=3) -> (element=w2121:waveform(dbl))
    n1731 = Index Array(array=w2052, index=6) -> (element=w2118:waveform(dbl))
    n1732 = Build Array(w2033, w2032) -> (→"APD Chart":waveform(dbl)[])
    n1733 = Array Size(array=w2110) -> (size(s)=w2165:i32)
    n1734 = call <vilib>:"Std Deviation and Variance.vi"("X"=w2045) -> ("standard deviation"=w2044:dbl)  [unwired: 1 in, 2 out]
    n1735 = Add Array Elements(numeric array=w2045) -> (sum=w2047:u32)
    n1736 = Add Array Elements(numeric array=w2110) -> (sum=w2175:u32)
    n1737 = call <vilib>:"Std Deviation and Variance.vi"("X"=w2110) -> ("standard deviation"=w2109:dbl)  [unwired: 1 in, 2 out]
    n1738 = Divide(x="T1 offset_x (mV)", y=1000.0) -> (x/y=w2122:dbl)
    n1739 = Divide(x=w2044, y=w2043) -> (x/y=w2040:dbl)
    "Rate sigma (Hz) 2" <- w2040
    n1740 = Multiply(x=w2043, y=w2165) -> (x*y=w2046:dbl)
    "Int. Time (s)" <- w2046
    n1741 = Divide(x=w2047, y=w2046) -> (x/y=w2041:dbl)
    "APD 2 Rate (Hz)" <- w2041
    n1742 = Divide(x=w2175, y=w2046) -> (x/y=w2107:dbl)
    "APD 1 Rate (Hz)" <- w2107
    n1743 = Divide(x=w2109, y=w2043) -> (x/y=w2108:dbl)
    "Rate sigma (Hz)" <- w2108
    n1744 = Divide(x=w2040, y=w2041) -> (x/y=→"Sigma/Mean 2":dbl)
    n1745 = Divide(x=w2108, y=w2107) -> (x/y=→"Sigma/Mean":dbl)
    n1746 = Divide(x="T2 offset_x (mV)", y=1000.0) -> (x/y=w2120:dbl)
    n1747 = case shown="1" "Calibration" {
      tunnel: "T1 alpha_x (nm/V)" -> [_ w2363 w2384]
      tunnel: "T1 kappa_x (pN/nm)" -> [_ _ w2374]
      tunnel: "T2 alpha_x (nm/V)" -> [_ w2362 w2382]
      tunnel: "T2 kappa_x (pN/nm)" -> [_ _ w2375]
      tunnel: w2121 -> [w2345 w2360 w2380]
      tunnel: w2118 -> [w2344 w2358 w2378]
      tunnel: [w2345 w2357 w2377] -> w2151
      tunnel: [w2344 w2356 w2376] -> w2150
      tunnel: ["T1 X (V)" ("Label.Text") "T1 X (nm)" ("Label.Text") "T1 X (pN)" ("Label.Text")] -> w2139
      tunnel: ["T2 X (V)" ("Label.Text") "T2 X (nm)" ("Label.Text") "T2 X (pN)" ("Label.Text")] -> w2138
      tunnel: ["Position (V)" ("Label.Text") "Position (nm)" ("Label.Text") "Force (pN)" ("Label.Text")] -> w2140
      tunnel: w2120 -> [_ w2348 w2367]
      tunnel: w2122 -> [_ w2351 w2369]
      tunnel: ["Mean (V)" ("Label.Text") "Mean (nm)" ("Label.Text") "Mean (pN)" ("Label.Text")] -> w2135
      tunnel: ["Difference (V)" ("Label.Text") "Difference (nm)" ("Label.Text") "Difference (pN)" ("Label.Text")] -> w2060
      frame 0, Default {
      }
      frame 1 {
        # "position"
        n1748 = Unbundle By Name(w2360) -> ("Y"=w2364:dbl[])
        n1749 = Unbundle By Name(w2358) -> ("Y"=w2349:dbl[])
        n1750 = Subtract(x=w2364, y=w2351) -> (x-y=w2352:dbl[])
        n1751 = Subtract(x=w2349, y=w2348) -> (x-y=w2350:dbl[])
        n1752 = Multiply(x=w2350, y=w2362) -> (x*y=w2359:dbl[])
        n1753 = Multiply(x=w2363, y=w2352) -> (x*y=w2361:dbl[])
        n1754 = Bundle By Name(cluster=w2358, "Y"=w2359) -> (w2356:waveform(dbl))
        n1755 = Bundle By Name(cluster=w2360, "Y"=w2361) -> (w2357:waveform(dbl))
      }
      frame 2 {
        # "force"
        n1756 = Unbundle By Name(w2380) -> ("Y"=w2385:dbl[])
        n1757 = Unbundle By Name(w2378) -> ("Y"=w2383:dbl[])
        n1758 = Subtract(x=w2383, y=w2367) -> (x-y=w2368:dbl[])
        n1759 = Subtract(x=w2385, y=w2369) -> (x-y=w2370:dbl[])
        n1760 = Compound Arithmetic op=MULTIPLY(w2368, w2382, w2375) -> (w2379:dbl[])
        n1761 = Compound Arithmetic op=MULTIPLY(w2374, w2384, w2370) -> (w2381:dbl[])
        n1762 = Bundle By Name(cluster=w2378, "Y"=w2379) -> (w2376:waveform(dbl))
        n1763 = Bundle By Name(cluster=w2380, "Y"=w2381) -> (w2377:waveform(dbl))
      }
    }
    n1764 = feedback-in #17("Calibration") -> ()
    n1765 = feedback #17(u16 1 ("Calibration")) -> (w2142:u16)
    n1766 = Not Equal?(x=w2142, y="Calibration") -> (x != y?=w2098:bool)
    n1767 = Unbundle By Name(w2121) -> ("Y"=w2124:dbl[])
    n1768 = Unbundle By Name(w2118) -> ("Y"=w2127:dbl[])
    n1769 = Subtract(x=w2124, y=w2122) -> (x-y=w2125:dbl[])
    n1770 = Subtract(x=w2127, y=w2120) -> (x-y=w2126:dbl[])
    n1771 = disable-structure shown="Enabled" {
      disable-tunnel: [-1.0 ("y") 1.0] -> w2128
      frame Disabled {
      }
      frame Enabled {
      }
    }
    n1772 = Multiply(x=w2126, y="T2 alpha_x (nm/V)") -> (x*y=w2117:dbl[])
    n1773 = Multiply(x="T1 alpha_x (nm/V)", y=w2125) -> (x*y=w2116:dbl[])
    n1774 = Multiply(x=w2150, y=w2128) -> (x*y=w2129:waveform(dbl))
    n1775 = case shown="False" "Read Lateness and Rel Phase" {
      tunnel: w1952 -> [w2311 w2333]
      tunnel: w1951 -> [w2312 w2332]
      tunnel: [w2311 w2331] -> w2113
      tunnel: [w2312 w2330] -> w2112
      frame False {
      }
      frame True {
        n1776 = xnode "Read/Write Control"("FPGA VI Reference In"=w2333, "error in"=w2332) -> ("FPGA VI Reference Out"=w2331:T19, "error out"=w2330:errorcluster, "GI Relative phase"=→"GI relative phase":i16, "Relative phase"=→"Relative phase (AI1)":i16, "AI Late Counter"=→"Late Counter (AI1)":u16, "GI Late Counter"=→"GI Late Counter":u16, "MCL Late Counter"=→"MCL Late Counter":u16, "MCL Relative Phase"=→"Relative Phase (MCL)":i16, "APD Acq Relative Phase"=→"APD Acq Relative Phase":i16, "APD 1 Gate Relative Phase"=→"APD 1 Gate Relative Phase":i16, "APD 2 Gate Relative Phase"=→"APD 2 Gate Relative Phase":i16, "APD Acq Late Counter"=→"APD Acq Late Counter":u16, "APD 1 Gate Late Counter"=→"APD 1 Gate Late Counter":u16, "APD 2 Gate Late Counter"=→"APD 2 Gate Late Counter":u16, "Green FB Relative Phase"=→"Relative phase (Green FB)":i16, "GI Relative phase 2"=→"GI relative phase 2":i16, "GI Late Counter 2"=→"GI Late Counter 2":u16, "Trap Pos FIFO Timeout"=→"Trap Pos FIFO Timeout":u16, "Trap AI FIFO Timeout"=→"Trap AI FIFO Timeout":u16)
      }
    }
    n1777 = Subtract(x=w2117, y=w2116) -> (x-y=w2115:dbl[])
    n1778 = Unbundle By Name(w2150) -> ("Y"=w2085:dbl[])
    n1779 = Unbundle By Name(w2151) -> ("Y"=w2086:dbl[])
    n1780 = Build Array(w2151, w2129) -> (→"Force":waveform(dbl)[])
    n1781 = Subtract(x=w2115, y="Offset (nm)") -> (x-y=w2083:dbl[])
    n1782 = call-poly <vilib>:"Mean.vi"("X"=w2085) -> ("mean"=w2064:dbl)  [unwired: 1 out]
    "T2 X" <- w2064
    n1783 = Absolute Value(x=w2086) -> (abs(x)=w2087:dbl[])
    n1784 = Absolute Value(x=w2085) -> (abs(x)=w2088:dbl[])
    n1785 = call-poly <vilib>:"Mean.vi"("X"=w2086) -> ("mean"=w2065:dbl)  [unwired: 1 out]
    "T1 X" <- w2065
    n1786 = Add(x=w2087, y=w2088) -> (x+y=w2089:dbl[])
    n1787 = Bundle By Name(cluster=w2121, "Y"=w2083) -> (w2051:waveform(dbl))
    "Bead Separation" <- w2051
    n1788 = Divide(x=w2089, y=2.0) -> (x/y=→"Vec Mean of T1 T2":dbl[])
    n1789 = case shown="True" w2098 {
      tunnel: w2140 -> [_ w2338]
      tunnel: w2139 -> [_ w2337]
      tunnel: w2138 -> [_ w2336]
      tunnel: w2135 -> [_ w2335]
      tunnel: w2060 -> [_ w2334]
      frame False {
      }
      frame True {
        n1790 = property on="Force" class="WFChart (strict)"("YScale.NameLbl.Text"=w2338) -> ()  [unwired: 2 in, 2 out]
        n1791 = property on="T2 X" class="DigNum (strict)"("Caption.Text"=w2336) -> ()  [unwired: 2 in, 2 out]
        n1792 = property on="T1 X" class="DigNum (strict)"("Caption.Text"=w2337) -> ()  [unwired: 2 in, 2 out]
        n1793 = property on="Mean" class="DigNum (strict)"("Caption.Text"=w2335) -> ()  [unwired: 2 in, 2 out]
        n1794 = property on="Difference" class="DigNum (strict)"("Caption.Text"=w2334) -> ()  [unwired: 2 in, 2 out]
      }
    }
    n1795 = local read "Tether"() -> (w2092:bool)
    n1796 = Absolute Value(x=w2065) -> (abs(x)=w2062:dbl)
    n1797 = Absolute Value(x=w2064) -> (abs(x)=w2061:dbl)
    n1798 = Add(x=w2062, y=w2061) -> (x+y=w2137:dbl)
    n1799 = Subtract(x=w2062, y=w2061) -> (x-y=→"Difference":dbl)
    n1800 = feedback #18(w2083) -> (w2082:dbl[])
    n1801 = Divide(x=w2137, y=2.0) -> (x/y=w2091:dbl)
    "Mean" <- w2091
    n1802 = case shown="True" w2092 {
      tunnel: w2091 -> [_ w2270]
      frame False {
      }
      frame True {
        n1803 = Greater?(x="Lost Tether Alarm Threshold (pN)", y=w2270) -> (0:w2268:bool)
        n1804 = case shown="True" w2268 {
          frame False {
          }
          frame True {
            n1805 = flat-sequence {
              frame #0 {
                # "stop only if saving"
                n1806 = local read "Saving..."() -> (w2283:bool)
                n1807 = And(x=w2283, y="TA Cancel Save?") -> (x .and. y?=w2282:bool)
                n1808 = local write "Stop Saving"(w2282) -> ()
              }
              frame #1 {
                n1809 = case shown="True" "TA Green Off?" {
                  frame False {
                  }
                  frame True {
                    w2286 = FALSE ("Fl. Triggered...")
                    n1810 = local write "Fl. Triggered..."(w2286) -> ()
                    n1811 = property on="Green Laser ON/Interlacing" class="Bool (strict)"("Val(Sgnl)"=w2286) -> ()  [unwired: 2 in, 2 out]
                  }
                }
              }
            }
            n1812 = local read "Time tether formed"() -> (w2277:timestamp)
            n1813 = Get Date/Time In Seconds() -> (seconds since 1Jan1904=w2278:timestamp)
            n1814 = Subtract(x=w2278, y=w2277) -> (x-y=w2276:dbl)
            n1815 = Number To Decimal String(number=w2276) -> (decimal integer string=w2273:string)  [unwired: 1 out]
            n1816 = local read "Messages"() -> (w2280:string)
            n1817 = call <vilib>:"Beep.vi"() -> ()  [unwired: 3 in, 9 out]
            n1818 = Concatenate Strings("Lost tether (" ("Message to add"), w2273, " s)." ("string")) -> (w2275:string)
            n1819 = local write "Tether"(FALSE ("Tether")) -> ()
            n1820 = call "Update messages.vi"("Message to add"=w2275, "Old message string"=w2280) -> ("New message string"=w2279:string)
            n1821 = local write "Messages"(w2279) -> ()
            n1822 = property on="Trap Pos. FB ON" class="Bool (strict)"("Val(Sgnl)"=FALSE ("Value (Signaling)")) -> ()  [unwired: 2 in, 2 out]
          }
        }
      }
    }
    n1823 = Build Array (concatenate)(w2083, w2082) -> (w2081:dbl[])
    n1824 = Split 1D Array(array=w2081, index=w1963) -> (first subarray=w2077:dbl[])  [unwired: 1 out]
    n1825 = feedback-in #18(w2077) -> ()
    n1826 = call-poly <vilib>:"Mean.vi"("X"=w2077) -> ("mean"=w2076:dbl)  [unwired: 1 out]
    "Bead Mean (nm)" <- w2076
    n1827 = Subtract(x=w2077, y=w2076) -> (x-y=w2075:dbl[])
    n1828 = Square(x=w2075) -> (x^2=w2074:dbl[])
    n1829 = call-poly <vilib>:"Mean.vi"("X"=w2074) -> ("mean"=w2073:dbl)  [unwired: 1 out]
    n1830 = Square Root(x=w2073) -> (sqrt(x)=w2072:dbl)
    n1831 = Multiply(x=10.0, y=w2072) -> (x*y=→"RMS (Ang)":dbl)
    n1832 = xnode "Read/Write Control"("FPGA VI Reference In"=w2113, "error in"=w2112) -> ("FPGA VI Reference Out"=w2231:T19, "error out"=w2225:errorcluster, "AI2 Y Sum Set 1"=w2221:i16, "AI2 Y Sum Set 2"=w2220:i16, "AI1 X Set 1"=w1997:fxp<+/-,16,1>, "AI1 X Set 2"=w1996:fxp<+/-,16,1>, "Trap Pos FB Int Signal"=→"Trap Pos FB Int Signal":fxp<+/-,24,9>, "Trap Pos FB Int-Norm Signal"=→"Trap Pos FB Int-Norm Signal":fxp<+/-,16,1>, "Trap Pos FB Action"=w1990:i64, "Scanning"=→"AOD Scanning":bool, "Scan I"=→"AOD Scan I":u64, "Scanning MCL"=w2223:bool, "Scan I (MCL)"=→"MCL Scan I":u64, "Green FB Signals"=w2160:T47)  [unwired: 1 out]
    "MCL Scanning" <- w2223
    "Trap Pos FB Action" <- w1990
    n1833 = local read "AI2 (V)"() -> (w2222:cluster{"Set 1":dbl, "Set 2":dbl})
    n1834 = Bundle By Name(cluster=w2222, "Set 1"=w2221, "Set 2"=w2220) -> (w2218:cluster{"Set 1":dbl, "Set 2":dbl})
    n1835 = Divide(x=w1990, y=327.67) -> (x/y=→"Action (%)":dbl)
    n1836 = local read "Trap X (AI1)"() -> (w2010:T10)
    n1837 = Divide(x=w2218, y=3276.7) -> (x/y=w2217:cluster{"Set 1":dbl, "Set 2":dbl})
    n1838 = local write "AI2 (V)"(w2217) -> ()
    n1839 = Bundle(cluster=w2010, "Trap 1"=w1997, "Trap 2"=w1996) -> (→"Trap X (AI1)":T10)
    n1840 = Divide(x=w2160, y=3276.7) -> (x/y=w2156:T48)
    n1841 = Unbundle By Name(w2156) -> ("Green FB Ch 0"=w2159:dbl, "Green FB Ch 1"=w2158:dbl, "Green FB Ch 2"=w2157:dbl)
    n1842 = Divide(x=w2159, y=w2157) -> (x/y=w2155:dbl)
    n1843 = Divide(x=w2158, y=w2157) -> (x/y=w2154:dbl)
    n1844 = flat-sequence "To save data" {
      tunnel: [w3160] -> w2242
      tunnel: [w3161] -> w2241
      tunnel: w2191 -> [w3154]
      tunnel: w2079 -> [w3158]
      tunnel: ["Save Calibration"] -> w2214
      tunnel: w2211 -> [w3157]
      tunnel: [w3150] -> w2210
      tunnel: [w3147] -> w2209
      tunnel: [w3144] -> w2208
      tunnel: w2190 -> [w3146]
      tunnel: w2096 -> [w3140]
      tunnel: [w3140] -> w2095
      tunnel: ["Start Saving"] -> w2053
      tunnel: [w3134] -> w1979
      tunnel: [w3133] -> w1978
      tunnel: w2242 -> [w3395]
      tunnel: w2241 -> [w3394]
      tunnel: w1980 -> [w3393]
      tunnel: w2214 -> [w3392]
      tunnel: w2210 -> [w3390]
      tunnel: w2209 -> [w3389]
      tunnel: w2208 -> [w3388]
      tunnel: w2066 -> [w3387]
      tunnel: w2105 -> [w3386]
      tunnel: w2095 -> [w3385]
      tunnel: w2053 -> [w3384]
      tunnel: w2051 -> [w3383]
      tunnel: w2027 -> [w3382]
      tunnel: w1979 -> [w3381]
      tunnel: w1978 -> [w3380]
      tunnel: w1977 -> [w3379]
      frame #0 {
        n1845 = Or(x="Save N Sets", y="Start Saving") -> (x .or. y?=w3141:bool)
        n1846 = To Double Precision Float(number=w3157) -> (double precision float=w3151:dbl)
        n1847 = Build Array(w3141, "Save Calibration", w3154, w3146) -> (w3156:bool[])
        n1848 = Compound Arithmetic op=OR("Save Calibration", w3154, w3141, w3146) -> (w3159:bool)
        n1849 = Boolean Array To Number(Boolean array=w3156) -> (number=w3153:u32)
        n1850 = feedback #19(FALSE ("Save APD Data\nwith Trap Data")) -> (w3135:bool)
        n1851 = feedback #20(refnum<k0> refnum) -> (w3162:refnum<file>)
        n1852 = feedback #21(refnum<k0> refnum) -> (w3137:refnum<file>)
        n1853 = feedback #22(FALSE ("Save APD Data\nwith Trap Data")) -> (w3145:bool)
        n1854 = feedback #23(refnum<k0> refnum) -> (w3148:refnum<file>)
        n1855 = feedback #24(0) -> (w3164:i32)
        n1856 = feedback #25() -> (w3152:u32)  [unwired: 1 out]
        n1857 = case shown="False" w3159 {
          tunnel: [w3171 1] -> w3160
          tunnel: w3164 -> [w3173 _]
          tunnel: [w3172 w3191] -> w3161
          tunnel: w3162 -> [w3172 _]
          tunnel: w3158 -> [_ w3211]
          tunnel: w3151 -> [_ w3209]
          tunnel: w3153 -> [_ w3212]
          tunnel: [w3170 w3190] -> w3150
          tunnel: w3152 -> [w3170 _]
          tunnel: [w3169 w3188] -> w3147
          tunnel: w3148 -> [w3169 _]
          tunnel: [w3168 w3187] -> w3144
          tunnel: w3145 -> [w3168 _]
          tunnel: "Start Saving" -> [_ w3185]
          tunnel: w3140 -> [_ w3184]
          tunnel: [w3167 w3175] -> w3133
          tunnel: w3137 -> [w3167 _]
          tunnel: [w3166 w3174] -> w3134
          tunnel: w3135 -> [w3166 _]
          frame False {
            n1858 = Increment(x=w3173) -> (x+1=w3171:i32)
          }
          frame True {
            w3181 = FALSE ("Start Saving")
            w3186 = 9.0  # File Version
            w3194 = FALSE ("prepend array or string size? (T)")
            w3192 = T29."big-endian, network order" ("byte order (0:big-endian, network order)")
            # "write file headers"
            n1859 = local read "BD 1 Frequency 1 (MHz)"() -> (w3208:dbl)
            n1860 = local read "BD 2 Frequency 1 (MHz)"() -> (w3207:dbl)
            n1861 = local read "BD 1 Frequency 2 (MHz)"() -> (w3206:dbl)
            n1862 = local read "BD 2 Frequency 2 (MHz)"() -> (w3205:dbl)
            n1863 = local read "BD 1 Frequency 3 (MHz)"() -> (w3204:dbl)
            n1864 = local read "BD 2 Frequency 3 (MHz)"() -> (w3203:dbl)
            n1865 = Array Size(array=w3184) -> (size(s)=w3183:i32)
            n1866 = To Double Precision Float(number=w3183) -> (double precision float=w3182:dbl)
            n1867 = local write "Save Calibration"(w3181) -> ()
            n1868 = local write "Start Saving"(w3181) -> ()
            n1869 = Build Array("Save APD Data\nwith Trap Data", "Save Trap Pos. Data") -> (w3178:bool[])
            n1870 = Boolean Array To Number(Boolean array=w3178) -> (number=w3177:u32)
            n1871 = Build Array(w3208, w3207, w3206, w3205, w3204, w3203) -> (w3202:dbl[])
            n1872 = case shown="4" w3212 {
              tunnel: w3211 -> [w3283 w3303 w3319 w3357]
              tunnel: w3182 -> [w3288 w3310 w3339 w3376]
              tunnel: w3209 -> [w3287 w3309 w3338 w3375]
              tunnel: [w3284 w3305 w3330 w3367] -> w3200
              tunnel: [w3275 "Cal sets to save" w3320 w3358] -> w3190
              tunnel: w3202 -> [w3285 w3306 w3332 w3369]
              tunnel: "Save APD Data\nwith Trap Data" -> [w3282 _ w3316 w3355]
              tunnel: [w3282 w3297 w3316 w3355] -> w3187
              tunnel: w3186 -> [w3278 w3298 w3314 w3353]
              tunnel: w3185 -> [w3277 _ _ _]
              tunnel: [w3268 w3297 w3313 w3343] -> w3174
              tunnel: "Save Trap Pos. Data" -> [w3268 _ w3313 w3343]
              tunnel: w3177 -> [w3267 _ w3312 w3342]
              frame 1, Default {
                # "timeseries"
                n1873 = case shown="True" "Profile" {
                  tunnel: [w3291 w3294] -> w3272
                  tunnel: [w3291 w3293] -> w3271
                  tunnel: [w3291 w3292] -> w3270
                  tunnel: [w3291 w3296] -> w3269
                  frame False {
                    w3291 = 0.0 ("f")
                  }
                  frame True {
                    n1874 = local read "Current Position"() -> (w3295:dbl[])
                    n1875 = local read "Y change (mm)"() -> (w3296:dbl)
                    n1876 = call "subVI_explode3array.vi"("Array"=w3295) -> ("x"=w3294:dbl, "y"=w3293:dbl, "z"=w3292:dbl)  [unwired: 12 in]
                  }
                }
                n1877 = local read "Save ave N"() -> (w3290:dbl)
                n1878 = Multiply(x=w3290, y=w3283) -> (x*y=w3289:dbl)
                n1879 = To Double Precision Float(number=w3267) -> (double precision float=w3281:dbl)
                n1880 = Build Array(w3278, w3283, w3289, w3288, w3287, 0.0 ("f")) -> (w3286:dbl[])
                n1881 = Build Array(w3281, w3272, w3271, w3270, w3269) -> (w3279:dbl[])
                n1882 = Select(t=u32 4000000000, s=w3277, f="N sets to save") -> (s? t:f=w3275:u32)
                n1883 = Build Array (concatenate)(w3286, w3285, w3279) -> (w3284:dbl[])
              }
              frame 2 {
                w3300 = 0.0 ("f")
                w3297 = FALSE ("Save APD Data\nwith Trap Data")
                # "calibration"
                n1884 = Boolean To (0,1)(Boolean=w3297) -> (0, 1=w3302:i16)
                n1885 = To Double Precision Float(number=w3302) -> (double precision float=w3301:dbl)
                n1886 = Build Array(w3301, w3300, w3300, w3300, w3300) -> (w3299:dbl[])
                n1887 = Build Array(w3298, w3303, w3303, w3310, w3309, 1.0 ("t")) -> (w3307:dbl[])
                n1888 = Build Array (concatenate)(w3307, w3306, w3299) -> (w3305:dbl[])
                "Calibrating Trap..." <- TRUE ("Calibrating...")
              }
              frame 4 {
                w3317 = 0.0 ("f")
                # "write file header for a trap \nraster scan"
                # "scan dir (x/y = 0/1)"
                # "cycles/step"
                # "n scans (f/b)"
                # "steps"
                # "freq. range"
                # "AOD raster scan"
                n1889 = local read "Number of F/B Scans (AOD)"() -> (w3324:u16)
                n1890 = local read "Cycles/step (AOD)"() -> (w3326:u64)
                n1891 = local read "Scan Range (MHz)"() -> (w3329:dbl)
                n1892 = local read "Scan steps (AOD)"() -> (w3328:u64)
                n1893 = local read "Scan BD"() -> (w3336:bool)
                n1894 = local read "Save ave N"() -> (w3341:dbl)
                n1895 = Boolean To (0,1)(Boolean=w3336) -> (0, 1=w3335:i16)
                n1896 = To Double Precision Float(number=w3324) -> (double precision float=w3323:dbl)
                n1897 = To Double Precision Float(number=w3328) -> (double precision float=w3327:dbl)
                n1898 = To Double Precision Float(number=w3326) -> (double precision float=w3325:dbl)
                n1899 = To Double Precision Float(number=w3335) -> (double precision float=w3334:dbl)
                n1900 = Multiply(x=w3341, y=w3319) -> (x*y=w3340:dbl)
                n1901 = To Double Precision Float(number=w3312) -> (double precision float=w3318:dbl)
                n1902 = Build Array(w3318, w3317, w3317, w3317, w3317) -> (w3315:dbl[])
                n1903 = local read "N sets should be saved"() -> (w3321:dbl)
                n1904 = Build Array(w3334, w3329, w3327, w3325, w3323) -> (w3331:dbl[])
                n1905 = Build Array(w3314, w3319, w3340, w3339, w3338, 2.0 ("t")) -> (w3333:dbl[])
                n1906 = Round Toward +Infinity(x=w3321) -> (ceil(x): smallest int >= x=w3322:dbl)
                n1907 = Build Array (concatenate)(w3333, w3332, w3315, w3331) -> (w3330:dbl[])
                n1908 = To Unsigned Long Integer(number=w3322) -> (unsigned 32bit integer=w3320:u32)
              }
              frame 8 {
                w3350 = 0.0 ("f")
                # "MCL raster scan"
                n1909 = local read "Number of scans (MCL)"() -> (w3345:u64)
                n1910 = local read "Scan lines (y)"() -> (w3344:u64)
                n1911 = local read "2D or 1D Scan"() -> (w3347:bool)
                n1912 = local read "Scan Range (V)\n(of steps)"() -> (w3366:dbl)
                n1913 = local read "Fast Scan Dir"() -> (w3373:bool)
                n1914 = local read "Cycles/step (MCL)"() -> (w3363:u64)
                n1915 = local read "Scan steps (MCL)"() -> (w3365:u64)
                n1916 = Select(t=w3344, s=w3347, f=w3345) -> (s? t:f=w3346:u64)
                n1917 = Boolean To (0,1)(Boolean=w3347) -> (0, 1=w3349:i16)
                n1918 = local read "Save ave N"() -> (w3378:dbl)
                n1919 = local read "Initial X"() -> (w3352:dbl)
                n1920 = local read "Initial Y"() -> (w3351:dbl)
                n1921 = To Double Precision Float(number=w3349) -> (double precision float=w3348:dbl)
                n1922 = Boolean To (0,1)(Boolean=w3373) -> (0, 1=w3372:i16)
                n1923 = To Double Precision Float(number=w3346) -> (double precision float=w3361:dbl)
                n1924 = To Double Precision Float(number=w3365) -> (double precision float=w3364:dbl)
                n1925 = To Double Precision Float(number=w3363) -> (double precision float=w3362:dbl)
                n1926 = To Double Precision Float(number=w3372) -> (double precision float=w3371:dbl)
                n1927 = Multiply(x=w3378, y=w3357) -> (x*y=w3377:dbl)
                n1928 = To Double Precision Float(number=w3342) -> (double precision float=w3356:dbl)
                n1929 = local read "N sets should be saved (MCL)"() -> (w3359:dbl)
                n1930 = Build Array(w3356, w3348, w3350, w3350, w3350) -> (w3354:dbl[])
                n1931 = Build Array(w3371, w3366, w3364, w3362, w3361, w3352, w3351) -> (w3368:dbl[])
                n1932 = Build Array(w3353, w3357, w3377, w3376, w3375, 3.0 ("t")) -> (w3370:dbl[])
                n1933 = Round Toward +Infinity(x=w3359) -> (ceil(x): smallest int >= x=w3360:dbl)
                n1934 = Build Array (concatenate)(w3370, w3369, w3354, w3368) -> (w3367:dbl[])
                n1935 = To Unsigned Long Integer(number=w3360) -> (unsigned 32bit integer=w3358:u32)
              }
            }
            n1936 = local read "Index"() -> (w3217:dbl)
            n1937 = call "Create new save file.vi"("Insert"="", "Ext"=".dat", "Index In"=w3217) -> ("Path Out"=w3176:path, "Index Out"=w3189:dbl)
            n1938 = local write "Save file name"(w3176) -> ()
            n1939 = local write "Index"(w3189) -> ()
            n1940 = local write "Save index"(w3189) -> ()
            n1941 = Array Size(array=w3200) -> (size(s)=w3201:i32)
            n1942 = Open/Create/Replace File(file path (use dialog)=w3176, operation (0:open)=T23."create", access (0:read/write)=enum16{"read/write", "read-only", "write-only"}."write-only") -> (refnum out=w3214:refnum<file>)  [unwired: 1 in, 4 out]
            n1943 = local write "Saving..."(TRUE ("Saving...")) -> ()
            n1944 = To Double Precision Float(number=w3201) -> (double precision float=w3199:dbl)
            n1945 = String Length(string="Comment (data description)") -> (length=w3197:i32)
            n1946 = To Double Precision Float(number=w3197) -> (double precision float=w3196:dbl)
            n1947 = Deny Access(7:w3214) -> (3:w3213:refnum<file>)  [unwired: 1 in, 2 out]
            n1948 = Build Array (concatenate)(w3199, w3200, w3196) -> (w3198:dbl[])
            n1949 = case "If fluorescence data to be saved" shown="True" w3187 {
              tunnel: w3176 -> [_ w3266]
              tunnel: [refnum<k0> refnum w3246] -> w3188
              frame False {
              }
              frame True {
                w3245 = 0.0
                n1950 = local read "APD Integration Time (s)"() -> (w3251:dbl)
                n1951 = local read "N APD Samp/step"() -> (w3244:dbl)
                n1952 = Path To String(path=w3266) -> (string=w3265:string)
                n1953 = String Length(string=w3265) -> (length=w3264:i32)
                n1954 = Subtract(x=w3264, y=4) -> (x-y=w3262:i32)
                n1955 = String Subset(string=w3265, length (rest)=w3262) -> (substring=w3261:string)  [unwired: 1 out]
                n1956 = Build Array(w3251, w3244, w3245, w3245, w3245, w3245, w3245, w3245) -> (w3248:dbl[])
                n1957 = Concatenate Strings(w3261, "_fl.dat" ("string")) -> (w3259:string)
                n1958 = Array Size(array=w3248) -> (size(s)=w3250:i32)
                n1959 = String To Path(string=w3259) -> (path=w3255:path)
                n1960 = Open/Create/Replace File(file path (use dialog)=w3255, operation (0:open)=T23."create", access (0:read/write)=enum16{"read/write", "read-only", "write-only"}."write-only") -> (refnum out=w3256:refnum<file>)  [unwired: 1 in, 4 out]
                n1961 = Deny Access(7:w3256) -> (3:w3252:refnum<file>)  [unwired: 1 in, 2 out]
                n1962 = To Double Precision Float(number=w3250) -> (double precision float=w3249:dbl)
                n1963 = Build Array (concatenate)(w3249, w3248) -> (w3247:dbl[])
                n1964 = Write to Binary File(file (use dialog)=w3252, data=w3247, 5:FALSE ("prepend array or string size? (T)"), 9:T29."big-endian, network order" ("byte order (0:big-endian, network order)")) -> (refnum out=w3246:refnum<file>)  [unwired: 1 in, 3 out]
              }
            }
            n1965 = case shown="True" w3174 {
              tunnel: w3176 -> [_ w3228]
              tunnel: [refnum<k0> refnum w3227] -> w3175
              frame False {
              }
              frame True {
                w3223 = 0.0 ("element")
                n1966 = Path To String(path=w3228) -> (string=w3242:string)
                n1967 = Build Array(w3223, w3223, w3223, w3223, w3223, w3223, w3223, w3223) -> (w3224:dbl[])
                n1968 = String Length(string=w3242) -> (length=w3241:i32)
                n1969 = Subtract(x=w3241, y=4) -> (x-y=w3239:i32)
                n1970 = Array Size(array=w3224) -> (size(s)=w3226:i32)
                n1971 = String Subset(string=w3242, length (rest)=w3239) -> (substring=w3238:string)  [unwired: 1 out]
                n1972 = To Double Precision Float(number=w3226) -> (double precision float=w3225:dbl)
                n1973 = Concatenate Strings(w3238, "_pos.dat" ("string")) -> (w3236:string)
                n1974 = Build Array (concatenate)(w3225, w3224) -> (w3222:dbl[])
                n1975 = String To Path(string=w3236) -> (path=w3232:path)
                n1976 = Open/Create/Replace File(file path (use dialog)=w3232, operation (0:open)=T23."create", access (0:read/write)=enum16{"read/write", "read-only", "write-only"}."write-only") -> (refnum out=w3233:refnum<file>)  [unwired: 1 in, 4 out]
                n1977 = Deny Access(7:w3233) -> (3:w3229:refnum<file>)  [unwired: 1 in, 2 out]
                n1978 = Write to Binary File(file (use dialog)=w3229, data=w3222, 5:FALSE ("prepend array or string size? (T)"), 9:T29."big-endian, network order" ("byte order (0:big-endian, network order)")) -> (refnum out=w3227:refnum<file>)  [unwired: 1 in, 3 out]
              }
            }
            n1979 = Write to Binary File(file (use dialog)=w3213, data=w3198, 5:w3194, 9:w3192) -> (refnum out=w3195:refnum<file>)  [unwired: 1 in, 3 out]
            n1980 = Write to Binary File(file (use dialog)=w3195, data="Comment (data description)", 5:w3194, 9:w3192) -> (refnum out=w3191:refnum<file>)  [unwired: 1 in, 3 out]
          }
        }
        n1981 = feedback-in #19(w3134) -> ()
        n1982 = feedback-in #20(w3161) -> ()
        n1983 = feedback-in #21(w3133) -> ()
        n1984 = feedback-in #22(w3144) -> ()
        n1985 = feedback-in #23(w3147) -> ()
        n1986 = feedback-in #24(w3160) -> ()
        n1987 = feedback-in #25(w3150) -> ()
      }
      frame #1 {
        n1988 = local read "Saving..."() -> (w3391:bool)
        n1989 = case shown="True" w3391 {
          tunnel: w3395 -> [_ w3405]
          tunnel: w3394 -> [_ w3419]
          tunnel: w3393 -> [_ w3415]
          tunnel: w3392 -> [_ w3414]
          tunnel: w3390 -> [_ w3413]
          tunnel: w3389 -> [_ w3408]
          tunnel: w3388 -> [_ w3407]
          tunnel: w3387 -> [_ w3406]
          tunnel: w3386 -> [_ w3404]
          tunnel: w3385 -> [_ w3402]
          tunnel: w3384 -> [_ w3401]
          tunnel: w3383 -> [_ w3400]
          tunnel: w3382 -> [_ w3399]
          tunnel: w3381 -> [_ w3398]
          tunnel: w3380 -> [_ w3397]
          tunnel: w3379 -> [_ w3396]
          frame False {
          }
          frame True {
            n1990 = Multiply(x=w3405, y=w3404) -> (x*y=→"Time (s)":dbl)
            n1991 = Less Or Equal?(x=w3405, y=w3413) -> (x <= y?=w3417:bool)
            n1992 = Or(x="Stop Saving", y="Abort save 2") -> (x .or. y?=w3409:bool)
            n1993 = Not(x=w3409) -> (.not. x?=w3418:bool)
            n1994 = And(x=w3417, y=w3418) -> (x .and. y?=w3416:bool)
            n1995 = case shown="False" w3416 {
              tunnel: w3419 -> [w3426 w3494]
              tunnel: [0.0 w3497] -> w3412
              tunnel: w3405 -> [_ w3495]
              tunnel: w3413 -> [_ w3496]
              tunnel: w3415 -> [_ w3491]
              tunnel: w3414 -> [_ _]
              tunnel: w3408 -> [w3424 w3484]
              tunnel: w3407 -> [w3423 w3485]
              tunnel: w3406 -> [_ w3483]
              tunnel: w3402 -> [_ w3482]
              tunnel: w3401 -> [_ w3436]
              tunnel: w3400 -> [_ w3475]
              tunnel: w3399 -> [_ w3453]
              tunnel: w3398 -> [w3421 w3434]
              tunnel: w3397 -> [w3422 w3433]
              tunnel: w3396 -> [_ w3430]
              frame False {
                w3420 = FALSE
                n1996 = Close File(refnum=w3426) -> ()  [unwired: 1 in, 2 out]
                n1997 = case shown="True" w3423 {
                  tunnel: w3424 -> [_ w3428]
                  frame False {
                  }
                  frame True {
                    n1998 = Close File(refnum=w3428) -> ()  [unwired: 1 in, 2 out]
                  }
                }
                n1999 = case shown="True" w3421 {
                  tunnel: w3422 -> [_ w3427]
                  frame False {
                  }
                  frame True {
                    n2000 = Close File(refnum=w3427) -> ()  [unwired: 1 in, 2 out]
                  }
                }
                n2001 = local write "Calibrating Trap..."(w3420) -> ()
                n2002 = call <vilib>:"Beep.vi"() -> ()  [unwired: 3 in, 9 out]
                n2003 = local write "Stop Saving"(w3420) -> ()
                n2004 = property on="Raster Scanning..." class="Bool (strict)"("Val(Sgnl)"=w3420) -> ()  [unwired: 2 in, 2 out]
                "Saving..." <- w3420
              }
              frame True {
                n2005 = local read "Calibrating Trap..."() -> (w3486:bool)
                n2006 = case "Write fl. data" shown="True" w3485 {
                  tunnel: w3484 -> [_ w3520]
                  tunnel: w3483 -> [_ w3519]
                  frame False {
                  }
                  frame True {
                    n2007 = Write to Binary File(file (use dialog)=w3520, data=w3519, 5:FALSE ("prepend array or string size? (T)"), 9:T29."big-endian, network order" ("byte order (0:big-endian, network order)")) -> ()  [unwired: 1 in, 4 out]
                  }
                }
                n2008 = Greater?(x="Save ave N", y=1.0) -> (0:w3489:bool)
                n2009 = Not(x=w3486) -> (.not. x?=w3488:bool)
                n2010 = And(x=w3488, y=w3489) -> (x .and. y?=w3431:bool)
                n2011 = case shown="True" w3431 {
                  tunnel: w3430 -> [w3500 w3511]
                  tunnel: [w3500 w3503] -> w3429
                  tunnel: "Save ave N" -> [_ w3504]
                  frame False {
                  }
                  frame True {
                    w3501 = 2 ("dimension size")
                    n2012 = Array Size(array=w3511) -> (size(s)=w3505:i32)
                    n2013 = Divide(x=w3505, y=w3501) -> (x/y=w3509:dbl)
                    n2014 = Reshape Array(w3511, w3509, w3501) -> (w3510:u64[][])
                    n2015 = Transpose 2D Array(2D array=w3510) -> (transposed array=w3508:u64[][])
                    n2016 = for {
                      tunnel: w3508 -> [w3513] mode=indexing
                      tunnel: [w3512] -> w3502 mode=indexing
                      tunnel: w3504 -> [w3514]
                      workers-P: _ -> [_]
                      n2017 = call "downsample 1D array - U64.vi"("Ave N"=w3514, "Array In"=w3513) -> ("Array Out"=w3512:u64[])  [unwired: 1 in]
                    }
                    n2018 = Transpose 2D Array(2D array=w3502) -> (transposed array=w3507:u64[][])
                    n2019 = Divide(x=w3505, y=w3504) -> (x/y=w3506:dbl)
                    n2020 = Reshape Array(w3507, w3506) -> (w3503:u64[])
                  }
                }
                n2021 = case shown="True" w3431 {
                  tunnel: w3491 -> [w3523 w3535]
                  tunnel: [w3523 w3527] -> w3487
                  tunnel: "Save ave N" -> [_ w3528]
                  tunnel: w3482 -> [_ w3526]
                  frame False {
                    # "don't downsample data for trap calibration"
                  }
                  frame True {
                    n2022 = Array Size(array=w3535) -> (size(s)=w3529:i32)
                    n2023 = Array Size(array=w3526) -> (size(s)=w3525:i32)
                    n2024 = Divide(x=w3529, y=w3525) -> (x/y=w3533:dbl)
                    n2025 = Reshape Array(w3535, w3533, w3525) -> (w3534:i16[][])
                    n2026 = Transpose 2D Array(2D array=w3534) -> (transposed array=w3532:i16[][])
                    n2027 = for {
                      tunnel: w3532 -> [w3538] mode=indexing
                      tunnel: [w3537] -> w3524 mode=indexing
                      tunnel: w3528 -> [w3536]
                      workers-P: _ -> [_]
                      n2028 = call "downsample 1D array - I16.vi"("Ave N"=w3536, "Array In"=w3538) -> ("Array Out"=w3537:i16[])  [unwired: 1 out]
                    }
                    n2029 = Transpose 2D Array(2D array=w3524) -> (transposed array=w3531:i16[][])
                    n2030 = Divide(x=w3529, y=w3528) -> (x/y=w3530:dbl)
                    n2031 = Reshape Array(w3531, w3530) -> (w3527:i16[])
                  }
                }
                n2032 = Index Array(array=w3453, index=1) -> (element=w3456:waveform(dbl))
                n2033 = Index Array(array=w3453, index=0) -> (element=w3458:waveform(dbl))
                n2034 = Unbundle By Name(w3456) -> ("Y"=w3460:dbl[])
                n2035 = Unbundle By Name(w3458) -> ("Y"=w3468:dbl[])
                n2036 = case "Write trap pos. data" shown="True" w3434 {
                  tunnel: w3433 -> [_ w3516]
                  tunnel: w3429 -> [_ w3515]
                  frame False {
                  }
                  frame True {
                    n2037 = Write to Binary File(file (use dialog)=w3516, data=w3515, 5:FALSE ("prepend array or string size? (T)"), 9:T29."big-endian, network order" ("byte order (0:big-endian, network order)")) -> ()  [unwired: 1 in, 4 out]
                  }
                }
                n2038 = Write to Binary File(file (use dialog)=w3494, data=w3487, 5:FALSE ("prepend array or string size? (T)"), 9:T29."big-endian, network order" ("byte order (0:big-endian, network order)")) -> ()  [unwired: 1 in, 4 out]
                n2039 = feedback #26(w3460) -> (w3462:dbl[])
                n2040 = Build Array (concatenate)(w3462, w3460) -> (w3461:dbl[])
                n2041 = Select(t=w3460, s=w3436, f=w3461) -> (s? t:f=w3446:dbl[])
                n2042 = feedback-in #26(w3446) -> ()
                n2043 = feedback #27(w3468) -> (w3481:dbl[])
                n2044 = Build Array (concatenate)(w3481, w3468) -> (w3480:dbl[])
                n2045 = Select(t=w3468, s=w3436, f=w3480) -> (s? t:f=w3455:dbl[])
                n2046 = feedback-in #27(w3455) -> ()
                n2047 = Divide(x=w3495, y=w3496) -> (x/y=w3498:dbl)
                n2048 = Multiply(x=w3498, y=100.0) -> (x*y=w3497:dbl)
                n2049 = Build Array(w3455, w3446) -> (→"Saved APD":dbl[][])
                n2050 = Array Size(array=w3455) -> (size(s)=w3473:i32)
                n2051 = Unbundle By Name(w3475) -> ("Y"=w3479:dbl[])
                n2052 = Subtract(x=w3473, y="N pts to average") -> (x-y=w3449:i32)
                n2053 = Multiply(x="N pts to average", y=u16 2) -> (x*y=w3450:u16)
                n2054 = Subtract(x=w3473, y=w3450) -> (x-y=w3448:i32)
                n2055 = feedback #28(w3479) -> (w3478:dbl[])
                n2056 = Build Array (concatenate)(w3478, w3479) -> (w3477:dbl[])
                n2057 = Select(t=w3479, s=w3436, f=w3477) -> (s? t:f=w3476:dbl[])
                "Trap Delta Graph" <- w3476
                n2058 = feedback-in #28(w3476) -> ()
                n2059 = Array Subset(array=w3455, index=w3449, length="N pts to average") -> (w3472:dbl[])
                n2060 = Array Subset(array=w3455, index=w3448, length="N pts to average") -> (w3471:dbl[])
                n2061 = Array Subset(array=w3446, index=w3449, length="N pts to average") -> (w3452:dbl[])
                n2062 = Array Subset(array=w3446, index=w3448, length="N pts to average") -> (w3451:dbl[])
                n2063 = call-poly <vilib>:"Mean.vi"("X"=w3472) -> ("mean"=w3470:dbl)  [unwired: 1 out]
                n2064 = call-poly <vilib>:"Mean.vi"("X"=w3452) -> ("mean"=w3445:dbl)  [unwired: 1 out]
                n2065 = call-poly <vilib>:"Mean.vi"("X"=w3471) -> ("mean"=w3469:dbl)  [unwired: 1 out]
                n2066 = call-poly <vilib>:"Mean.vi"("X"=w3451) -> ("mean"=w3444:dbl)  [unwired: 1 out]
                n2067 = Subtract(x=w3445, y=w3444) -> (x-y=w3435:dbl)
                "Delta Fl. 2" <- w3435
                n2068 = Subtract(x=w3470, y=w3469) -> (x-y=w3467:dbl)
                "Delta Fl. 1" <- w3467
                n2069 = Initialize Array(w3467, 1 ("dimension size")) -> (w3464:dbl[])
                n2070 = Initialize Array(w3435, 1 ("dimension size")) -> (w3441:dbl[])
                n2071 = feedback #29(w3464) -> (w3465:dbl[])
                n2072 = Build Array (concatenate)(w3465, w3464) -> (w3463:dbl[])
                n2073 = feedback #30(w3441) -> (w3442:dbl[])
                n2074 = Build Array (concatenate)(w3442, w3441) -> (w3440:dbl[])
                n2075 = Select(t=w3464, s=w3436, f=w3463) -> (s? t:f=w3439:dbl[])
                n2076 = feedback-in #29(w3439) -> ()
                n2077 = Select(t=w3441, s=w3436, f=w3440) -> (s? t:f=w3438:dbl[])
                n2078 = feedback-in #30(w3438) -> ()
                n2079 = Build Array(w3439, w3438) -> (→"Save APD Deriv":dbl[][])
              }
            }
            "Progress" <- w3412
            "Progress 2" <- w3412
          }
        }
      }
    }
    n2080 = Bundle By Name(cluster=w2156, "Green FB Ch 0"=w2155, "Green FB Ch 1"=w2154) -> (w2134:T48)
    "Green FB Signals (V)" <- w2134
    n2081 = Unbundle By Name(w2134) -> ("Green FB Ch 2"=→"Green FB Plot":dbl)
    n2082 = local read "wait to reset values"() -> (w2226:bool)
    n2083 = Not(x=w2223) -> (.not. x?=w2227:bool)
    n2084 = And(x=w2227, y=w2226) -> (x .and. y?=w2228:bool)
    n2085 = case "Part of MCL raster scanning: returns to initial positions after scan done" shown="False" w2228 {
      tunnel: w2231 -> [w2964 w2971]
      tunnel: [w2964 w2970] -> w2230
      tunnel: w2225 -> [w2963 w2969]
      tunnel: [w2963 w2968] -> w2224
      frame False {
      }
      frame True {
        w2979 = 10.0 ("y")
        w2978 = 32767.0 ("y")
        # "to return scan values\nafter a synchronous \nAOM scan"
        n2086 = local read "AO2"() -> (w2972:dbl)
        n2087 = local read "AO1"() -> (w2973:dbl)
        n2088 = local write "wait to reset values"(FALSE ("wait to reset values")) -> ()
        n2089 = Multiply(x=w2973, y=w2978) -> (x*y=w2975:dbl)
        n2090 = Multiply(x=w2972, y=w2978) -> (x*y=w2977:dbl)
        n2091 = Divide(x=w2975, y=w2979) -> (x/y=w2974:dbl)
        n2092 = Divide(x=w2977, y=w2979) -> (x/y=w2976:dbl)
        n2093 = To Word Integer(number=w2974) -> (16bit integer=w2980:i16)
        n2094 = To Word Integer(number=w2976) -> (16bit integer=w2981:i16)
        n2095 = local read "Total Counts (ticks)"() -> (w2965:u32)
        n2096 = xnode "Read/Write Control"("FPGA VI Reference In"=w2971, "error in"=w2969, "AO1"=w2980, "AO2"=w2981, "MCL count"=w2965) -> ("FPGA VI Reference Out"=w2970:T19, "error out"=w2968:errorcluster)
        n2097 = local read "Scan Range (V)\n(of steps)"() -> (w2966:dbl)
        n2098 = property on="Scan Range (V)\n(of steps)" class="DigNum (strict)"("Val(Sgnl)"=w2966) -> ()  [unwired: 2 in, 2 out]
      }
    }
    n2099 = node-c288() -> ()  [unwired: 2 out]
  }
  n2100 = node-c288(3 ("Processor")) -> (w74:T24)  [unwired: 3 out]
  n2101 = timed-loop "Oscillate AOD (debugging)" {
    tunnel: w24 -> [w3540]
    tunnel: [w3539] -> w36
    timing: w74 -> [_]
    timing-out: [_] -> w73
    stop <- w3539 stop-if-true
    n2102 = node-c288() -> ()  [unwired: 2 out]
    n2103 = event shown="[0] \"Oscillate Set 2\", \"Fish for Tether\": Value Change" {
      selector: _ -> [_ _ _]
      dyn-events: _ -> [_ _ _]
      timeout: _ -> [_ _ _]
      tunnel: w3540 -> [w3547 _ _]
      tunnel: [FALSE ("Stop All") _ w3815] -> w3539
      event "Oscillate Set 2", "Fish for Tether": Value Change {
        n2104 = event-data() -> ()  [unwired: 6 out]
        n2105 = local read "Oscillate Set 2"() -> (w3546:bool)
        n2106 = Or(x=w3546, y="Fish for Tether") -> (x .or. y?=w3544:bool)
        n2107 = case shown="True" w3544 {
          tunnel: w3547 -> [_ w3550]
          tunnel: "Fish for Tether" -> [_ w3549]
          frame False {
          }
          frame True {
            n2108 = case shown="True" w3549 {
              frame False {
              }
              frame True {
                n2109 = local write "Scan axis 2"(TRUE) -> ()
                n2110 = local write "Tether"(FALSE ("Tether")) -> ()
              }
            }
            n2111 = node-c288("Period") -> (w3552:T24)  [unwired: 3 out]
            n2112 = timed-loop "Oscillate AOD" {
              timing: w3552 -> [_]
              timing-out: [_] -> w3551
              tunnel: w3550 -> [w3562]
              tunnel: w3549 -> [w3561]
              i -> [w3564]
              stop <- w3560 stop-if-true
              n2113 = node-c288() -> (w3563:i64)  [unwired: 1 out]
              n2114 = flat-sequence {
                tunnel: w3564 -> [w3590]
                tunnel: w3563 -> [w3589]
                tunnel: w3562 -> [w3573]
                tunnel: w3561 -> [w3575]
                tunnel: [w3575] -> w3559
                tunnel: [w3574] -> w3558
                tunnel: [w3572] -> w3557
                tunnel: [w3569] -> w3555
                tunnel: w3559 -> [w3626]
                tunnel: w3558 -> [w3624]
                tunnel: w3557 -> [w3623]
                tunnel: [w3622] -> w3556
                tunnel: w3555 -> [w3621]
                tunnel: [w3690] -> w3560
                tunnel: w3556 -> [w3688]
                frame #0 {
                  n2115 = Divide(x=w3589, y=i64 1000) -> (x/y=w3584:dbl)
                  n2116 = Multiply(x=w3584, y=w3590) -> (x*y=w3586:dbl)
                  n2117 = Multiply(x="Osc. freq. (Hz)", y=6.283185307179586) -> (x*y=w3587:dbl)
                  n2118 = Multiply(x=w3587, y=w3586) -> (x*y=w3571:dbl)
                  n2119 = local read "BD 1 Frequency 2 (MHz)"() -> (w3568:dbl)
                  n2120 = local read "BD 1 Frequency 1 (MHz)"() -> (w3565:dbl)
                  n2121 = case shown="True" w3575 {
                    tunnel: w3571 -> [w3596 w3603]
                    tunnel: w3568 -> [_ w3613]
                    tunnel: [w3593 w3597] -> w3576
                    tunnel: [FALSE w3606] -> w3572
                    tunnel: [0.0 w3599] -> w3569
                    tunnel: w3565 -> [_ w3598]
                    frame False {
                      n2122 = Sine(x=w3596) -> (sin(x)=w3594:dbl)
                      n2123 = Multiply(x=w3594, y="Osc. amp. (MHz)") -> (x*y=w3593:dbl)
                    }
                    frame True {
                      n2124 = Cosine(x=w3603) -> (cos(x)=w3616:dbl)
                      n2125 = Subtract(x=w3613, y=w3598) -> (x-y=w3612:dbl)
                      n2126 = Decrement(x=w3616) -> (x-1=w3615:dbl)
                      n2127 = Subtract(x=w3612, y="Closest Delta (MHz)") -> (x-y=w3609:dbl)
                      n2128 = Divide(x=w3615, y=2.0) -> (x/y=w3610:dbl)
                      n2129 = Multiply(x=w3610, y=w3609) -> (x*y=w3597:dbl)
                      n2130 = local read "Vec Mean of T1 T2"() -> (w3605:dbl[])
                      n2131 = Greater?(x=w3605, y="Stop F (pN)") -> (0:w3607:bool[])
                      n2132 = Or Array Elements(Boolean array=w3607) -> (logical OR=w3606:bool)
                      n2133 = Divide(x=w3603, y=6.283185307179586) -> (x/y=w3602:dbl)
                      n2134 = Round Toward +Infinity(x=w3602) -> (ceil(x): smallest int >= x=w3599:dbl)
                      "Attempts" <- w3599
                      n2135 = Greater?(x=w3599, y="Attempt Limit") -> (0:w3601:bool)
                      n2136 = case shown="True" w3601 {
                        frame False {
                        }
                        frame True {
                          n2137 = local write "Fish for Tether"(FALSE ("Fish for Tether")) -> ()
                          n2138 = call <vilib>:"Beep.vi"() -> ()  [unwired: 3 in, 9 out]
                          n2139 = local read "Messages"() -> (w3618:string)
                          n2140 = call "Update messages.vi"("Message to add"="Tether fishing timeout." ("Messages"), "Old message string"=w3618) -> ("New message string"=→"Messages":string)
                        }
                      }
                    }
                  }
                  n2141 = local read "Y RF Frequency Limits (MHz)"() -> (w3577:T16)
                  n2142 = local read "X RF Frequency Limits (MHz)"() -> (w3578:T16)
                  n2143 = local read "BD 1 Frequency 3 (MHz)"() -> (w3583:dbl)
                  n2144 = local read "BD 2 Frequency 2 (MHz)"() -> (w3567:dbl)
                  n2145 = Select(t=w3568, s="Scan axis 2", f=w3567) -> (s? t:f=w3579:dbl)
                  n2146 = Add(x=w3576, y=w3579) -> (x+y=w3574:dbl)
                  n2147 = Select(t=w3574, s="Scan axis 2", f=w3568) -> (s? t:f=w3566:dbl)
                  n2148 = Select(t=w3567, s="Scan axis 2", f=w3574) -> (s? t:f=w3581:dbl)
                  n2149 = local read "BD 2 Frequency 3 (MHz)"() -> (w3582:dbl)
                  n2150 = call "set RF board frequency - interlace.vi"("Board 2 Frequency Limits"=w3577, "Board 1 Frequency Limits"=w3578, "FPGA VI Reference In"=w3573, "Board 2 Frequency 3 (MHz)"=w3582, "Board 1 Frequency 3 (MHz)"=w3583, "Board 2 Frequency 2 (MHz)"=w3567, "Board 2 Frequency 1 (MHz)"=w3581, "Board 1 Frequency 2 (MHz)"=w3566, "Board 1 Frequency 1  (MHz)"=w3565) -> ()  [unwired: 1 in, 2 out]
                }
                frame #1 {
                  n2151 = And(x=w3626, y=w3623) -> (x .and. y?=w3625:bool)
                  n2152 = case "Only if were fishing and now formed tether" shown="True" w3625 {
                    tunnel: w3624 -> [w3628 w3640]
                    tunnel: [w3627 w3639] -> w3622
                    tunnel: w3621 -> [_ w3635]
                    frame False {
                      n2153 = local read "Fish for Tether"() -> (w3627:bool)
                      n2154 = case shown="True" w3627 {
                        tunnel: w3628 -> [_ _]
                        frame False {
                        }
                        frame True {
                        }
                      }
                    }
                    frame True {
                      w3639 = FALSE ("Fish for Tether")
                      n2155 = call <vilib>:"Beep.vi"() -> ()  [unwired: 3 in, 9 out]
                      n2156 = Number To Decimal String(number=w3635, width (-)=i16 1) -> (decimal integer string=w3633:string)
                      n2157 = case shown="\"2\", \"3\", \"4\", \"5\", \"6\"" "Then..." {
                        selector: "Then..." -> [_ w3643]
                        tunnel: w3640 -> [w3642 _]
                        frame "1", Default {
                          # "do nothing"
                          n2158 = property on="BD 1 Frequency 1 (MHz)" class="DigNum (strict)"("Val(Sgnl)"=w3642) -> ()  [unwired: 2 in, 2 out]
                        }
                        frame "2", "3", "4", "5", "6" {
                          n2159 = flat-sequence {
                            tunnel: w3643 -> [w3645]
                            frame #0 {
                              n2160 = property on="Trap Delta (MHz)" class="DigNum (strict)"("Val(Sgnl)"="Move to Delta 1 (MHz)") -> ()  [unwired: 2 in, 2 out]
                            }
                            frame #1 {
                              n2161 = case shown="\"5\", \"6\"" w3645 {
                                selector: w3645 -> [w3648 w3658 _]
                                frame "3", "4" {
                                n2162 = flat-sequence {
                                tunnel: w3648 -> [w3649]
                                tunnel: [w3649] -> w3646
                                tunnel: [w3651] -> w3647
                                tunnel: w3646 -> [w3651]
                                tunnel: w3647 -> [w3655]
                                frame #0 {
                                n2163 = property on="Green Laser ON/Interlacing" class="Bool (strict)"("Val(Sgnl)"=TRUE ("Value (Signaling)")) -> ()  [unwired: 2 in, 2 out]
                                }
                                frame #1 {
                                n2164 = Multiply(x="Wait Before Save (s)", y=u32 1000 ("x")) -> (x*y=w3653:u32)
                                n2165 = Wait (ms)(milliseconds to wait=w3653) -> ()  [unwired: 1 out]
                                }
                                frame #2 {
                                n2166 = property on="Start Saving" class="Bool (strict)"("Value"=TRUE ("Start Saving")) -> ()  [unwired: 2 in, 2 out]
                                n2167 = case shown="Default" w3655 {
                                frame Default {
                                }
                                frame "4" {
                                n2168 = property on="Fl. Triggered..." class="Bool (strict)"("Val(Sgnl)"=TRUE ("Value (Signaling)")) -> ()  [unwired: 2 in, 2 out]
                                }
                                }
                                }
                                }
                                }
                                frame "5", "6" {
                                n2169 = stacked-sequence {
                                tunnel: w3658 -> [_ _ _ _ _ _ _ _ w3675 _ _]
                                frame #0 {
                                n2170 = Replace Array Subset(array=u32[] [0] ("Index Values"), new element="Raster Set Upon Tether", index=0) -> (w3659:u32[])
                                n2171 = property on="Saved AOD Raster Scan Parameter Sets" class="Arr (strict)"("Index Values"=w3659) -> ()  [unwired: 2 in, 2 out]
                                }
                                frame #1 {
                                n2172 = Wait (ms)(milliseconds to wait=u32 500) -> ()  [unwired: 1 out]
                                }
                                frame #2 {
                                n2173 = property on="Load parameters" class="Bool (strict)"("Val(Sgnl)"=TRUE ("Value (Signaling)")) -> ()  [unwired: 2 in, 2 out]
                                }
                                frame #3 {
                                n2174 = Wait (ms)(milliseconds to wait=u32 500) -> ()  [unwired: 1 out]
                                }
                                frame #4 {
                                n2175 = property on="Trap Raster Scan" class="Bool (strict)"("Val(Sgnl)"=TRUE ("Value (Signaling)")) -> ()  [unwired: 2 in, 2 out]
                                }
                                frame #5 {
                                n2176 = Wait (ms)(milliseconds to wait=u32 2000) -> ()  [unwired: 1 out]
                                }
                                frame #6 {
                                n2177 = while {
                                stop <- w3670 stop-if-true
                                n2178 = local read "Raster Scanning..."() -> (w3669:bool)
                                n2179 = local read "Saving..."() -> (w3672:bool)
                                n2180 = Wait (ms)(milliseconds to wait=u32 100) -> ()  [unwired: 1 out]
                                n2181 = Not(x=w3672) -> (.not. x?=w3671:bool)
                                n2182 = Not(x=w3669) -> (.not. x?=w3668:bool)
                                n2183 = And(x=w3671, y=w3668) -> (x .and. y?=w3670:bool)
                                }
                                }
                                frame #7 {
                                n2184 = property on="Trap Delta (MHz)" class="DigNum (strict)"("Val(Sgnl)"="Move to Delta 2 (MHz)") -> ()  [unwired: 2 in, 2 out]
                                }
                                frame #8 {
                                n2185 = local read "Tether"() -> (w3676:bool)
                                n2186 = case shown="True" w3676 {
                                tunnel: w3675 -> [_ w3677]
                                frame False {
                                }
                                frame True {
                                n2187 = flat-sequence {
                                tunnel: w3677 -> [w3679]
                                frame #0 {
                                n2188 = Wait (ms)(milliseconds to wait=u32 500) -> ()  [unwired: 1 out]
                                }
                                frame #1 {
                                n2189 = case shown="\"6\"" w3679 {
                                frame Default {
                                }
                                frame "6" {
                                n2190 = property on="Green Laser ON/Interlacing" class="Bool (strict)"("Val(Sgnl)"=TRUE ("Green Laser ON/Interlacing")) -> ()  [unwired: 2 in, 2 out]
                                }
                                }
                                }
                                frame #2 {
                                n2191 = Wait (ms)(milliseconds to wait=u32 500) -> ()  [unwired: 1 out]
                                }
                                frame #3 {
                                n2192 = local write "Start Saving"("Save at end (5, 6)") -> ()
                                }
                                }
                                }
                                }
                                }
                                frame #9 {
                                n2193 = local read "Bead Sep. Int. Time (s)"() -> (w3685:dbl)
                                n2194 = Multiply(x=w3685, y=1000.0) -> (x*y=w3684:dbl)
                                n2195 = Wait (ms)(milliseconds to wait=w3684) -> ()  [unwired: 1 out]
                                }
                                frame #10 {
                                n2196 = property on="Rescale on Mean" class="Bool (strict)"("Val(Sgnl)"=TRUE ("Value (Signaling)")) -> ()  [unwired: 2 in, 2 out]
                                }
                                }
                                }
                                frame "2", Default {
                                }
                              }
                            }
                          }
                        }
                      }
                      n2197 = Concatenate Strings("Formed tether in ", w3633, " attempt(s)." ("string")) -> (w3630:string)
                      n2198 = local read "Messages"() -> (w3637:string)
                      n2199 = local write "Fish for Tether"(w3639) -> ()
                      n2200 = call "Update messages.vi"("Message to add"=w3630, "Old message string"=w3637) -> ("New message string"=w3636:string)
                      n2201 = local write "Messages"(w3636) -> ()
                      n2202 = Get Date/Time In Seconds() -> (seconds since 1Jan1904=→"Time tether formed":timestamp)
                      "Tether" <- "Tether Alarm?"
                    }
                  }
                }
                frame #2 {
                  n2203 = local read "Oscillate Set 2"() -> (w3689:bool)
                  n2204 = local read "Stop All"() -> (w3691:bool)
                  n2205 = Not Or(1:w3688, 2:w3689) -> (0:w3687:bool)
                  n2206 = Compound Arithmetic op=OR(w3691, w3687) -> (w3690:bool)
                }
              }
              n2207 = node-c288() -> ()  [unwired: 2 out]
            }
            n2208 = node-c288(w3551) -> ()  [unwired: 1 out]
          }
        }
      }
      event "Fl. Triggered...": Value Change {
        n2209 = event-data() -> ()  [unwired: 7 out]
        n2210 = case shown="True" "Fl. Triggered..." {
          frame False {
          }
          frame True {
            n2211 = node-c288() -> (w3703:T24)  [unwired: 4 out]
            n2212 = timed-loop {
              timing: w3703 -> [_]
              timing-out: [_] -> w3702
              tunnel: "Action" -> [w3707]
              shift-right: [w3704] -> _
              shift-left: u8 255 -> [w3706]
              stop <- w3708 stop-if-true
              n2213 = node-c288() -> ()  [unwired: 2 out]
              n2214 = flat-sequence {
                tunnel: w3707 -> [w3720]
                tunnel: w3706 -> [w3717]
                tunnel: [w3716] -> w3705
                tunnel: [w3806] -> w3708
                tunnel: w3705 -> [w3805]
                tunnel: [w3805] -> w3704
                frame #0 {
                  n2215 = local read "Delta Fl. 2"() -> (w3711:dbl)
                  n2216 = local read "Delta Fl. 1"() -> (w3712:dbl)
                  n2217 = Select(t=w3712, s="APD to Watch", f=w3711) -> (s? t:f=w3710:dbl)
                  n2218 = Multiply(x="Fl. Delta Thresh. (kHz)", y=1000.0) -> (x*y=w3719:dbl)
                  n2219 = Greater?(x=w3710, y=w3719) -> (0:w3714:bool)
                  n2220 = Or(x="Force Yank", y=w3714) -> (x .or. y?=w3715:bool)
                  n2221 = case shown="True" w3715 {
                    tunnel: w3720 -> [_ w3730]
                    tunnel: w3717 -> [w3722 w3726]
                    tunnel: [w3722 w3723] -> w3716
                    frame False {
                    }
                    frame True {
                      n2222 = flat-sequence {
                        tunnel: w3727 -> [w3736]
                        tunnel: [w3736] -> w3731
                        tunnel: w3730 -> [w3735]
                        tunnel: [w3735] -> w3729
                        tunnel: [w3734] -> w3728
                        tunnel: w3726 -> [w3733]
                        tunnel: [w3732] -> w3725
                        tunnel: w3731 -> [w3761]
                        tunnel: w3729 -> [w3760]
                        tunnel: w3728 -> [w3759]
                        tunnel: w3725 -> [w3758]
                        tunnel: [w3758] -> w3724
                        tunnel: w3724 -> [w3803]
                        tunnel: [w3803] -> w3723
                        frame #0 {
                          n2223 = call <vilib>:"Beep.vi"() -> ()  [unwired: 3 in, 9 out]
                          n2224 = local write "Waiting"(FALSE ("Waiting")) -> ()
                          n2225 = Increment(x=w3733) -> (x+1=w3732:u8)
                          n2226 = case shown="\"Yank\"" w3735 {
                            tunnel: w3732 -> [_ _ w3742]
                            frame "Image" {
                              n2227 = property on="Confocal Image" class="Bool (strict)"("Val(Sgnl)"=TRUE ("Value (Signaling)")) -> ()  [unwired: 2 in, 2 out]
                            }
                            frame "Alarm", Default {
                            }
                            frame "Yank" {
                              n2228 = flat-sequence {
                                tunnel: w3742 -> [w3745]
                                tunnel: [w3744] -> w3741
                                tunnel: ["N Array El"] -> w3740
                                tunnel: w3741 -> [w3755]
                                tunnel: w3740 -> [w3751]
                                frame #0 {
                                n2229 = Multiply(x="Yank Delay (s)", y=1000.0) -> (x*y=w3748:dbl)
                                n2230 = Quotient & Remainder(x=w3745, y="N Array El") -> (x-y*floor(x/y)=w3744:u8)  [unwired: 1 out]
                                n2231 = Wait (ms)(milliseconds to wait=w3748) -> ()  [unwired: 1 out]
                                }
                                frame #1 {
                                n2232 = Random Number (0-1)() -> (number: 0 to 1=w3752:dbl)
                                n2233 = Multiply(x=w3751, y=w3752) -> (x*y=w3750:dbl)
                                n2234 = Round Toward -Infinity(1:w3750) -> (0:w3749:dbl)
                                n2235 = Select(t=w3749, s="Random Choice", f=w3755) -> (s? t:f=w3753:dbl)
                                n2236 = Index Array(array="Yank to Delta Array (MHz)", index=w3753) -> (element=w3756:dbl)
                                n2237 = property on="Trap Delta (MHz)" class="DigNum (strict)"("Val(Sgnl)"=w3756) -> ()  [unwired: 2 in, 2 out]
                                }
                              }
                            }
                          }
                          n2238 = local read "Time (s)"() -> (w3734:dbl)
                          "Fl. High" <- TRUE ("Yanking")
                        }
                        frame #1 {
                          n2239 = node-c288() -> (w3763:T24)  [unwired: 4 out]
                          n2240 = timed-loop {
                            timing: w3763 -> [_]
                            timing-out: [_] -> w3762
                            tunnel: w3761 -> [w3779]
                            tunnel: w3760 -> [w3777]
                            tunnel: w3759 -> [w3776]
                            stop <- w3778 stop-if-true
                            n2241 = node-c288() -> ()  [unwired: 2 out]
                            n2242 = local read "Fl. Delta Thresh. (kHz)"() -> (w3771:dbl)
                            n2243 = local read "Fl. Triggered..."() -> (w3780:bool)
                            n2244 = local read "Delta Fl. 1"() -> (w3767:dbl)
                            n2245 = local read "Delta Fl. 2"() -> (w3765:dbl)
                            n2246 = local read "Stop All"() -> (w3774:bool)
                            n2247 = local read "APD to Watch"() -> (w3766:bool)
                            n2248 = Select(t=w3767, s=w3766, f=w3765) -> (s? t:f=w3764:dbl)
                            n2249 = Not(x=w3780) -> (.not. x?=w3775:bool)
                            n2250 = Multiply(x=w3771, y=1000.0) -> (x*y=w3770:dbl)
                            n2251 = Negate(x=w3770) -> (-x=w3769:dbl)
                            n2252 = Less?(x=w3764, y=w3769) -> (x < y?=w3773:bool)
                            n2253 = Compound Arithmetic op=OR(w3773, w3774, w3775, "Force Reset") -> (w3778:bool)
                            n2254 = case shown="True" w3778 {
                              tunnel: w3779 -> [_ w3791]
                              tunnel: w3777 -> [_ w3790]
                              tunnel: w3776 -> [_ w3788]
                              frame False {
                              }
                              frame True {
                                n2255 = case shown="\"Yank\"" w3790 {
                                tunnel: w3791 -> [_ w3792]
                                frame "Image", Default {
                                }
                                frame "Yank" {
                                n2256 = flat-sequence {
                                tunnel: [w3797] -> w3793
                                tunnel: w3792 -> [w3797]
                                tunnel: w3793 -> [w3798]
                                frame #0 {
                                n2257 = local read "Yank Delay (s)"() -> (w3796:dbl)
                                n2258 = Multiply(x=w3796, y=1000.0) -> (x*y=w3794:dbl)
                                n2259 = Wait (ms)(milliseconds to wait=w3794) -> ()  [unwired: 1 out]
                                }
                                frame #1 {
                                n2260 = property on="Trap Delta (MHz)" class="DigNum (strict)"("Val(Sgnl)"=w3798) -> ()  [unwired: 2 in, 2 out]
                                }
                                }
                                }
                                }
                                n2261 = local read "Time (s)"() -> (w3789:dbl)
                                n2262 = Subtract(x=w3789, y=w3788) -> (x-y=w3785:dbl)
                                "Duration (s)" <- w3785
                                n2263 = Number To Decimal String(number=w3785, width (-)=i16 0) -> (decimal integer string=w3783:string)
                                n2264 = Concatenate Strings(w3783, " s fluorescence event." ("string")) -> (w3781:string)
                                n2265 = local read "Messages"() -> (w3787:string)
                                n2266 = call "Update messages.vi"("Message to add"=w3781, "Old message string"=w3787) -> ("New message string"=w3786:string)
                                n2267 = call <vilib>:"Beep.vi"() -> ()  [unwired: 3 in, 9 out]
                                n2268 = local write "Messages"(w3786) -> ()
                              }
                            }
                            n2269 = node-c288() -> ()  [unwired: 2 out]
                          }
                          n2270 = node-c288(w3762) -> ()  [unwired: 1 out]
                        }
                        frame #2 {
                          n2271 = local write "Fl. High"(FALSE ("Yanking")) -> ()
                        }
                      }
                      n2272 = local read "Trap Delta (MHz)"() -> (w3727:dbl)
                    }
                  }
                }
                frame #1 {
                  n2273 = local read "Stop All"() -> (w3809:bool)
                  n2274 = local read "Fl. Triggered..."() -> (w3807:bool)
                  n2275 = Not(x=w3807) -> (.not. x?=w3808:bool)
                  n2276 = Or(x=w3808, y=w3809) -> (x .or. y?=w3806:bool)
                  n2277 = Not(x=w3806) -> (.not. x?=→"Waiting":bool)
                }
              }
              n2278 = node-c288() -> ()  [unwired: 2 out]
            }
            n2279 = node-c288(w3702) -> ()  [unwired: 1 out]
          }
        }
      }
      event "Stop All": Value Change {
        n2280 = event-data() -> ()  [unwired: 7 out]
        n2281 = local read "Stop All"() -> (w3815:bool)
      }
    }
    n2282 = node-c288() -> ()  [unwired: 2 out]
  }
  n2283 = node-c288(w73) -> ()  [unwired: 1 out]
  n2284 = node-c288(w163) -> ()  [unwired: 1 out]
  n2285 = flat-sequence {
    tunnel: w33 -> [w3820]
    tunnel: [w3819] -> w39
    tunnel: [w3816] -> w38
    tunnel: w37 -> [_]
    tunnel: w36 -> [_]
    tunnel: w35 -> [_]
    tunnel: w34 -> [_]
    tunnel: w32 -> [w3817]
    tunnel: w39 -> [w3823]
    tunnel: w38 -> [w3822]
    frame #0 {
      w3818 = FALSE ("APD to FIFO")
      n2286 = xnode "Read/Write Control"("FPGA VI Reference In"=w3820, "error in"=w3817, "APD to FIFO"=w3818, "AI to FIFO"=w3818) -> ("FPGA VI Reference Out"=w3819:T19, "error out"=w3816:errorcluster)
    }
    frame #1 {
      n2287 = xnode "Invoke Method"("FPGA VI Reference In"=w3823, "error in"=w3822) -> ("FPGA VI Reference Out"=w3821:T19)  [unwired: 1 out]
      n2288 = xnode "Close FPGA VI Reference"("FPGA VI Reference In"=w3821) -> ()  [unwired: 1 in, 1 out]
    }
  }
